vi "LabVIEW Function Structure.vi"() -> ()   [LabVIEW 2017]
uses:
  Picture/Home.ctl
  Picture/Machine Paramter and Control.ctl
  Picture/Vision Paramter and Control.ctl
  Picture/Machine Alarm History.ctl
  Picture/Machine Information.ctl
  Picture/Pause.ctl
  Picture/Start.ctl
  Picture/Stop.ctl
  Picture/Open Image File.ctl
  Picture/Open Excel File.ctl
  Picture/User Login.ctl
  Picture/SaveButtom.ctl
  Picture/Data and Run Information new.ctl
  <vilib>/vision/Image Controls.llb/IMAQ Image.ctl
  <vilib>/userdefined/High Color/IMAQdx.ctl
  SubVIs/Global System.vi
  SubVIs/Trige.vi
  <vilib>/Utility/file.llb/Write Delimited Spreadsheet (string).vi
  <vilib>/Utility/file.llb/Write Delimited Spreadsheet (DBL).vi
  <vilib>/Utility/file.llb/Read Delimited Spreadsheet (string).vi
  <resource>/objmgr/imaqdx.rc
panel:
  out "Message":string
  out "引用输出":refnum<k24>
  out "数字 3":dbl
  out "字符串":string
  out "元素":string
  out "数据上传OK/NG 2":bool
  out "路径 2":path
  out "压力表有无 2":string="0"
  out "压力表代码":string
  out "压力表有无":string
  out "连接的字符串":string
  out "数组 2":T1[](array[typedef])
  out "夹爪压力保存路径":path
  out "工单数量":string
  out "压力表类型":string
  out "工单号":string
  out "T/F":string
  out "ValidateBarcode":string="True,10270194,C.0C.50E,Firehawk药物支架系统（CE无标签）RV3035,RV3035,10"
  out "字符一致性连接的字符串":string
  out "computer3":string
  out "computer2":string
  out "computer1":string
  out "运行时间 4":dbl
  in  "前后位置切换":bool
  out "穿管检测初始化状态":bool
  out "穿管压力获取初始化状态":bool
  out "表面检测初始化状态":bool
  out "表面检测处理初始化状态":bool
  out "字符检测初始化状态":bool
  out "扫码枪初始化状态":bool
  out "task out Input 2":refnum<k7>
  out "task out Output 2":refnum<k7>
  out "项名称 2":string[](array[string])
  out "All Files in Dir 2":path[](array[path]) caption="目录中的所有文件"
  in  "数组":dbl[](array[numeric])=[1.0, 2.0, 3.0, 4.0, 5.0, 6.0, 7.0, 8.0, 9.0, 10.0, 11.0, 12.0, 13.0, 14.0, 15.0, 16.0, 17.0, 18.0, 19.0]
  out "Start Time 3":u32
  out "CCD6":path
  out "task out Output":refnum<k7>
  out "task out Input":refnum<k7>
  in  "选项卡控件":T2(tab)
  in  "数值":dbl format="%#_13g"
  in  "选项卡控件 2":enum32{"选项卡 1", "选项卡 2", "选项卡 3"}(tab)
  out "表面检测相机5":T1(plugin-control)
  out "表面检测相机4":T1(plugin-control)
  out "表面检测相机3":T1(plugin-control)
  out "衬丝检测":T1(plugin-control)
  in  "返工按钮":bool
  out "字符比对":bool
  out "穿管相机1":T1(plugin-control)
  out "字符检测相机6":T1(plugin-control)
  in  "穿管触发":bool=TRUE
  out "穿管相机2":T1(plugin-control)
  in  "表面检测触发":bool=TRUE
  in  "字符检测触发":bool=TRUE
  out "XY Graph":cluster{"Y":dbl[], "Y":dbl[]}[](graph) caption="压力-位置图"
  out "相机字符识别":string
  out "扫码枪字符识别":string
  in  "扫码枪触发":bool
  in  "穿管结果强制":bool
  out "传递信息显示":string
  out "x/y":dbl
  out "数据上传OK/NG":bool
  out "穿管产品型号":string[](array[string])
  out "表面产品型号":string[](array[string])
  out "产品型号":string
  out "模板匹配OK/NG":bool
  out "相机A":T1(plugin-control)
  in  "CCDA手动触发":bool
  out "字符方向判定结果":bool
  out "通讯状态":bool
  out "DB5000X-IsSuccess":bool
  out "DB5000R-IsSuccess":bool
  out "DB5000W":bool
  out "设备状态":string="Please Click Start Botton\n------------------------------------"
  out "lock":bool
  out "Tel":string="何东坡 15850164018"
  out "SoftWare Name":string="何东坡 15850164018"
  out "Company Name":string="昆山嘉斯特自动化\n\n昆山嘉斯特自动化"
  out "SW  Updated :":string="#1"
  out "SW  Rev :":string="1.0.0.0V"
  out "Build Date :":string="2018/10/20"
  out "Machine Factor":string[][](table)=[["MOTION", "LIGHT", "SCAN", "VISION"]]
  in  "电脑一表面检测图像处理状态":bool
  in  "电脑一CCD读字符状态":bool
  in  "电脑一穿管检测状态":bool
  in  "电脑一穿管压力获取状态":bool
  in  "电脑一条码枪扫码状态":bool
  in  "确定按钮":bool
  out "结果":string
  in  "输入":string
  in  "压力表数据库":string[][](table)=[["C.0C.01B", "C.0C.19B", "C.0C.01C", "C.0C.19C", "C.0B.0QE", "C.0B.40E"], ["C.0C.02B", "C.0C.74B", "C.0C.02C", "C.0C.20C", "C.0B.0RE", "C.0B.41E"], ["C.0C.03B", "C.0C.24B", "C.0C.03C", "C.0C.21C", "C.0B.0SE", "C.0B.02E"], ["C.0C.04B", "C.0C.20B", "C.0C.04C", "C.0C.22C", "C.0B.0TE", "C.0B.03E"], ["C.0C.05B", "C.0C.78B", "C.0C.05C", "C.0C.23C", "C.0B.0UE", "C.0B.42E"], ["C.0C.06B", "C.0C.25B", "C.0C.06C", "C.0C.24C", "C.0B.0VE", "C.0B.43E"], ["C.0C.07B", "C.0C.19G", "C.0C.07C", "C.0C.25C", "C.0B.0WE", "C.0B.06E"], ["C.0C.08B", "C.0C.20G", "C.0C.08C", "C.0C.26C", "C.0B.0XE", "C.0B.07E"], ["C.0C.09B", "C.0C.24G", "C.0C.09C", "C.0C.27C", "C.0B.0YE", "C.0B.44E"], ["C.0C.10B", "C.0C.25G", "C.0C.10C", "C.0C.28C", "C.0B.0ZE", "C.0B.45E"], ["C.0C.11B", "C.0A.0JD", "C.0C.11C", "C.0C.30C", "C.0B.10E", "C.0B.63E"], ["C.0C.12B", "C.0A.0KD", "C.0C.12C", "C.0C.51C", "C.0B.11E", "C.0B.11E"], ["C.0C.13B", "C.0A.0PD", "C.0C.13C", "C.0C.52C", "C.0B.12E", "C.0B.46E"], ["C.0C.14B", "C.0A.0QD", "C.0C.14C", "C.0C.53C", "C.0B.13E", "C.0B.47E"], ["C.0C.15B", "C.0A.16D", "C.0C.15C", "C.0C.54C", "C.0B.14E", "C.0B.64E"], ["C.0C.16B", "C.0A.1AD", "C.0C.16C", "C.0C.55C", "C.0B.15E", "C.0B.15E"], ["C.0C.17B", "", "C.0C.17C", "C.0C.56C", "C.0B.16E", "C.0B.04F"], ["C.0C.18B", "", "C.0C.18C", "C.0C.57C", "C.0B.17E", "C.0B.05F"], ["C.0C.21B", "", "C.0C.31C", "C.0C.58C", "C.0B.18E", "C.0B.06F"], ["C.0C.22B", "", "C.0C.32C", "C.0C.59C", "C.0B.19E", "C.0B.07F"], ["C.0C.23B", "", "C.0C.33C", "C.0C.60C", "C.0B.1AE", "C.0B.08F"], ["C.0C.59B", "", "C.0C.34C", "C.0C.19E", "C.0B.1BE", "C.0B.09F"], ["C.0C.60B", "", "C.0C.35C", "C.0C.20E", "C.0B.1CE", "C.0B.10F"], ["C.0C.61B", "", "C.0C.36C", "C.0C.21E", "C.0B.1DE", "C.0B.11F"], ["C.0C.62B", "", "C.0C.37C", "C.0C.22E", "C.0B.1EE", "C.0B.12F"], ["C.0C.63B", "", "C.0C.38C", "C.0C.23E", "C.0B.1FE", "C.0B.13F"], ["C.0C.64B", "", "C.0C.39C", "C.0C.24E", "C.0B.1GE", "C.0B.14F"], ["C.0C.65B", "", "C.0C.40C", "C.0C.25E", "C.0B.1HE", "C.0B.15F"], ["C.0C.66B", "", "C.0C.41C", "C.0C.26E", "C.0B.1KE", ""], ["C.0C.67B", "", "C.0C.42C", "C.0C.27E", "C.0B.1LE", ""], ["C.0C.68B", "", "C.0C.43C", "C.0C.28E", "C.0B.1NE", ""], ["C.0C.69B", "", "C.0C.44C", "C.0C.51E", "C.0B.1QE", ""], ["C.0C.70B", "", "C.0C.45C", "C.0C.52E", "C.0B.1SE", ""], ["C.0C.71B", "", "C.0C.46C", "C.0C.53E", "C.0B.1EE", ""], ["C.0C.72B", "", "C.0C.47C", "C.0C.54E", "C.0B.1FE", ""], ["C.0C.73B", "", "C.0C.48C", "C.0C.55E", "C.0B.0QE", ""], ["C.0C.75B", "", "C.0C.49C", "C.0C.56E", "C.0B.0RE", ""], ["C.0C.76B", "", "C.0C.50C", "C.0C.57E", "C.0B.1GE", ""], ["C.0C.77B", "", "C.0C.29C", "C.0C.58E", "C.0B.1HE", ""], ["C.0C.01G", "", "C.0C.01E", "C.0C.59E", "C.0B.0UE", ""], ["C.0C.02G", "", "C.0C.02E", "C.0C.60E", "C.0B.0VE", ""], ["C.0C.03G", "", "C.0C.03E", "C.0C.19H", "C.0B.0WE", ""], ["C.0C.04G", "", "C.0C.04E", "C.0C.20H", "C.0B.1KE", ""], ["C.0C.05G", "", "C.0C.05E", "C.0C.21H", "C.0B.1LE", ""], ["C.0C.06G", "", "C.0C.06E", "C.0C.22H", "C.0B.0YE", ""], ["C.0C.07G", "", "C.0C.07E", "C.0C.23H", "C.0B.0ZE", ""], ["C.0C.08G", "", "C.0C.08E", "C.0C.24H", "C.0B.10E", ""], ["C.0C.09G", "", "C.0C.09E", "C.0C.25H", "C.0B.1NE", ""], ["C.0C.10G", "", "C.0C.10E", "C.0C.26H", "C.0B.12E", ""], ["C.0C.11G", "", "C.0C.11E", "C.0C.27H", "C.0B.13E", ""], ["C.0C.12G", "", "C.0C.12E", "C.0C.28H", "C.0B.14E", ""], ["C.0C.13G", "", "C.0C.13E", "C.0C.29H", "C.0B.1QE", ""], ["C.0C.14G", "", "C.0C.14E", "C.0C.30H", "C.0B.16E", ""], ["C.0C.15G", "", "C.0C.15E", "", "C.0B.17E", ""], ["C.0C.16G", "", "C.0C.16E", "", "C.0B.18E", ""], ["C.0C.17G", "", "C.0C.17E", "", "C.0B.1SE", ""], ["C.0C.18G", "", "C.0C.18E", "", "C.0B.1AE", ""], ["C.0C.21G", "", "C.0C.29E", "", "C.0B.1BE", ""], ["C.0C.22G", "", "C.0C.30E", "", "C.0B.1CE", ""], ["C.0C.23G", "", "C.0C.31E", "", "C.0B.31B", ""], ["C.0A.00D", "", "C.0C.32E", "", "C.0B.32B", ""], ["C.0A.01D", "", "C.0C.33E", "", "C.0B.33B", ""], ["C.0A.02D", "", "C.0C.34E", "", "C.0B.34B", ""], ["C.0A.03D", "", "C.0C.35E", "", "C.0B.35B", ""], ["C.0A.04D", "", "C.0C.36E", "", "C.0B.36B", ""], ["C.0A.05D", "", "C.0C.37E", "", "C.0B.37B", ""], ["C.0A.06D", "", "C.0C.38E", "", "C.0B.38B", ""], ["C.0A.07D", "", "C.0C.39E", "", "C.0B.39B", ""], ["C.0A.08D", "", "C.0C.40E", "", "C.0B.3AB", ""], ["C.0A.09D", "", "C.0C.41E", "", "C.0B.3BB", ""], ["C.0A.0AD", "", "C.0C.42E", "", "C.0B.3CB", ""], ["C.0A.0BD", "", "C.0C.43E", "", "C.0B.1EB", ""], ["C.0A.0CD", "", "C.0C.44E", "", "C.0B.1FB", ""], ["C.0A.0DD", "", "C.0C.45E", "", "C.0B.1GB", ""], ["C.0A.0ED", "", "C.0C.46E", "", "C.0B.12B", ""], ["C.0A.0FD", "", "C.0C.47E", "", "C.0B.1HB", ""], ["C.0A.0GD", "", "C.0C.48E", "", "C.0B.14B", ""], ["C.0A.0HD", "", "C.0C.49E", "", "C.0B.1JB", ""], ["C.0A.0LD", "", "C.0C.50E", "", "C.0B.16B", ""], ["C.0A.0MD", "", "C.0C.51E", "", "C.0B.1KB", ""], ["C.0A.0ND", "", "C.0C.52E", "", "C.0B.18B", ""], ["C.0A.0RD", "", "C.0C.53E", "", "C.0B.1LB", ""], ["C.0A.0SD", "", "C.0C.54E", "", "C.0B.1CB", ""], ["C.0A.0TD", "", "C.0C.55E", "", "C.0B.1MB", ""], ["C.0A.0UD", "", "C.0C.56E", "", "C.0B.1NB", ""], ["C.0A.0VD", "", "C.0C.57E", "", "C.0B.1PB", ""], ["C.0A.0WD", "", "C.0C.58E", "", "C.0B.1QB", ""], ["C.0A.0XD", "", "C.0C.59E", "", "C.0B.1RB", ""], ["C.0A.0YD", "", "C.0C.60E", "", "C.0B.1SB", ""], ["C.0A.0ZD", "", "C.0C.01H", "", "C.0B.1TB", ""], ["C.0A.10D", "", "C.0C.02H", "", "C.0B.1UB", ""], ["C.0A.11D", "", "C.0C.03H", "", "C.0B.1VB", ""], ["C.0A.12D", "", "C.0C.04H", "", "C.0B.1WB", ""], ["C.0A.13D", "", "C.0C.05H", "", "C.0B.1XB", ""], ["C.0A.14D", "", "C.0C.06H", "", "C.0B.1YB", ""], ["C.0A.15D", "", "C.0C.07H", "", "C.0B.1ZB", ""], ["C.0A.17D", "", "C.0C.08H", "", "C.0B.13B", ""], ["C.0A.18D", "", "C.0C.09H", "", "C.0B.21B", ""], ["C.0A.19D", "", "C.0C.10H", "", "C.0B.22B", ""], ["C.0A.1BD", "", "C.0C.11H", "", "C.0B.23B", ""], ["C.0A.1CD", "", "C.0C.12H", "", "C.0B.15B", ""], ["C.0A.1DD", "", "C.0C.13H", "", "C.0B.25B", ""], ["C.0A.1ED", "", "C.0C.14H", "", "C.0B.26B", ""], ["C.0A.1FD", "", "C.0C.15H", "", "C.0B.27B", ""], ["C.0A.1GD", "", "C.0C.16H", "", "C.0B.17B", ""], ["C.0A.1HD", "", "C.0C.17H", "", "C.0B.29B", ""], ["C.0A.1JD", "", "C.0C.18H", "", "C.0B.2AB", ""], ["C.0A.1KD", "", "C.0C.19H", "", "C.0B.2BB", ""], ["C.0A.1LD", "", "C.0C.20H", "", "C.0B.19B", ""], ["C.0A.1MD", "", "C.0C.21H", "", "C.0B.2DB", ""], ["C.0A.1ND", "", "C.0C.22H", "", "C.0B.2EB", ""], ["C.0A.1PD", "", "C.0C.23H", "", "C.0B.2FB", ""], ["", "", "C.0C.24H", "", "C.0B.2GB", ""], ["", "", "C.0C.25H", "", "C.0B.1AB", ""], ["", "", "C.0C.26H", "", "C.0B.1BB", ""], ["", "", "C.0C.27H", "", "C.0B.2KB", ""], ["", "", "C.0C.28H", "", "C.0B.2LB", ""], ["", "", "C.0C.29H", "", "C.0B.2MB", ""], ["", "", "C.0C.30H", "", "C.0B.1DB", ""], ["", "", "C.04.001", "", "C.0B.2PB", ""], ["", "", "C.04.002", "", "C.0B.2QB", ""], ["", "", "C.04.003", "", "C.0B.2RB", ""], ["", "", "C.04.004", "", "C.0B.2SB", ""], ["", "", "C.04.005", "", "C.0B.2TB", ""], ["", "", "C.04.006", "", "C.0B.2UB", ""], ["", "", "C.04.007", "", "C.0B.2VB", ""], ["", "", "C.04.008", "", "C.0B.2WB", ""], ["", "", "C.04.009", "", "C.0B.2XB", ""], ["", "", "C.04.010", "", "C.0B.2YB", ""], ["", "", "C.04.011", "", "C.0B.2ZB", ""], ["", "", "C.04.012", "", "C.0B.30B", ""], ["", "", "C.04.013", "", "C.0B.48E", ""], ["", "", "C.04.014", "", "C.0B.49E", ""], ["", "", "C.04.015", "", "C.0B.65E", ""], ["", "", "C.04.016", "", "C.0B.19E", ""], ["", "", "C.04.017", "", "C.0B.50E", ""], ["", "", "C.04.018", "", "C.0B.51E", ""], ["", "", "C.04.019", "", "C.0B.22E", ""], ["", "", "C.04.020", "", "C.0B.23E", ""], ["", "", "C.04.021", "", "C.0B.52E", ""], ["", "", "C.04.022", "", "C.0B.53E", ""], ["", "", "C.04.023", "", "C.0B.26E", ""], ["", "", "C.04.024", "", "C.0B.27E", ""], ["", "", "C.04.025", "", "C.0B.54E", ""], ["", "", "C.04.026", "", "C.0B.30E", ""], ["", "", "C.04.027", "", "C.0B.31E", ""], ["", "", "C.04.028", "", "C.0B.55E", ""], ["", "", "C.04.029", "", "C.0B.56E", ""], ["", "", "C.04.030", "", "C.0B.57E", ""], ["", "", "C.04.031", "", "C.0B.58E", ""], ["", "", "C.04.032", "", "C.0B.34E", ""], ["", "", "C.04.033", "", "C.0B.35E", ""], ["", "", "C.04.034", "", "C.0B.59E", ""], ["", "", "C.04.035", "", "C.0B.60E", ""], ["", "", "C.04.036", "", "C.0B.61E", ""], ["", "", "C.04.037", "", "C.0B.62E", ""], ["", "", "C.04.038", "", "C.0B.38E", ""], ["", "", "C.04.039", "", "C.0B.39E", ""], ["", "", "C.04.040", "", "C.0B.16F", ""], ["", "", "C.04.041", "", "C.0B.17F", ""], ["", "", "C.04.042", "", "C.0B.18F", ""], ["", "", "C.04.043", "", "C.0B.19F", ""], ["", "", "C.04.044", "", "C.0B.20F", ""], ["", "", "C.04.045", "", "C.0B.21F", ""], ["", "", "C.04.046", "", "C.0B.22F", ""], ["", "", "C.04.047", "", "C.0B.23F", ""], ["", "", "C.04.048", "", "C.0B.24F", ""], ["", "", "C.04.049", "", "C.0B.25F", ""], ["", "", "C.04.050", "", "C.0B.26F", ""], ["", "", "C.04.051", "", "C.0B.27F", ""], ["", "", "C.04.052", "", "C.0B.28F", ""], ["", "", "C.04.053", "", "C.0B.29F", ""], ["", "", "C.04.054", "", "C.0B.30F", ""], ["", "", "C.04.055", "", "C.0B.31F", ""], ["", "", "C.04.056", "", "C.0B.32F", ""], ["", "", "C.04.057", "", "C.0B.33F", ""], ["", "", "C.04.058", "", "C.0B.34F", ""], ["", "", "C.04.059", "", "C.0B.35F", ""], ["", "", "C.04.060", "", "C.0B.36F", ""], ["", "", "C.08.001", "", "C.0B.37F", ""], ["", "", "C.08.002", "", "C.0B.38F", ""], ["", "", "C.08.003", "", "C.0B.39F", ""], ["", "", "C.08.004", "", "C.0B.40F", ""], ["", "", "C.08.005", "", "C.0B.41F", ""], ["", "", "C.08.006", "", "C.0B.42F", ""], ["", "", "C.08.007", "", "C.0B.30B", ""], ["", "", "C.08.008", "", "C.0B.2ZB", ""], ["", "", "C.08.009", "", "C.0B.2YB", ""], ["", "", "C.08.010", "", "C.0B.2XB", ""], ["", "", "C.08.011", "", "C.0B.2WB", ""], ["", "", "C.08.012", "", "C.0B.2VB", ""], ["", "", "C.08.013", "", "C.0B.2UB", ""], ["", "", "C.08.014", "", "C.0B.2TB", ""], ["", "", "C.08.015", "", "C.0B.2SB", ""], ["", "", "C.08.016", "", "C.0B.2RB", ""], ["", "", "C.08.017", "", "C.0B.2QB", ""], ["", "", "C.08.018", "", "C.0B.2PB", ""], ["", "", "C.08.019", "", "C.0B.1DB", ""], ["", "", "C.08.020", "", "C.0B.1CB", ""], ["", "", "C.08.021", "", "C.0B.2MB", ""], ["", "", "C.08.022", "", "C.0B.1LB", ""], ["", "", "C.08.023", "", "C.0B.2LB", ""], ["", "", "C.08.024", "", "C.0B.2KB", ""], ["", "", "C.08.025", "", "C.0B.1BB", ""], ["", "", "C.08.026", "", "C.0B.1AB", ""], ["", "", "C.08.027", "", "C.0B.2GB", ""], ["", "", "C.08.028", "", "C.0B.2FB", ""], ["", "", "C.08.029", "", "C.0B.2EB", ""], ["", "", "C.08.030", "", "C.0B.2DB", ""], ["", "", "C.08.031", "", "C.0B.19B", ""], ["", "", "C.08.032", "", "C.0B.18B", ""], ["", "", "C.08.033", "", "C.0B.2BB", ""], ["", "", "C.08.034", "", "C.0B.1KB", ""], ["", "", "C.08.035", "", "C.0B.2AB", ""], ["", "", "C.08.036", "", "C.0B.29B", ""], ["", "", "C.08.037", "", "C.0B.17B", ""], ["", "", "C.08.038", "", "C.0B.16B", ""], ["", "", "C.08.039", "", "C.0B.27B", ""], ["", "", "C.08.040", "", "C.0B.1JB", ""], ["", "", "C.08.041", "", "C.0B.26B", ""], ["", "", "C.08.042", "", "C.0B.25B", ""], ["", "", "C.08.043", "", "C.0B.15B", ""], ["", "", "C.08.044", "", "C.0B.14B", ""], ["", "", "C.08.045", "", "C.0B.23B", ""], ["", "", "C.08.046", "", "C.0B.1HB", ""], ["", "", "C.08.047", "", "C.0B.22B", ""], ["", "", "C.08.048", "", "C.0B.21B", ""], ["", "", "C.08.049", "", "C.0B.13B", ""], ["", "", "C.08.050", "", "C.0B.12B", ""], ["", "", "C.08.051", "", "C.0B.1ZB", ""], ["", "", "C.08.052", "", "C.0B.1GB", ""], ["", "", "C.08.053", "", "C.0B.1YB", ""], ["", "", "C.08.054", "", "C.0B.1XB", ""], ["", "", "C.08.055", "", "C.0B.1WB", ""], ["", "", "C.08.056", "", "C.0B.1FB", ""], ["", "", "C.08.057", "", "C.0B.1VB", ""], ["", "", "C.08.058", "", "C.0B.1EB", ""], ["", "", "C.08.059", "", "C.0B.1UB", ""], ["", "", "C.08.060", "", "C.0B.1TB", ""], ["", "", "", "", "C.0B.1SB", ""], ["", "", "", "", "C.0B.1RB", ""], ["", "", "", "", "C.0B.1QB", ""], ["", "", "", "", "C.0B.1PB", ""], ["", "", "", "", "C.0B.1NB", ""], ["", "", "", "", "C.0B.1MB", ""], ["", "", "", "", "C.0B.3CB", ""], ["", "", "", "", "C.0B.3BB", ""], ["", "", "", "", "C.0B.3AB", ""], ["", "", "", "", "C.0B.39B", ""], ["", "", "", "", "C.0B.38B", ""], ["", "", "", "", "C.0B.37B", ""], ["", "", "", "", "C.0B.36B", ""], ["", "", "", "", "C.0B.35B", ""], ["", "", "", "", "C.0B.34B", ""], ["", "", "", "", "C.0B.33B", ""], ["", "", "", "", "C.0B.32B", ""], ["", "", "", "", "C.0B.31B", ""], ["", "", "", "", "C.0B.1TE", ""], ["", "", "", "", "C.0B.1DE", ""], ["", "", "", "", "C.0B.1CE", ""], ["", "", "", "", "C.0B.1BE", ""], ["", "", "", "", "C.0B.1AE", ""], ["", "", "", "", "C.0B.1SE", ""], ["", "", "", "", "C.0B.18E", ""], ["", "", "", "", "C.0B.17E", ""], ["", "", "", "", "C.0B.16E", ""], ["", "", "", "", "C.0B.1QE", ""], ["", "", "", "", "C.0B.14E", ""], ["", "", "", "", "C.0B.13E", ""], ["", "", "", "", "C.0B.12E", ""], ["", "", "", "", "C.0B.1NE", ""], ["", "", "", "", "C.0B.10E", ""], ["", "", "", "", "C.0B.0ZE", ""], ["", "", "", "", "C.0B.0YE", ""], ["", "", "", "", "C.0B.1LE", ""], ["", "", "", "", "C.0B.1KE", ""], ["", "", "", "", "C.0B.0WE", ""], ["", "", "", "", "C.0B.0VE", ""], ["", "", "", "", "C.0B.0UE", ""], ["", "", "", "", "C.0B.1HE", ""], ["", "", "", "", "C.0B.1GE", ""], ["", "", "", "", "C.0B.0RE", ""], ["", "", "", "", "C.0B.0QE", ""], ["", "", "", "", "C.0B.1FE", ""], ["", "", "", "", "C.0B.1EE", ""]]
  in  "Save 压力表数据库 Message":T3
  in  "警报记录":string[][](table)
  in  "压力表打印代码据库":string[][](table)=[["C.0A.00D", "C.04.001", "C.0B.31B", ""], ["C.0A.01D", "C.04.002", "C.0B.32B", ""], ["C.0A.02D", "C.04.003", "C.0B.33B", ""], ["C.0A.03D", "C.04.004", "C.0B.34B", ""], ["C.0A.04D", "C.04.005", "C.0B.35B", ""], ["C.0A.05D", "C.04.006", "C.0B.36B", ""], ["C.0A.06D", "C.04.007", "C.0B.37B", ""], ["C.0A.07D", "C.04.008", "C.0B.38B", ""], ["C.0A.08D", "C.04.009", "C.0B.39B", ""], ["C.0A.09D", "C.04.010", "C.0B.3AB", ""], ["C.0A.0AD", "C.04.011", "C.0B.3BB", ""], ["C.0A.0BD", "C.04.012", "C.0B.3CB", ""], ["C.0A.0CD", "C.04.013", "C.0B.1MB", ""], ["C.0A.0DD", "C.04.014", "C.0B.1NB", ""], ["C.0A.0ED", "C.04.015", "C.0B.1PB", ""], ["C.0A.0FD", "C.04.016", "C.0B.1QB", ""], ["C.0A.0GD", "C.04.017", "C.0B.1RB", ""], ["C.0A.0HD", "C.04.018", "C.0B.1SB", ""], ["C.0A.0JD", "C.04.019", "C.0B.1TB", ""], ["C.0A.0KD", "C.04.020", "C.0B.1UB", ""], ["C.0A.0LD", "C.04.021", "C.0B.1VB", ""], ["C.0A.0MD", "C.04.022", "C.0B.1WB", ""], ["C.0A.0ND", "C.04.023", "C.0B.1XB", ""], ["C.0A.0PD", "C.04.024", "C.0B.1YB", ""], ["C.0A.0QD", "C.04.025", "C.0B.1ZB", ""], ["C.0A.0RD", "C.04.026", "C.0B.13B", ""], ["C.0A.0SD", "C.04.027", "C.0B.21B", ""], ["C.0A.0TD", "C.04.028", "C.0B.22B", ""], ["C.0A.0UD", "C.04.029", "C.0B.23B", ""], ["C.0A.0VD", "C.04.030", "C.0B.15B", ""], ["C.0A.0WD", "C.04.031", "C.0B.25B", ""], ["C.0A.0XD", "C.04.032", "C.0B.26B", ""], ["C.0A.0YD", "C.04.033", "C.0B.27B", ""], ["C.0A.0ZD", "C.04.034", "C.0B.17B", ""], ["C.0A.10D", "C.04.035", "C.0B.29B", ""], ["C.0A.11D", "C.04.036", "C.0B.2AB", ""], ["C.0A.12D", "C.04.037", "C.0B.2BB", ""], ["C.0A.13D", "C.04.038", "C.0B.19B", ""], ["C.0A.14D", "C.04.039", "C.0B.2DB", ""], ["C.0A.15D", "C.04.040", "C.0B.2EB", ""], ["C.0A.16D", "C.04.041", "C.0B.2FB", ""], ["C.0A.17D", "C.04.042", "C.0B.2GB", ""], ["C.0A.18D", "C.04.043", "C.0B.1AB", ""], ["C.0A.19D", "C.04.044", "C.0B.1BB", ""], ["C.0A.1AD", "C.04.045", "C.0B.2KB", ""], ["C.0A.1BD", "C.04.046", "C.0B.2LB", ""], ["C.0A.1CD", "C.04.047", "C.0B.2MB", ""], ["C.0A.1DD", "C.04.048", "C.0B.1DB", ""], ["C.0A.1ED", "C.04.049", "C.0B.2PB", ""], ["C.0A.1FD", "C.04.050", "C.0B.2QB", ""], ["C.0A.1GD", "C.04.051", "C.0B.2RB", ""], ["C.0A.1HD", "C.04.052", "C.0B.2SB", ""], ["C.0A.1JD", "C.04.053", "C.0B.2TB", ""], ["C.0A.1KD", "C.04.054", "C.0B.2UB", ""], ["C.0A.1LD", "C.04.055", "C.0B.2VB", ""], ["C.0A.1MD", "C.04.056", "C.0B.2WB", ""], ["C.0A.1ND", "C.04.057", "C.0B.2XB", ""], ["C.0A.1PD", "C.04.058", "C.0B.2YB", ""], ["C.0C.01B", "C.04.059", "C.0B.2ZB", ""], ["C.0C.02B", "C.04.060", "C.0B.30B", ""], ["C.0C.03B", "C.08.001", "C.0B.00N", " "], ["C.0C.04B", "C.08.002", "C.0B.01N", " "], ["C.0C.05B", "C.08.003", "C.0B.02N", " "], ["C.0C.06B", "C.08.004", "C.0B.03N", " "], ["C.0C.07B", "C.08.005", "C.0B.04N", " "], ["C.0C.08B", "C.08.006", "C.0B.05N", " "], ["C.0C.09B", "C.08.007", "C.0B.06N", " "], ["C.0C.10B", "C.08.008", "C.0B.07N", " "], ["C.0C.11B", "C.08.009", "C.0B.08N", " "], ["C.0C.12B", "C.08.010", "C.0B.09N", " "], ["C.0C.13B", "C.08.011", "C.0B.10N", " "], ["C.0C.14B", "C.08.012", "C.0B.11N", " "], ["C.0C.15B", "C.08.013", "C.0B.12N", " "], ["C.0C.16B", "C.08.014", "C.0B.13N", " "], ["C.0C.17B", "C.08.015", "C.0B.14N", " "], ["C.0C.18B", "C.08.016", "C.0B.15N", " "], ["C.0C.19B", "C.08.017", "C.0B.16N", " "], ["C.0C.20B", "C.08.018", "C.0B.17N", " "], ["C.0C.21B", "C.08.019", "C.0B.18N", " "], ["C.0C.22B", "C.08.020", "C.0B.19N", " "], ["C.0C.23B", "C.08.021", "C.0B.20N", " "], ["C.0C.24B", "C.08.022", "C.0B.21N", " "], ["C.0C.25B", "C.08.023", "C.0B.22N", " "], ["C.0C.59B", "C.08.024", "C.0B.23N", " "], ["C.0C.60B", "C.08.025", "C.0B.24N", " "], ["C.0C.61B", "C.08.026", "C.0B.25N", " "], ["C.0C.62B", "C.08.027", "C.0B.26N", " "], ["C.0C.63B", "C.08.028", "C.0B.27N", " "], ["C.0C.64B", "C.08.029", "C.0B.28N", " "], ["C.0C.65B", "C.08.030", "C.0B.29N", " "], ["C.0C.66B", "C.08.031", "C.0B.40E", " "], ["C.0C.67B", "C.08.032", "C.0B.41E", " "], ["C.0C.68B", "C.08.033", "C.0B.02E", " "], ["C.0C.69B", "C.08.034", "C.0B.03E", " "], ["C.0C.70B", "C.08.035", "C.0B.42E", " "], ["C.0C.71B", "C.08.036", "C.0B.43E", " "], ["C.0C.72B", "C.08.037", "C.0B.06E", " "], ["C.0C.73B", "C.08.038", "C.0B.07E", " "], ["C.0C.74B", "C.08.039", "C.0B.44E", " "], ["C.0C.75B", "C.08.040", "C.0B.45E", " "], ["C.0C.76B", "C.08.041", "C.0B.63E", " "], ["C.0C.77B", "C.08.042", "C.0B.11E", " "], ["C.0C.78B", "C.08.043", "C.0B.46E", " "], ["C.0C.01G", "C.08.044", "C.0B.47E", " "], ["C.0C.02G", "C.08.045", "C.0B.64E", " "], ["C.0C.03G", "C.08.046", "C.0B.15E", " "], ["C.0C.04G", "C.08.047", "C.0B.48E", " "], ["C.0C.05G", "C.08.048", "C.0B.49E", " "], ["C.0C.06G", "C.08.049", "C.0B.65E", " "], ["C.0C.07G", "C.08.050", "C.0B.19E", " "], ["C.0C.08G", "C.08.051", "C.0B.50E", " "], ["C.0C.09G", "C.08.052", "C.0B.51E", " "], ["C.0C.10G", "C.08.053", "C.0B.22E", " "], ["C.0C.11G", "C.08.054", "C.0B.23E", " "], ["C.0C.12G", "C.08.055", "C.0B.52E", " "], ["C.0C.13G", "C.08.056", "C.0B.53E", " "], ["C.0C.14G", "C.08.057", "C.0B.26E", " "], ["C.0C.15G", "C.08.058", "C.0B.27E", " "], ["C.0C.16G", "C.08.059", "C.0B.54E", " "], ["C.0C.17G", "C.08.060", "C.0B.30E", " "], ["C.0C.18G", "C.0C.01C", "C.0B.31E", " "], ["C.0C.19G", "C.0C.02C", "C.0B.55E", " "], ["C.0C.20G", "C.0C.03C", "C.0B.56E", " "], ["C.0C.21G", "C.0C.04C", "C.0B.57E", " "], ["C.0C.22G", "C.0C.05C", "C.0B.58E", " "], ["C.0C.23G", "C.0C.06C", "C.0B.34E", " "], ["C.0C.24G", "C.0C.07C", "C.0B.35E", " "], ["C.0C.25G", "C.0C.08C", "C.0B.59E", " "], [" ", "C.0C.09C", "C.0B.60E", " "], [" ", "C.0C.10C", "C.0B.61E", " "], [" ", "C.0C.11C", "C.0B.62E", " "], [" ", "C.0C.12C", "C.0B.38E", " "], [" ", "C.0C.13C", "C.0B.39E", " "], [" ", "C.0C.14C", "C.0B.0QE", " "], [" ", "C.0C.15C", "C.0B.0RE", " "], [" ", "C.0C.16C", "C.0B.0SE", " "], [" ", "C.0C.17C", "C.0B.0TE", " "], [" ", "C.0C.18C", "C.0B.0UE", " "], [" ", "C.0C.19C", "C.0B.0VE", " "], [" ", "C.0C.20C", "C.0B.0WE", " "], [" ", "C.0C.21C", "C.0B.0XE", " "], [" ", "C.0C.22C", "C.0B.0YE", " "], [" ", "C.0C.23C", "C.0B.0ZE", " "], [" ", "C.0C.24C", "C.0B.10E", " "], [" ", "C.0C.25C", "C.0B.11E", " "], [" ", "C.0C.26C", "C.0B.12E", " "], [" ", "C.0C.27C", "C.0B.13E", " "], [" ", "C.0C.28C", "C.0B.14E", " "], [" ", "C.0C.29C", "C.0B.15E", " "], [" ", "C.0C.30C", "C.0B.16E", " "], [" ", "C.0C.31C", "C.0B.17E", " "], [" ", "C.0C.32C", "C.0B.18E", " "], [" ", "C.0C.33C", "C.0B.19E", " "], [" ", "C.0C.34C", "C.0B.1AE", " "], [" ", "C.0C.35C", "C.0B.1BE", " "], [" ", "C.0C.36C", "C.0B.1CE", " "], [" ", "C.0C.37C", "C.0B.1DE", " "], [" ", "C.0C.38C", "C.0B.1EE", " "], [" ", "C.0C.39C", "C.0B.1FE", " "], [" ", "C.0C.40C", "C.0B.1GE", " "], [" ", "C.0C.41C", "C.0B.1HE", " "], [" ", "C.0C.42C", "C.0B.1KE", " "], [" ", "C.0C.43C", "C.0B.1LE", " "], [" ", "C.0C.44C", "C.0B.1NE", " "], [" ", "C.0C.45C", "C.0B.1QE", " "], [" ", "C.0C.46C", "C.0B.1SE", " "], [" ", "C.0C.47C", " ", ""], [" ", "C.0C.48C", " ", ""], [" ", "C.0C.49C", " ", ""], [" ", "C.0C.50C", " ", ""], [" ", "C.0C.51C", " ", ""], [" ", "C.0C.52C", " ", ""], [" ", "C.0C.53C", " ", ""], [" ", "C.0C.54C", " ", ""], [" ", "C.0C.55C", " ", ""], [" ", "C.0C.56C", " ", ""], [" ", "C.0C.57C", " ", ""], [" ", "C.0C.58C", " ", ""], [" ", "C.0C.59C", " ", ""], [" ", "C.0C.60C", " ", ""], [" ", "C.0C.01E", " ", ""], [" ", "C.0C.02E", " ", ""], [" ", "C.0C.03E", " ", ""], [" ", "C.0C.04E", " ", ""], [" ", "C.0C.05E", " ", ""], [" ", "C.0C.06E", " ", ""], [" ", "C.0C.07E", " ", ""], [" ", "C.0C.08E", " ", ""], [" ", "C.0C.09E", " ", ""], [" ", "C.0C.10E", " ", ""], [" ", "C.0C.11E", " ", ""], [" ", "C.0C.12E", " ", ""], [" ", "C.0C.13E", " ", ""], [" ", "C.0C.14E", " ", ""], [" ", "C.0C.15E", " ", ""], [" ", "C.0C.16E", " ", ""], [" ", "C.0C.17E", " ", ""], [" ", "C.0C.18E", " ", ""], [" ", "C.0C.19E", " ", ""], [" ", "C.0C.20E", " ", ""], [" ", "C.0C.21E", " ", ""], [" ", "C.0C.22E", " ", ""], [" ", "C.0C.23E", " ", ""], [" ", "C.0C.24E", " ", ""], [" ", "C.0C.25E", " ", ""], [" ", "C.0C.26E", " ", ""], [" ", "C.0C.27E", " ", ""], [" ", "C.0C.28E", " ", ""], [" ", "C.0C.29E", " ", ""], [" ", "C.0C.30E", " ", ""], [" ", "C.0C.31E", " ", ""], [" ", "C.0C.32E", " ", ""], [" ", "C.0C.33E", " ", ""], [" ", "C.0C.34E", " ", ""], [" ", "C.0C.35E", " ", ""], [" ", "C.0C.36E", " ", ""], [" ", "C.0C.37E", " ", ""], [" ", "C.0C.38E", " ", ""], [" ", "C.0C.39E", " ", ""], [" ", "C.0C.40E", " ", ""], [" ", "C.0C.41E", " ", ""], [" ", "C.0C.42E", " ", ""], [" ", "C.0C.43E", " ", ""], [" ", "C.0C.44E", " ", ""], [" ", "C.0C.45E", " ", ""], [" ", "C.0C.46E", " ", ""], [" ", "C.0C.47E", " ", ""], [" ", "C.0C.48E", " ", ""], [" ", "C.0C.49E", " ", ""], [" ", "C.0C.50E", " ", ""], [" ", "C.0C.51E", " ", ""], [" ", "C.0C.52E", " ", ""], [" ", "C.0C.53E", " ", ""], [" ", "C.0C.54E", " ", ""], [" ", "C.0C.55E", " ", ""], [" ", "C.0C.56E", " ", ""], [" ", "C.0C.57E", " ", ""], [" ", "C.0C.58E", " ", ""], [" ", "C.0C.59E", " ", ""], [" ", "C.0C.60E", " ", ""]]
  out "产品种类":string
  out "压力表打印代码":string
  in  "Type_b":bool
  in  "Type_c":bool
  in  "computer5":bool
  in  "computer4":bool
  in  "computer3":bool
  in  "computer2":bool
  in  "computer1":bool
  in  "清空数据库":bool
  in  "DB5000.X":T4
  in  "输出OUTPUT":T5
  out "输入INPUT":T6
  in  "PLC参数保存":T3
  out "盘管压力值 2":dbl[](array[numeric])
  in  "补偿值":dbl format="%#_13g"
  out "补偿后压力值":dbl format="%#_3g"
  out "数字":u32
  out "数字 2":u32
  out "衬丝口位置":string
  out "长短料":string
  out "粗细料":string
  out "一致性结果字符串":string
  out "ValidateBarcode 2":string="True,10270194,C.0C.50E,Firehawk药物支架系统（CE无标签）RV3035,RV3035,10"
  out "ValidateBarcode 3":string="True,10270194,C.0C.50E,Firehawk药物支架系统（CE无标签）RV3035,RV3035,10"
  out "夹爪压力值":dbl[](array[numeric])
  in  "DB5000.R":T7
  out "Content":u16
  in  "Vision Paramter Save Buttom":T3
  in  "文件名":string(tree)
  out "数据波形图":dbl[][](graph)
  in  "压力数据显示":string[][](table)
  out "查询图片":T1(plugin-control)
  in  "搜索历史图片":bool
  in  "搜索项":string(tree)
  in  "NG/OK":string(combo)="Image"
  in  "检索条件":string(combo)="CCD6"
  out "Ground 2":u16(ring) items=["Administrator", "Engineer", "Operator"]
  in  "Other Param Save Buttom":T3
  out "Start Time 2":u32
  out "CCD2":path
  out "项名称":string[](array[string])
  out "All Files in Dir":path[](array[path]) caption="目录中的所有文件"
  out "CCD1":path
  in  "logo":T8
  out "CMD":string
  out "路径":path
  in  "Auto Run Load Program Name":string(combo)
  in  "Data and Run Information":T9
  in  "User Login":T10
  in  "Open Excel File":T11
  in  "Open Image File":T12
  in  "Stop":T13
  in  "Start":T14
  in  "Pause":T15
  in  "Machine Inforamtion":T16
  in  "Machine Alarm Histroy":T17
  in  "Vision Paramter and Control":T18
  in  "Machine Paramter and Control":T19
  in  "Home":T20
  in  "计数器清零":bool
  out "条码名称":string="Default"
  out "system time":string
  # "检测孔径检测流程"
  # "孔径判定结果"
  # "Standby"
  # "PLC孔径启动信号"
  # "检测孔径尺寸"
  # "铜片检测流程"
  # "铜片检测结果输出"
  # "Standby"
  # "PLC铜片启动信号"
  # "检测孔径"
  # "LoadSystem"
  # "判定结果"
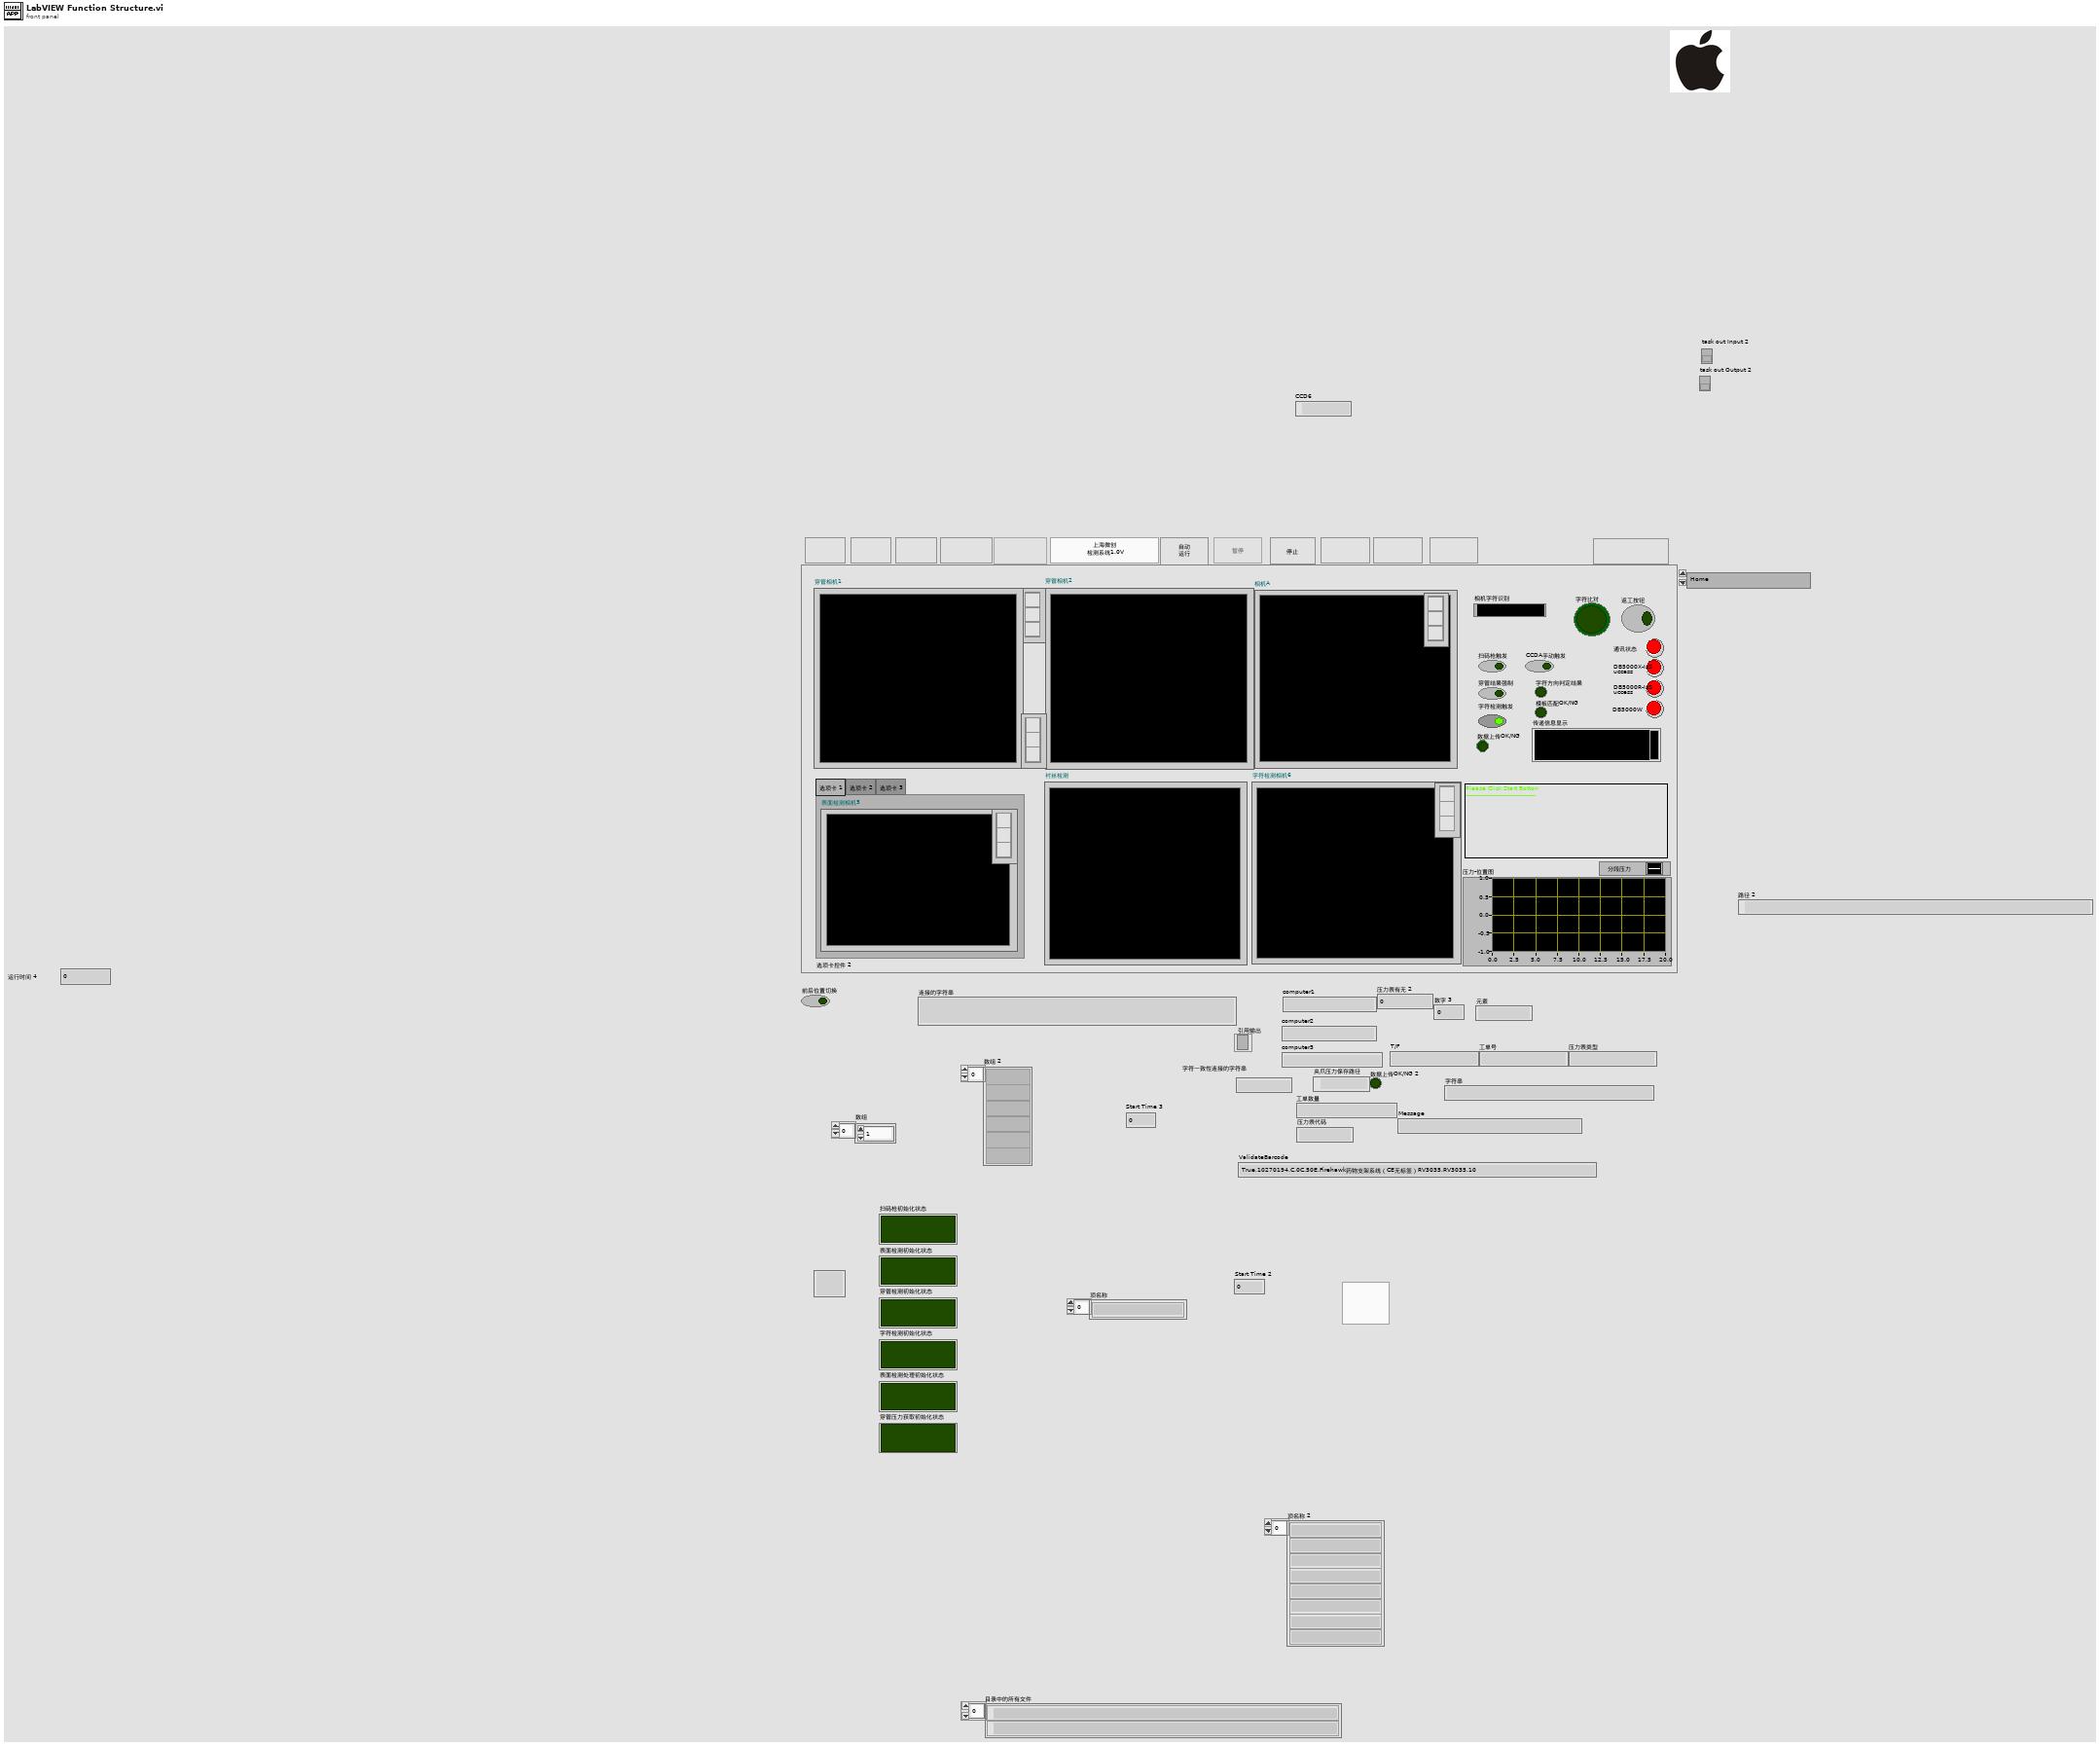
[diagram p1: front panel]
types:
  T1 = typedef "IMAQ Image.ctl" = refnum<image>
  T2 = enum32{"Home", "Machine Information", "Machine Alarm History", "Data and Run Information ", "Machine Paramter and Control", "Vision Paramter and Contorol", "Open Excel File", "Open Image File"}
  T3 = typedef "SaveButtom.ctl" = bool
  T4 = cluster{"字符识别启动\n信号-读":bool, "电脑1扫码枪\n触发-读":bool, "电脑1CCD读取\n字符触发-读":bool, "电脑1表面检测\n触发-读":bool, "电脑1穿管检测\n触发-读":bool, "区间位置\n1-读":bool, "区间位置\n2-读":bool, "区间位置\n3-读":bool, "区间位置\n4-读":bool, "区间位置\n5-读":bool, "区间位置\n6-读":bool, "区间位置\n7-读":bool, "区间位置\n8-读":bool, "区间位置\n9-读":bool, "区间位置\n10-读":bool, "区间位置\n11-读":bool, "区间位置\n12-读":bool, "区间位置\n13-读":bool, "区间位置\n14-读":bool, "区间位置\n15-读":bool, "区间位置\n16-读":bool, "区间位置\n17-读":bool, "区间位置\n18-读":bool, "区间位置\n19-读":bool, "夹爪1\n状态-读":bool, "夹爪2\n状态-读":bool, "夹爪3\n状态-读":bool, "夹爪\n4状态-读":bool, "夹爪\n5状态-读":bool, "夹爪\n6状态-读":bool, "夹爪7\n状态-读":bool, "夹爪8\n状态-读":bool, "夹爪9\n状态-读":bool, "夹爪10\n状态-读":bool, "前后位置\n切换触发-读":bool, "电脑1压力获取\n触发-读":bool, "PC1 ready-\n写 ":bool, "混料-写\n":bool, "字符1检测\npass-写":bool, "字符1检测\nfail-写":bool, "表面检测\npass-写":bool, "表面检测\nfail-写":bool, "穿管检测\npass-写":bool, "穿管检测\nfail-写":bool, "扫码枪\npass-写":bool, "扫码枪fail-\n写":bool, "产品尺寸A-\n写":bool, "产品尺寸B-\n写":bool, "数据传递\n信号-读":bool, "表面检测完\n成信号-读":bool, "穿管NG停止\n信号-写":bool, "电脑1返工\n信号-写":bool, "PLC初始化\n信号-读":bool, "产品尺寸C-\n写":bool, "表面检测错位\n气缸-读":bool, "电脑1衬丝检测\n触发-读":bool, "衬丝能检测\npass-写":bool, "衬丝能检测f\nail-写":bool, "长衬丝-写\n":bool, "短衬丝-写\n":bool, "细料-写":bool, "粗料-写":bool, "一致性检测\n触发-读":bool}
  T5 = cluster{"字符检测pass":bool, "字符检测fail":bool, "表面检测pass":bool, "表面检测fail":bool, "穿管检测pass":bool, "穿管检测fail":bool, "PC1 Ready":bool, "混料":bool, "产品尺寸":bool, "备用1":bool, "字符检测就绪":bool, "表面检测测就绪":bool, "穿管测就绪":bool, "备用2":bool, "备用3":bool, "备用4":bool}
  T6 = cluster{"位置1":bool, "位置2":bool, "位置3":bool, "位置4":bool, "位置6":bool, "位置7":bool, "位置8":bool, "位置9":bool, "位置11":bool, "位置12":bool, "位置13":bool, "位置14":bool, "位置16":bool, "位置17":bool, "位置18":bool, "位置19":bool, "字符检测1触发":bool, "表面检测触发":bool, "穿管检测触发":bool, "位置切换触发":bool, "位置5":bool, "位置10":bool, "位置15":bool, "扫码枪触发":bool, "备用":bool}
  T7 = cluster{"夹爪1压力值":sgl, "夹爪2压力值":sgl, "夹爪3压力值":sgl, "夹爪4压力值":sgl, "夹爪5压力值":sgl, "夹爪6压力值":sgl, "夹爪7压力值":sgl, "夹爪8压力值":sgl, "夹爪9压力值":sgl, "夹爪10压力值":sgl, "盘管底部压力值":sgl, "备用1":sgl, "备用2":sgl, "备用3":sgl, "备用4":sgl}
  T8 = typedef "三星logo.ctl" = bool
  T9 = typedef "Data and Run Information new.ctl" = bool
  T10 = typedef "User Login.ctl" = bool
  T11 = typedef "Open Excel File.ctl" = bool
  T12 = typedef "Open Image File.ctl" = bool
  T13 = typedef "Stop.ctl" = bool
  T14 = typedef "Start.ctl" = bool
  T15 = typedef "Pause.ctl" = bool
  T16 = typedef "Machine Information.ctl" = bool
  T17 = typedef "Machine Alarm History.ctl" = bool
  T18 = typedef "Vision Paramter and Control.ctl" = bool
  T19 = typedef "Machine Paramter and Control.ctl" = bool
  T20 = typedef "Home.ctl" = bool
  T21 = cluster{"index":i32, "this vi":refnum<vi>, "step":cluster{"test step":string[], "step status":bool[], "step index":i32}, "用户登录":cluster{"admin":cluster{"用户名":string[], "密码":string[]}, "engineer":cluster{"用户名":string[], "密码":string[]}, "operator":cluster{"用户名":string[], "密码":string[]}}, "用户权限":i32, "error out":errorcluster, "AllStepNumber":i32, "Run ErrNumber":string, "LoadProgram":string, "TotalNumber":string, "PassNumber":string, "FailNumber":string, "Start Time":string, "2 Pause Message":string, "3 Pause Message":string, "4 Pause Message":string}
  T22 = enum8{"Enabled", "Disabled", "Disabled and Grayed Out"}
  T23 = typedef "Semaphore RefNum" = refnum<k1>
  T24 = cluster{"master data":string, "priority":u16, "secondary data":string[]}
  T25 = cluster{"case name":string[], "queue array":refnum<queue>[]}
  T26 = cluster{"地址":string, "远程端口或服务名称":u16, "超时秒数":dbl}
  T27 = typedef "Image Type" = u32
  T28 = typedef "IMAQdx.ctl" = refnum<k21>
  T29 = cluster{"admin":cluster{"用户名":string[], "密码":string[]}, "engineer":cluster{"用户名":string[], "密码":string[]}, "operator":cluster{"用户名":string[], "密码":string[]}}
  T30 = cluster{"IsNorImage":bool, "Exposure Values":u32, "ImagePath":path}
  T31 = typedef "IMAQ Rectangle" = cluster{"Left":i32, "Top":i32, "Right":i32, "Bottom":i32, "Rotation":dbl}
  T32 = cluster{"Parameters (OCR/OCV 1)":cluster{"Threshold Data":cluster{"Method":enum16{"Fixed Range", "Uniform", "Linear", "Non Linear", "Local", "Color"}, "Looking for":u32, "Color Mode":u32, "Kernel Size":cluster{"Width":i32, "Height":i32}, "Ranges":cluster{"Min":i32, "Max":i32}[]}, "Reject Border":bool, "Number Of Erosions":i32, "Size & Spacing":cluster{"Segment Algorithm":u16, "Min Bounding Rect Width":i32, "Max Bounding Rect Width":i32, "Min Bounding Rect Height":i32, "Max Bounding Rect Height":i32, "Min Character Size":i32, "Max Character Size":i32, "Min Char Spacing":i32, "Max Horiz Element Spacing":i32, "Max Vert Element Spacing":i32, "Max Space Distance":i32}, "Read Options":cluster{"Read Strategy":i32, "Read Resolution":i32, "Scale Dependant":bool, "Aspect Ratio":i32, "Acceptance Level":i32, "Substitution Character":string, "MultiLine":bool}, "Valid Characters":cluster{"Pre-defined characters":i32, "User-defined characters":string}[], "Use Text Pattern":bool, "Orientation":u32, "# Lines Expected":u32, "Number of Blocks":i32}, "Rectangle":T31, "字符长度判定":dbl, "Reference System":cluster{"Origin":cluster{"X":sgl, "Y":sgl}, "Angle (deg)":sgl, "Axis Reference":u32}, "File Path (字符库)":path, "File Path (连接件模板)":path, "Url":string, "accessKey":string}
  T33 = typedef "IMAQ Curve Parameters.ctl" = cluster{"Extraction Mode":u32, "Edge Threshold":i32, "Edge Filter Size":u32, "Min Length":i32, "Row Search Step Size":i32, "Col Search Step Size":i32, "Max Endpoint Gap":i32, "Closed":bool, "Subpixel":bool}
  T34 = typedef "IMAQ Match Range Setting.ctl" = cluster{"Match Constraints":u32, "Min":dbl, "Max":dbl}
  T35 = cluster{"Rectangle":T31, "Settings":cluster{"Curve Parameters":T33, "Match Mode":cluster{"Rotation":bool, "Scale":bool, "Occlusion":bool, "Reserved 1":bool, "Reserved 2":bool, "Reserved 3":bool}, "Range Settings":T34[], "Number of Matches":i32, "Minimum Match Score":sgl, "SubPixel Accuracy":bool, "Adv. Geometric Match Options 2":cluster{"Setup Data Item":u16, "Item Value":dbl}[]}, "Template File Path":path}
  T36 = cluster{"字符识别启动信号-读":bool, "电脑1扫码枪\n触发-读":bool, "电脑1CCD读取\n字符触发-读":bool, "电脑1表面检测\n触发-读":bool, "电脑1穿管检测\n触发-读":bool, "区间位置1-读":bool, "区间位置2-读":bool, "区间位置3-读":bool, "区间位置4-读":bool, "区间位置5-读":bool, "区间位置6-读":bool, "区间位置7-读":bool, "区间位置8-读":bool, "区间位置9-读":bool, "区间位置10-读":bool, "区间位置11-读":bool, "区间位置12-读":bool, "区间位置13-读":bool, "区间位置14-读":bool, "区间位置15-读":bool, "区间位置16-读":bool, "区间位置17-读":bool, "区间位置18-读":bool, "区间位置19-读":bool, "夹爪1状态-读":bool, "夹爪2状态-读":bool, "夹爪3状态-读":bool, "夹爪4状态-读":bool, "夹爪5状态-读":bool, "夹爪6状态-读":bool, "夹爪7状态-读":bool, "夹爪8状态-读":bool, "夹爪9状态-读":bool, "夹爪10状态-读":bool, "电脑1产品前后位置\n切换触发-读":bool, "电脑1压力获取\n触发-读":bool, "PC1 ready-写 ":bool, "混料-写":bool, "字符1检测pass-写":bool, "字符1检测fail-写":bool, "表面检测pass-写":bool, "表面检测fail-写":bool, "穿管检测pass-写":bool, "穿管检测fail-写":bool, "扫码枪pass-写":bool, "扫码枪fail-写":bool, "产品尺寸A-写":bool, "产品尺寸B-写":bool, "数据传递信号-读":bool, "表面检测完成信号-读":bool, "穿管NG停止信号-写":bool, "电脑1返工信号-写":bool, "PLC初始化信号-读":bool, "产品尺寸C-写":bool, "表面检测错位气缸-读":bool, "电脑1衬丝检测触发-读":bool, "衬丝能检测pass-写":bool, "衬丝能检测fail-写":bool, "长衬丝-写":bool, "短衬丝-写":bool, "细料-写":bool, "粗料-写":bool, "一致性检测触发-读":bool}
  T37 = typedef "Edge Options.ctl" = cluster{"Edge Polarity":T38, "Kernel Size":u32, "Width":u32, "Minimum Edge Strength":sgl, "Interpolation Type":enum32{"Zero Order", "Bilinear", "Quadratic", "Cubic", "Bilinear Fixed"}, "Data Processing Method":enum32{"Average", "Median"}}
  T38 = typedef "Edge Polarity.ctl" = u32
  T39 = typedef "IMAQ Line" = cluster{"Start X":i32, "Start Y":i32, "End X":i32, "End Y":i32}
  T40 = cluster{"Settings (Clamp (Rake) 1)":cluster{"Contrast":i32, "Filter width":i32, "Steepness":i32, "Subsampling Ratio":u32, "Show Search Area":bool, "Show Search Lines":bool, "Show Edges Found":bool, "Show Result":bool}, "Options (Find Straight Edge 1)":cluster{"Search Direction":u32, "Edge Options":T37, "Show Search Area":bool, "Show Search Lines":bool, "Show Edges Found":bool, "Show Result":bool, "Search Area Color":u32, "Search Lines Color":u32, "Edge Locations Color":u32, "Result Color":u32, "Overlay Group Name":string}, "相对距离设定":cluster{"上限":dbl, "下限":dbl}, "衬丝直径设定":cluster{"上限":dbl, "下限":dbl}, "保护套直径设定":cluster{"上限":dbl, "下限":dbl}, "Edge Options (Edge Detector 1)":cluster{"Edge Polarity":u32, "Kernel Size":u32, "Width":u32, "Minimum Edge Strength":sgl, "Interpolation Type":enum32{"Zero Order", "Bilinear", "Quadratic", "Cubic", "Bilinear Fixed"}, "Data Processing Method":enum32{"Average", "Median"}}, "保护套标准位置":T39}
  T41 = cluster{"find straight edge Rectangle":T31, "Line 1":T39, "clamp Rectangle ":T31, "Line 2":T39}
  T42 = cluster{"位置1":cluster{"上限":dbl, "下限":dbl}, "位置2":cluster{"上限":dbl, "下限":dbl}, "位置3":cluster{"上限":dbl, "下限":dbl}, "位置4":cluster{"上限":dbl, "下限":dbl}, "位置5":cluster{"上限":dbl, "下限":dbl}, "位置6":cluster{"上限":dbl, "下限":dbl}, "位置7":cluster{"上限":dbl, "下限":dbl}, "位置8":cluster{"上限":dbl, "下限":dbl}, "位置9":cluster{"上限":dbl, "下限":dbl}, "位置10":cluster{"上限":dbl, "下限":dbl}}
  T43 = typedef "Straight Edge Options.ctl" = cluster{"Number of Lines":i32, "Type":T44, "Min. Score":dbl, "Max. Score":dbl, "Orientation":dbl, "Angle Range":dbl, "Angle Tolerance":dbl, "Step Size":u32, "Min. SNR (db)":dbl, "Min. Points (%)":dbl, "Hough Iterations":i32}
  T44 = typedef "Straight Edge Process.ctl" = enum32{"First Edge Rake", "Best Edge Rake", "Hough Edge Rake", "First Edge Projection", "Best Edge Projection"}
  T45 = cluster{"Rectangle":T31, "Find Straight Edge 1":T43, "Process (Edge Detector 1)":enum16{"Get First Edge", "Get First + Last Edge", "Get All Edges", "Get Best Edge"}, "Edge Options (Edge Detector 1)":cluster{"Edge Polarity":u32, "Kernel Size":u32, "Width":u32, "Minimum Edge Strength":sgl, "Interpolation Type":enum32{"Zero Order", "Bilinear", "Quadratic", "Cubic", "Bilinear Fixed"}, "Data Processing Method":enum32{"Average", "Median"}}, "Options (Find Straight Edge 1)":cluster{"Search Direction":u32, "Edge Options":T37, "Show Search Area":bool, "Show Search Lines":bool, "Show Edges Found":bool, "Show Result":bool, "Search Area Color":u32, "Search Lines Color":u32, "Edge Locations Color":u32, "Result Color":u32, "Overlay Group Name":string}, "Parameters (Pattern Matching 1)":cluster{"Number of Matches Requested":i32, "Minimum Match Score":sgl, "Angle Ranges":cluster{"Start Angle":sgl, "End Angle":sgl}[]}, "Template File Path (Pattern Matching 1)":path}
  T46 = cluster{"相机1启动":bool, "相机1反馈":bool, "相机2启动":bool, "相机2反馈":bool, "相机3启动":bool, "相机3反馈":bool, "相机4启动":bool, "相机4反馈":bool, "DI 8":bool, "DI 9":bool, "DI 10":bool, "DI 11":bool, "DI 12":bool, "DI 13":bool, "DI 14":bool, "DI 15":bool, "相机5启动":bool, "相机5反馈":bool, "相机6启动":bool, "相机6反馈":bool}
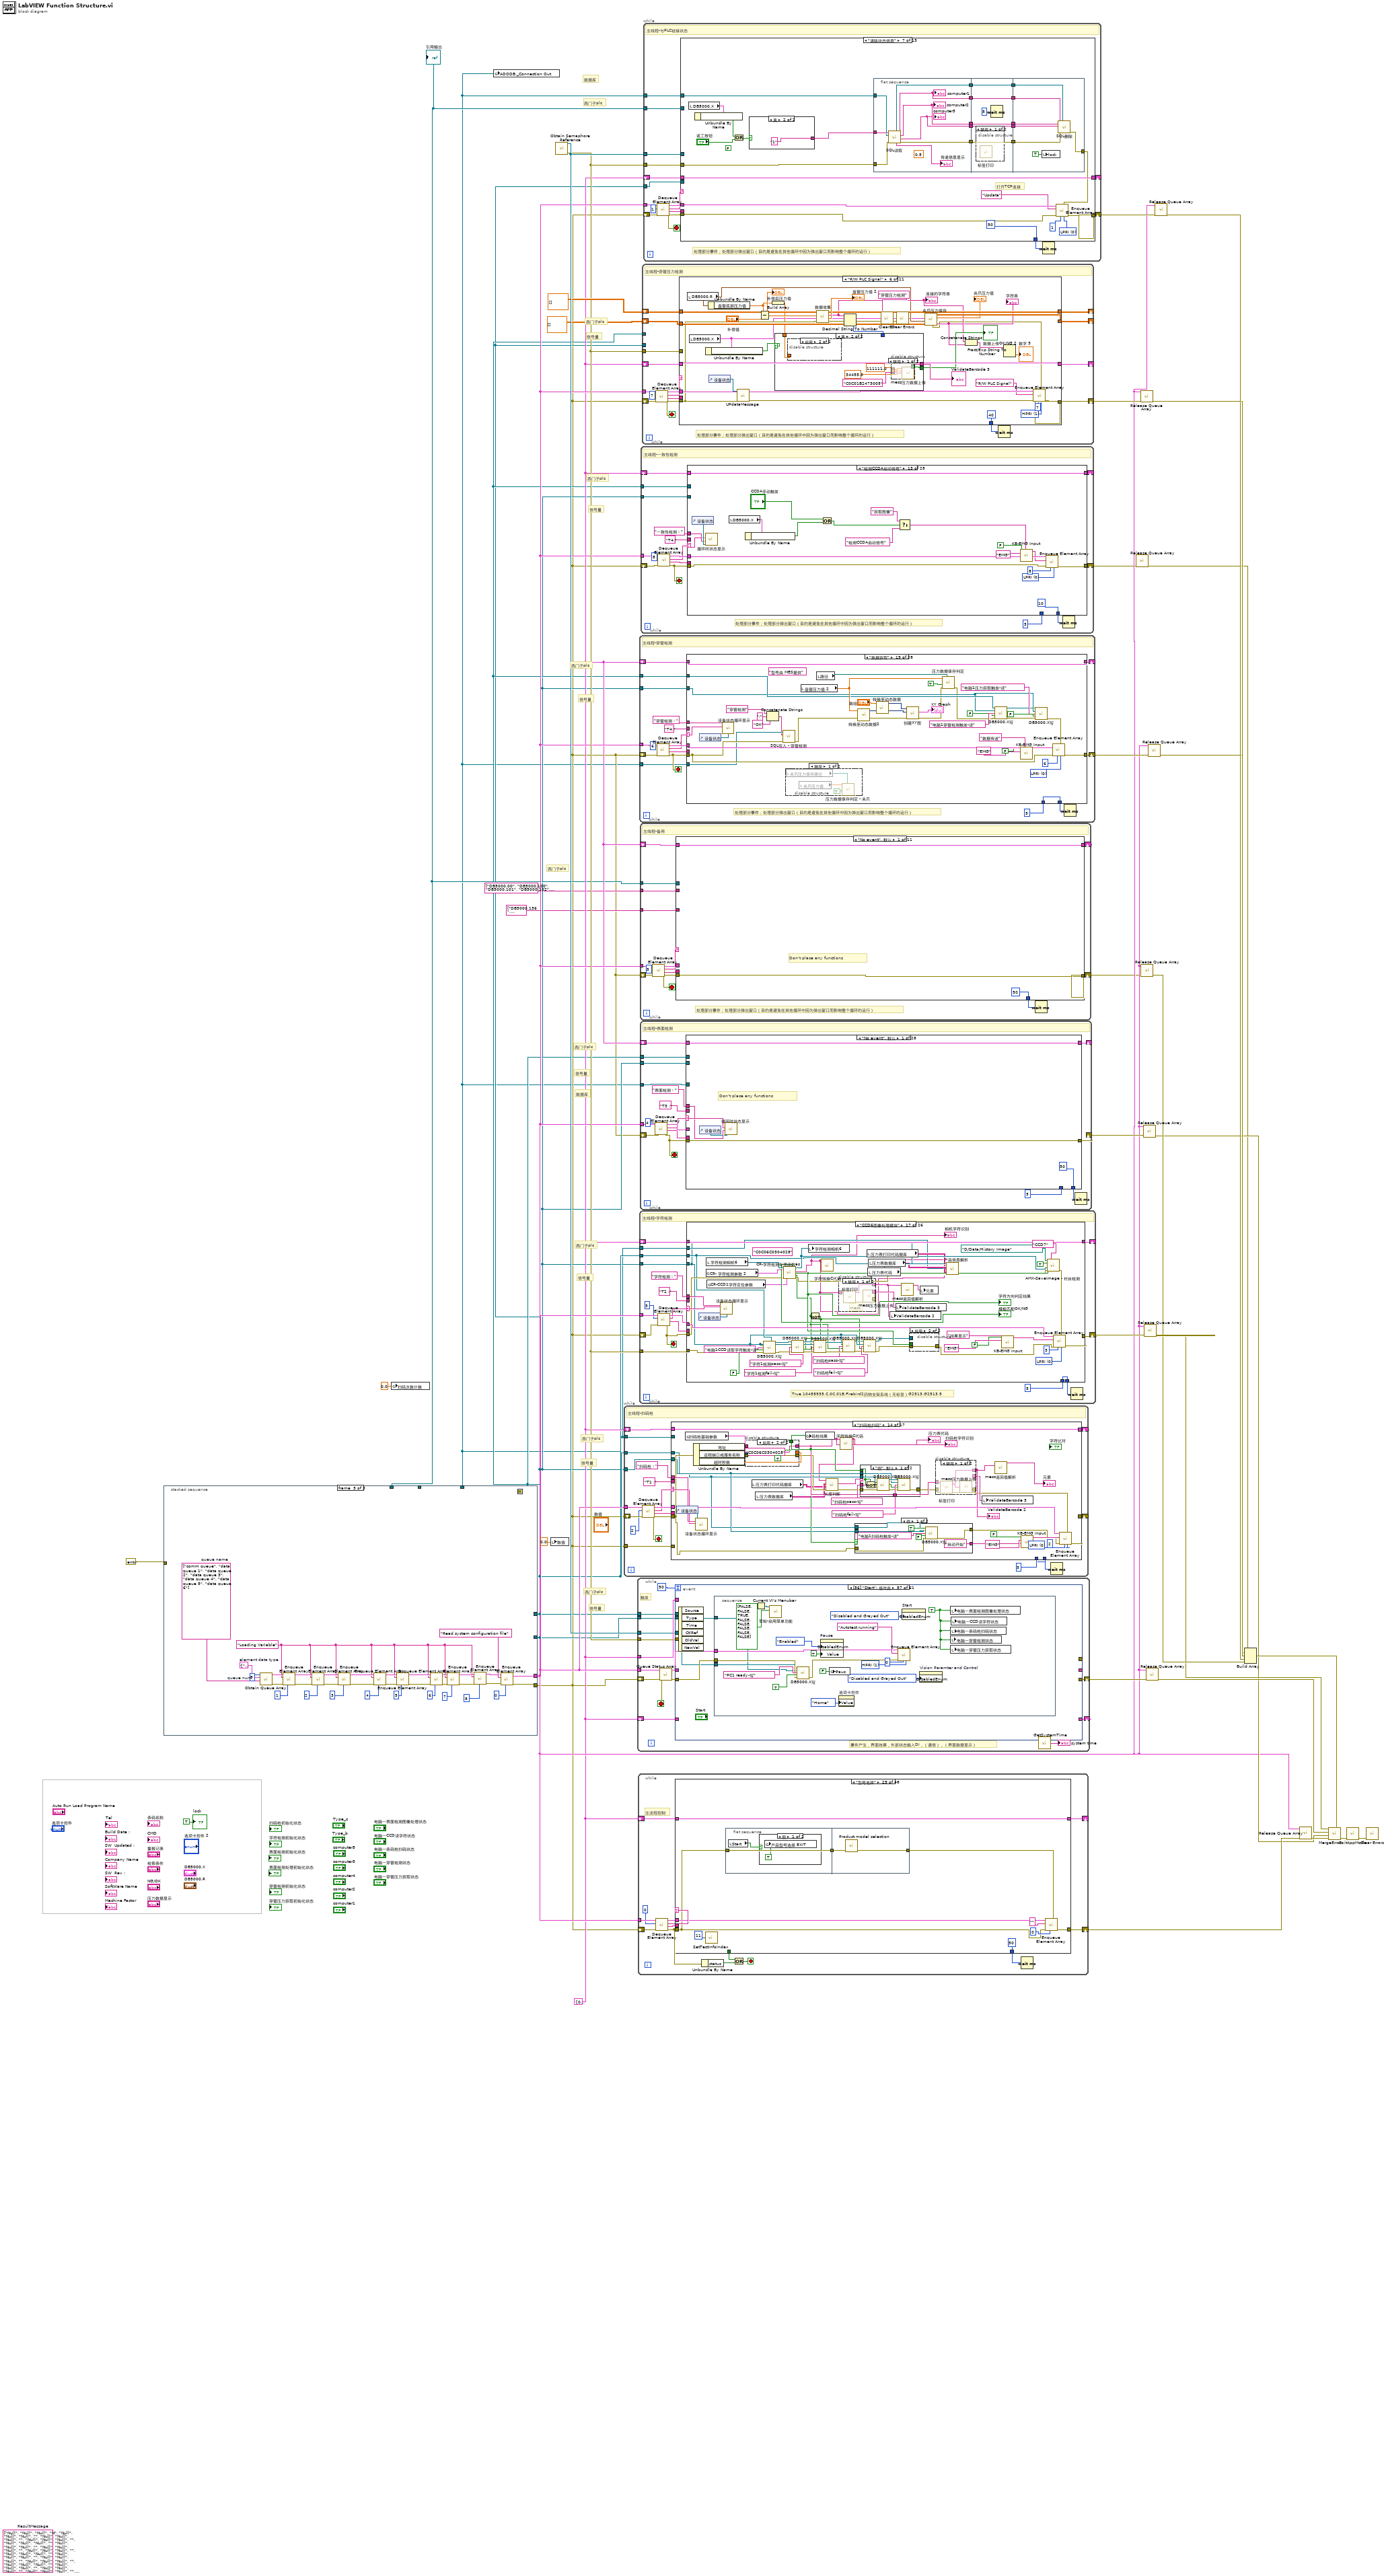
[diagram p0: block diagram]
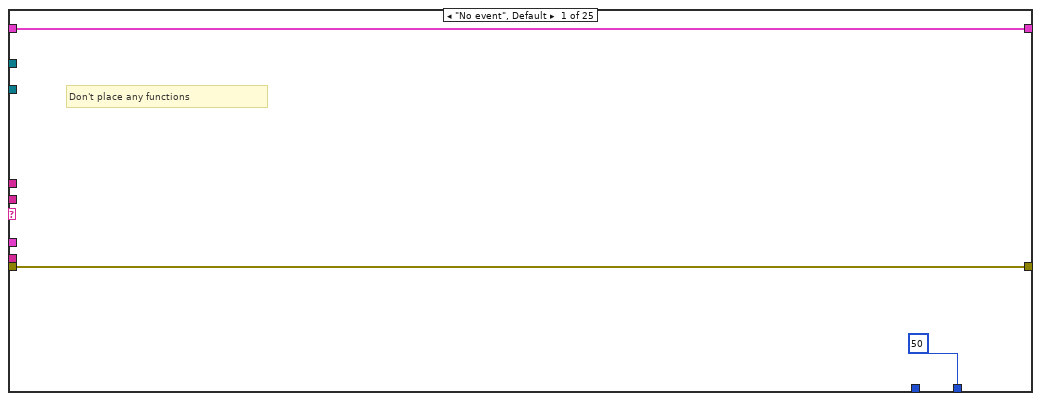
[diagram p2: hidden frame]
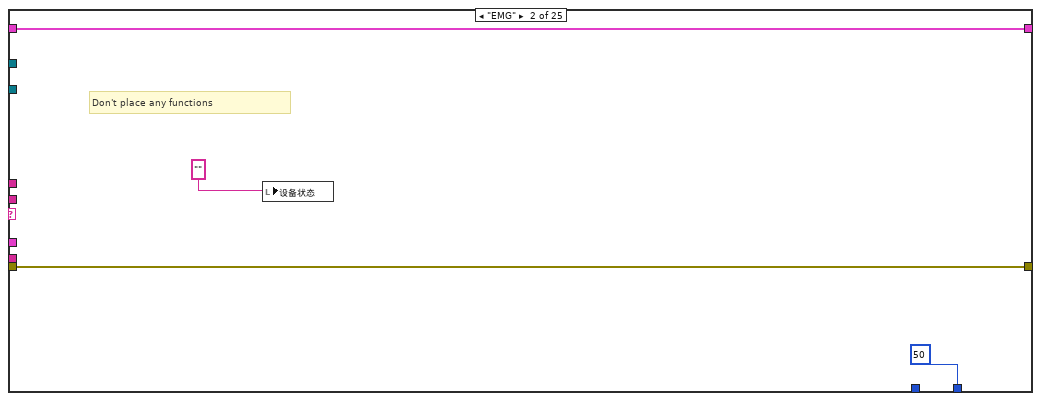
[diagram p3: hidden frame]
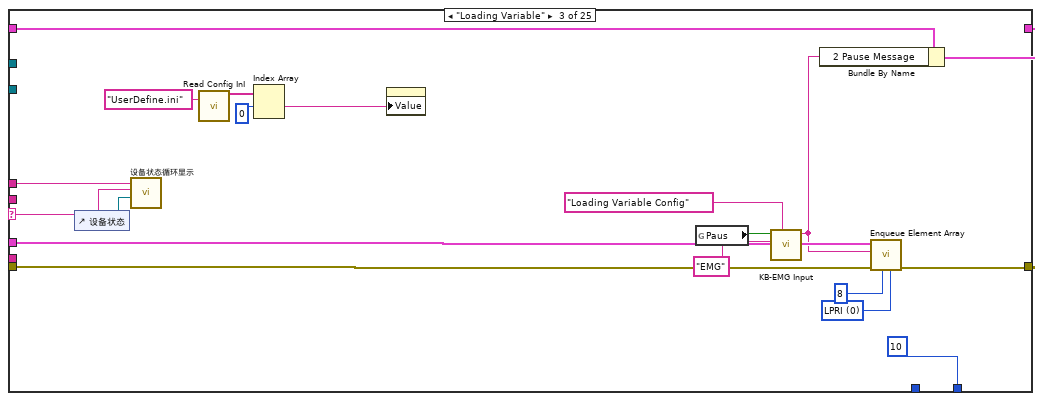
[diagram p4: hidden frame]
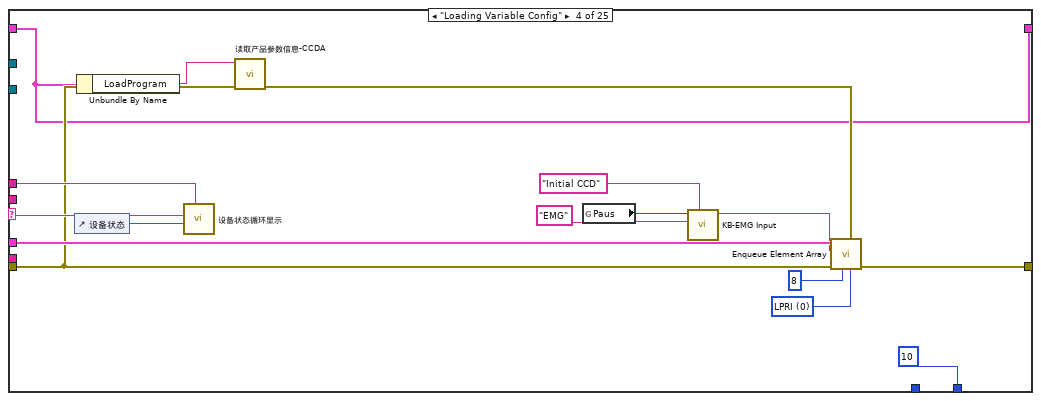
[diagram p5: hidden frame]
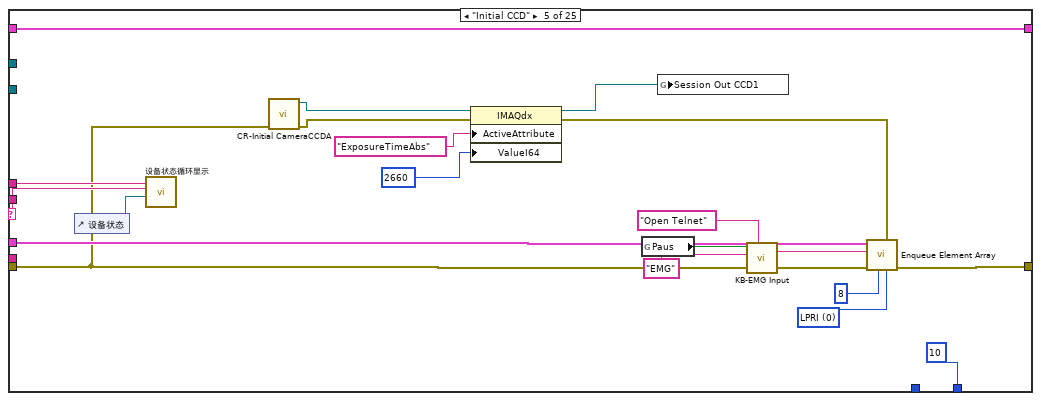
[diagram p6: hidden frame]
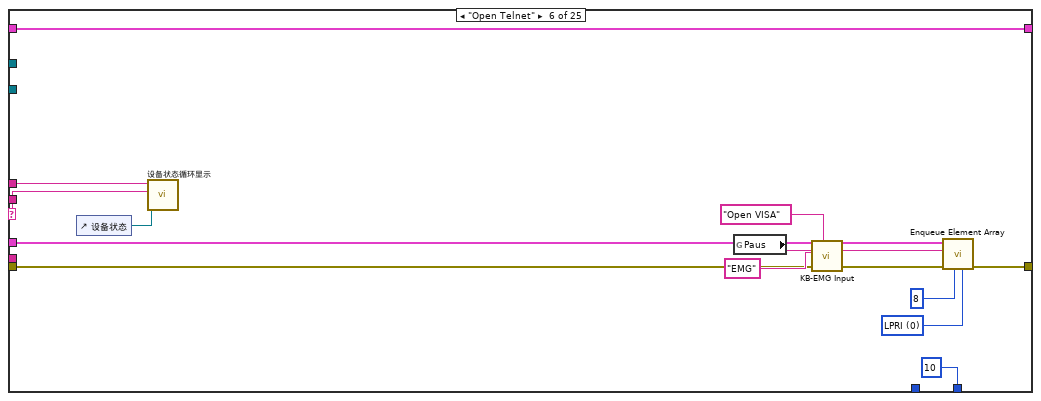
[diagram p7: hidden frame]
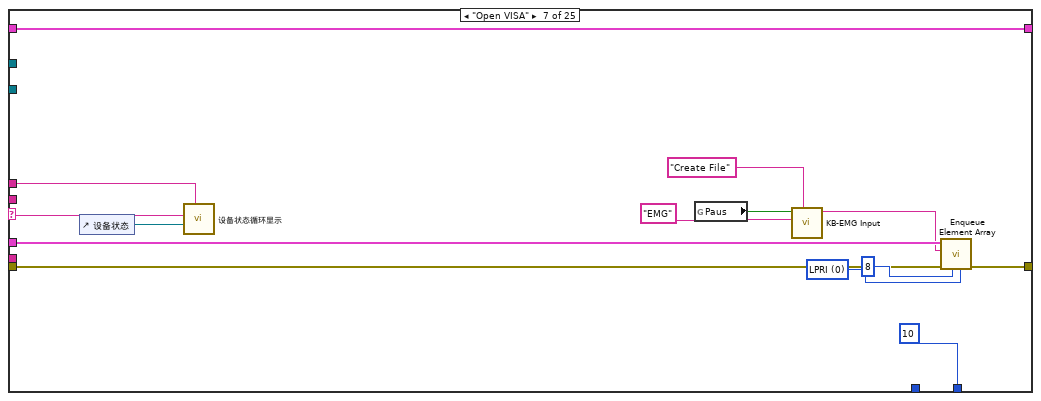
[diagram p8: hidden frame]
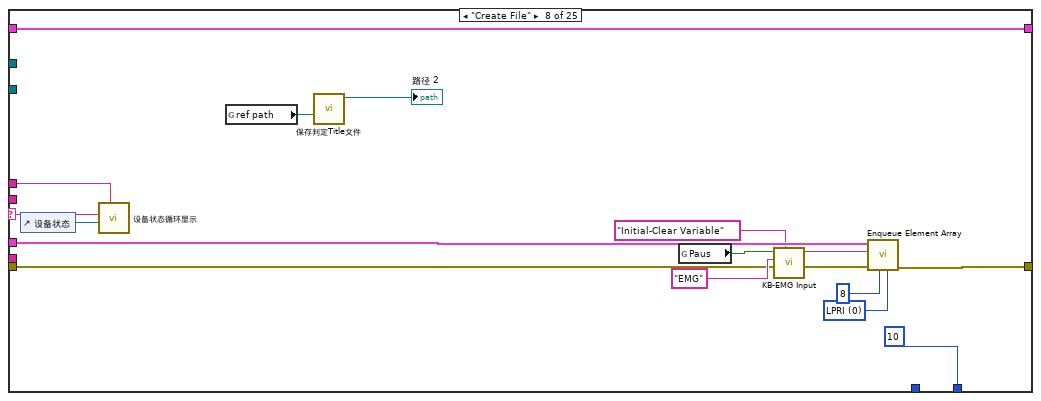
[diagram p9: hidden frame]
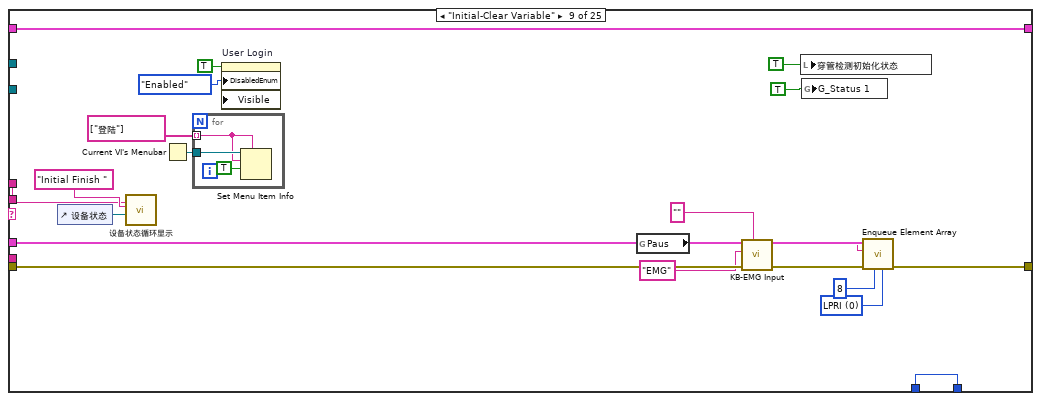
[diagram p10: hidden frame]
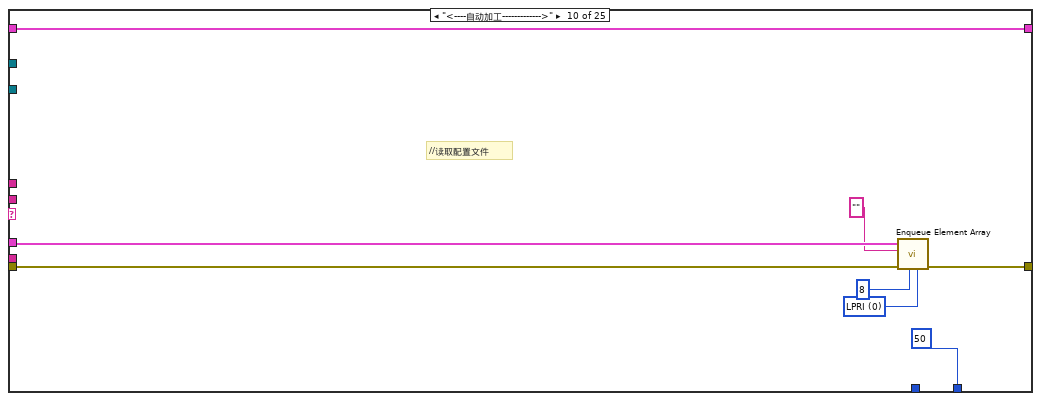
[diagram p11: hidden frame]
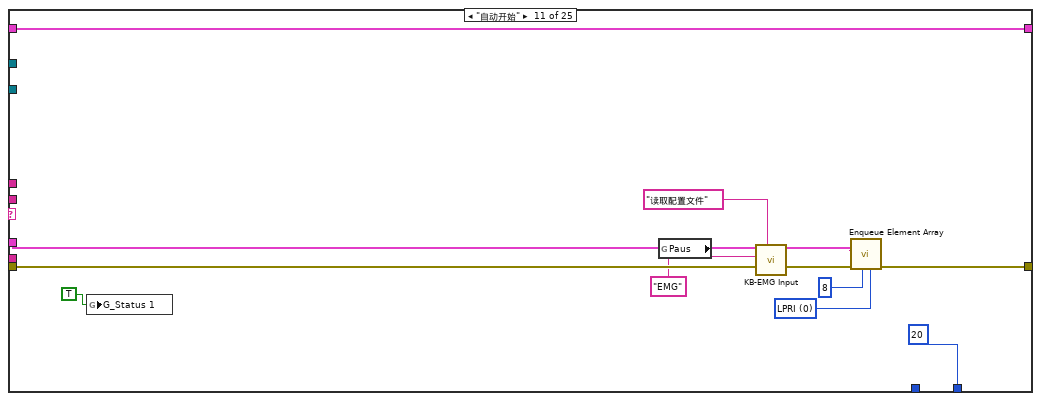
[diagram p12: hidden frame]
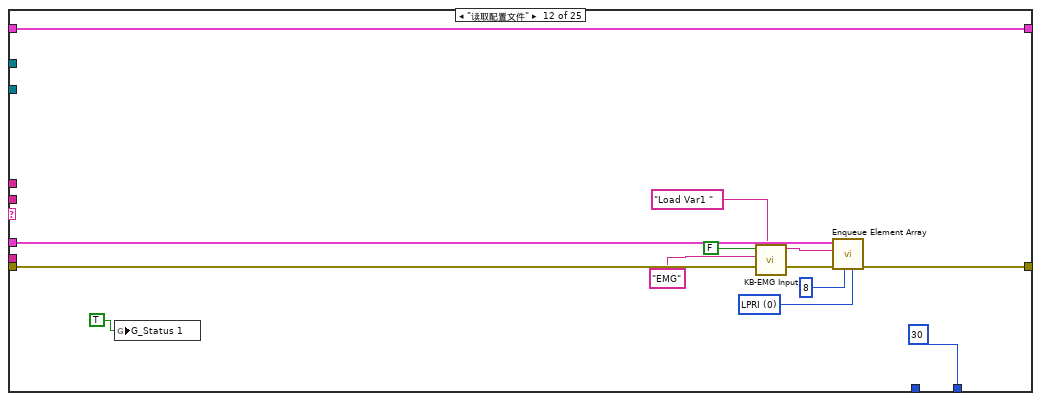
[diagram p13: hidden frame]
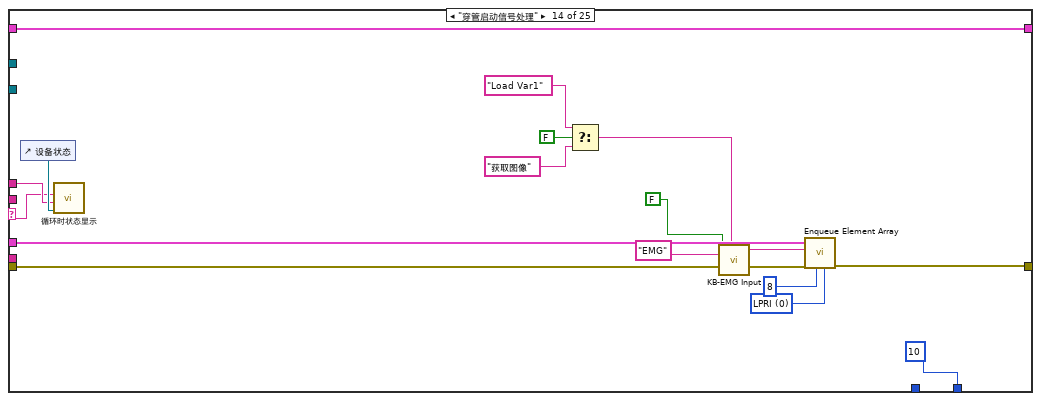
[diagram p14: hidden frame]
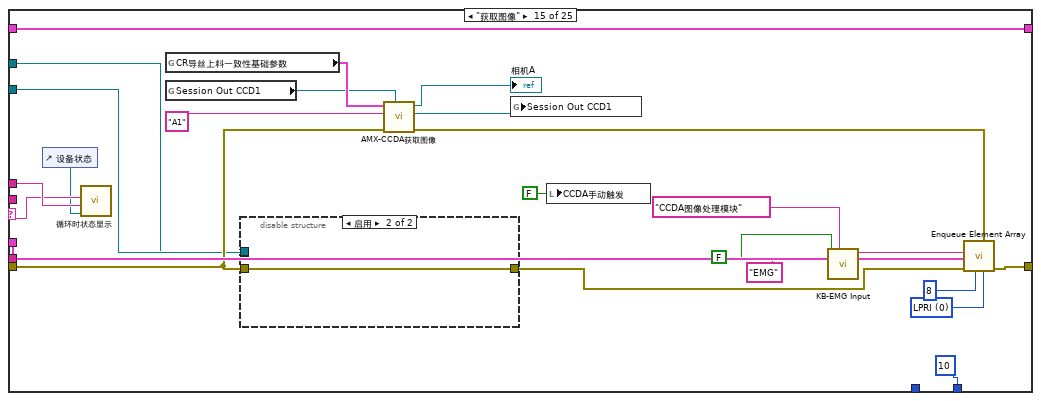
[diagram p15: hidden frame]
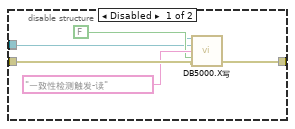
[diagram p16: hidden frame]
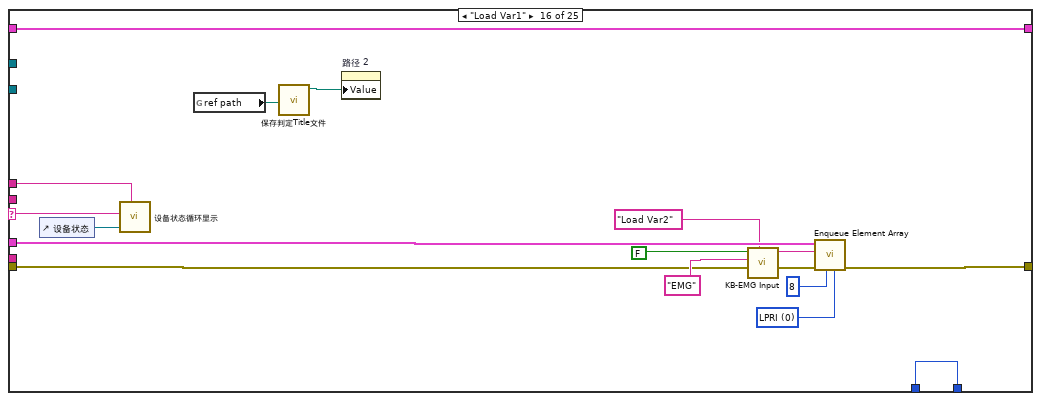
[diagram p17: hidden frame]
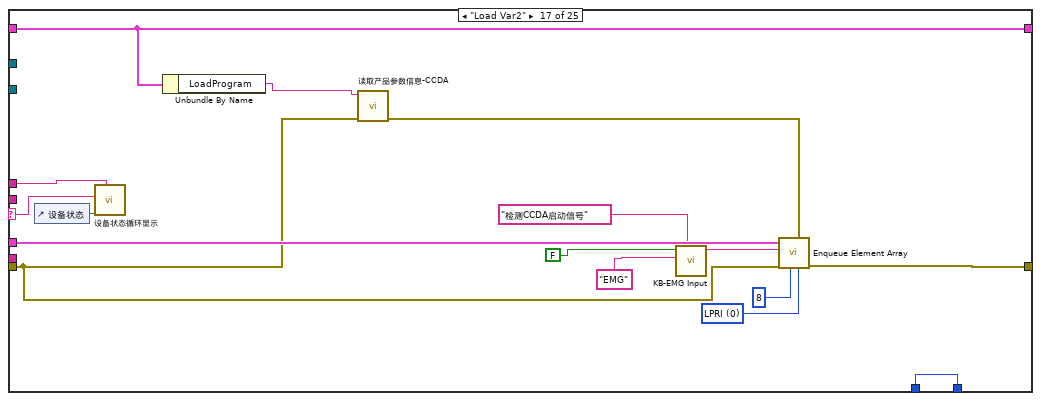
[diagram p18: hidden frame]
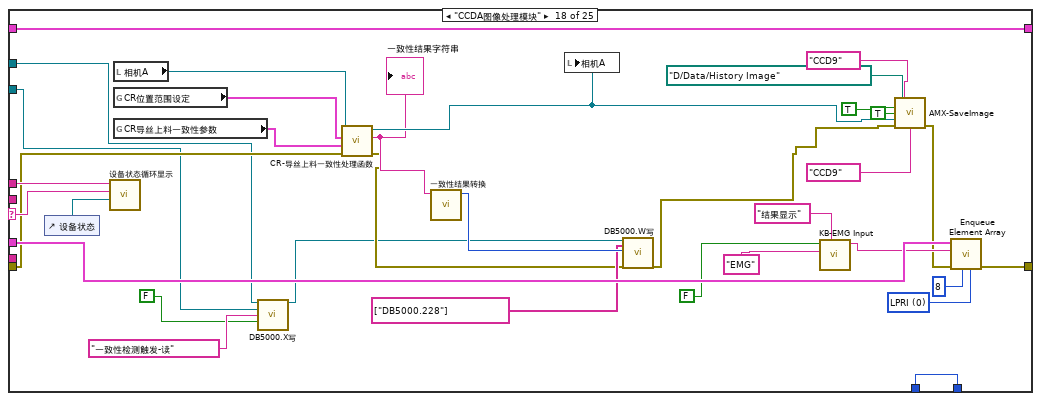
[diagram p19: hidden frame]
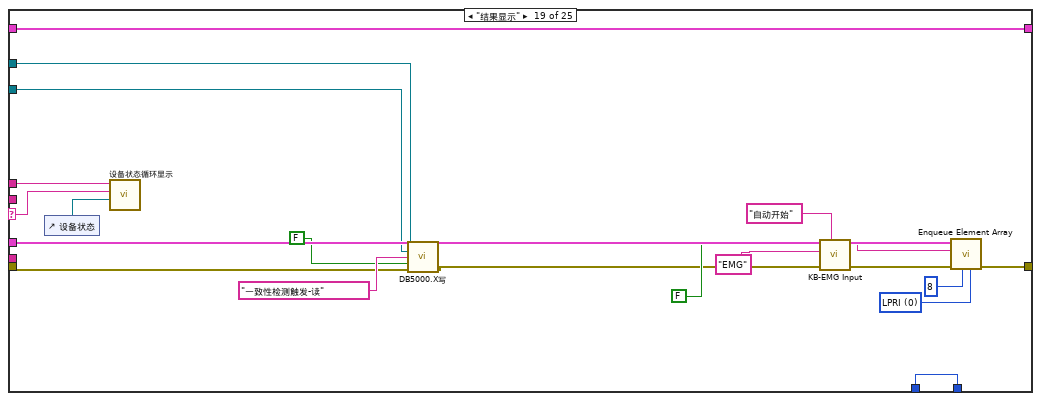
[diagram p20: hidden frame]
diagram:
  (unwired) string[][] [["Null", "Null", "Null", "N"], ["Null", "Null", "Null", ""], ["Null", "Null", "Null", ""], ["Null", "Null", "Null", ""], ["Null", "Null", "Null", ""], ["Null", "Null", "Null", ""], ["Null", "Null", "Null", ""], ["Null", "Null", "Null", ""], ["Null", "Null", "Null", ""], ["Null", "Null", "Null", ""], ["Null", "Null", "Null", ""], ["Null", "Null", "Null", ""], ["Null", "Null", "Null", ""], ["Null", "Null", "Null", ""], ["Null", "Null", "Null", ""], ["Null", "Null", "Null", ""], ["Null", "Null", "Null", ""], ["Null", "Null", "Null", ""], ["Null", "Null", "Null", ""], ["Null", "Null", "Null", ""], ["Null", "Null", "Null", ""], ["Null", "Null", "Null", ""], ["Null", "Null", "Null", ""], ["Null", "Null", "Null", ""], ["Null", "Null", "Null", ""], ["Null", "Null", "Null", ""], ["Null", "Null", "Null", ""], ["Null", "Null", "Null", ""], ["Null", "Null", "Null", ""], ["Null", "Null", "Null", ""], ["Null", "Null", "Null", "N"]]  # ResultMessage
  w14 = T21 {"index"=0, "this vi"=refnum, "step"={"test step"=[], "step status"=[], "step index"=0}, "用户登录"={"admin"={"用户名"=[], "密码"=[]}, "engineer"={"用户名"=[], "密码"=[]}, "operator"={"用户名"=[], "密码"=[]}}, "用户权限"=0, "error out"={"status"=FALSE, "code"=0, "source"=""}, "AllStepNumber"=0, "Run ErrNumber"="", "LoadProgram"="", "TotalNumber"="", "PassNumber"="", "FailNumber"="", "Start Time"="", "2 Pause Message"="", "3 Pause Message"="", "4 Pause Message"=""} ("parameter buffer")
  # "数据库"
  # "信号量"
  # "西门子plc"
  # "信号量"
  # "西门子plc"
  # "信号量"
  # "西门子plc"
  # "信号量"
  # "西门子plc"
  # "信号量"
  # "西门子plc"
  # "信号量"
  # "信号量"
  # "西门子plc"
  # "西门子plc"
  # "西门子plc"
  # "西门子plc"
  # "数据库"
  n1 = stacked-sequence {
    seq-local: [_ w96 _] -> [_ _ _]
    tunnel: [_ _ w132] -> w2
    tunnel: [_ _ w131] -> w15
    tunnel: [_ w95 _] -> _
    tunnel: errorcluster {"status"=FALSE, "code"=0, "source"=""} ("error in (no error)") -> [_ w83 _]
    tunnel: [_ w89 _] -> w1
    tunnel: [_ w84 _] -> w9
    tunnel: [_ w84 _] -> w8
    tunnel: [_ w81 _] -> w7
    frame #0 {
      w41 = "" ("相机字符识别")
      w40 = "" ("电脑一工单数量")
      w42 = FALSE ("电脑一表面检测图像处理状态")
      w43 = "" ("电脑一序号")
      w47 = FALSE ("扫码枪初始化状态")
      w45 = FALSE
      w48 = T15 FALSE ("Pause")
      n2 = shared-variable "我的电脑\\网络共享变量库.lvlib\\电脑一工单数量"(w40) -> ()  [unwired: 1 in, 1 out]
      n3 = local write "相机字符识别"(w41) -> ()
      n4 = local write "扫码枪字符识别"(w41) -> ()
      n5 = shared-variable "我的电脑\\网络共享变量库.lvlib\\电脑一检测信息"(w40) -> ()  [unwired: 1 in, 1 out]
      n6 = local write "传递信息显示"("" ("传递信息显示")) -> ()
      n7 = shared-variable "我的电脑\\网络共享变量库.lvlib\\电脑一序号"(w43) -> ()  [unwired: 1 in, 1 out]
      n8 = shared-variable "我的电脑\\网络共享变量库.lvlib\\电脑一模板类型"(w43) -> ()  [unwired: 1 in, 1 out]
      n9 = shared-variable "我的电脑\\网络共享变量库.lvlib\\电脑一新返工1"(w43) -> ()  [unwired: 1 in, 1 out]
      n10 = shared-variable "我的电脑\\网络共享变量库.lvlib\\电脑一工单号"(w43) -> ()  [unwired: 1 in, 1 out]
      n11 = local write "扫码枪初始化状态"(w47) -> ()
      n12 = local write "字符检测初始化状态"(w47) -> ()
      n13 = local write "表面检测初始化状态"(w47) -> ()
      n14 = local write "穿管检测初始化状态"(w47) -> ()
      n15 = local write "表面检测处理初始化状态"(w47) -> ()
      n16 = local write "穿管压力获取初始化状态"(w47) -> ()
      n17 = disable-structure shown="启用" {
        frame Disabled {
          n18 = for {
            N: 40 -> [_]
            tunnel: [w74] -> w63 mode=indexing
            tunnel: [w73] -> w61 mode=indexing
            tunnel: [w72] -> w62 mode=indexing
            tunnel: [w67] -> _ mode=indexing
            tunnel: [w66] -> _ mode=indexing
            tunnel: [w65] -> _ mode=indexing
            i -> [w75]
            n19 = Number To Decimal String(number=w75) -> (decimal integer string=w68:string)  [unwired: 1 in]
            n20 = Concatenate Strings(w68, "3" ("字符串")) -> (w67:string)
            n21 = Concatenate Strings(w68, "4" ("字符串")) -> (w66:string)
            n22 = Concatenate Strings(w68, "5" ("字符串")) -> (w65:string)
            n23 = call "IMAQ Create"("Image Name"=w67) -> ("New Image"=w74:T1)  [unwired: 4 in, 1 out]
            n24 = call "IMAQ Create"("Image Name"=w66) -> ("New Image"=w72:T1)  [unwired: 4 in, 1 out]
            n25 = call "IMAQ Create"("Image Name"=w65) -> ("New Image"=w73:T1)  [unwired: 4 in, 1 out]
          }
          "数组 2" <- w63
          n26 = global write "Global System.vi" "CCD3"(w63) -> ()
          n27 = global write "Global System.vi" "CCD4"(w62) -> ()
          n28 = global write "Global System.vi" "CCD5"(w61) -> ()
        }
        frame Enabled {
        }
      }
      n29 = local write "电脑一穿管检测状态"(w42) -> ()
      n30 = local write "电脑一表面检测图像处理状态"(w42) -> ()
      n31 = local write "电脑一条码枪扫码状态"(w42) -> ()
      n32 = local write "电脑一穿管压力获取状态"(w42) -> ()
      n33 = local write "电脑一CCD读字符状态"(w42) -> ()
      n34 = disable-structure shown="禁用" {
        frame Disabled {
          n35 = shared-variable "我的电脑\\PLC-OPC.lvlib\\PLC初始化信号"() -> ()  [unwired: 1 in, 2 out]
          n36 = call "SQL-选择清空数据库.vi"("computer1"=TRUE ("computer 4"), "computer 2"=TRUE ("computer 4"), "computer 3"=TRUE ("computer 4"), "computer 4"=TRUE, "computer 5"=TRUE) -> ()  [unwired: 13 in, 2 out]
        }
        frame Enabled {
        }
      }
      n37 = local write "字符比对"(FALSE ("字符比对")) -> ()
      n38 = global write "Global System.vi" "test info C"(string[] ["Read system configuration files", "Read user configuration file"]) -> ()
      n39 = local write "字符检测触发"(w45) -> ()
      n40 = local write "表面检测触发"(w45) -> ()
      n41 = local write "扫码枪触发"(w45) -> ()
      n42 = local write "穿管触发"(w45) -> ()
      n43 = property on="选项卡控件" class="TabCtl (严格)"("Value"=T2."Home" ("选项卡控件")) -> ()  [unwired: 2 in, 2 out]
      n44 = Concatenate Strings("Start....." ("Process 2"), "\r\n") -> (→"设备状态":string)
      n45 = global write "Global System.vi" "CCD1 Trigle Signal"(FALSE ("CCD1 Trigle Signal")) -> ()
      n46 = global write "Global System.vi" "EMG"(FALSE ("EMG")) -> ()
      n47 = global write "Global System.vi" "产品型号选择 EXIT"(FALSE ("EMG")) -> ()
      n48 = global write "Global System.vi" "EMG"(FALSE ("EMG")) -> ()
      n49 = global write "Trige.vi" "Trigle_3"(TRUE ("Trigle_3")) -> ()
      n50 = global write "Global System.vi" "G_Status 1"(TRUE ("G_Status 1")) -> ()
      n51 = global write "Global System.vi" "G_Status 2"(TRUE ("G_Status 1")) -> ()
      n52 = local write "Pause"(w48) -> ()
      n53 = local write "Start"(T14 TRUE ("Start")) -> ()
      n54 = global write "Global System.vi" "Paus"(w48) -> ()
    }
    frame #1 {
      (unwired) T22."Enabled" ("禁用")
      w113 = T22."Disabled and Grayed Out" ("禁用")
      n55 = control-ref of="Start"() -> (w112:refnum<vi>)
      n56 = control-ref of="Pause"() -> (w111:refnum<vi>)
      n57 = control-ref of="Stop"() -> (w110:refnum<vi>)
      n58 = control-ref of="Data and Run Information"() -> (w109:refnum<vi>)
      n59 = control-ref of="Machine Inforamtion"() -> (w108:refnum<vi>)
      n60 = control-ref of="Machine Paramter and Control"() -> (w107:refnum<vi>)
      n61 = control-ref of="Vision Paramter and Control"() -> (w106:refnum<vi>)
      n62 = control-ref of="Machine Alarm Histroy"() -> (w105:refnum<vi>)
      n63 = control-ref of="Open Excel File"() -> (w104:refnum<vi>)
      n64 = control-ref of="Open Image File"() -> (w98:refnum<vi>)
      n65 = Build Array(w112, w111, w110, w109, w108, w107, w106, w105, w104, w98) -> (w103:refnum<vi>[])
      n66 = control-ref of="User Login"() -> (w115:refnum<vi>)
      n67 = control-ref of="Home"() -> (w121:refnum<vi>)
      n68 = Build Array(w115) -> (w116:refnum<vi>[])
      n69 = Build Array(w121) -> (w120:refnum<vi>[])
      n70 = call <vilib>:"Obtain Semaphore Reference.vi"("error in (no error)"=w83) -> ("error out"=w82:errorcluster, "semaphore"=w81:T23)  [unwired: 4 in, 1 out]
      n71 = call "初始化SIEMENS.vi"("错误输入（无错误）"=w83) -> ("错误输出"=w88:errorcluster, "通讯状态"=→"通讯状态":bool, "gInitialSIEMENSS7"=w86:refnum<k24>)  [unwired: 8 in]
      n72 = call "军蚁-工具栏按钮操作.vi"("error in (no error)"=w83, "布尔"=FALSE, "禁用"=w113, "引用数组"=w116) -> ("error out"=w101:errorcluster)  [unwired: 7 in]
      n73 = call "军蚁-工具栏按钮操作.vi"("error in (no error)"=w83, "布尔"=TRUE, "禁用"=w113, "引用数组"=w103) -> ("error out"=w100:errorcluster)  [unwired: 7 in]
      n74 = call "军蚁-工具栏按钮操作.vi"("error in (no error)"=w83, "布尔"=TRUE, "禁用"=T22."Enabled", "引用数组"=w120) -> ("error out"=w102:errorcluster)  [unwired: 7 in]
      n75 = call "DB5000.X写 -AllRest.vi"("引用"=w86, "semaphore"=w81, "error in (no error)"=w88) -> ("引用输出"=w84:refnum<k24>, "error out"=w87:errorcluster)  [unwired: 11 in]
      n76 = Merge Errors(w102, w101, w100) -> (w99:errorcluster)
      n77 = call <userlib>:"ADO Connection Create.vi"("error in (no error)"=w83) -> ("error out"=w91:errorcluster, "ADODB._Connection Out"=w92:refnum<k7>)  [unwired: 9 in]
      n78 = call "BeforeStart.vi"("error in (no error)"=w99) -> ("error out"=w94:errorcluster, "ref path"=w95:path)  [unwired: 8 in, 1 out]
      n79 = Current VI's Menubar "当前VI菜单栏"() -> (w122:refnum<k9>)
      n80 = global write "Global System.vi" "ref path"(w95) -> ()
      n81 = call <userlib>:"ADO Connection Open.vi"("error in (no error)"=w91, "ConnectionString"="DSN=WCYL2;Driver=wcyljust ODBC 5.1 Driver;UID=root;PWD=root123;", "ADODB._Connection In"=w92) -> ("error out"=w90:errorcluster, "ADODB._Connection Out"=w89:refnum<k7>)  [unwired: 7 in]
      n82 = call "军蚁-禁用菜单功能.vi"("error in"=w94, "菜单引用"=w122) -> ("error Out"=w97:errorcluster)  [unwired: 9 in]
      n83 = Merge Errors(w97, w94, w90, w87, w82) -> (w96:errorcluster)
    }
    frame #2 {
      w123 = "Loading Variable" ("master data")
      w154 = string[] ["comm queue", "data queue 1", "data queue 2", "data queue 3", "data queue 4", "data queue 5", "data queue 6"]  # queue name
      w155 = 9  # queue num
      w156 = T24 {"master data"="", "priority"=0, "secondary data"=[]}  # element data type
      n84 = call "Obtain Queue Array.vi"("queue name"=w154, "element data type"=w156, "queue num"=w155) -> ("error out"=w148:errorcluster, "queue out"=w149:T25)  [unwired: 2 in, 1 out]
      n85 = call "Enqueue Element Array.vi"("queue index"=1, "error in"=w148, "master data"=w123, "queue in"=w149) -> ("error out"=w146:errorcluster, "queue out"=w147:T25)  [unwired: 6 in]
      n86 = call "Enqueue Element Array.vi"("queue index"=2, "error in"=w146, "master data"=w123, "queue in"=w147) -> ("error out"=w144:errorcluster, "queue out"=w145:T25)  [unwired: 6 in]
      n87 = call "Enqueue Element Array.vi"("queue index"=3, "error in"=w144, "master data"=w123, "queue in"=w145) -> ("error out"=w142:errorcluster, "queue out"=w143:T25)  [unwired: 6 in]
      n88 = call "Enqueue Element Array.vi"("queue index"=4, "error in"=w142, "master data"=w123, "queue in"=w143) -> ("error out"=w135:errorcluster, "queue out"=w136:T25)  [unwired: 6 in]
      n89 = call "Enqueue Element Array.vi"("queue index"=5, "error in"=w135, "master data"=w123, "queue in"=w136) -> ("error out"=w138:errorcluster, "queue out"=w137:T25)  [unwired: 6 in]
      n90 = call "Enqueue Element Array.vi"("queue index"=6, "error in"=w138, "master data"=w123, "queue in"=w137) -> ("error out"=w133:errorcluster, "queue out"=w134:T25)  [unwired: 6 in]
      n91 = call "Enqueue Element Array.vi"("queue index"=7, "error in"=w133, "master data"=w123, "queue in"=w134) -> ("error out"=w127:errorcluster, "queue out"=w129:T25)  [unwired: 6 in]
      n92 = call "Enqueue Element Array.vi"("queue index"=8, "error in"=w127, "master data"=w123, "queue in"=w129) -> ("error out"=w126:errorcluster, "queue out"=w128:T25)  [unwired: 6 in]
      n93 = call "Enqueue Element Array.vi"("queue index"=0, "error in"=w126, "master data"="Read system configuration file", "queue in"=w128) -> ("error out"=w132:errorcluster, "queue out"=w131:T25)  [unwired: 6 in]
    }
  }
  "引用输出" <- w9
  n94 = global write "Global System.vi" "扫码次数计数"(0.0 ("扫码次数计数")) -> ()
  n95 = global write "Global System.vi" "ADODB._Connection Out"(w1) -> ()
  n96 = local write "数值"(0.0 ("数值")) -> ()
  n97 = call <vilib>:"Obtain Semaphore Reference.vi"() -> ("error out"=w17:errorcluster, "semaphore"=w26:T23)  [unwired: 5 in, 1 out]
  n98 = while "While循环" {
    shift-right: [w174] -> _
    shift-left: w2 -> [w170]
    shift-right: [w171] -> _
    shift-left: w14 -> [w172]
    tunnel: w15 -> [w166]
    tunnel: w2 -> [w160]
    tunnel: w8 -> [w159]
    tunnel: w7 -> [w158]
    tunnel: w1 -> [w157]
    stop <- w165 stop-if-true
    # "主线程-扫码枪"
    n99 = call "Dequeue Element Array.vi"("queue in"=w166, "queue index"=2, "error in"=w170) -> ("queue out"=w169:T25, "master data"=w168:string, "secondary data"=w167:string[], "error out"=w165:errorcluster)  [unwired: 2 in, 1 out]
    n100 = case shown="\"扫码枪扫码\"" w168 {
      selector: w168 -> [w176 _ w196 w212 w226 w239 w253 w267 _ _ _ w331 w346 w382 w480 w568 _]
      tunnel: w169 -> [_ _ w206 w222 w236 w250 w264 w278 w297 w307 w321 w340 w351 w387 w485 w578 w583]
      tunnel: w165 -> [w178 w184 w195 w211 w225 w240 w254 w268 w292 w303 w310 w332 w344 w368 w466 w575 w580]
      tunnel: [w178 w184 w205 w221 w235 w249 w263 w277 w296 w306 w320 w339 w356 w392 w490 w577 w591] -> w174
      tunnel: [50 50 10 10 10 10 10 10 w293 50 20 10 w352 w388 w486 w567 50] -> w173
      tunnel: w172 -> [w179 w185 w188 w209 w224 w238 w252 w266 w285 w304 w312 w329 w343 w380 w478 w566 w589]
      tunnel: [w179 w185 w187 w209 w224 w238 w252 w266 w285 w304 w312 w328 w343 w380 w478 w566 w589] -> w171
      tunnel: w167 -> [_ _ _ _ _ _ _ _ _ _ _ _ _ _ _ _ _]
      tunnel: "扫码枪 : " -> [w175 _ w198 w214 w228 w246 w260 w274 w290 _ _ w334 w353 w389 w487 _ _]
      tunnel: "T1 :" -> [_ _ _ _ _ _ _ _ _ _ _ _ _ _ _ _ _]
      tunnel: 5 -> [_ _ _ _ _ _ _ _ w293 _ _ _ w352 w388 w486 w567 _]
      tunnel: w160 -> [_ _ _ _ _ _ _ _ _ _ _ _ _ _ _ _ _]
      tunnel: w159 -> [_ _ _ _ _ _ _ _ _ _ _ _ _ w366 w459 _ _]
      tunnel: w158 -> [_ _ _ _ _ _ _ _ _ _ _ _ _ w365 w458 _ _]
      tunnel: w157 -> [_ _ _ _ _ _ _ _ _ _ _ _ _ _ w451 _ _]
      frame "No event", Default {
        # "Don't place any functions"
        n101 = disable-structure shown="禁用" {
          disable-tunnel: w176 -> [w181 _]
          disable-tunnel: w175 -> [w180 _]
          frame Disabled {
            n102 = control-ref of="设备状态"() -> (w182:refnum<vi>)
            n103 = call "循环时状态显示.vi"("Str引用句柄"=w182, "cmd:"=w180, "新信息输入"=w181) -> ()  [unwired: 9 in]
          }
          frame Enabled {
          }
        }
      }
      frame "EMG" {
        # "Don't place any functions"
      }
      frame "Loading Variable" {
        w203 = u16 0 items=["HPRI"=1, "LPRI"=0] ("priority")
        n104 = control-ref of="设备状态"() -> (w202:refnum<vi>)
        n105 = call "设备状态循环显示.vi"("cmd:"=w198, "Str引用句柄"=w202, "新信息输入"=w196) -> ()  [unwired: 9 in]
        n106 = call "Read Config InI.vi"("名称或相对路径"="UserDefine.ini") -> ("ParamSet"=w189:string[])  [unwired: 14 in, 4 out]
        n107 = Index Array(array=w189, index #1=0 ("索引")) -> (element #1=w186:string)  [unwired: 1 in, 1 out]
        n108 = global read "Global System.vi" "ref path"() -> (w192:path)
        n109 = Build Path(base path=w192, name or relative path="Template Program" ("名称或相对路径")) -> (appended path=w194:path)
        n110 = Build Path(base path=w194, name or relative path=w186) -> ()  [unwired: 1 out]
        n111 = global read "Global System.vi" "Paus"() -> (w200:bool)
        n112 = Bundle By Name(cluster=w188, "LoadProgram"=w186) -> (w187:T21)
        n113 = call "KB-EMG Input.vi"("Other Message"="Loading Variable Config" ("Element 1"), "EMG Iput"="EMG", "Emg"=w200) -> ("String OutPut"=w197:string)  [unwired: 8 in]
        n114 = call "Enqueue Element Array.vi"("priority"=w203, "queue index"=2, "error in"=w195, "master data"=w197, "queue in"=w206) -> ("error out"=w205:errorcluster)  [unwired: 5 in, 1 out]
      }
      frame "Loading Variable Config" {
        w219 = u16 0 items=["HPRI"=1, "LPRI"=0] ("priority")
        n115 = control-ref of="设备状态"() -> (w218:refnum<vi>)
        n116 = call "设备状态循环显示.vi"("cmd:"=w214, "Str引用句柄"=w218, "新信息输入"=w212) -> ()  [unwired: 9 in]
        n117 = Unbundle By Name(w209) -> ("LoadProgram"=w208:string)
        n118 = call "读取扫码枪参数.vi"("错误输入（无错误）"=w211, "LoadProductName"=w208) -> ("错误输出"=w210:errorcluster)  [unwired: 9 in]
        n119 = global read "Global System.vi" "Paus"() -> (w216:bool)
        n120 = call "KB-EMG Input.vi"("Other Message"="Initial CCD" ("Element 1"), "EMG Iput"="EMG", "Emg"=w216) -> ("String OutPut"=w213:string)  [unwired: 8 in]
        n121 = call "Enqueue Element Array.vi"("priority"=w219, "device error in"=w210, "queue index"=2, "error in"=w211, "master data"=w213, "queue in"=w222) -> ("error out"=w221:errorcluster)  [unwired: 4 in, 1 out]
      }
      frame "Initial CCD" {
        w233 = u16 0 items=["HPRI"=1, "LPRI"=0] ("priority")
        n122 = control-ref of="设备状态"() -> (w232:refnum<vi>)
        n123 = call "设备状态循环显示.vi"("cmd:"=w228, "Str引用句柄"=w232, "新信息输入"=w226) -> ()  [unwired: 9 in]
        n124 = global read "Global System.vi" "Paus"() -> (w230:bool)
        n125 = call "KB-EMG Input.vi"("Other Message"="Open Telnet" ("Element 1"), "EMG Iput"="EMG", "Emg"=w230) -> ("String OutPut"=w227:string)  [unwired: 8 in]
        n126 = call "Enqueue Element Array.vi"("priority"=w233, "queue index"=2, "error in"=w225, "master data"=w227, "queue in"=w236) -> ("error out"=w235:errorcluster)  [unwired: 5 in, 1 out]
      }
      frame "Open Telnet" {
        w247 = u16 0 items=["HPRI"=1, "LPRI"=0] ("priority")
        n127 = control-ref of="设备状态"() -> (w245:refnum<vi>)
        n128 = call "设备状态循环显示.vi"("cmd:"=w246, "Str引用句柄"=w245, "新信息输入"=w239) -> ()  [unwired: 9 in]
        n129 = global read "Global System.vi" "Paus"() -> (w243:bool)
        n130 = call "KB-EMG Input.vi"("Other Message"="Open VISA" ("master data"), "EMG Iput"="EMG", "Emg"=w243) -> ("String OutPut"=w241:string)  [unwired: 8 in]
        n131 = call "Enqueue Element Array.vi"("priority"=w247, "queue index"=2, "error in"=w240, "master data"=w241, "queue in"=w250) -> ("error out"=w249:errorcluster)  [unwired: 5 in, 1 out]
      }
      frame "Open VISA" {
        w261 = u16 0 items=["HPRI"=1, "LPRI"=0] ("priority")
        n132 = control-ref of="设备状态"() -> (w259:refnum<vi>)
        n133 = call "设备状态循环显示.vi"("cmd:"=w260, "Str引用句柄"=w259, "新信息输入"=w253) -> ()  [unwired: 9 in]
        n134 = global read "Global System.vi" "Paus"() -> (w257:bool)
        n135 = call "KB-EMG Input.vi"("Other Message"="Create File" ("master data"), "EMG Iput"="EMG", "Emg"=w257) -> ("String OutPut"=w255:string)  [unwired: 8 in]
        n136 = call "Enqueue Element Array.vi"("priority"=w261, "queue index"=2, "error in"=w254, "master data"=w255, "queue in"=w264) -> ("error out"=w263:errorcluster)  [unwired: 5 in, 1 out]
      }
      frame "Create File" {
        w275 = u16 0 items=["HPRI"=1, "LPRI"=0] ("priority")
        n137 = control-ref of="设备状态"() -> (w273:refnum<vi>)
        n138 = call "设备状态循环显示.vi"("cmd:"=w274, "Str引用句柄"=w273, "新信息输入"=w267) -> ()  [unwired: 9 in]
        n139 = global read "Global System.vi" "Paus"() -> (w271:bool)
        n140 = call "KB-EMG Input.vi"("Other Message"="Initial-Clear Variable" ("master data"), "EMG Iput"="EMG", "Emg"=w271) -> ("String OutPut"=w269:string)  [unwired: 8 in]
        n141 = call "Enqueue Element Array.vi"("priority"=w275, "queue index"=2, "error in"=w268, "master data"=w269, "queue in"=w278) -> ("error out"=w277:errorcluster)  [unwired: 5 in, 1 out]
      }
      frame "Initial-Clear Variable" {
        w294 = u16 0 items=["HPRI"=1, "LPRI"=0] ("priority")
        n142 = control-ref of="设备状态"() -> (w291:refnum<vi>)
        n143 = call "设备状态循环显示.vi"("cmd:"=w290, "Str引用句柄"=w291, "新信息输入"="Initial Finish " ("字符串")) -> ()  [unwired: 9 in]
        n144 = Current VI's Menubar() -> (w283:refnum<k9>)
        n145 = for {
          tunnel: w283 -> [w300]
          tunnel: string[] ["登陆"] -> [w298] mode=indexing
          n146 = Set Menu Item Info(7:w298, 9:TRUE ("已启用"), 10:w298, 11:w300) -> ()  [unwired: 3 in, 2 out]
        }
        n147 = local write "扫码枪初始化状态"(TRUE ("扫码枪初始化状态")) -> ()
        n148 = global write "Global System.vi" "扫码次数计数"(0.0 ("扫码次数计数")) -> ()
        n149 = global read "Global System.vi" "Paus"() -> (w288:bool)
        n150 = call "KB-EMG Input.vi"("Other Message"="" ("Element 1"), "EMG Iput"="EMG", "Emg"=w288) -> ("String OutPut"=w286:string)  [unwired: 8 in]
        n151 = call "Enqueue Element Array.vi"("priority"=w294, "queue index"=2, "error in"=w292, "master data"=w286, "queue in"=w297) -> ("error out"=w296:errorcluster)  [unwired: 5 in, 1 out]
      }
      frame "<----自动加工------------->" {
        w301 = u16 0 items=["HPRI"=1, "LPRI"=0] ("priority")
        # "//读取配置文件"
        n152 = call "Enqueue Element Array.vi"("priority"=w301, "queue index"=2, "error in"=w303, "master data"="" ("Element 1"), "queue in"=w307) -> ("error out"=w306:errorcluster)  [unwired: 5 in, 1 out]
      }
      frame "自动开始" {
        w318 = u16 0 items=["HPRI"=1, "LPRI"=0] ("priority")
        n153 = global write "Global System.vi" "G_Status 2"(TRUE ("G_Status 1")) -> ()
        n154 = global write "Global System.vi" "码枪结果"(FALSE ("码枪结果")) -> ()
        n155 = global read "Global System.vi" "Paus"() -> (w315:bool)
        n156 = call "KB-EMG Input.vi"("Other Message"="读取网络变量" ("EMG Iput"), "EMG Iput"="EMG", "Emg"=w315) -> ("String OutPut"=w314:string)  [unwired: 8 in]
        n157 = call "Enqueue Element Array.vi"("priority"=w318, "queue index"=2, "error in"=w310, "master data"=w314, "queue in"=w321) -> ("error out"=w320:errorcluster)  [unwired: 5 in, 1 out]
      }
      frame "读取网络变量" {
        w337 = u16 0 items=["HPRI"=1, "LPRI"=0] ("priority")
        # "正面垫片PLC启动信号"
        n158 = control-ref of="设备状态"() -> (w335:refnum<vi>)
        n159 = local read "DB5000.X"() -> (w323:T4)
        n160 = call "循环时状态显示 - 3.vi"("Str引用句柄"=w335, "cmd:"=w334, "新信息输入"=w331) -> ()  [unwired: 9 in]
        n161 = Unbundle By Name(w323) -> ("电脑1扫码枪\n触发-读"=w322:bool)
        n162 = Or(x=w322, y="扫码枪触发") -> (x .or. y?=w325:bool)
        n163 = case shown="假" w325 {
          tunnel: ["读取网络变量" ("EMG Iput") " Load Var2" ("EMG Iput")] -> w326
          frame False {
          }
          frame True {
          }
        }
        n164 = call "KB-EMG Input.vi"("Other Message"=w326, "EMG Iput"="EMG", "Emg"=FALSE) -> ("String OutPut"=w327:string)  [unwired: 8 in]
        n165 = Bundle By Name(cluster=w329, "2 Pause Message"=w327) -> (w328:T21)
        n166 = call "Enqueue Element Array.vi"("priority"=w337, "queue index"=2, "error in"=w332, "master data"=w327, "queue in"=w340) -> ("error out"=w339:errorcluster)  [unwired: 5 in, 1 out]
      }
      frame "Load Var2" {
        w354 = u16 0 items=["HPRI"=1, "LPRI"=0] ("priority")
        n167 = control-ref of="设备状态"() -> (w347:refnum<vi>)
        n168 = call "设备状态循环显示.vi"("cmd:"=w353, "Str引用句柄"=w347, "新信息输入"=w346) -> ()  [unwired: 9 in]
        n169 = call "KB-EMG Input.vi"("Other Message"="扫码枪扫码" ("t"), "EMG Iput"="EMG", "Emg"=FALSE) -> ("String OutPut"=w345:string)  [unwired: 8 in]
        n170 = call "Enqueue Element Array.vi"("priority"=w354, "queue index"=2, "error in"=w344, "master data"=w345, "queue in"=w351) -> ("error out"=w356:errorcluster)  [unwired: 5 in, 1 out]
      }
      frame "扫码枪扫码" {
        w390 = u16 0 items=["HPRI"=1, "LPRI"=0] ("priority")
        n171 = control-ref of="设备状态"() -> (w383:refnum<vi>)
        n172 = global read "Global System.vi" "扫码枪基础参数"() -> (w379:T26)
        n173 = Unbundle By Name(w379) -> ("地址"=w378:string, "远程端口或服务名称"=w377:u16, "超时秒数"=w376:dbl)
        n174 = call "设备状态循环显示.vi"("cmd:"=w389, "Str引用句柄"=w383, "新信息输入"=w382) -> ()  [unwired: 9 in]
        n175 = disable-structure shown="启用" {
          disable-tunnel: w378 -> [w399 _]
          disable-tunnel: w377 -> [w398 _]
          disable-tunnel: w376 -> [w397 _]
          disable-tunnel: [w396 "C0C06C0304028" ("扫码枪字符识别")] -> w370
          disable-tunnel: [w395 TRUE ("码枪结果")] -> w369
          disable-tunnel: w368 -> [w394 w401]
          disable-tunnel: [w393 w401] -> w364
          frame Disabled {
            n176 = call "扫码触发.vi"("error in (no error)"=w394, "超时秒数"=w397, "远程端口或服务名称"=w398, "地址"=w399) -> ("error out 2"=w393:errorcluster, "结果"=w395:bool, "数据输出"=w396:string)  [unwired: 5 in]
          }
          frame Enabled {
          }
        }
        "扫码枪字符识别" <- w370
        n177 = local read "压力表打印代码据库"() -> (w362:string[][])
        n178 = local read "压力表数据库"() -> (w363:string[][])
        n179 = global write "Global System.vi" "码枪结果"(w369) -> ()
        n180 = call "字符转换C代码.vi"("扫码枪字符识别"=w370) -> ("子字符串 4"=w361:string)  [unwired: 10 in]
        "压力表代码" <- w361
        n181 = call "长度判断.vi"("error in (no error)"=w364, "压力打印代码据库"=w362, "压力表数据库"=w363, "输入元素"=w361) -> ("error out"=w360:errorcluster, "产品种类"=w357:string)  [unwired: 4 in, 2 out]
        n182 = case shown="假" w369 {
          tunnel: ["自动开始" ("t") "结果显示" ("t")] -> w384
          tunnel: w368 -> [w426 w431]
          tunnel: [w425 w431] -> w367
          tunnel: w366 -> [w424 _]
          tunnel: w365 -> [w423 _]
          frame False {
            n183 = call "DB5000.X写.vi"("引用"=w424, "启用延时"=TRUE, "semaphore"=w423, "地址名称"="电脑1扫码枪触发-读" ("组合框"), "value"=FALSE, "error in (no error)"=w426) -> ("error out"=w425:errorcluster)  [unwired: 8 in, 1 out]
          }
          frame True {
          }
        }
        n184 = case shown="\"假\", 默认" w357 {
          tunnel: "扫码枪pass-写" ("组合框") -> [w412 w418]
          tunnel: "扫码枪fail-写" ("组合框") -> [w411 w419]
          tunnel: w369 -> [w404 _]
          tunnel: w366 -> [w408 w417]
          tunnel: w365 -> [w407 w415]
          tunnel: w360 -> [w406 w422]
          tunnel: [w405 w420] -> w359
          frame "假", Default {
            n185 = Not(x=w404) -> (.not. x?=w403:bool)
            n186 = call "DB5000.X写.vi"("引用"=w408, "semaphore"=w407, "地址名称"=w412, "value"=w404, "error in (no error)"=w406) -> ("引用输出"=w409:refnum<k24>, "error out"=w410:errorcluster)  [unwired: 9 in]
            n187 = call "DB5000.X写.vi"("引用"=w409, "semaphore"=w407, "地址名称"=w411, "value"=w403, "error in (no error)"=w410) -> ("error out"=w405:errorcluster)  [unwired: 9 in, 1 out]
          }
          frame "数据匹配失败" {
            n188 = call "DB5000.X写.vi"("引用"=w417, "semaphore"=w415, "地址名称"=w418, "value"=FALSE, "error in (no error)"=w422) -> ("引用输出"=w416:refnum<k24>, "error out"=w421:errorcluster)  [unwired: 9 in]
            n189 = call "DB5000.X写.vi"("引用"=w416, "semaphore"=w415, "地址名称"=w419, "value"=TRUE, "error in (no error)"=w421) -> ("error out"=w420:errorcluster)  [unwired: 9 in, 1 out]
          }
        }
        n190 = disable-structure shown="禁用" {
          disable-tunnel: w359 -> [w433 w438]
          disable-tunnel: [w437 w438] -> w358
          disable-tunnel: [w436 _] -> w375
          disable-tunnel: w370 -> [w435 _]
          disable-tunnel: [w434 _] -> w373
          frame Disabled {
            n191 = call "标签打印.vi"("error in (no error)"=w433, "barcode"=w435) -> ("error out"=w437:errorcluster, "Print"=w436:string)  [unwired: 8 in]
            n192 = call "mess压力数据上传.vi"("barcode"=w435) -> ("ValidateBarcode"=w434:string)  [unwired: 12 in, 2 out]
          }
          frame Enabled {
          }
        }
        "ValidateBarcode 2" <- w375
        n193 = local write "ValidateBarcode 3"(w373) -> ()
        n194 = call "mess返回值解析.vi"("ValidateBarcode"=w375) -> ("元素"=→"元素":string)  [unwired: 10 in]
        n195 = call "KB-EMG Input.vi"("Other Message"=w384, "EMG Iput"="EMG", "Emg"=FALSE) -> ("String OutPut"=w381:string)  [unwired: 8 in]
        n196 = call "Enqueue Element Array.vi"("priority"=w390, "device error in"=w358, "queue index"=2, "error in"=w367, "master data"=w381, "queue in"=w387) -> ("error out"=w392:errorcluster)  [unwired: 4 in, 1 out]
      }
      frame "结果显示" {
        w444 = TRUE ("启用延时")
        w488 = u16 0 items=["HPRI"=1, "LPRI"=0] ("priority")
        n197 = control-ref of="设备状态"() -> (w481:refnum<vi>)
        n198 = local read "扫码枪字符识别"() -> (w440:string)
        n199 = local read "压力表数据库"() -> (w475:string[][])
        n200 = local read "压力表打印代码据库"() -> (w474:string[][])
        n201 = local read "压力表代码"() -> (w476:string)
        n202 = call "设备状态循环显示.vi"("cmd:"=w487, "Str引用句柄"=w481, "新信息输入"=w480) -> ()  [unwired: 9 in]
        n203 = call "DB5000.X写.vi"("引用"=w459, "启用延时"=TRUE, "semaphore"=w458, "地址名称"="电脑1扫码枪触发-读" ("组合框"), "value"=FALSE, "error in (no error)"=w466) -> ("error out"=w465:errorcluster)  [unwired: 8 in, 1 out]
        n204 = call "mess解析.vi"("ValidateBarcode"=w440, "压力表数据库"=w475, "压力打印代码据库"=w474, "输入元素"=w476, "error in (no error)"=w465) -> ("粗细料"=w471:string, "长短料"=w472:string, "压力表有无"=→"压力表有无 2":string, "衬丝口位置"=w473:string, "工单号"=w470:string, "产品种类"=w439:string, "工单数量"=w468:string, "压力表打印代码"=w467:string, "error out"=w461:errorcluster)  [unwired: 10 in, 4 out]
        "粗细料" <- w471
        n205 = local write "压力表打印代码"(w467) -> ()
        n206 = case shown="\"长料\"" w472 {
          tunnel: w461 -> [w536 w544]
          tunnel: w459 -> [w535 w543]
          tunnel: w458 -> [w534 w542]
          tunnel: [w537 w540] -> w457
          tunnel: [w532 w539] -> w447
          tunnel: w444 -> [w531 w538]
          frame "短料", Default {
            w532 = "短衬丝-写" ("组合框")
            n207 = call "DB5000.X写.vi"("引用"=w535, "启用延时"=w531, "semaphore"=w534, "地址名称"=w532, "value"=TRUE ("电脑1扫码枪\n触发-读"), "error in (no error)"=w536) -> ("error out"=w537:errorcluster)  [unwired: 8 in, 1 out]
          }
          frame "长料" {
            w539 = "长衬丝-写" ("组合框")
            n208 = call "DB5000.X写.vi"("引用"=w543, "启用延时"=w538, "semaphore"=w542, "地址名称"=w539, "value"=TRUE ("电脑1扫码枪\n触发-读"), "error in (no error)"=w544) -> ("error out"=w540:errorcluster)  [unwired: 8 in, 1 out]
          }
        }
        n209 = case shown="\"A\", 默认" w473 {
          tunnel: w459 -> [w551 w557 w565]
          tunnel: w458 -> [w550 w556 w564]
          tunnel: w461 -> [w548 w555 w562]
          tunnel: [w547 w554 w561] -> w462
          tunnel: [w546 w553 w560] -> w449
          tunnel: w444 -> [w545 w552 w559]
          frame "A", Default {
            w546 = "产品尺寸A-写" ("组合框")
            n210 = call "DB5000.X写.vi"("引用"=w551, "启用延时"=w545, "semaphore"=w550, "地址名称"=w546, "value"=TRUE ("电脑1扫码枪\n触发-读"), "error in (no error)"=w548) -> ("error out"=w547:errorcluster)  [unwired: 8 in, 1 out]
          }
          frame "B" {
            w553 = "产品尺寸B-写" ("组合框")
            n211 = call "DB5000.X写.vi"("引用"=w557, "启用延时"=w552, "semaphore"=w556, "地址名称"=w553, "value"=TRUE ("电脑1扫码枪\n触发-读"), "error in (no error)"=w555) -> ("error out"=w554:errorcluster)  [unwired: 8 in, 1 out]
          }
          frame "C" {
            w560 = "产品尺寸C-写" ("组合框")
            n212 = call "DB5000.X写.vi"("引用"=w565, "启用延时"=w559, "semaphore"=w564, "地址名称"=w560, "value"=TRUE ("电脑1扫码枪\n触发-读"), "error in (no error)"=w562) -> ("error out"=w561:errorcluster)  [unwired: 8 in, 1 out]
          }
        }
        n213 = case shown="\"粗料\", 默认" w471 {
          tunnel: w461 -> [w523 w530]
          tunnel: [w522 w526] -> w460
          tunnel: w459 -> [w520 w529]
          tunnel: w458 -> [w519 w528]
          tunnel: [w518 w525] -> w448
          tunnel: w444 -> [w517 w524]
          frame "粗料", Default {
            w518 = "粗料-写" ("组合框")
            n214 = call "DB5000.X写.vi"("引用"=w520, "启用延时"=w517, "semaphore"=w519, "地址名称"=w518, "value"=TRUE ("电脑1扫码枪\n触发-读"), "error in (no error)"=w523) -> ("error out"=w522:errorcluster)  [unwired: 8 in, 1 out]
          }
          frame "细料" {
            w525 = "细料-写" ("组合框")
            n215 = call "DB5000.X写.vi"("引用"=w529, "启用延时"=w524, "semaphore"=w528, "地址名称"=w525, "value"=TRUE ("电脑1扫码枪\n触发-读"), "error in (no error)"=w530) -> ("error out"=w526:errorcluster)  [unwired: 8 in, 1 out]
          }
        }
        n216 = disable-structure shown="启用" {
          disable-tunnel: [w491 w492] -> w441
          disable-tunnel: w439 -> [_ w495]
          frame Disabled {
            n217 = global read "Global System.vi" "码枪结果"() -> (w491:bool)
          }
          frame Enabled {
            n218 = Equal?(x=w495, y="数据匹配失败") -> (x = y?=w493:bool)
            n219 = Not(x=w493) -> (.not. x?=w492:bool)
          }
        }
        n220 = Format Date/Time String(time format string (%c)="%Y-%m-%d %H:%M:%S" ("时间格式字符串(%c)")) -> (date/time string=w442:string)  [unwired: 2 in]
        n221 = Build Array(w442, w449, w448, w447) -> (w446:string[])
        n222 = Concatenate Strings("字符一致性:", "OK" ("字符串")) -> (w453:string)
        n223 = Merge Errors(w462, w460, w457) -> (w456:errorcluster)
        n224 = case shown="真" w441 {
          tunnel: w470 -> [w501 w516]
          tunnel: w440 -> [w500 w515]
          tunnel: w456 -> [w498 w514]
          tunnel: [w497 w513] -> w455
          tunnel: w453 -> [w499 w512]
          tunnel: w468 -> [_ _]
          tunnel: w467 -> [_ _]
          tunnel: w439 -> [_ w509]
          tunnel: w451 -> [_ w508]
          frame False {
            n225 = disable-structure shown="启用" {
              disable-tunnel: w501 -> [w507 _]
              disable-tunnel: w500 -> [w506 _]
              disable-tunnel: w499 -> [w505 _]
              disable-tunnel: w498 -> [w504 _]
              disable-tunnel: [w503 _] -> w497
              frame Disabled {
                n226 = call "SQL写入 - NG.vi"("WorkNumber"=w507, "ProductNumber"=w506, "TestMessage"=w505, "ProssureType"="A1", "error in (no error)"=w504) -> ("error out"=w503:errorcluster)  [unwired: 9 in, 1 out]
              }
              frame Enabled {
              }
            }
            n227 = local write "字符比对"(FALSE ("字符比对")) -> ()
          }
          frame True {
            n228 = call "SQL写入.vi"("WorkNumber"=w516, "ProductNumber"=w515, "TestMessage"=w512, "ProssureType"=w509, "error in (no error)"=w514, "ADODB._Connection In"=w508, "Workorder"="1000") -> ("error out"=w513:errorcluster)  [unwired: 11 in, 1 out]
            n229 = local write "字符比对"(FALSE ("字符比对")) -> ()
          }
        }
        n230 = call-poly <vilib>:"Write Delimited Spreadsheet.vi"("file path (dialog if empty)"=path "C:/Users/Administrator/Desktop/产品信息.txt", "1D data"=w446, "append to file? (new file:F)"=TRUE) -> ()  [unwired: 11 in, 2 out]
        n231 = call "KB-EMG Input.vi"("Other Message"="自动开始" ("t"), "EMG Iput"="EMG", "Emg"=FALSE) -> ("String OutPut"=w479:string)  [unwired: 8 in]
        n232 = call "Enqueue Element Array.vi"("priority"=w488, "device error in"=w455, "queue index"=2, "error in"=w466, "master data"=w479, "queue in"=w485) -> ("error out"=w490:errorcluster)  [unwired: 4 in, 1 out]
      }
      frame "<-----自动加工结束--------手动部分------->" {
        w573 = u16 0 items=["HPRI"=1, "LPRI"=0] ("priority")
        # "//读取配置文件"
        n233 = local read "设备状态"() -> (w572:string)
        n234 = Concatenate Strings(w572, "....." ("字符串"), "\r\n", w568) -> (w569:string)
        n235 = local write "设备状态"(w569) -> ()
        n236 = call "Enqueue Element Array.vi"("priority"=w573, "queue index"=2, "error in"=w575, "master data"="" ("Element 1"), "queue in"=w578) -> ("error out"=w577:errorcluster)  [unwired: 5 in, 1 out]
      }
      frame "*Emergency alarm" {
        w586 = u16 1 items=["HPRI"=1, "LPRI"=0] ("priority")
        w587 = u16 0 items=["HPRI"=1, "LPRI"=0] ("priority")
        n237 = call "Enqueue Element Array.vi"("priority"=w586, "queue index"=0, "error in"=w580, "master data"="" ("Element 1"), "queue in"=w583) -> ("error out"=w581:errorcluster, "queue out"=w582:T25)  [unwired: 5 in]
        n238 = call "SetTestInfoIndex.vi"("test info index"=13) -> ()
        n239 = call "Enqueue Element Array.vi"("priority"=w587, "queue index"=2, "error in"=w581, "master data"="" ("Element 1"), "queue in"=w582) -> ("error out"=w591:errorcluster)  [unwired: 5 in, 1 out]
      }
    }
    n240 = Wait (ms)(milliseconds to wait=w173) -> ()  [unwired: 1 out]
  }
  n241 = while {
    shift-right: [w598] -> w33
    shift-left: w2 -> [w603]
    shift-right: [w601] -> _
    shift-left: w14 -> [w602]
    tunnel: w15 -> [w605]
    tunnel: w14 -> [w597]
    tunnel: w26 -> [w596]
    tunnel: w17 -> [w595]
    tunnel: w8 -> [w594]
    tunnel: w7 -> [w593]
    stop <- w599 stop-if-true
    # "触发"
    # "事件产生，界面效果，外部状态输入DI，（通信），（界面数据显示）"
    n242 = call "Queue Status Array.vi"("error in (no error)"=w603, "queue in"=w605) -> ("error out"=w599:errorcluster, "queue out"=w600:T25)  [unwired: 4 in]
    n243 = event shown="[56] \"Start\": 值改变" {
      selector: _ -> [_ _ _ _ _ _ _ _ _ _ _ _ _ _ _ _ _ _ _ _ _ _ _ _ _ _ _ _ _ _ _ _ _ _ _ _ _ _ _ _ _ _ _ _ _ _ _ _ _ _ _ _ _ _ _ _ _ _ _ _ _]
      dyn-events: _ -> [_ _ _ _ _ _ _ _ _ _ _ _ _ _ _ _ _ _ _ _ _ _ _ _ _ _ _ _ _ _ _ _ _ _ _ _ _ _ _ _ _ _ _ _ _ _ _ _ _ _ _ _ _ _ _ _ _ _ _ _ _]
      timeout: 50 -> [_ _ _ _ _ _ _ _ _ _ _ _ _ _ _ _ _ _ _ _ _ _ _ _ _ _ _ _ _ _ _ _ _ _ _ _ _ _ _ _ _ _ _ _ _ _ _ _ _ _ _ _ _ _ _ _ _ _ _ _ _]
      tunnel: w602 -> [w610 w618 w625 _ _ _ _ _ _ _ _ _ _ _ _ _ _ _ _ _ _ _ _ _ _ _ _ _ _ _ _ _ _ _ _ _ _ _ _ _ _ _ _ _ _ _ _ _ _ _ _ _ _ _ _ _ _ _ _ _ _]
      tunnel: [w610 w618 w625 _ _ _ _ _ _ _ _ _ _ _ _ _ _ _ _ _ _ _ _ _ _ _ _ _ _ _ _ _ _ _ _ _ _ _ _ _ _ _ _ _ _ _ _ _ _ _ _ _ _ _ _ _ _ _ _ _ _] -> w601
      tunnel: [errorcluster {"status"=FALSE, "code"=0, "source"=""} ("error out") _ _ _ _ _ _ _ _ _ _ _ _ _ _ _ _ _ _ _ _ _ _ _ _ _ _ _ _ _ _ _ _ _ _ _ _ _ _ _ _ _ _ _ _ _ _ _ _ _ _ _ _ _ _ _ _ _ _ _ _] -> _
      tunnel: w600 -> [w608 w617 w624 w712 w720 w731 w738 w744 w753 w762 w771 w780 w798 w818 w833 w842 _ _ _ _ _ _ _ _ _ _ _ _ _ _ _ _ _ _ _ _ _ _ _ _ _ _ _ _ _ _ _ _ _ _ _ _ w1069 w1078 w1090 w1092 w1101 w1124 w1143 w1183 w1221]
      tunnel: w599 -> [w607 w616 w623 w711 w719 w730 w737 w743 w752 w761 w770 w779 w793 w817 w832 w841 w852 w860 w866 w872 w878 w884 w890 w896 w902 w908 w914 w920 w926 w932 w938 w944 w950 w956 w962 w968 w974 w980 w986 w992 w998 w1004 w1010 w1016 w1022 w1028 w1034 w1040 w1046 w1052 w1058 w1064 w1068 w1077 w1089 w1091 w1100 w1123 w1142 w1179 w1210]
      tunnel: [w607 w615 w622 _ w718 w728 w735 w742 w751 w760 w769 w778 w793 w817 w831 w840 w851 w859 w865 w871 w877 w883 w889 w895 w901 w907 w913 w919 w925 w931 w937 w943 w949 w955 w961 w967 w973 w979 w985 w991 w997 w1003 w1009 w1015 w1021 w1027 w1033 w1039 w1045 w1051 w1057 w1063 w1067 w1076 w1088 _ _ w1121 w1142 w1178 w1220] -> w598
      tunnel: [w608 w614 w621 _ _ w729 w736 _ _ _ _ _ w798 w818 _ _ _ _ _ _ _ _ _ _ _ _ _ _ _ _ _ _ _ _ _ _ _ _ _ _ _ _ _ _ _ _ _ _ _ _ _ _ _ _ _ _ _ w1122 w1143 w1183 w1217] -> _
      tunnel: w597 -> [_ _ _ _ _ _ _ _ _ _ _ _ _ _ _ _ _ _ _ _ _ _ _ _ _ _ _ _ _ _ _ _ _ _ _ _ _ _ _ _ _ _ _ _ _ _ _ _ _ _ _ _ _ _ _ _ _ _ _ _ _]
      tunnel: w596 -> [_ _ _ _ _ _ _ _ _ _ _ _ _ _ _ _ _ _ _ _ _ _ _ _ _ _ _ _ _ _ _ _ _ _ _ _ _ _ _ _ _ _ _ _ _ _ _ _ _ _ _ _ _ _ _ _ _ _ w1135 _ _]
      tunnel: w595 -> [_ _ _ _ _ _ _ _ _ _ _ _ _ _ _ _ _ _ _ _ _ _ _ _ _ _ _ _ _ _ _ _ _ _ _ _ _ _ _ _ _ _ _ _ _ _ _ _ _ _ _ _ _ _ _ _ _ _ w1133 _ _]
      tunnel: w594 -> [_ _ _ _ _ _ _ _ _ _ _ _ _ _ _ _ _ w862 w868 w874 w880 w886 w892 w898 w904 w910 w916 w922 w928 w934 w940 w946 w952 w958 w964 w970 w976 w982 w988 w994 w1000 w1006 w1012 w1018 w1024 w1030 w1036 w1042 w1048 w1054 w1060 w1066 _ _ _ _ w1099 _ w1128 w1176 w1212]
      tunnel: w593 -> [_ _ _ _ _ _ _ _ _ _ _ _ _ _ _ _ _ w857 w863 w869 w875 w881 w887 w893 w899 w905 w911 w917 w923 w929 w935 w941 w947 w953 w959 w965 w971 w977 w983 w989 w995 w1001 w1007 w1013 w1019 w1025 w1031 w1037 w1043 w1049 w1055 w1061 _ _ _ _ w1098 _ w1129 w1177 w1211]
      event Timeout {
        # "不要在事件结构里面放入\"弹出窗口\"这样的VI保证该循环畅通无阻。"
        n244 = event-data() -> ()  [unwired: 1 in, 1 out]
      }
      event Panel Close? {
        w612 = u16 1 items=["HPRI"=1, "LPRI"=0] ("priority")
        n245 = event-data() -> ()  [unwired: 1 in, 4 out]
        n246 = call "Enqueue Element Array.vi"("priority"=w612, "queue index"=0, "error in"=w616, "master data"="*Exit application", "queue in"=w617) -> ("error out"=w615:errorcluster, "queue out"=w614:T25)  [unwired: 5 in]
        n247 = event-data("Discard?"=TRUE) -> ()  [unwired: 1 in, 1 out]
      }
      event Menu Selection (User) {
        n248 = event-data() -> ("ItemTag"=w620:string)  [unwired: 1 in, 6 out]
        n249 = case shown="\"产品型号删除\"" w620 {
          tunnel: w624 -> [w627 w635 w640 w652 w666 w673 w680 w687 w691 w698 w705 w710]
          tunnel: w623 -> [w626 w634 w639 w651 w665 w672 w679 w686 w690 w697 w704 w709]
          tunnel: [w626 w633 w638 w650 w664 w671 w678 w685 w688 w695 w702 w709] -> w622
          tunnel: [w627 w632 w637 w649 w663 w670 w677 w684 w689 w696 w703 w710] -> w621
          frame "登陆", Default {
            (unwired) enum32{"Login", "Statistics"}."Login" ("Login and Satistics")
            (unwired) enum32{"Login", "UPH"}."Login" ("Main UPH and Login")
            n250 = property on="选项卡控件" class="TabCtl (严格)"("Value"=T2."Home" ("选项卡控件")) -> ()  [unwired: 2 in, 2 out]
          }
          frame "SOP帮助" {
            w630 = u16 1 items=["HPRI"=1, "LPRI"=0] ("priority")
            n251 = call "Enqueue Element Array.vi"("priority"=w630, "queue index"=0, "error in"=w634, "master data"="SOP帮助", "queue in"=w635) -> ("error out"=w633:errorcluster, "queue out"=w632:T25)  [unwired: 5 in]
          }
          frame "PLC信号" {
            n252 = disable-structure shown="禁用" {
              disable-tunnel: w640 -> [w647 _]
              disable-tunnel: w639 -> [w646 _]
              disable-tunnel: [w645 _] -> w638
              disable-tunnel: [w644 _] -> w637
              frame Disabled {
                w642 = u16 1 items=["HPRI"=1, "LPRI"=0] ("priority")
                n253 = call "Enqueue Element Array.vi"("priority"=w642, "queue index"=0, "error in"=w646, "master data"="SOP帮助", "queue in"=w647) -> ("error out"=w645:errorcluster, "queue out"=w644:T25)  [unwired: 5 in]
              }
              frame Enabled {
              }
            }
            n254 = property on="选项卡控件" class="TabCtl (严格)"("Value"=T2."Machine Paramter and Control" ("选项卡控件")) -> ()  [unwired: 2 in, 2 out]
          }
          frame "数据库清理" {
            n255 = disable-structure shown="禁用" {
              disable-tunnel: w652 -> [w659 _]
              disable-tunnel: w651 -> [w658 _]
              disable-tunnel: [w657 _] -> w650
              disable-tunnel: [w656 _] -> w649
              frame Disabled {
                w654 = u16 1 items=["HPRI"=1, "LPRI"=0] ("priority")
                n256 = call "Enqueue Element Array.vi"("priority"=w654, "queue index"=0, "error in"=w658, "master data"="数据库清理", "queue in"=w659) -> ("error out"=w657:errorcluster, "queue out"=w656:T25)  [unwired: 5 in]
              }
              frame Enabled {
              }
            }
            n257 = property on="选项卡控件" class="TabCtl (严格)"("Value"=T2."Data and Run Information " ("选项卡控件")) -> ()  [unwired: 2 in, 2 out]
          }
          frame "基本参数设置" {
            w661 = u16 1 items=["HPRI"=1, "LPRI"=0] ("priority")
            n258 = call "Enqueue Element Array.vi"("priority"=w661, "queue index"=0, "error in"=w665, "master data"="基本参数设", "queue in"=w666) -> ("error out"=w664:errorcluster, "queue out"=w663:T25)  [unwired: 5 in]
          }
          frame "型号选择" {
            w668 = u16 1 items=["HPRI"=1, "LPRI"=0] ("priority")
            n259 = call "Enqueue Element Array.vi"("priority"=w668, "queue index"=0, "error in"=w672, "master data"="型号选择", "queue in"=w673) -> ("error out"=w671:errorcluster, "queue out"=w670:T25)  [unwired: 5 in]
          }
          frame "产品型号新增" {
            w675 = u16 1 items=["HPRI"=1, "LPRI"=0] ("priority")
            n260 = call "Enqueue Element Array.vi"("priority"=w675, "queue index"=0, "error in"=w679, "master data"="产品新增", "queue in"=w680) -> ("error out"=w678:errorcluster, "queue out"=w677:T25)  [unwired: 5 in]
          }
          frame "产品型号删除" {
            w682 = u16 1 items=["HPRI"=1, "LPRI"=0] ("priority")
            n261 = call "Enqueue Element Array.vi"("priority"=w682, "queue index"=0, "error in"=w686, "master data"="产品型号删除", "queue in"=w687) -> ("error out"=w685:errorcluster, "queue out"=w684:T25)  [unwired: 5 in]
          }
          frame "相机参数设置" {
            w693 = u16 1 items=["HPRI"=1, "LPRI"=0] ("priority")
            n262 = call "Enqueue Element Array.vi"("priority"=w693, "queue index"=0, "error in"=w690, "master data"="Vision Paramter and Control", "queue in"=w691) -> ("error out"=w688:errorcluster, "queue out"=w689:T25)  [unwired: 5 in]
          }
          frame "镭射参数设置" {
            w700 = u16 1 items=["HPRI"=1, "LPRI"=0] ("priority")
            n263 = call "Enqueue Element Array.vi"("priority"=w700, "queue index"=0, "error in"=w697, "master data"="Machine Paramter and Control", "queue in"=w698) -> ("error out"=w695:errorcluster, "queue out"=w696:T25)  [unwired: 5 in]
          }
          frame "串口参数设置" {
            w707 = u16 1 items=["HPRI"=1, "LPRI"=0] ("priority")
            n264 = call "Enqueue Element Array.vi"("priority"=w707, "queue index"=0, "error in"=w704, "master data"="Machine Alarm Histroy", "queue in"=w705) -> ("error out"=w702:errorcluster, "queue out"=w703:T25)  [unwired: 5 in]
          }
          frame "参数设置" {
          }
        }
      }
      event "计数器清零": Value Change {
        n265 = event-data() -> ()  [unwired: 1 in, 6 out]
        n266 = stacked-sequence {
          tunnel: w712 -> [w714 _]
          tunnel: w711 -> [w713 _]
          frame #0 {
            w716 = u16 1 items=["HPRI"=1, "LPRI"=0] ("priority")
            n267 = call "Enqueue Element Array.vi"("priority"=w716, "queue index"=2, "error in"=w713, "master data"="清除", "queue in"=w714) -> ()  [unwired: 5 in, 2 out]
          }
          frame #1 {
            (unwired) 0.0 ("计数器")
          }
        }
      }
      event Value Change {
        n268 = event-data() -> ()  [unwired: 1 in, 6 out]
        n269 = stacked-sequence {
          tunnel: w720 -> [w723]
          tunnel: w719 -> [w722]
          tunnel: [w721] -> w718
          frame #0 {
            w725 = u16 1 items=["HPRI"=1, "LPRI"=0] ("priority")
            (unwired) enum32{"Login", "Statistics"}."Login" ("Login and Satistics")
            n270 = call "Enqueue Element Array.vi"("priority"=w725, "queue index"=0, "error in"=w722, "master data"="登录", "queue in"=w723) -> ("error out"=w721:errorcluster)  [unwired: 5 in, 1 out]
            n271 = property on="选项卡控件" class="TabCtl (严格)"("Value"=T2."Home" ("选项卡控件")) -> ()  [unwired: 2 in, 2 out]
          }
        }
      }
      event Value Change {
        w733 = u16 1 items=["HPRI"=1, "LPRI"=0] ("priority")
        n272 = event-data() -> ()  [unwired: 1 in, 3 out]
        n273 = call "Enqueue Element Array.vi"("priority"=w733, "queue index"=0, "error in"=w730, "master data"="Machine Paramter and Control", "queue in"=w731) -> ("error out"=w728:errorcluster, "queue out"=w729:T25)  [unwired: 5 in]
      }
      event "清空数据库": Value Change {
        w740 = u16 1 items=["HPRI"=1, "LPRI"=0] ("priority")
        n274 = event-data() -> ()  [unwired: 1 in, 6 out]
        n275 = call "Enqueue Element Array.vi"("priority"=w740, "queue index"=0, "error in"=w737, "master data"="数据库清理", "queue in"=w738) -> ("error out"=w735:errorcluster, "queue out"=w736:T25)  [unwired: 5 in]
      }
      event Value Change {
        n276 = event-data() -> ()  [unwired: 1 in, 3 out]
        n277 = stacked-sequence {
          tunnel: w744 -> [w747]
          tunnel: w743 -> [w746]
          tunnel: [w745] -> w742
          frame #0 {
            w749 = u16 1 items=["HPRI"=1, "LPRI"=0] ("priority")
            n278 = call "Enqueue Element Array.vi"("priority"=w749, "queue index"=0, "error in"=w746, "master data"="Machine Inforamtion", "queue in"=w747) -> ("error out"=w745:errorcluster)  [unwired: 5 in, 1 out]
          }
        }
      }
      event Value Change {
        n279 = event-data() -> ()  [unwired: 1 in, 3 out]
        n280 = stacked-sequence {
          tunnel: w753 -> [w756]
          tunnel: w752 -> [w755]
          tunnel: [w754] -> w751
          frame #0 {
            w758 = u16 1 items=["HPRI"=1, "LPRI"=0] ("priority")
            n281 = call "Enqueue Element Array.vi"("priority"=w758, "queue index"=0, "error in"=w755, "master data"="型号选择", "queue in"=w756) -> ("error out"=w754:errorcluster)  [unwired: 5 in, 1 out]
          }
        }
      }
      event Value Change {
        n282 = event-data() -> ()  [unwired: 1 in, 3 out]
        n283 = stacked-sequence {
          tunnel: w762 -> [w765]
          tunnel: w761 -> [w764]
          tunnel: [w763] -> w760
          frame #0 {
            w767 = u16 1 items=["HPRI"=1, "LPRI"=0] ("priority")
            n284 = call "Enqueue Element Array.vi"("priority"=w767, "queue index"=0, "error in"=w764, "master data"="Machine Alarm Histroy", "queue in"=w765) -> ("error out"=w763:errorcluster)  [unwired: 5 in, 1 out]
          }
        }
      }
      event Value Change {
        n285 = event-data() -> ()  [unwired: 1 in, 3 out]
        n286 = stacked-sequence {
          tunnel: w771 -> [w774]
          tunnel: w770 -> [w773]
          tunnel: [w772] -> w769
          frame #0 {
            w776 = u16 1 items=["HPRI"=1, "LPRI"=0] ("priority")
            n287 = call "Enqueue Element Array.vi"("priority"=w776, "queue index"=0, "error in"=w773, "master data"="Data and Run Information", "queue in"=w774) -> ("error out"=w772:errorcluster)  [unwired: 5 in, 1 out]
          }
        }
      }
      event Value Change {
        n288 = event-data() -> ()  [unwired: 1 in, 3 out]
        n289 = stacked-sequence {
          tunnel: w780 -> [w783]
          tunnel: w779 -> [w782]
          tunnel: [w781] -> w778
          frame #0 {
            w785 = u16 1 items=["HPRI"=1, "LPRI"=0] ("priority")
            n290 = call "Enqueue Element Array.vi"("priority"=w785, "queue index"=0, "error in"=w782, "master data"="Open Image File", "queue in"=w783) -> ("error out"=w781:errorcluster)  [unwired: 5 in, 1 out]
          }
        }
      }
      event "搜索项": Value Change {
        n291 = event-data() -> ("NewVal"=w796:string)  [unwired: 1 in]
        n292 = Match Pattern(string=w796, regular expression=".png" ("正则表达式"), offset (0)=0 ("偏移量(0)")) -> (offset past match=w790:i32)  [unwired: 3 out]
        n293 = Match Pattern(string=w796, regular expression=".jpeg" ("正则表达式"), offset (0)=0 ("偏移量(0)")) -> (offset past match=w794:i32)  [unwired: 3 out]
        n294 = Less Than 0?(x=w790) -> (x < 0?=w789:bool)
        n295 = Less Than 0?(x=w794) -> (x < 0?=w788:bool)
        n296 = Not And(1:w788, 2:w789) -> (0:w787:bool)
        n297 = case shown="真" w787 {
          tunnel: w796 -> [_ w811]
          tunnel: w793 -> [_ w806]
          frame False {
            n298 = One Button Dialog(message="请点击选择图片" ("消息")) -> ()  [unwired: 1 in, 1 out]
          }
          frame True {
            w807 = T27 4 items=["Grayscale (U8)", "Grayscale (I16)", "Grayscale (SGL)", "Complex (CSG)", "RGB (U32)", "HSL (U32)", "RGB (U64)", "Grayscale (U16)"] ("Image Type")
            w809 = 0 ("开始索引(0)")
            n299 = local read "项名称"() -> (w810:string[])
            n300 = call "IMAQ Create"("Border Size"=w809, "Image Name"="Test", "Image Type"=w807, "error in (no error)"=w806) -> ("New Image"=w805:T1, "error out"=w804:errorcluster)  [unwired: 1 in]
            n301 = Search 1D Array(1D array=w810, element=w811, start index (0)=w809) -> (index of element=w803:i32)
            n302 = local read "All Files in Dir"() -> (w802:path[])
            n303 = Index Array(array=w802, index=w803) -> (element=w801:path)
            n304 = call "IMAQ ReadFile"("File Path"=w801, "error in (no error)"=w804, "Image"=w805) -> ("Image Out"=→"查询图片":T1)  [unwired: 4 in, 4 out]
          }
        }
      }
      event "文件名": Value Change {
        n305 = event-data() -> ("NewVal"=w812:string)  [unwired: 1 in]
        n306 = Match Pattern(string=w812, regular expression=".xls" ("正则表达式"), offset (0)=0 ("偏移量(0)")) -> (offset past match=w814:i32)  [unwired: 3 out]
        n307 = Greater Than 0?(x=w814) -> (x > 0?=w813:bool)
        n308 = case shown="真" w813 {
          tunnel: w817 -> [_ w827]
          tunnel: w812 -> [_ w820]
          frame False {
            n309 = One Button Dialog(message="请点击选择图片" ("消息")) -> ()  [unwired: 1 in, 1 out]
          }
          frame True {
            n310 = local read "项名称 2"() -> (w824:string[])
            n311 = local read "All Files in Dir 2"() -> (w825:path[])
            n312 = Search 1D Array(1D array=w824, element=w820, start index (0)=0 ("开始索引(0)")) -> (index of element=w829:i32)
            n313 = Index Array(array=w825, index=w829) -> (element=w828:path)
            n314 = call "读取历史数据.vi"("file path (dialog if empty)"=w828, "error in (no error)"=w827) -> ("Title"=w821:string[], "Data"=w823:string[][], "行首字符串"=w822:string[], "数据波形图"=→"数据波形图":dbl[][])  [unwired: 9 in, 1 out]
            n315 = property on="压力数据显示" class="Tbl (严格)"("Column Headers[]"=w821, "Row Headers[]"=w822, "Value"=w823) -> ()  [unwired: 2 in, 2 out]
          }
        }
      }
      event "搜索历史图片": Value Change {
        n316 = event-data() -> ()  [unwired: 1 in, 6 out]
        n317 = stacked-sequence {
          tunnel: w833 -> [w836]
          tunnel: w832 -> [w835]
          tunnel: [w834] -> w831
          frame #0 {
            w838 = u16 1 items=["HPRI"=1, "LPRI"=0] ("priority")
            n318 = call "Enqueue Element Array.vi"("priority"=w838, "queue index"=0, "error in"=w835, "master data"="Search Histroy Image", "queue in"=w836) -> ("error out"=w834:errorcluster)  [unwired: 5 in, 1 out]
          }
        }
      }
      event Value Change {
        n319 = event-data() -> ()  [unwired: 1 in, 3 out]
        n320 = stacked-sequence {
          tunnel: w842 -> [w845]
          tunnel: w841 -> [w844]
          tunnel: [w843] -> w840
          frame #0 {
            w847 = u16 1 items=["HPRI"=1, "LPRI"=0] ("priority")
            n321 = call "Enqueue Element Array.vi"("priority"=w847, "queue index"=0, "error in"=w844, "master data"="Open Excel File", "queue in"=w845) -> ("error out"=w843:errorcluster)  [unwired: 5 in, 1 out]
          }
        }
      }
      event "确定按钮": Value Change {
        n322 = event-data() -> ()  [unwired: 1 in, 6 out]
        n323 = local read "压力表打印代码据库"() -> (w850:string[][])
        n324 = local read "压力表数据库"() -> (w856:string[][])
        n325 = call "长度判断.vi"("输入元素 2"="输入", "error in (no error)"=w852, "压力打印代码据库"=w850, "压力表数据库"=w856, "输入元素"="输入") -> ("error out"=w851:errorcluster, "压力表打印代码"=→"压力表打印代码":string, "产品种类"=→"产品种类":string, "压力表有无判定"=→"结果":string)  [unwired: 3 in]
      }
      event "DB5000.X.字符识别启动\n信号-读": Value Change {
        n326 = event-data() -> ("NewVal"=w861:bool)  [unwired: 1 in, 1 out]
        n327 = call "DB5000.X写.vi"("引用"=w862, "semaphore"=w857, "地址名称"="字符识别启动信号-读" ("组合框"), "value"=w861, "error in (no error)"=w860) -> ("error out"=w859:errorcluster)  [unwired: 9 in, 1 out]
      }
      event "DB5000.X.电脑1扫码枪\n触发-读": Value Change {
        n328 = event-data() -> ("NewVal"=w867:bool)  [unwired: 1 in, 1 out]
        n329 = call "DB5000.X写.vi"("引用"=w868, "semaphore"=w863, "地址名称"="电脑1扫码枪触发-读" ("组合框"), "value"=w867, "error in (no error)"=w866) -> ("error out"=w865:errorcluster)  [unwired: 9 in, 1 out]
      }
      event "DB5000.X.电脑1CCD读取\n字符触发-读": Value Change {
        n330 = event-data() -> ("NewVal"=w873:bool)  [unwired: 1 in, 1 out]
        n331 = call "DB5000.X写.vi"("引用"=w874, "semaphore"=w869, "地址名称"="电脑1CCD读取字符触发-读" ("组合框"), "value"=w873, "error in (no error)"=w872) -> ("error out"=w871:errorcluster)  [unwired: 9 in, 1 out]
      }
      event "DB5000.X.电脑1表面检测\n触发-读": Value Change {
        n332 = event-data() -> ("NewVal"=w879:bool)  [unwired: 1 in, 1 out]
        n333 = call "DB5000.X写.vi"("引用"=w880, "semaphore"=w875, "地址名称"="电脑1表面检测触发-读" ("组合框"), "value"=w879, "error in (no error)"=w878) -> ("error out"=w877:errorcluster)  [unwired: 9 in, 1 out]
      }
      event "DB5000.X.电脑1穿管检测\n触发-读": Value Change {
        n334 = event-data() -> ("NewVal"=w885:bool)  [unwired: 1 in, 1 out]
        n335 = call "DB5000.X写.vi"("引用"=w886, "semaphore"=w881, "地址名称"="电脑1穿管检测触发-读" ("组合框"), "value"=w885, "error in (no error)"=w884) -> ("error out"=w883:errorcluster)  [unwired: 9 in, 1 out]
      }
      event "DB5000.X.区间位置\n1-读": Value Change {
        n336 = event-data() -> ("NewVal"=w891:bool)  [unwired: 1 in, 1 out]
        n337 = call "DB5000.X写.vi"("引用"=w892, "semaphore"=w887, "地址名称"="区间位置1-读" ("组合框"), "value"=w891, "error in (no error)"=w890) -> ("error out"=w889:errorcluster)  [unwired: 9 in, 1 out]
      }
      event "DB5000.X.前后位置\n切换触发-读": Value Change {
        n338 = event-data() -> ("NewVal"=w897:bool)  [unwired: 1 in, 1 out]
        n339 = call "DB5000.X写.vi"("引用"=w898, "semaphore"=w893, "地址名称"="电脑1产品前后位置切换触发-读" ("组合框"), "value"=w897, "error in (no error)"=w896) -> ("error out"=w895:errorcluster)  [unwired: 9 in, 1 out]
      }
      event "DB5000.X.电脑1压力获取\n触发-读": Value Change {
        n340 = event-data() -> ("NewVal"=w903:bool)  [unwired: 1 in, 1 out]
        n341 = call "DB5000.X写.vi"("引用"=w904, "semaphore"=w899, "地址名称"="电脑1压力获取触发-读" ("组合框"), "value"=w903, "error in (no error)"=w902) -> ("error out"=w901:errorcluster)  [unwired: 9 in, 1 out]
      }
      event "DB5000.X.PC1 ready-\n写": Value Change {
        n342 = event-data() -> ("NewVal"=w909:bool)  [unwired: 1 in, 1 out]
        n343 = call "DB5000.X写.vi"("引用"=w910, "semaphore"=w905, "地址名称"="PC1 ready-写" ("组合框"), "value"=w909, "error in (no error)"=w908) -> ("error out"=w907:errorcluster)  [unwired: 9 in, 1 out]
      }
      event "DB5000.X.混料-写": Value Change {
        n344 = event-data() -> ("NewVal"=w915:bool)  [unwired: 1 in, 1 out]
        n345 = call "DB5000.X写.vi"("引用"=w916, "semaphore"=w911, "地址名称"="混料-写" ("组合框"), "value"=w915, "error in (no error)"=w914) -> ("error out"=w913:errorcluster)  [unwired: 9 in, 1 out]
      }
      event "DB5000.X.字符1检测\npass-写": Value Change {
        n346 = event-data() -> ("NewVal"=w921:bool)  [unwired: 1 in, 1 out]
        n347 = call "DB5000.X写.vi"("引用"=w922, "semaphore"=w917, "地址名称"="字符1检测pass-写" ("组合框"), "value"=w921, "error in (no error)"=w920) -> ("error out"=w919:errorcluster)  [unwired: 9 in, 1 out]
      }
      event "DB5000.X.字符1检测\nfail-写": Value Change {
        n348 = event-data() -> ("NewVal"=w927:bool)  [unwired: 1 in, 1 out]
        n349 = call "DB5000.X写.vi"("引用"=w928, "semaphore"=w923, "地址名称"="字符1检测fail-写" ("组合框"), "value"=w927, "error in (no error)"=w926) -> ("error out"=w925:errorcluster)  [unwired: 9 in, 1 out]
      }
      event "DB5000.X.表面检测\npass-写": Value Change {
        n350 = event-data() -> ("NewVal"=w933:bool)  [unwired: 1 in, 1 out]
        n351 = call "DB5000.X写.vi"("引用"=w934, "semaphore"=w929, "地址名称"="表面检测pass-写" ("组合框"), "value"=w933, "error in (no error)"=w932) -> ("error out"=w931:errorcluster)  [unwired: 9 in, 1 out]
      }
      event "DB5000.X.表面检测\nfail-写": Value Change {
        n352 = event-data() -> ("NewVal"=w939:bool)  [unwired: 1 in, 1 out]
        n353 = call "DB5000.X写.vi"("引用"=w940, "semaphore"=w935, "地址名称"="表面检测fail-写" ("组合框"), "value"=w939, "error in (no error)"=w938) -> ("error out"=w937:errorcluster)  [unwired: 9 in, 1 out]
      }
      event "DB5000.X.穿管检测\npass-写": Value Change {
        n354 = event-data() -> ("NewVal"=w945:bool)  [unwired: 1 in, 1 out]
        n355 = call "DB5000.X写.vi"("引用"=w946, "semaphore"=w941, "地址名称"="穿管检测pass-写" ("组合框"), "value"=w945, "error in (no error)"=w944) -> ("error out"=w943:errorcluster)  [unwired: 9 in, 1 out]
      }
      event "DB5000.X.穿管检测\nfail-写": Value Change {
        n356 = event-data() -> ("NewVal"=w951:bool)  [unwired: 1 in, 1 out]
        n357 = call "DB5000.X写.vi"("引用"=w952, "semaphore"=w947, "地址名称"="穿管检测fail-写" ("组合框"), "value"=w951, "error in (no error)"=w950) -> ("error out"=w949:errorcluster)  [unwired: 9 in, 1 out]
      }
      event "DB5000.X.扫码枪\npass-写": Value Change {
        n358 = event-data() -> ("NewVal"=w957:bool)  [unwired: 1 in, 1 out]
        n359 = call "DB5000.X写.vi"("引用"=w958, "semaphore"=w953, "地址名称"="扫码枪pass-写" ("组合框"), "value"=w957, "error in (no error)"=w956) -> ("error out"=w955:errorcluster)  [unwired: 9 in, 1 out]
      }
      event "DB5000.X.扫码枪fail-\n写": Value Change {
        n360 = event-data() -> ("NewVal"=w963:bool)  [unwired: 1 in, 1 out]
        n361 = call "DB5000.X写.vi"("引用"=w964, "semaphore"=w959, "地址名称"="扫码枪fail-写" ("组合框"), "value"=w963, "error in (no error)"=w962) -> ("error out"=w961:errorcluster)  [unwired: 9 in, 1 out]
      }
      event "DB5000.X.产品尺寸A-\n写": Value Change {
        n362 = event-data() -> ("NewVal"=w969:bool)  [unwired: 1 in, 1 out]
        n363 = call "DB5000.X写.vi"("引用"=w970, "semaphore"=w965, "地址名称"="产品尺寸A-写" ("组合框"), "value"=w969, "error in (no error)"=w968) -> ("error out"=w967:errorcluster)  [unwired: 9 in, 1 out]
      }
      event "DB5000.X.产品尺寸B-\n写": Value Change {
        n364 = event-data() -> ("NewVal"=w975:bool)  [unwired: 1 in, 1 out]
        n365 = call "DB5000.X写.vi"("引用"=w976, "semaphore"=w971, "地址名称"="产品尺寸B-写" ("组合框"), "value"=w975, "error in (no error)"=w974) -> ("error out"=w973:errorcluster)  [unwired: 9 in, 1 out]
      }
      event "DB5000.X.数据传递\n信号-读": Value Change {
        n366 = event-data() -> ("NewVal"=w981:bool)  [unwired: 1 in, 1 out]
        n367 = call "DB5000.X写.vi"("引用"=w982, "semaphore"=w977, "地址名称"="数据传递信号-读" ("组合框"), "value"=w981, "error in (no error)"=w980) -> ("error out"=w979:errorcluster)  [unwired: 9 in, 1 out]
      }
      event "DB5000.X.表面检测完\n成信号-读": Value Change {
        n368 = event-data() -> ("NewVal"=w987:bool)  [unwired: 1 in, 1 out]
        n369 = call "DB5000.X写.vi"("引用"=w988, "semaphore"=w983, "地址名称"="表面检测完成信号-读" ("组合框"), "value"=w987, "error in (no error)"=w986) -> ("error out"=w985:errorcluster)  [unwired: 9 in, 1 out]
      }
      event "DB5000.X.穿管NG停止\n信号-写": Value Change {
        n370 = event-data() -> ("NewVal"=w993:bool)  [unwired: 1 in, 1 out]
        n371 = call "DB5000.X写.vi"("引用"=w994, "semaphore"=w989, "地址名称"="穿管NG停止信号-写" ("组合框"), "value"=w993, "error in (no error)"=w992) -> ("error out"=w991:errorcluster)  [unwired: 9 in, 1 out]
      }
      event "DB5000.X.电脑1返工\n信号-写": Value Change {
        n372 = event-data() -> ("NewVal"=w999:bool)  [unwired: 1 in, 1 out]
        n373 = call "DB5000.X写.vi"("引用"=w1000, "semaphore"=w995, "地址名称"="电脑1返工信号-写" ("组合框"), "value"=w999, "error in (no error)"=w998) -> ("error out"=w997:errorcluster)  [unwired: 9 in, 1 out]
      }
      event "DB5000.X.PLC初始化\n信号-读": Value Change {
        n374 = event-data() -> ("NewVal"=w1005:bool)  [unwired: 1 in, 1 out]
        n375 = call "DB5000.X写.vi"("引用"=w1006, "semaphore"=w1001, "地址名称"="PLC初始化信号-读" ("组合框"), "value"=w1005, "error in (no error)"=w1004) -> ("error out"=w1003:errorcluster)  [unwired: 9 in, 1 out]
      }
      event "DB5000.X.产品尺寸C-\n写": Value Change {
        n376 = event-data() -> ("NewVal"=w1011:bool)  [unwired: 1 in, 1 out]
        n377 = call "DB5000.X写.vi"("引用"=w1012, "semaphore"=w1007, "地址名称"="产品尺寸C-写" ("组合框"), "value"=w1011, "error in (no error)"=w1010) -> ("error out"=w1009:errorcluster)  [unwired: 9 in, 1 out]
      }
      event "DB5000.X.表面检测错位\n气缸-读": Value Change {
        n378 = event-data() -> ("NewVal"=w1017:bool)  [unwired: 1 in, 1 out]
        n379 = call "DB5000.X写.vi"("引用"=w1018, "semaphore"=w1013, "地址名称"="表面检测错位气缸-读" ("组合框"), "value"=w1017, "error in (no error)"=w1016) -> ("error out"=w1015:errorcluster)  [unwired: 9 in, 1 out]
      }
      event "DB5000.X.电脑1衬丝检测\n触发-读": Value Change {
        n380 = event-data() -> ("NewVal"=w1023:bool)  [unwired: 1 in, 1 out]
        n381 = call "DB5000.X写.vi"("引用"=w1024, "semaphore"=w1019, "地址名称"="电脑1衬丝检测触发-读" ("组合框"), "value"=w1023, "error in (no error)"=w1022) -> ("error out"=w1021:errorcluster)  [unwired: 9 in, 1 out]
      }
      event "DB5000.X.衬丝能检测\npass-写": Value Change {
        n382 = event-data() -> ("NewVal"=w1029:bool)  [unwired: 1 in, 1 out]
        n383 = call "DB5000.X写.vi"("引用"=w1030, "semaphore"=w1025, "地址名称"="衬丝能检测pass-写" ("组合框"), "value"=w1029, "error in (no error)"=w1028) -> ("error out"=w1027:errorcluster)  [unwired: 9 in, 1 out]
      }
      event "DB5000.X.衬丝能检测f\nail-写": Value Change {
        n384 = event-data() -> ("NewVal"=w1035:bool)  [unwired: 1 in, 1 out]
        n385 = call "DB5000.X写.vi"("引用"=w1036, "semaphore"=w1031, "地址名称"="衬丝能检测fail-写" ("组合框"), "value"=w1035, "error in (no error)"=w1034) -> ("error out"=w1033:errorcluster)  [unwired: 9 in, 1 out]
      }
      event "DB5000.X.长衬丝-写": Value Change {
        n386 = event-data() -> ("NewVal"=w1041:bool)  [unwired: 1 in, 1 out]
        n387 = call "DB5000.X写.vi"("引用"=w1042, "semaphore"=w1037, "地址名称"="长衬丝-写" ("组合框"), "value"=w1041, "error in (no error)"=w1040) -> ("error out"=w1039:errorcluster)  [unwired: 9 in, 1 out]
      }
      event "DB5000.X.短衬丝-写": Value Change {
        n388 = event-data() -> ("NewVal"=w1047:bool)  [unwired: 1 in, 1 out]
        n389 = call "DB5000.X写.vi"("引用"=w1048, "semaphore"=w1043, "地址名称"="短衬丝-写" ("组合框"), "value"=w1047, "error in (no error)"=w1046) -> ("error out"=w1045:errorcluster)  [unwired: 9 in, 1 out]
      }
      event "DB5000.X.细料-写": Value Change {
        n390 = event-data() -> ("NewVal"=w1053:bool)  [unwired: 1 in, 1 out]
        n391 = call "DB5000.X写.vi"("引用"=w1054, "semaphore"=w1049, "地址名称"="细料-写" ("组合框"), "value"=w1053, "error in (no error)"=w1052) -> ("error out"=w1051:errorcluster)  [unwired: 9 in, 1 out]
      }
      event "DB5000.X.粗料-写": Value Change {
        n392 = event-data() -> ("NewVal"=w1059:bool)  [unwired: 1 in, 1 out]
        n393 = call "DB5000.X写.vi"("引用"=w1060, "semaphore"=w1055, "地址名称"="粗料-写" ("组合框"), "value"=w1059, "error in (no error)"=w1058) -> ("error out"=w1057:errorcluster)  [unwired: 9 in, 1 out]
      }
      event "DB5000.X.一致性检测\n触发-读": Value Change {
        n394 = event-data() -> ("NewVal"=w1065:bool)  [unwired: 1 in, 1 out]
        n395 = call "DB5000.X写.vi"("引用"=w1066, "semaphore"=w1061, "地址名称"="一致性检测触发-读" ("组合框"), "value"=w1065, "error in (no error)"=w1064) -> ("error out"=w1063:errorcluster)  [unwired: 9 in, 1 out]
      }
      event Value Change {
        n396 = event-data() -> ()  [unwired: 1 in, 3 out]
        n397 = stacked-sequence {
          tunnel: w1069 -> [w1072]
          tunnel: w1068 -> [w1071]
          tunnel: [w1070] -> w1067
          frame #0 {
            w1074 = u16 1 items=["HPRI"=1, "LPRI"=0] ("priority")
            n398 = call "Enqueue Element Array.vi"("priority"=w1074, "queue index"=2, "error in"=w1071, "master data"="Machine Paramter Save Buttom", "queue in"=w1072) -> ("error out"=w1070:errorcluster)  [unwired: 5 in, 1 out]
          }
        }
      }
      event Value Change {
        n399 = event-data() -> ()  [unwired: 1 in, 3 out]
        n400 = stacked-sequence {
          tunnel: w1078 -> [w1081]
          tunnel: w1077 -> [w1080]
          tunnel: [w1079] -> w1076
          frame #0 {
            w1083 = u16 1 items=["HPRI"=1, "LPRI"=0] ("priority")
            n401 = call "Enqueue Element Array.vi"("priority"=w1083, "queue index"=0, "error in"=w1080, "master data"="Save 压力表数据库 Message", "queue in"=w1081) -> ("error out"=w1079:errorcluster)  [unwired: 5 in, 1 out]
          }
        }
      }
      event Value Change {
        w1086 = u16 1 items=["HPRI"=1, "LPRI"=0] ("priority")
        n402 = event-data() -> ()  [unwired: 1 in, 3 out]
        n403 = call "Enqueue Element Array.vi"("priority"=w1086, "queue index"=2, "error in"=w1089, "master data"="Other Param Save Buttom", "queue in"=w1090) -> ("error out"=w1088:errorcluster)  [unwired: 5 in, 1 out]
      }
      event Value Change {
        n404 = event-data() -> ()  [unwired: 1 in, 6 out]
        n405 = stacked-sequence {
          tunnel: w1092 -> [w1094]
          tunnel: w1091 -> [w1093]
          frame #0 {
            w1096 = u16 1 items=["HPRI"=1, "LPRI"=0] ("priority")
            n406 = call "Enqueue Element Array.vi"("priority"=w1096, "queue index"=0, "error in"=w1093, "master data"="Home", "queue in"=w1094) -> ()  [unwired: 5 in, 2 out]
          }
        }
      }
      event Value Change {
        n407 = event-data() -> ()  [unwired: 1 in, 6 out]
        n408 = stacked-sequence {
          tunnel: w1101 -> [w1117]
          tunnel: w1100 -> [w1106]
          tunnel: w1099 -> [w1104]
          tunnel: w1098 -> [w1103]
          frame #0 {
            w1109 = TRUE ("电脑一表面检测图像处理状态")
            w1119 = u16 1 items=["HPRI"=1, "LPRI"=0] ("priority")
            n409 = Current VI's Menubar() -> (w1110:refnum<k9>)
            n410 = call "军蚁-启用菜单功能.vi"("数组"=bool[] [FALSE, FALSE, TRUE, FALSE, FALSE, FALSE, FALSE, FALSE], "菜单引用"=w1110) -> ()  [unwired: 9 in, 1 out]
            n411 = call "DB5000.X写.vi"("引用"=w1104, "semaphore"=w1103, "地址名称"="PC1 ready-写" ("组合框"), "value"=TRUE, "error in (no error)"=w1106) -> ("error out"=w1105:errorcluster)  [unwired: 9 in, 1 out]
            n412 = property on="Pause" class="Bool (严格)"("DisabledEnum"=T22."Enabled" ("禁用"), "Value"=TRUE ("可见")) -> ()  [unwired: 2 in, 2 out]
            n413 = global write "Global System.vi" "Paus"(FALSE ("Paus")) -> ()
            n414 = property on="选项卡控件" class="TabCtl (严格)"("Value"=T2."Home" ("选项卡控件")) -> ()  [unwired: 2 in, 2 out]
            n415 = call "Enqueue Element Array.vi"("priority"=w1119, "queue index"=0, "error in"=w1105, "master data"="Autotest running", "queue in"=w1117) -> ()  [unwired: 5 in, 2 out]
            n416 = property on="Start" class="Bool (严格)"("DisabledEnum"=T22."Disabled and Grayed Out" ("禁用")) -> ()  [unwired: 2 in, 2 out]
            n417 = property on="Vision Paramter and Control" class="Bool (严格)"("DisabledEnum"=T22."Disabled and Grayed Out" ("禁用")) -> ()  [unwired: 2 in, 2 out]
            n418 = local write "电脑一穿管检测状态"(w1109) -> ()
            n419 = local write "电脑一表面检测图像处理状态"(w1109) -> ()
            n420 = local write "电脑一条码枪扫码状态"(w1109) -> ()
            n421 = local write "电脑一穿管压力获取状态"(w1109) -> ()
            n422 = local write "电脑一CCD读字符状态"(w1109) -> ()
          }
        }
      }
      event Value Change {
        w1126 = u16 1 items=["HPRI"=1, "LPRI"=0] ("priority")
        n423 = event-data() -> ()  [unwired: 1 in, 6 out]
        n424 = call "Enqueue Element Array.vi"("priority"=w1126, "queue index"=2, "error in"=w1123, "master data"="Vision Paramter Save", "queue in"=w1124) -> ("error out"=w1121:errorcluster, "queue out"=w1122:T25)  [unwired: 5 in]
      }
      event Value Change {
        n425 = event-data() -> ()  [unwired: 1 in, 1 out]
        n426 = flat-sequence {
          tunnel: [w1147] -> w1140
          tunnel: [w1147] -> w1139
          tunnel: [w1146] -> w1136
          tunnel: w1135 -> [w1146]
          tunnel: [w1145] -> w1134
          tunnel: w1133 -> [w1145]
          tunnel: [w1144] -> w1130
          tunnel: w1140 -> [w1169]
          tunnel: [w1169] -> w1138
          tunnel: w1139 -> [_]
          tunnel: w1136 -> [w1168]
          tunnel: w1134 -> [w1167]
          tunnel: [w1154] -> w1132
          tunnel: [w1166] -> w1131
          tunnel: w1130 -> [w1165]
          tunnel: w1128 -> [w1153]
          tunnel: w1129 -> [w1152]
          tunnel: w1128 -> [w1151]
          tunnel: w1138 -> [w1173]
          tunnel: [w1173] -> w1137
          tunnel: w1132 -> [w1171]
          tunnel: w1131 -> [w1170]
          tunnel: w1137 -> [w1175]
          frame #0 {
            n427 = global read "Global System.vi" "ADODB._Connection Out"() -> (w1144:refnum<k7>)
            n428 = Two Button Dialog(message="退出程序" ("消息"), 1:"取消" ("F按钮名称（“取消”）"), 2:"确定" ("T按钮名称（“确定”）")) -> (T button?=w1147:bool)
          }
          frame #1 {
            n429 = call <userlib>:"ADO Connection Close.vi"("ADODB._Connection In"=w1165) -> ()  [unwired: 9 in, 2 out]
            n430 = call <vilib>:"Acquire Semaphore.vi"("error in (no error)"=w1167, "semaphore"=w1168) -> ("error out"=w1155:errorcluster, "semaphore out"=w1166:T23)  [unwired: 3 in, 1 out]
            n431 = call "关闭SIEMENS.vi"("gInitialSIEMENSS7 In"=w1151) -> ()  [unwired: 10 in, 1 out]
            n432 = global read "Global System.vi" "Session Out CCD0"() -> (w1164:T28)
            n433 = global read "Global System.vi" "Session Out CCD1"() -> (w1163:T28)
            n434 = global read "Global System.vi" "Session Out CCD2"() -> (w1162:T28)
            n435 = global read "Global System.vi" "Session Out CCD3"() -> (w1161:T28)
            n436 = global read "Global System.vi" "Session Out CCD4"() -> (w1160:T28)
            n437 = global read "Global System.vi" "Session Out CCD5"() -> (w1159:T28)
            n438 = global read "Global System.vi" "Session Out CCD6"() -> (w1158:T28)
            n439 = Build Array(w1164, w1163, w1162, w1161, w1160, w1159, w1158) -> ()  [unwired: 1 out]
            n440 = call "DB5000.X写.vi"("引用"=w1153, "semaphore"=w1152, "地址名称"="PC1 ready-写" ("组合框"), "value"=FALSE, "error in (no error)"=w1155) -> ("error out"=w1154:errorcluster)  [unwired: 9 in, 1 out]
          }
          frame #2 {
            n441 = call <vilib>:"Release Semaphore Reference.vi"("error in (no error)"=w1171, "semaphore"=w1170) -> ()  [unwired: 8 in, 2 out]
            n442 = Wait (ms)(milliseconds to wait=u32 500 ("等待时间（毫秒）")) -> ()  [unwired: 1 out]
          }
          frame #3 {
            w1174 = FALSE ("电脑一表面检测图像处理状态")
            n443 = Quit LabVIEW(quit? (T)=w1175) -> ()
            n444 = local write "电脑一穿管检测状态"(w1174) -> ()
            n445 = local write "电脑一表面检测图像处理状态"(w1174) -> ()
            n446 = local write "电脑一条码枪扫码状态"(w1174) -> ()
            n447 = local write "电脑一穿管压力获取状态"(w1174) -> ()
            n448 = local write "电脑一CCD读字符状态"(w1174) -> ()
          }
        }
        n449 = property on="Start" class="Bool (严格)"("DisabledEnum"=T22."Enabled" ("禁用")) -> ()  [unwired: 2 in, 2 out]
      }
      event Value Change {
        n450 = event-data() -> ()  [unwired: 1 in, 6 out]
        n451 = flat-sequence {
          tunnel: [w1185] -> w1182
          tunnel: [w1185] -> _
          tunnel: [w1184] -> w1180
          tunnel: w1182 -> [w1205]
          tunnel: [w1205] -> w1181
          tunnel: w1180 -> [w1204]
          tunnel: w1179 -> [w1195]
          tunnel: [w1194] -> w1178
          tunnel: w1176 -> [w1193]
          tunnel: w1177 -> [w1192]
          tunnel: w1176 -> [w1189]
          tunnel: w1181 -> [w1207]
          frame #0 {
            n452 = global read "Global System.vi" "ADODB._Connection Out"() -> (w1184:refnum<k7>)
            n453 = Two Button Dialog(message="退出程序" ("消息"), 1:"取消" ("F按钮名称（“取消”）"), 2:"确定" ("T按钮名称（“确定”）")) -> (T button?=w1185:bool)
          }
          frame #1 {
            n454 = call "关闭SIEMENS.vi"("gInitialSIEMENSS7 In"=w1189) -> ()  [unwired: 10 in, 1 out]
            n455 = global read "Global System.vi" "Session Out CCD2"() -> (w1201:T28)
            n456 = global read "Global System.vi" "Session Out CCD0"() -> (w1203:T28)
            n457 = global read "Global System.vi" "Session Out CCD1"() -> (w1202:T28)
            n458 = global read "Global System.vi" "Session Out CCD3"() -> (w1200:T28)
            n459 = global read "Global System.vi" "Session Out CCD4"() -> (w1199:T28)
            n460 = global read "Global System.vi" "Session Out CCD5"() -> (w1198:T28)
            n461 = global read "Global System.vi" "Session Out CCD6"() -> (w1197:T28)
            n462 = call "DB5000.X写.vi"("引用"=w1193, "semaphore"=w1192, "地址名称"="PC1 ready-写" ("组合框"), "value"=FALSE, "error in (no error)"=w1195) -> ("error out"=w1194:errorcluster)  [unwired: 9 in, 1 out]
            n463 = Build Array(w1203, w1202, w1201, w1200, w1199, w1198, w1197) -> (w1196:T28[])
            n464 = call <userlib>:"ADO Connection Close.vi"("ADODB._Connection In"=w1204) -> ()  [unwired: 9 in, 2 out]
            n465 = call "相机关闭.vi"("数组"=w1196) -> ()  [unwired: 10 in, 1 out]
          }
          frame #2 {
            w1206 = FALSE ("电脑一表面检测图像处理状态")
            n466 = Quit LabVIEW(quit? (T)=w1207) -> ()
            n467 = local write "电脑一穿管检测状态"(w1206) -> ()
            n468 = local write "电脑一表面检测图像处理状态"(w1206) -> ()
            n469 = local write "电脑一条码枪扫码状态"(w1206) -> ()
            n470 = local write "电脑一穿管压力获取状态"(w1206) -> ()
            n471 = local write "电脑一CCD读字符状态"(w1206) -> ()
          }
        }
      }
      event Value Change {
        w1215 = FALSE ("电脑一表面检测图像处理状态")
        (unwired) T22."Enabled" ("禁用")
        (unwired) "Pause" ("布尔文本.文本")
        (unwired) cluster{u32, u32}[] [{16711680, 0}] ("颜色[4]")
        n472 = event-data() -> ()  [unwired: 1 in, 6 out]
        n473 = local write "Start"(T14 TRUE ("Start")) -> ()
        n474 = property on="Pause" class="Bool (严格)"("DisabledEnum"=T22."Disabled and Grayed Out" ("禁用")) -> ()  [unwired: 2 in, 2 out]
        n475 = call "DB5000.X写.vi"("引用"=w1212, "semaphore"=w1211, "地址名称"="PC1 ready-写" ("组合框"), "value"=FALSE, "error in (no error)"=w1210) -> ("error out"=w1209:errorcluster)  [unwired: 9 in, 1 out]
        n476 = property on="Start" class="Bool (严格)"("DisabledEnum"=T22."Enabled" ("禁用")) -> ()  [unwired: 2 in, 2 out]
        n477 = local write "电脑一穿管检测状态"(w1215) -> ()
        n478 = local write "电脑一表面检测图像处理状态"(w1215) -> ()
        n479 = local write "电脑一条码枪扫码状态"(w1215) -> ()
        n480 = local write "电脑一穿管压力获取状态"(w1215) -> ()
        n481 = local write "电脑一CCD读字符状态"(w1215) -> ()
        n482 = property on="Vision Paramter and Control" class="Bool (严格)"("DisabledEnum"=T22."Enabled" ("禁用")) -> ()  [unwired: 2 in, 2 out]
        n483 = local read "Ground 2"() -> (w1216:u16)
        n484 = global write "Global System.vi" "Paus"(TRUE ("Paus")) -> ()
        n485 = case shown="5" w1216 {
          frame 0, 1 {
            # "Administrator"
            n486 = Current VI's Menubar() -> (w1224:refnum<k9>)
            n487 = call "军蚁-启用菜单功能.vi"("数组"=bool[] [TRUE, TRUE, FALSE, FALSE, FALSE, TRUE, TRUE, TRUE], "菜单引用"=w1224) -> ()  [unwired: 9 in, 1 out]
          }
          frame 2, Default {
            # "Operator"
            n488 = Current VI's Menubar() -> (w1226:refnum<k9>)
            n489 = call "军蚁-启用菜单功能.vi"("数组"=bool[] [FALSE, FALSE, FALSE, FALSE, FALSE, FALSE, FALSE, FALSE], "菜单引用"=w1226) -> ()  [unwired: 9 in, 1 out]
          }
          frame 5 {
            # "Administrator"
            n490 = Current VI's Menubar() -> (w1228:refnum<k9>)
            n491 = call "军蚁-启用菜单功能.vi"("数组"=bool[] [TRUE, TRUE, FALSE, FALSE, FALSE, TRUE, TRUE, TRUE], "菜单引用"=w1228) -> ()  [unwired: 9 in, 1 out]
          }
        }
        n492 = disable-structure shown="禁用" {
          disable-tunnel: w1221 -> [w1237 _]
          disable-tunnel: w1210 -> [w1236 _]
          disable-tunnel: [w1235 _] -> w1220
          disable-tunnel: [w1234 _] -> w1217
          disable-tunnel: w1209 -> [w1230 _]
          frame Disabled {
            w1232 = u16 1 items=["HPRI"=1, "LPRI"=0] ("priority")
            n493 = call "Enqueue Element Array.vi"("priority"=w1232, "device error in"=w1230, "queue index"=2, "error in"=w1236, "master data"="", "queue in"=w1237) -> ("error out"=w1235:errorcluster, "queue out"=w1234:T25)  [unwired: 4 in]
          }
          frame Enabled {
          }
        }
      }
    }
    n494 = call "GetSystemTime.vi"() -> ("date/time string"=→"system time":string)  [unwired: 7 in]
  }
  n495 = while {
    shift-right: [w1251] -> w34
    shift-left: w2 -> [w1239]
    shift-right: [w1245] -> _
    shift-left: w14 -> [w1246]
    tunnel: w15 -> [w1241]
    stop <- w1250 stop-if-true
    # "主流程控制"
    n496 = call "Dequeue Element Array.vi"("queue in"=w1241, "queue index"=0 ("timeout in ms (-1)"), "error in"=w1239) -> ("queue out"=w1243:T25, "master data"=w1238:string, "secondary data"=w1242:string[], "error out"=w1244:errorcluster)  [unwired: 2 in, 1 out]
    n497 = case shown="\"型号选择\"" w1238 {
      tunnel: w1243 -> [_ w1266 w1275 w1294 w1297 w1308 w1317 w1329 _ w1393 w1409 _ w1419 w1427 w1435 w1443 _ w1457 w1462 w1487 w1528 w1532 _ w1555 w1565 w1575 w1584 w1594 w1604 w1620 w1637 w1666 w1694 w1709 w1718 w1735 w1745 w1755 w1769 w1785 w1808 w1814 _ w1832 _ _ _ w1855]
      tunnel: w1244 -> [w1252 w1262 w1269 w1291 w1296 w1304 w1313 w1320 w1387 w1390 w1407 w1414 w1417 w1425 w1433 w1441 w1448 w1454 w1461 w1486 w1526 w1531 w1547 w1550 w1560 w1570 w1579 w1588 w1598 w1614 w1628 w1659 w1688 w1704 w1712 w1730 w1740 w1750 w1758 w1779 w1803 w1816 w1822 w1831 w1840 w1843 w1847 w1851]
      tunnel: [w1252 w1265 w1274 w1293 w1301 w1307 w1316 w1328 w1387 w1392 w1408 w1414 w1418 w1426 w1434 w1442 w1448 w1456 w1460 w1490 w1493 w1530 w1547 w1554 w1564 w1574 w1583 w1593 w1603 w1619 w1636 w1665 w1693 w1708 w1717 w1734 w1744 w1754 w1768 w1784 w1807 w1820 w1822 w1830 w1840 w1843 w1847 w1854] -> w1251
      tunnel: [_ _ _ _ _ _ _ _ _ _ _ _ _ _ _ _ _ _ _ _ _ _ _ _ _ _ _ _ _ _ _ _ _ _ _ _ _ _ _ _ _ _ _ _ TRUE _ _ _] -> w1248
      tunnel: [_ 50 50 50 50 50 10 10 _ 50 50 _ 50 50 50 50 _ 50 50 50 50 20 _ 50 50 50 50 50 50 50 50 50 50 50 50 50 50 50 50 50 50 50 _ 50 10 _ 50 50] -> w1247
      tunnel: w1246 -> [w1253 w1261 w1272 w1288 w1299 w1305 w1314 w1324 w1388 w1397 w1413 w1415 w1423 w1431 w1439 w1447 w1449 w1455 w1479 w1482 w1527 w1534 w1548 w1552 w1562 w1572 w1581 w1591 w1601 w1617 w1634 w1663 w1691 w1706 w1715 w1732 w1742 w1752 w1766 w1782 w1805 w1818 w1823 w1829 w1841 w1844 w1848 w1852]
      tunnel: [w1253 w1260 w1272 w1288 w1299 w1305 w1314 w1323 w1388 w1397 w1413 w1415 w1423 w1431 w1439 w1447 w1449 w1455 w1479 w1482 w1527 w1534 w1548 w1552 w1562 w1572 w1581 w1591 w1601 w1617 w1634 w1663 w1691 w1706 w1715 w1732 w1742 w1752 w1766 w1782 w1805 w1818 w1823 w1829 w1841 w1844 w1848 w1852] -> w1245
      tunnel: w1242 -> [_ _ _ _ _ _ _ _ _ _ _ _ _ _ _ _ _ _ _ _ _ _ _ _ _ _ _ _ _ _ _ _ _ _ _ _ _ _ _ _ _ _ _ w1828 _ _ _ _]
      frame "----------初始化----------" {
      }
      frame "Read system configuration file" {
        # "系统文件属于不给客户开放的参数配置"
        n498 = call "SetTestInfoIndex.vi"("test info index"=-1) -> ()
        n499 = global read "Global System.vi" "ref path"() -> (w1255:path)
        n500 = Build Path ("创建路径")(base path=w1255, name or relative path="SystemDefine.ini" ("名称或相对路径")) -> (appended path=w1254:path)
        n501 = call "ReadSysConfigForStart.vi"("error in"=w1262, "configuration file path"=w1254) -> ("error out"=w1257:errorcluster, "用户登录"=w1259:T29)  [unwired: 8 in]
        n502 = Bundle By Name(cluster=w1261, "用户登录"=w1259) -> (w1260:T21)
        n503 = call "Enqueue Element Array.vi"("device error in"=w1257, "queue index"=0, "error in"=w1262, "master data"="Read user configuration file" ("Element 1"), "queue in"=w1266) -> ("error out"=w1265:errorcluster)  [unwired: 5 in, 1 out]
      }
      frame "Read user configuration file" {
        # "用户文件属于给客户开放的参数配置"
        n504 = call "SetTestInfoIndex.vi"("test info index"=-1) -> ()
        n505 = disable-structure shown="启用" {
          disable-tunnel: w1269 -> [w1278 w1280]
          disable-tunnel: [w1277 w1280] -> w1268
          frame Disabled {
            n506 = call "ReadSysParaSetting.vi"("error in"=w1278, "config file name"="UserDefine.ini") -> ("error out"=w1277:errorcluster)  [unwired: 8 in, 1 out]
          }
          frame Enabled {
          }
        }
        n507 = call "Enqueue Element Array.vi"("device error in"=w1268, "queue index"=0, "error in"=w1269, "master data"="Initialization interface" ("Element 1"), "queue in"=w1275) -> ("error out"=w1274:errorcluster)  [unwired: 5 in, 1 out]
      }
      frame "Initialization interface" {
        (unwired) path "D:/Inspect System/Source Code/压力表型号数据库.txt" ("基路径")
        (unwired) enum32{"Login", "Statistics"}."Login" ("Login and Satistics")
        n508 = call "SetTestInfoIndex.vi"("test info index"=-1) -> ()
        n509 = global read "Global System.vi" "ref path"() -> (w1285:path)
        n510 = Build Path(base path=w1285, name or relative path="压力表型号数据库.txt" ("名称或相对路径")) -> (appended path=w1283:path)
        n511 = Build Path(base path=w1285, name or relative path="压力表打印代码.txt" ("名称或相对路径")) -> (appended path=w1282:path)
        n512 = call-poly <vilib>:"Read Delimited Spreadsheet.vi"("file path (dialog if empty)"=w1282) -> ("all rows"=w1281:string[][])  [unwired: 9 in, 5 out]
        n513 = call-poly <vilib>:"Read Delimited Spreadsheet.vi"("file path (dialog if empty)"=w1283) -> ("all rows"=w1287:string[][])  [unwired: 9 in, 5 out]
        n514 = local write "压力表打印代码据库"(w1281) -> ()
        n515 = local write "压力表数据库"(w1287) -> ()
        n516 = call "Enqueue Element Array.vi"("queue index"=0, "error in"=w1291, "master data"="Hardware initialization" ("Element 1"), "queue in"=w1294) -> ("error out"=w1293:errorcluster)  [unwired: 6 in, 1 out]
      }
      frame "Hardware initialization" {
        # "设备硬件的初始化，这里有可能会有多步。\ncase结构可以在下面无限添加。"
        n517 = call "Enqueue Element Array.vi"("queue index"=0, "error in"=w1296, "master data"="" ("Element 1"), "queue in"=w1297) -> ("error out"=w1301:errorcluster)  [unwired: 6 in, 1 out]
      }
      frame "----------用户登录----------" {
        n518 = call "Enqueue Element Array.vi"("queue index"=0, "error in"=w1304, "master data"="" ("Element 1"), "queue in"=w1308) -> ("error out"=w1307:errorcluster)  [unwired: 6 in, 1 out]
      }
      frame "登录" {
        n519 = call "登录.vi"("error in (no error)"=w1313) -> ("error in (no error) 2"=w1312:errorcluster, "Ground 2"=→"Ground 2":u16, "Element 1"=w1311:string)  [unwired: 8 in]
        n520 = call "Enqueue Element Array.vi"("device error in"=w1312, "queue index"=0, "error in"=w1313, "master data"=w1311, "queue in"=w1317) -> ("error out"=w1316:errorcluster)  [unwired: 5 in, 1 out]
      }
      frame "*Initialization UI after login" {
        (unwired) string[] ["参数设置", "基本参数设置", "相机参数设置", "串口参数设置", "网络参数设置", "图像处理序列", "型号选择"]
        n521 = local read "Ground 2"() -> (w1319:u16)
        n522 = Bundle By Name(cluster=w1324, "用户权限"=w1319) -> (w1323:T21)
        n523 = call "SetTestInfoIndex.vi"("test info index"=15) -> ()
        n524 = Current VI's Menubar() -> (w1322:refnum<k9>)
        n525 = case shown="5" w1319 {
          tunnel: w1322 -> [w1348 w1366 w1386]
          tunnel: T22."Disabled and Grayed Out" ("禁用") -> [_ _ _]
          tunnel: w1320 -> [w1338 w1357 w1381]
          frame 2, Default {
            (unwired) enum32{"Login", "Statistics"}."Statistics" ("Login and Satistics")
            # "Operator"
            n526 = call "军蚁-启用菜单功能.vi"("error in"=w1338, "数组"=bool[] [FALSE, FALSE, FALSE, FALSE, FALSE, FALSE, FALSE, FALSE], "菜单引用"=w1348) -> ()  [unwired: 8 in, 1 out]
            n527 = control-ref of="Start"() -> (w1337:refnum<vi>)
            n528 = control-ref of="Pause"() -> (w1336:refnum<vi>)
            n529 = control-ref of="Stop"() -> (w1335:refnum<vi>)
            n530 = control-ref of="Vision Paramter and Control"() -> (w1344:refnum<vi>)
            n531 = control-ref of="Open Excel File"() -> (w1334:refnum<vi>)
            n532 = control-ref of="Machine Paramter and Control"() -> (w1345:refnum<vi>)
            n533 = control-ref of="Data and Run Information"() -> (w1343:refnum<vi>)
            n534 = control-ref of="Machine Inforamtion"() -> (w1342:refnum<vi>)
            n535 = control-ref of="Machine Alarm Histroy"() -> (w1341:refnum<vi>)
            n536 = control-ref of="Data and Run Information"() -> (w1340:refnum<vi>)
            n537 = Build Array(w1337, w1336, w1335, w1334) -> (w1333:refnum<vi>[])
            n538 = Build Array(w1345, w1344, w1343, w1342, w1341, w1340) -> (w1339:refnum<vi>[])
            n539 = call "军蚁-工具栏按钮操作.vi"("error in (no error)"=w1338, "布尔"=FALSE, "禁用"=T22."Disabled and Grayed Out", "引用数组"=w1339) -> ()  [unwired: 7 in, 1 out]
            n540 = call "军蚁-工具栏按钮操作.vi"("error in (no error)"=w1338, "布尔"=TRUE, "禁用"=T22."Enabled", "引用数组"=w1333) -> ()  [unwired: 7 in, 1 out]
          }
          frame 5 {
            (unwired) bool[] [TRUE, FALSE, FALSE, FALSE, FALSE, FALSE, FALSE]
            (unwired) enum32{"Login", "Statistics"}."Statistics" ("Login and Satistics")
            w1355 = TRUE
            # "Engineer"
            n541 = call "军蚁-启用菜单功能.vi"("error in"=w1357, "数组"=bool[] [TRUE, TRUE, FALSE, FALSE, FALSE, TRUE, TRUE, TRUE], "菜单引用"=w1366) -> ()  [unwired: 8 in, 1 out]
            n542 = control-ref of="Start"() -> (w1361:refnum<vi>)
            n543 = control-ref of="Pause"() -> (w1360:refnum<vi>)
            n544 = control-ref of="Stop"() -> (w1359:refnum<vi>)
            n545 = control-ref of="Data and Run Information"() -> (w1362:refnum<vi>)
            n546 = control-ref of="Open Excel File"() -> (w1363:refnum<vi>)
            n547 = control-ref of="Open Image File"() -> (w1364:refnum<vi>)
            n548 = control-ref of="Machine Paramter and Control"() -> (w1354:refnum<vi>)
            n549 = control-ref of="Vision Paramter and Control"() -> (w1353:refnum<vi>)
            n550 = control-ref of="Machine Inforamtion"() -> (w1352:refnum<vi>)
            n551 = Build Array(w1361, w1360, w1359, w1362, w1363, w1364) -> (w1358:refnum<vi>[])
            n552 = Build Array(w1354, w1353, w1352) -> (w1351:refnum<vi>[])
            n553 = call "军蚁-工具栏按钮操作.vi"("error in (no error)"=w1357, "布尔"=w1355, "禁用"=T22."Enabled", "引用数组"=w1358) -> ()  [unwired: 7 in, 1 out]
            n554 = call "军蚁-工具栏按钮操作.vi"("error in (no error)"=w1357, "布尔"=w1355, "禁用"=T22."Disabled and Grayed Out", "引用数组"=w1351) -> ()  [unwired: 7 in, 1 out]
          }
          frame 0, 1 {
            (unwired) enum32{"Login", "Statistics"}."Statistics" ("Login and Satistics")
            # "Administrator"
            n555 = control-ref of="Data and Run Information"() -> (w1368:refnum<vi>)
            n556 = control-ref of="Open Excel File"() -> (w1383:refnum<vi>)
            n557 = Build Array(w1368, w1383) -> (w1382:refnum<vi>[])
            n558 = call "军蚁-启用菜单功能.vi"("error in"=w1381, "数组"=bool[] [TRUE, TRUE, FALSE, FALSE, FALSE, TRUE, TRUE, TRUE], "菜单引用"=w1386) -> ()  [unwired: 8 in, 1 out]
            n559 = control-ref of="Start"() -> (w1378:refnum<vi>)
            n560 = control-ref of="Pause"() -> (w1377:refnum<vi>)
            n561 = control-ref of="Stop"() -> (w1376:refnum<vi>)
            n562 = control-ref of="Open Excel File"() -> (w1375:refnum<vi>)
            n563 = control-ref of="Open Image File"() -> (w1374:refnum<vi>)
            n564 = control-ref of="Machine Paramter and Control"() -> (w1373:refnum<vi>)
            n565 = control-ref of="Vision Paramter and Control"() -> (w1372:refnum<vi>)
            n566 = control-ref of="Machine Inforamtion"() -> (w1371:refnum<vi>)
            n567 = control-ref of="Machine Alarm Histroy"() -> (w1367:refnum<vi>)
            n568 = Build Array(w1378, w1377, w1376, w1375, w1374, w1373, w1372, w1371, w1367) -> (w1370:refnum<vi>[])
            n569 = call "军蚁-工具栏按钮操作.vi"("error in (no error)"=w1381, "布尔"=TRUE, "禁用"=T22."Enabled", "引用数组"=w1370) -> ()  [unwired: 7 in, 1 out]
            n570 = call "军蚁-工具栏按钮操作.vi"("error in (no error)"=w1381, "布尔"=FALSE, "禁用"=T22."Disabled and Grayed Out", "引用数组"=w1382) -> ()  [unwired: 7 in, 1 out]
          }
        }
        n571 = call "Enqueue Element Array.vi"("queue index"=0, "error in"=w1320, "master data"="" ("Element 1"), "queue in"=w1329) -> ("error out"=w1328:errorcluster)  [unwired: 6 in, 1 out]
      }
      frame "----------参数设置----------" {
      }
      frame "Parameter setup" {
        # "parameter setup  dialogbox\n\nInitial UI"
        n572 = call "SetTestInfoIndex.vi"("test info index"=1) -> ()
        n573 = disable-structure shown="禁用" {
          disable-tunnel: w1390 -> [w1399 w1402]
          disable-tunnel: [w1398 w1402] -> w1389
          frame Disabled {
            n574 = global read "Global System.vi" "ref path"() -> (w1401:path)
            n575 = call "Read User File Data.vi"("error in"=w1399, "名称或相对路径"="SystemDefine.ini", "ref path"=w1401) -> ("error out"=w1398:errorcluster)  [unwired: 7 in, 1 out]
          }
          frame Enabled {
          }
        }
        n576 = call "Enqueue Element Array.vi"("device error in"=w1389, "queue index"=0, "error in"=w1390, "master data"="" ("Element 1"), "queue in"=w1393) -> ("error out"=w1392:errorcluster)  [unwired: 5 in, 1 out]
      }
      frame "Save data" {
        n577 = call "SetTestInfoIndex.vi"("test info index"=1) -> ()
        n578 = global read "Global System.vi" "ref path"() -> (w1405:path)
        n579 = Build Path(base path=w1405, name or relative path="UserDefine.ini" ("名称或相对路径")) -> (appended path=w1403:path)
        n580 = call "Write Data To User File.vi"("File path"=w1403) -> ()  [unwired: 10 in, 1 out]
        n581 = call "Enqueue Element Array.vi"("queue index"=0, "error in"=w1407, "master data"="" ("Element 1"), "queue in"=w1409) -> ("error out"=w1408:errorcluster)  [unwired: 6 in, 1 out]
      }
      frame "----------界面跳转初始化----------" {
      }
      frame "Main Interface" {
        n582 = call "SetTestInfoIndex.vi"("test info index"=1) -> ()
        n583 = call "Enqueue Element Array.vi"("queue index"=0, "error in"=w1417, "master data"="Reset device" ("Element 1"), "queue in"=w1419) -> ("error out"=w1418:errorcluster)  [unwired: 6 in, 1 out]
      }
      frame "Reset device" {
        n584 = call "SetTestInfoIndex.vi"("test info index"=1) -> ()
        n585 = call "Enqueue Element Array.vi"("queue index"=0, "error in"=w1425, "master data"="Software reset" ("Element 1"), "queue in"=w1427) -> ("error out"=w1426:errorcluster)  [unwired: 6 in, 1 out]
      }
      frame "Software reset" {
        n586 = call "SetTestInfoIndex.vi"("test info index"=1) -> ()
        n587 = call "Enqueue Element Array.vi"("queue index"=0, "error in"=w1433, "master data"="Hardware reset" ("Element 1"), "queue in"=w1435) -> ("error out"=w1434:errorcluster)  [unwired: 6 in, 1 out]
      }
      frame "Hardware reset" {
        n588 = call "SetTestInfoIndex.vi"("test info index"=1) -> ()
        n589 = call "Enqueue Element Array.vi"("queue index"=0, "error in"=w1441, "master data"="" ("Element 1"), "queue in"=w1443) -> ("error out"=w1442:errorcluster)  [unwired: 6 in, 1 out]
      }
      frame "----------自动化测试----------" {
      }
      frame "Autotest running" {
        w1451 = u16 1 items=["HPRI"=1, "LPRI"=0] ("priority")
        n590 = call "SetTestInfoIndex.vi"("test info index"=-1) -> ()
        n591 = disable-structure shown="禁用" {
          frame Disabled {
            n592 = property on="Pause" class="Bool (严格)"("DisabledEnum"=T22."Disabled" ("禁用")) -> ()  [unwired: 2 in, 2 out]
          }
          frame Enabled {
          }
        }
        n593 = call "Enqueue Element Array.vi"("priority"=w1451, "queue index"=0, "error in"=w1454, "master data"="检测启动按钮" ("Element 1"), "queue in"=w1457) -> ("error out"=w1456:errorcluster)  [unwired: 5 in, 1 out]
      }
      frame "所有工位复位" {
        w1463 = u16 1 items=["HPRI"=1, "LPRI"=0] ("priority")
        n594 = call "SetTestInfoIndex.vi"("test info index"=-1) -> ()
        n595 = call "Enqueue Element Array.vi"("priority"=w1463, "queue index"=2, "error in"=w1461, "master data"="读取配置文件", "queue in"=w1462) -> ("error out"=w1467:errorcluster, "queue out"=w1466:T25)  [unwired: 5 in]
        n596 = call "Enqueue Element Array.vi"("priority"=w1463, "queue index"=3, "error in"=w1467, "master data"="读取配置文件", "queue in"=w1466) -> ("error out"=w1469:errorcluster, "queue out"=w1470:T25)  [unwired: 5 in]
        n597 = call "Enqueue Element Array.vi"("priority"=w1463, "queue index"=4, "error in"=w1469, "master data"="读取配置文件", "queue in"=w1470) -> ("error out"=w1471:errorcluster, "queue out"=w1472:T25)  [unwired: 5 in]
        n598 = call "Enqueue Element Array.vi"("priority"=w1463, "queue index"=0, "error in"=w1471, "master data"="检测所有工位复位", "queue in"=w1472) -> ("error out"=w1460:errorcluster)  [unwired: 5 in, 1 out]
      }
      frame "检测所有工位复位" {
        n599 = call "SetTestInfoIndex.vi"("test info index"=-1) -> ()
        n600 = Select(t="Autotest running" ("Element 1"), s=TRUE, f="检测所有工位复位" ("Element 1")) -> (s? t:f=w1483:string)
        n601 = call "Enqueue Element Array.vi"("queue index"=0, "error in"=w1486, "master data"=w1483, "queue in"=w1487) -> ("error out"=w1490:errorcluster)  [unwired: 6 in, 1 out]
      }
      frame "检测启动按钮" {
        w1495 = u16 1 items=["HPRI"=1, "LPRI"=0] ("priority")
        w1500 = u16 1 items=["HPRI"=1, "LPRI"=0] ("priority")
        (unwired) "自动开始" ("t")
        w1507 = u16 1 items=["HPRI"=1, "LPRI"=0] ("priority")
        w1512 = u16 1 items=["HPRI"=1, "LPRI"=0] ("priority")
        w1513 = u16 1 items=["HPRI"=1, "LPRI"=0] ("priority")
        w1520 = u16 1 items=["HPRI"=1, "LPRI"=0] ("priority")
        w1522 = u16 1 items=["HPRI"=1, "LPRI"=0] ("priority")
        n602 = call "SetTestInfoIndex.vi"("test info index"=-1) -> ()
        n603 = call "Enqueue Element Array.vi"("priority"=w1522, "queue index"=6, "error in"=w1526, "master data"="自动开始" ("t"), "queue in"=w1528) -> ("error out"=w1503:errorcluster, "queue out"=w1505:T25)  [unwired: 5 in]
        n604 = call "Enqueue Element Array.vi"("priority"=w1507, "queue index"=5, "error in"=w1503, "master data"="自动开始" ("t"), "queue in"=w1505) -> ("error out"=w1502:errorcluster, "queue out"=w1504:T25)  [unwired: 5 in]
        n605 = call "Enqueue Element Array.vi"("priority"=w1500, "queue index"=3, "error in"=w1502, "master data"="自动开始" ("t"), "queue in"=w1504) -> ("error out"=w1518:errorcluster, "queue out"=w1519:T25)  [unwired: 5 in]
        n606 = call "Enqueue Element Array.vi"("priority"=w1520, "queue index"=4, "error in"=w1518, "master data"="自动开始" ("t"), "queue in"=w1519) -> ("error out"=w1517:errorcluster, "queue out"=w1515:T25)  [unwired: 5 in]
        n607 = call "Enqueue Element Array.vi"("priority"=w1513, "queue index"=2, "error in"=w1517, "queue in"=w1515) -> ("error out"=w1510:errorcluster, "queue out"=w1509:T25)  [unwired: 6 in]
        n608 = call "Enqueue Element Array.vi"("priority"=w1512, "queue index"=7, "error in"=w1510, "master data"="自动开始" ("t"), "queue in"=w1509) -> ("error out"=w1494:errorcluster, "queue out"=w1492:T25)  [unwired: 5 in]
        n609 = call "Enqueue Element Array.vi"("priority"=w1495, "queue index"=8, "error in"=w1494, "master data"="自动开始" ("t"), "queue in"=w1492) -> ("error out"=w1493:errorcluster)  [unwired: 5 in, 1 out]
      }
      frame "马达停止" {
        n610 = call "SetTestInfoIndex.vi"("test info index"=-1) -> ()
        n611 = disable-structure shown="禁用" {
          disable-tunnel: w1532 -> [w1538 _]
          disable-tunnel: w1531 -> [w1537 _]
          disable-tunnel: [w1536 _] -> w1530
          frame Disabled {
            w1543 = u16 1 items=["HPRI"=1, "LPRI"=0] ("priority")
            w1540 = u16 1 items=["HPRI"=1, "LPRI"=0] ("priority")
            n612 = call "Enqueue Element Array.vi"("priority"=w1540, "queue index"=2, "error in"=w1537, "master data"="No event", "queue in"=w1538) -> ("error out"=w1546:errorcluster, "queue out"=w1545:T25)  [unwired: 5 in]
            n613 = call "Enqueue Element Array.vi"("priority"=w1543, "queue index"=3, "error in"=w1546, "master data"="No event", "queue in"=w1545) -> ("error out"=w1536:errorcluster)  [unwired: 5 in, 1 out]
          }
          frame Enabled {
          }
        }
      }
      frame "----------手动测试----------" {
      }
      frame "Manual test" {
        n614 = call "SetTestInfoIndex.vi"("test info index"=11) -> ()
        n615 = call "Enqueue Element Array.vi"("queue index"=0, "error in"=w1550, "master data"="" ("Element 1"), "queue in"=w1555) -> ("error out"=w1554:errorcluster)  [unwired: 6 in, 1 out]
      }
      frame "Machine Paramter and Control" {
        w1557 = TRUE
        n616 = call "SetTestInfoIndex.vi"("test info index"=11) -> ()
        n617 = property on="选项卡控件" class="TabCtl (严格)"("Value"=T2."Machine Paramter and Control" ("选项卡控件")) -> ()  [unwired: 2 in, 2 out]
        n618 = property on="Vision Paramter and Control" class="Bool (严格)"("Value"=w1557) -> ()  [unwired: 2 in, 2 out]
        n619 = property on="Machine Alarm Histroy" class="Bool (严格)"("Value"=w1557) -> ()  [unwired: 2 in, 2 out]
        n620 = property on="Data and Run Information" class="Bool (严格)"("Value"=w1557) -> ()  [unwired: 2 in, 2 out]
        n621 = property on="Machine Inforamtion" class="Bool (严格)"("Value"=w1557) -> ()  [unwired: 2 in, 2 out]
        n622 = property on="Start" class="Bool (严格)"("Value"=w1557) -> ()  [unwired: 2 in, 2 out]
        n623 = property on="Pause" class="Bool (严格)"("Value"=w1557) -> ()  [unwired: 2 in, 2 out]
        n624 = property on="Stop" class="Bool (严格)"("Value"=w1557) -> ()  [unwired: 2 in, 2 out]
        n625 = property on="Open Image File" class="Bool (严格)"("Value"=w1557) -> ()  [unwired: 2 in, 2 out]
        n626 = property on="Open Excel File" class="Bool (严格)"("Value"=w1557) -> ()  [unwired: 2 in, 2 out]
        n627 = property on="User Login" class="Bool (严格)"("Value"=w1557) -> ()  [unwired: 2 in, 2 out]
        n628 = property on="Home" class="Bool (严格)"("Value"=w1557) -> ()  [unwired: 2 in, 2 out]
        n629 = call "Enqueue Element Array.vi"("queue index"=0, "error in"=w1560, "master data"="" ("Element 1"), "queue in"=w1565) -> ("error out"=w1564:errorcluster)  [unwired: 6 in, 1 out]
      }
      frame "Home" {
        (unwired) enum32{"Login", "Statistics"}."Statistics" ("Login and Satistics")
        (unwired) enum32{"Login", "UPH"}."UPH" ("Main UPH and Login")
        w1567 = TRUE
        n630 = call "SetTestInfoIndex.vi"("test info index"=11) -> ()
        n631 = property on="选项卡控件" class="TabCtl (严格)"("Value"=T2."Home" ("选项卡控件")) -> ()  [unwired: 2 in, 2 out]
        n632 = property on="Vision Paramter and Control" class="Bool (严格)"("Value"=w1567) -> ()  [unwired: 2 in, 2 out]
        n633 = property on="Machine Alarm Histroy" class="Bool (严格)"("Value"=w1567) -> ()  [unwired: 2 in, 2 out]
        n634 = property on="Data and Run Information" class="Bool (严格)"("Value"=w1567) -> ()  [unwired: 2 in, 2 out]
        n635 = property on="Machine Inforamtion" class="Bool (严格)"("Value"=w1567) -> ()  [unwired: 2 in, 2 out]
        n636 = property on="Machine Paramter and Control" class="Bool (严格)"("Value"=w1567) -> ()  [unwired: 2 in, 2 out]
        n637 = property on="Start" class="Bool (严格)"("Value"=w1567) -> ()  [unwired: 2 in, 2 out]
        n638 = property on="Pause" class="Bool (严格)"("Value"=w1567) -> ()  [unwired: 2 in, 2 out]
        n639 = property on="Stop" class="Bool (严格)"("Value"=w1567) -> ()  [unwired: 2 in, 2 out]
        n640 = property on="Open Image File" class="Bool (严格)"("Value"=w1567) -> ()  [unwired: 2 in, 2 out]
        n641 = property on="Open Excel File" class="Bool (严格)"("Value"=w1567) -> ()  [unwired: 2 in, 2 out]
        n642 = property on="User Login" class="Bool (严格)"("Value"=w1567) -> ()  [unwired: 2 in, 2 out]
        n643 = call "Enqueue Element Array.vi"("queue index"=0, "error in"=w1570, "master data"="" ("Element 1"), "queue in"=w1575) -> ("error out"=w1574:errorcluster)  [unwired: 6 in, 1 out]
      }
      frame "注册机" {
        n644 = call "注册.vi"("Key Number"="pottery" ("Key")) -> ("error out"=w1577:errorcluster)  [unwired: 10 in]
        n645 = case shown="无错误" w1577 {
          selector: w1577 -> [w1586 _]
          frame No Error {
            n646 = call "显示对话框信息"("error in (no error)"=w1586) -> ()  [unwired: 9 in, 2 out]
          }
          frame Error {
          }
        }
        n647 = call "Enqueue Element Array.vi"("queue index"=0, "error in"=w1579, "master data"="" ("Element 1"), "queue in"=w1584) -> ("error out"=w1583:errorcluster)  [unwired: 6 in, 1 out]
      }
      frame "基本参数设" {
        n648 = call "SetTestInfoIndex.vi"("test info index"=11) -> ()
        n649 = call "UI-BaseParamSet.vi"("error in (no error)"=w1588) -> ("error out"=w1587:errorcluster)  [unwired: 10 in]
        n650 = call "Enqueue Element Array.vi"("device error in"=w1587, "queue index"=0, "error in"=w1588, "master data"="" ("Element 1"), "queue in"=w1594) -> ("error out"=w1593:errorcluster)  [unwired: 5 in, 1 out]
      }
      frame "型号选择" {
        n651 = call "SetTestInfoIndex.vi"("test info index"=11) -> ()
        n652 = flat-sequence {
          tunnel: w1598 -> [w1607]
          tunnel: [w1607] -> w1596
          tunnel: [w1610] -> w1597
          tunnel: w1596 -> [w1611]
          frame #0 {
            n653 = local read "Start"() -> (w1606:T14)
            n654 = case shown="假" w1606 {
              frame False {
                n655 = global write "Global System.vi" "产品型号选择 EXIT"(TRUE ("产品型号选择 EXIT")) -> ()
              }
              frame True {
                n656 = global write "Global System.vi" "产品型号选择 EXIT"(FALSE ("产品型号选择 EXIT")) -> ()
              }
            }
          }
          frame #1 {
            n657 = call "Product model selection.vi"("error in (no error)"=w1611) -> ("error in (no error) 2"=w1610:errorcluster)  [unwired: 10 in]
          }
        }
        n658 = call "Enqueue Element Array.vi"("device error in"=w1597, "queue index"=0, "error in"=w1598, "master data"="" ("Element 1"), "queue in"=w1604) -> ("error out"=w1603:errorcluster)  [unwired: 5 in, 1 out]
      }
      frame "产品新增" {
        n659 = call "SetTestInfoIndex.vi"("test info index"=11) -> ()
        n660 = flat-sequence {
          tunnel: w1614 -> [w1623]
          tunnel: [w1623] -> w1612
          tunnel: [w1624] -> w1613
          tunnel: w1612 -> [w1625]
          frame #0 {
            n661 = global write "Global System.vi" "产品型号选择 EXIT"(FALSE ("产品型号选择 EXIT")) -> ()
          }
          frame #1 {
            n662 = call "产品新增.vi"("error in (no error)"=w1625) -> ("error in (no error) 2"=w1624:errorcluster)  [unwired: 10 in]
          }
        }
        n663 = call "Enqueue Element Array.vi"("device error in"=w1613, "queue index"=0, "error in"=w1614, "master data"="" ("Element 1"), "queue in"=w1620) -> ("error out"=w1619:errorcluster)  [unwired: 5 in, 1 out]
      }
      frame "数据库清理" {
        n664 = global read "Global System.vi" "ADODB._Connection Out"() -> (w1626:refnum<k7>)
        n665 = call "SetTestInfoIndex.vi"("test info index"=11) -> ()
        n666 = Two Button Dialog(message="清空数据库" ("消息")) -> (T button?=w1630:bool)  [unwired: 2 in]
        n667 = case shown="真" w1630 {
          tunnel: w1628 -> [w1644 w1654]
          tunnel: [w1644 w1653] -> w1627
          tunnel: w1626 -> [_ w1645]
          frame False {
          }
          frame True {
            n668 = local read "computer1"() -> (w1652:bool)
            n669 = local read "computer2"() -> (w1651:bool)
            n670 = local read "computer3"() -> (w1650:bool)
            n671 = local read "computer4"() -> (w1649:bool)
            n672 = local read "computer5"() -> (w1648:bool)
            n673 = local read "Type_b"() -> (w1646:bool)
            n674 = local read "Type_c"() -> (w1647:bool)
            n675 = call "SQL-选择清空数据库.vi"("computer1"=w1652, "computer 2"=w1651, "ADODB._Connection Out"=w1645, "computer 3"=w1650, "computer 4"=w1649, "error in (no error)"=w1654, "type_c"=w1647, "computer 5"=w1648, "type_b"=w1646) -> ("error out"=w1653:errorcluster)  [unwired: 9 in, 1 out]
          }
        }
        n676 = property on="选项卡控件" class="TabCtl (严格)"("Value"=T2."Data and Run Information " ("选项卡控件")) -> ()  [unwired: 2 in, 2 out]
        n677 = disable-structure shown="禁用" {
          frame Disabled {
            n678 = case shown="\"computer1\"" {
              selector: _ -> [_ _ _ _ _]
              frame "computer2", Default {
                n679 = call "SQL-清空数据库信息.vi"("字符串"="truncate table computer2;" ("Command Text")) -> ()  [unwired: 10 in, 1 out]
              }
              frame "computer1" {
                n680 = call "SQL-清空数据库信息.vi"("字符串"="truncate table computer1;" ("Command Text")) -> ()  [unwired: 10 in, 1 out]
              }
              frame "computer3" {
                n681 = call "SQL-清空数据库信息.vi"("字符串"="truncate table computer3;" ("Command Text")) -> ()  [unwired: 10 in, 1 out]
              }
              frame "computer4" {
                n682 = call "SQL-清空数据库信息.vi"("字符串"="truncate table computer4;" ("Command Text")) -> ()  [unwired: 10 in, 1 out]
              }
              frame "computer5" {
                n683 = call "SQL-清空数据库信息.vi"("字符串"="truncate table computer5;" ("Command Text")) -> ()  [unwired: 10 in, 1 out]
              }
            }
          }
          frame Enabled {
          }
        }
        n684 = call "Enqueue Element Array.vi"("device error in"=w1627, "queue index"=0, "error in"=w1628, "master data"="" ("Element 1"), "queue in"=w1637) -> ("error out"=w1636:errorcluster)  [unwired: 5 in, 1 out]
      }
      frame "Save 压力表数据库 Message" {
        (unwired) path "D:/Inspect System/Source Code/压力表型号数据库.txt" ("file path (dialog if empty)")
        n685 = call "SetTestInfoIndex.vi"("test info index"=11) -> ()
        n686 = Two Button Dialog(message="数据保存成功" ("消息"), 1:"取消" ("按钮名称（“确定”）"), 2:"确定" ("T按钮名称（“确定”）")) -> (T button?=w1656:bool)
        n687 = property on="选项卡控件" class="TabCtl (严格)"("Value"=T2."Machine Alarm History" ("选项卡控件")) -> ()  [unwired: 2 in, 2 out]
        n688 = case shown="真" w1656 {
          frame False {
          }
          frame True {
            (unwired) TRUE ("append to file? (new file:F)")
            n689 = Index Array(array="压力表数据库", index (col) #1=0 ("禁用的索引 (列)"), index (col) #2=1 ("禁用的索引 (列)"), index (col) #3=2 ("禁用的索引 (列)")) -> (element #1=w1683:string[], element #2=w1682:string[], element #3=w1681:string[])  [unwired: 3 in]
            n690 = global read "Global System.vi" "ref path"() -> (w1673:path)
            n691 = Index Array(array="压力表打印代码据库") -> (element=w1669:string[])  [unwired: 2 in]
            n692 = Build Path(base path=w1673, name or relative path="压力表型号数据库.txt" ("名称或相对路径")) -> (appended path=w1674:path)
            n693 = Build Array(w1683, w1682, w1681) -> (w1677:string[][])
            n694 = Build Path(base path=w1673, name or relative path="压力表打印代码.txt" ("名称或相对路径")) -> (appended path=w1668:path)
            n695 = call-poly <vilib>:"Write Delimited Spreadsheet.vi"("file path (dialog if empty)"=w1668, "1D data"=w1669, "transpose? (no:F)"=TRUE) -> ()  [unwired: 11 in, 2 out]
            n696 = call-poly <vilib>:"Write Delimited Spreadsheet.vi"("file path (dialog if empty)"=w1674, "2D data"=w1677, "append to file? (new file:F)"=TRUE, "transpose? (no:F)"=TRUE) -> ()  [unwired: 10 in, 2 out]
          }
        }
        n697 = call "Enqueue Element Array.vi"("queue index"=0, "error in"=w1659, "master data"="" ("Element 1"), "queue in"=w1666) -> ("error out"=w1665:errorcluster)  [unwired: 6 in, 1 out]
      }
      frame "产品型号删除" {
        n698 = call "SetTestInfoIndex.vi"("test info index"=11) -> ()
        n699 = flat-sequence {
          tunnel: w1688 -> [w1697]
          tunnel: [w1697] -> w1686
          tunnel: [w1698] -> w1687
          tunnel: w1686 -> [w1699]
          frame #0 {
            n700 = global write "Global System.vi" "产品型号选择 EXIT"(FALSE ("产品型号选择 EXIT")) -> ()
          }
          frame #1 {
            n701 = call "产品删除.vi"("error in (no error)"=w1699) -> ("error in (no error) 2"=w1698:errorcluster)  [unwired: 10 in]
          }
        }
        n702 = call "Enqueue Element Array.vi"("device error in"=w1687, "queue index"=0, "error in"=w1688, "master data"="" ("Element 1"), "queue in"=w1694) -> ("error out"=w1693:errorcluster)  [unwired: 5 in, 1 out]
      }
      frame "Machine Inforamtion" {
        w1701 = TRUE
        n703 = call "SetTestInfoIndex.vi"("test info index"=11) -> ()
        n704 = property on="选项卡控件" class="TabCtl (严格)"("Value"=T2."Machine Information" ("选项卡控件")) -> ()  [unwired: 2 in, 2 out]
        n705 = call "Read Machine Component Models.vi"("名称或相对路径"="Machine Compoent models.txt") -> ()  [unwired: 10 in, 1 out]
        n706 = property on="Machine Paramter and Control" class="Bool (严格)"("Value"=w1701) -> ()  [unwired: 2 in, 2 out]
        n707 = property on="Vision Paramter and Control" class="Bool (严格)"("Value"=w1701) -> ()  [unwired: 2 in, 2 out]
        n708 = property on="Machine Alarm Histroy" class="Bool (严格)"("Value"=w1701) -> ()  [unwired: 2 in, 2 out]
        n709 = property on="Data and Run Information" class="Bool (严格)"("Value"=w1701) -> ()  [unwired: 2 in, 2 out]
        n710 = property on="Start" class="Bool (严格)"("Value"=w1701) -> ()  [unwired: 2 in, 2 out]
        n711 = property on="Pause" class="Bool (严格)"("Value"=w1701) -> ()  [unwired: 2 in, 2 out]
        n712 = property on="Stop" class="Bool (严格)"("Value"=w1701) -> ()  [unwired: 2 in, 2 out]
        n713 = property on="Open Image File" class="Bool (严格)"("Value"=w1701) -> ()  [unwired: 2 in, 2 out]
        n714 = property on="Open Excel File" class="Bool (严格)"("Value"=w1701) -> ()  [unwired: 2 in, 2 out]
        n715 = property on="Home" class="Bool (严格)"("Value"=w1701) -> ()  [unwired: 2 in, 2 out]
        n716 = property on="User Login" class="Bool (严格)"("Value"=w1701) -> ()  [unwired: 2 in, 2 out]
        n717 = call "Enqueue Element Array.vi"("queue index"=0, "error in"=w1704, "master data"="" ("Element 1"), "queue in"=w1709) -> ("error out"=w1708:errorcluster)  [unwired: 6 in, 1 out]
      }
      frame "SOP帮助" {
        (unwired) "C:\\Users\\Administrator\\Desktop\\实验图片\\铜垫片检测\\LX Inspect System\\Source Code\\GRR模板\\Foot 段差检测机-操作指导书.docx" ("command line")
        n718 = call "SetTestInfoIndex.vi"("test info index"=11) -> ()
        n719 = disable-structure shown="禁用" {
          disable-tunnel: w1712 -> [w1721 w1726]
          disable-tunnel: [w1720 w1726] -> w1711
          frame Disabled {
            n720 = global read "Global System.vi" "ref path"() -> (w1725:path)
            n721 = Build Path(base path=w1725, name or relative path="SOP.docx" ("名称或相对路径")) -> (appended path=w1723:path)
            n722 = Path To String(path=w1723) -> (string=w1722:string)
            n723 = call <vilib>:"System Exec.vi"("error in (no error)"=w1721, "command line"=w1722) -> ("error out"=w1720:errorcluster)  [unwired: 6 in, 3 out]
          }
          frame Enabled {
          }
        }
        n724 = call "Enqueue Element Array.vi"("device error in"=w1711, "queue index"=0, "error in"=w1712, "master data"="" ("Element 1"), "queue in"=w1718) -> ("error out"=w1717:errorcluster)  [unwired: 5 in, 1 out]
      }
      frame "Vision Paramter and Control" {
        w1727 = TRUE
        n725 = call "SetTestInfoIndex.vi"("test info index"=11) -> ()
        n726 = property on="选项卡控件" class="TabCtl (严格)"("Value"=T2."Vision Paramter and Contorol" ("选项卡控件")) -> ()  [unwired: 2 in, 2 out]
        n727 = property on="Machine Paramter and Control" class="Bool (严格)"("Value"=w1727) -> ()  [unwired: 2 in, 2 out]
        n728 = property on="Machine Alarm Histroy" class="Bool (严格)"("Value"=w1727) -> ()  [unwired: 2 in, 2 out]
        n729 = property on="Data and Run Information" class="Bool (严格)"("Value"=w1727) -> ()  [unwired: 2 in, 2 out]
        n730 = property on="Machine Inforamtion" class="Bool (严格)"("Value"=w1727) -> ()  [unwired: 2 in, 2 out]
        n731 = property on="Start" class="Bool (严格)"("Value"=w1727) -> ()  [unwired: 2 in, 2 out]
        n732 = property on="Pause" class="Bool (严格)"("Value"=w1727) -> ()  [unwired: 2 in, 2 out]
        n733 = property on="Stop" class="Bool (严格)"("Value"=w1727) -> ()  [unwired: 2 in, 2 out]
        n734 = property on="Open Image File" class="Bool (严格)"("Value"=w1727) -> ()  [unwired: 2 in, 2 out]
        n735 = property on="Open Excel File" class="Bool (严格)"("Value"=w1727) -> ()  [unwired: 2 in, 2 out]
        n736 = property on="User Login" class="Bool (严格)"("Value"=w1727) -> ()  [unwired: 2 in, 2 out]
        n737 = property on="Home" class="Bool (严格)"("Value"=w1727) -> ()  [unwired: 2 in, 2 out]
        n738 = call "Enqueue Element Array.vi"("queue index"=0, "error in"=w1730, "master data"="" ("Element 1"), "queue in"=w1735) -> ("error out"=w1734:errorcluster)  [unwired: 6 in, 1 out]
      }
      frame "Machine Alarm Histroy" {
        w1737 = TRUE
        n739 = call "SetTestInfoIndex.vi"("test info index"=11) -> ()
        n740 = property on="选项卡控件" class="TabCtl (严格)"("Value"=T2."Machine Alarm History" ("选项卡控件")) -> ()  [unwired: 2 in, 2 out]
        n741 = property on="Machine Paramter and Control" class="Bool (严格)"("Value"=w1737) -> ()  [unwired: 2 in, 2 out]
        n742 = property on="Vision Paramter and Control" class="Bool (严格)"("Value"=w1737) -> ()  [unwired: 2 in, 2 out]
        n743 = property on="Data and Run Information" class="Bool (严格)"("Value"=w1737) -> ()  [unwired: 2 in, 2 out]
        n744 = property on="Machine Inforamtion" class="Bool (严格)"("Value"=w1737) -> ()  [unwired: 2 in, 2 out]
        n745 = property on="Start" class="Bool (严格)"("Value"=w1737) -> ()  [unwired: 2 in, 2 out]
        n746 = property on="Pause" class="Bool (严格)"("Value"=w1737) -> ()  [unwired: 2 in, 2 out]
        n747 = property on="Stop" class="Bool (严格)"("Value"=w1737) -> ()  [unwired: 2 in, 2 out]
        n748 = property on="Open Image File" class="Bool (严格)"("Value"=w1737) -> ()  [unwired: 2 in, 2 out]
        n749 = property on="Open Excel File" class="Bool (严格)"("Value"=w1737) -> ()  [unwired: 2 in, 2 out]
        n750 = property on="Home" class="Bool (严格)"("Value"=w1737) -> ()  [unwired: 2 in, 2 out]
        n751 = property on="User Login" class="Bool (严格)"("Value"=w1737) -> ()  [unwired: 2 in, 2 out]
        n752 = call "Enqueue Element Array.vi"("queue index"=0, "error in"=w1740, "master data"="" ("Element 1"), "queue in"=w1745) -> ("error out"=w1744:errorcluster)  [unwired: 6 in, 1 out]
      }
      frame "Data and Run Information" {
        w1747 = TRUE
        n753 = call "SetTestInfoIndex.vi"("test info index"=11) -> ()
        n754 = property on="选项卡控件" class="TabCtl (严格)"("Value"=T2."Data and Run Information " ("选项卡控件")) -> ()  [unwired: 2 in, 2 out]
        n755 = property on="Machine Paramter and Control" class="Bool (严格)"("Value"=w1747) -> ()  [unwired: 2 in, 2 out]
        n756 = property on="Vision Paramter and Control" class="Bool (严格)"("Value"=w1747) -> ()  [unwired: 2 in, 2 out]
        n757 = property on="Machine Alarm Histroy" class="Bool (严格)"("Value"=w1747) -> ()  [unwired: 2 in, 2 out]
        n758 = property on="Machine Inforamtion" class="Bool (严格)"("Value"=w1747) -> ()  [unwired: 2 in, 2 out]
        n759 = property on="Start" class="Bool (严格)"("Value"=w1747) -> ()  [unwired: 2 in, 2 out]
        n760 = property on="Pause" class="Bool (严格)"("Value"=w1747) -> ()  [unwired: 2 in, 2 out]
        n761 = property on="Stop" class="Bool (严格)"("Value"=w1747) -> ()  [unwired: 2 in, 2 out]
        n762 = property on="Open Image File" class="Bool (严格)"("Value"=w1747) -> ()  [unwired: 2 in, 2 out]
        n763 = property on="Open Excel File" class="Bool (严格)"("Value"=w1747) -> ()  [unwired: 2 in, 2 out]
        n764 = property on="Home" class="Bool (严格)"("Value"=w1747) -> ()  [unwired: 2 in, 2 out]
        n765 = property on="User Login" class="Bool (严格)"("Value"=w1747) -> ()  [unwired: 2 in, 2 out]
        n766 = call "Enqueue Element Array.vi"("queue index"=0, "error in"=w1750, "master data"="" ("Element 1"), "queue in"=w1755) -> ("error out"=w1754:errorcluster)  [unwired: 6 in, 1 out]
      }
      frame "Open Image File" {
        w1762 = TRUE
        n767 = call "SetTestInfoIndex.vi"("test info index"=11) -> ()
        n768 = property on="Machine Paramter and Control" class="Bool (严格)"("Value"=w1762) -> ()  [unwired: 2 in, 2 out]
        n769 = property on="Vision Paramter and Control" class="Bool (严格)"("Value"=w1762) -> ()  [unwired: 2 in, 2 out]
        n770 = property on="Machine Alarm Histroy" class="Bool (严格)"("Value"=w1762) -> ()  [unwired: 2 in, 2 out]
        n771 = property on="Data and Run Information" class="Bool (严格)"("Value"=w1762) -> ()  [unwired: 2 in, 2 out]
        n772 = property on="Machine Inforamtion" class="Bool (严格)"("Value"=w1762) -> ()  [unwired: 2 in, 2 out]
        n773 = property on="Home" class="Bool (严格)"("Value"=w1762) -> ()  [unwired: 2 in, 2 out]
        n774 = property on="Start" class="Bool (严格)"("Value"=w1762) -> ()  [unwired: 2 in, 2 out]
        n775 = property on="Pause" class="Bool (严格)"("Value"=w1762) -> ()  [unwired: 2 in, 2 out]
        n776 = property on="Stop" class="Bool (严格)"("Value"=w1762) -> ()  [unwired: 2 in, 2 out]
        n777 = property on="Open Excel File" class="Bool (严格)"("Value"=w1762) -> ()  [unwired: 2 in, 2 out]
        n778 = property on="User Login" class="Bool (严格)"("Value"=w1762) -> ()  [unwired: 2 in, 2 out]
        n779 = property on="选项卡控件" class="TabCtl (严格)"("Value"=T2."Open Image File" ("选项卡控件")) -> ()  [unwired: 2 in, 2 out]
        n780 = call <vilib>:"Recursive File List.vi"("error in (no error)"=w1758, "Folder Path"=path "D:/Data/History Image") -> ("error out"=w1760:errorcluster, "dup Folder Path"=w1761:path)  [unwired: 5 in, 3 out]
        n781 = List Folder(path=w1761, error in=w1760) -> (error out=w1757:errorcluster)  [unwired: 2 in, 3 out]
        n782 = call "Enqueue Element Array.vi"("queue index"=0, "error in"=w1757, "master data"="" ("Element 1"), "queue in"=w1769) -> ("error out"=w1768:errorcluster)  [unwired: 6 in, 1 out]
      }
      frame "Search Histroy Image" {
        n783 = property on="NG/OK" class="CmbBox"() -> ("Value"=w1777:string)  [unwired: 2 in, 2 out]
        n784 = property on="检索条件" class="CmbBox"() -> ("Value"=w1778:string)  [unwired: 2 in, 2 out]
        n785 = call "SetTestInfoIndex.vi"("test info index"=11) -> ()
        n786 = call "TSP-搜索树形列表.vi"("error in (no error)"=w1779, "NG/OK"=w1777, "检索条件"=w1778) -> ("错误输出"=w1776:errorcluster, "项缩进层次"=w1772:i32[], "项名称"=w1773:string[], "All Files in Dir"=→"All Files in Dir":path[])  [unwired: 4 in, 1 out]
        "项名称" <- w1773
        n787 = invoke on="搜索项" class="Tree (严格)" method="Edit Tree Items.Delete"(error in=w1776) -> (error out=w1775:errorcluster)  [unwired: 4 in, 4 out]
        n788 = for {
          shift-right: [w1789] -> w1774
          shift-left: w1775 -> [w1790]
          tunnel: w1773 -> [w1788] mode=indexing
          tunnel: w1772 -> [w1787] mode=indexing
          n789 = invoke on="搜索项" class="Tree (严格)" method="Edit Tree Items.Add Item to End"(error in=w1790, "Left Cell"=w1788, "Item Indent"=w1787) -> (error out=w1789:errorcluster)  [unwired: 5 in, 7 out]
        }
        n790 = call "Enqueue Element Array.vi"("device error in"=w1774, "queue index"=0, "error in"=w1779, "master data"="" ("Element 1"), "queue in"=w1785) -> ("error out"=w1784:errorcluster)  [unwired: 5 in, 1 out]
      }
      frame "Open Excel File" {
        n791 = call "SetTestInfoIndex.vi"("test info index"=11) -> ()
        n792 = property on="选项卡控件" class="TabCtl (严格)"("Value"=T2."Open Excel File" ("选项卡控件")) -> ()  [unwired: 2 in, 2 out]
        n793 = Build Path(base path=path "D:/Inspect System/Source Code" ("基路径"), name or relative path="data" ("名称或相对路径")) -> (appended path=w1797:path)
        n794 = call <vilib>:"Recursive File List.vi"("Folder Path"=w1797) -> ("error out"=w1800:errorcluster, "dup Folder Path"=w1799:path)  [unwired: 6 in, 3 out]
        n795 = call "TSP-搜索树形列表（表格）.vi"() -> ("错误输出"=w1794:errorcluster, "项缩进层次"=w1793:i32[], "项名称"=w1792:string[], "All Files in Dir"=→"All Files in Dir 2":path[])  [unwired: 7 in, 1 out]
        "项名称 2" <- w1792
        n796 = List Folder(path=w1799, error in=w1800) -> ()  [unwired: 2 in, 4 out]
        n797 = invoke on="文件名" class="Tree (严格)" method="Edit Tree Items.Delete"(error in=w1794) -> (error out=w1795:errorcluster)  [unwired: 4 in, 4 out]
        n798 = for {
          shift-right: [w1810] -> _
          shift-left: w1795 -> [w1811]
          tunnel: w1792 -> [w1813] mode=indexing
          tunnel: w1793 -> [w1812] mode=indexing
          n799 = invoke on="文件名" class="Tree (严格)" method="Edit Tree Items.Add Item to End"(error in=w1811, "Left Cell"=w1813, "Item Indent"=w1812) -> (error out=w1810:errorcluster)  [unwired: 5 in, 7 out]
        }
        n800 = call "Enqueue Element Array.vi"("queue index"=0, "error in"=w1803, "master data"="" ("Element 1"), "queue in"=w1808) -> ("error out"=w1807:errorcluster)  [unwired: 6 in, 1 out]
      }
      frame "P Chart Select" {
        n801 = call "SetTestInfoIndex.vi"("test info index"=11) -> ()
        n802 = call "Enqueue Element Array.vi"("queue index"=0, "error in"=w1816, "master data"="" ("Element 1"), "queue in"=w1814) -> ("error out"=w1820:errorcluster)  [unwired: 6 in, 1 out]
      }
      frame "----------数据查询----------" {
      }
      frame "*Error handler" {
        n803 = call "SetTestInfoIndex.vi"("test info index"=5) -> ()
        n804 = call "GeneralErrorHandler.vi"("secondary data"=w1828) -> ("stop?"=w1827:bool)  [unwired: 7 in, 1 out]
        n805 = case shown="真" w1827 {
          tunnel: [_ "*Reset device"] -> w1826
          tunnel: [_ w1835] -> w1825
          frame False {
          }
          frame True {
            n806 = Build Array("*Exit application" ("Element 1")) -> (w1835:string[])
          }
        }
        n807 = call "Enqueue Element Array.vi"("queue index"=0, "error in"=w1831, "secondary data"=w1825, "master data"=w1826, "queue in"=w1832) -> ("error out"=w1830:errorcluster)  [unwired: 5 in, 1 out]
      }
      frame "*Exit application" {
        n808 = call "SetTestInfoIndex.vi"("test info index"=7) -> ()
      }
      frame "----------9----------" {
      }
      frame "No event", Default {
        # "Don't place any functions"
        n809 = call "SetTestInfoIndex.vi"("test info index"=-1) -> ()
      }
      frame "Template case" {
        n810 = call "SetTestInfoIndex.vi"("test info index"=-1) -> ()
        n811 = call "Enqueue Element Array.vi"("queue index"=0, "error in"=w1851, "master data"="" ("Element 1"), "queue in"=w1855) -> ("error out"=w1854:errorcluster)  [unwired: 6 in, 1 out]
      }
    }
    n812 = Unbundle By Name(w1244) -> ("status"=w1249:bool)
    n813 = Or(x=w1248, y=w1249) -> (x .or. y?=w1250:bool)
    n814 = Wait (ms)(milliseconds to wait=w1247) -> ()  [unwired: 1 out]
  }
  n815 = while "While循环" {
    shift-right: [w1873] -> w32
    shift-left: w2 -> [w1869]
    shift-right: [w1870] -> _
    shift-left: w14 -> [w1871]
    tunnel: w15 -> [w1865]
    tunnel: w7 -> [w1858]
    tunnel: w8 -> [w1859]
    tunnel: w1 -> [w1857]
    stop <- w1864 stop-if-true
    # "处理部分事件；处理部分弹出窗口（目的是避免在其他循环中因为弹出窗口而影响整个循环的运行）"
    # "主线程-穿管检测"
    n816 = call "Dequeue Element Array.vi"("queue in"=w1865, "queue index"=6, "error in"=w1869) -> ("queue out"=w1868:T25, "master data"=w1867:string, "secondary data"=w1866:string[], "error out"=w1864:errorcluster)  [unwired: 2 in, 1 out]
    n817 = case shown="\"数据获取\"" w1867 {
      selector: w1867 -> [_ _ w1888 w1908 w1926 w1939 w1952 w1967 _ _ _ _ w2050 w2078 w2108 w2118 w2137 w2178 w2234 w2256 w2274 _ w2302 w2318 w2328 w2339 w2349 _]
      tunnel: w1868 -> [_ _ w1902 w1918 w1935 w1949 w1963 w1980 w2001 w2011 w2024 w2036 w2059 w2088 w2115 w2126 w2142 w2183 w2239 w2261 w2285 w2294 w2308 w2324 w2334 w2345 w2356 w2361]
      tunnel: w1864 -> [w1875 w1879 w1889 w1906 w1925 w1940 w1953 w1968 w1993 w2007 w2020 w2032 w2042 w2079 w2089 w2117 w2134 w2170 w2215 w2254 w2281 w2291 w2305 w2321 w2331 w2342 w2352 w2358]
      tunnel: [w1875 w1879 w1901 w1917 w1924 w1948 w1962 w1979 w2000 w2010 w2023 w2035 w2058 w2087 w2114 w2131 w2147 w2188 w2244 w2266 w2284 w2293 w2307 w2323 w2333 w2344 w2355 w2369] -> w1873
      tunnel: [50 50 10 10 10 10 10 10 w1996 50 20 30 10 10 w2103 w2127 w2143 w2184 w2240 w2262 w2273 50 50 50 50 50 50 50] -> w1872
      tunnel: w1871 -> [w1876 w1880 w1883 w1904 w1920 w1937 w1951 w1966 w1983 w2008 w2014 w2026 w2048 w2076 w2106 w2116 w2132 w2160 w2232 w2253 w2282 w2288 w2301 w2314 w2326 w2336 w2353 w2367]
      tunnel: [w1876 w1880 w1890 w1904 w1920 w1937 w1951 w1966 w1983 w2008 w2014 w2026 w2048 w2076 w2106 w2116 w2132 w2160 w2232 w2253 w2282 w2288 w2301 w2313 w2326 w2336 w2353 w2367] -> w1870
      tunnel: w1866 -> [_ _ _ _ _ _ _ _ _ _ _ _ _ _ _ _ _ _ _ _ _ _ _ _ _ _ _ _]
      tunnel: "穿管检测 : " -> [_ _ w1891 w1910 w1928 w1945 w1959 w1976 w1990 _ _ _ w2052 w2081 w2109 w2128 w2144 w2185 w2241 w2263 _ _ w2300 _ _ w2338 _ _]
      tunnel: "T4:" -> [_ _ _ _ _ _ _ _ _ _ _ _ _ _ _ _ _ _ _ _ _ _ _ _ _ _ w2348 _]
      tunnel: 5 -> [_ _ _ _ _ _ _ _ w1996 _ _ _ _ _ w2103 w2127 w2143 w2184 w2240 w2262 w2273 _ _ _ _ _ _ _]
      tunnel: w1859 -> [_ _ _ _ _ _ _ _ _ _ _ _ _ _ _ _ _ w2150 w2222 _ _ _ _ _ _ _ _ _]
      tunnel: w1858 -> [_ _ _ _ _ _ _ _ _ _ _ _ _ _ _ _ _ w2149 w2219 _ _ _ _ _ _ _ _ _]
      tunnel: w1857 -> [_ _ _ _ _ _ _ _ _ _ _ _ _ _ _ _ _ _ w2214 _ _ _ _ _ _ _ _ _]
      frame "No event", Default {
        # "Don't place any functions"
      }
      frame "EMG" {
        # "Don't place any functions"
        n818 = local write "设备状态"("") -> ()
      }
      frame "Loading Variable" {
        w1899 = u16 0 items=["HPRI"=1, "LPRI"=0] ("priority")
        n819 = control-ref of="设备状态"() -> (w1895:refnum<vi>)
        n820 = call "设备状态循环显示.vi"("cmd:"=w1891, "Str引用句柄"=w1895, "新信息输入"=w1888) -> ()  [unwired: 9 in]
        n821 = call "Read Config InI.vi"("名称或相对路径"="UserDefine.ini") -> ("ParamSet"=w1898:string[])  [unwired: 14 in, 4 out]
        n822 = Index Array(array=w1898, index #1=0 ("索引")) -> (element #1=w1882:string)  [unwired: 1 in, 1 out]
        n823 = global read "Global System.vi" "ref path"() -> (w1887:path)
        n824 = property on="Auto Run Load Program Name" class="CmbBox"("Value"=w1882) -> ()  [unwired: 2 in, 2 out]
        n825 = Build Path(base path=w1887, name or relative path="Template Program" ("名称或相对路径")) -> (appended path=w1885:path)
        n826 = Build Path(base path=w1885, name or relative path=w1882) -> (appended path=→"CCD1":path)
        n827 = global read "Global System.vi" "Paus"() -> (w1893:bool)
        n828 = call "KB-EMG Input.vi"("Other Message"="Loading Variable Config" ("Element 1"), "EMG Iput"="EMG", "Emg"=w1893) -> ("String OutPut"=w1881:string)  [unwired: 8 in]
        n829 = Bundle By Name(cluster=w1883, "2 Pause Message"=w1881, "LoadProgram"=w1882) -> (w1890:T21)
        n830 = call "Enqueue Element Array.vi"("priority"=w1899, "queue index"=6, "error in"=w1889, "master data"=w1881, "queue in"=w1902) -> ("error out"=w1901:errorcluster)  [unwired: 5 in, 1 out]
      }
      frame "Loading Variable Config" {
        w1915 = u16 0 items=["HPRI"=1, "LPRI"=0] ("priority")
        n831 = control-ref of="设备状态"() -> (w1914:refnum<vi>)
        n832 = Unbundle By Name(w1904) -> ("LoadProgram"=w1907:string)
        n833 = call "设备状态循环显示.vi"("cmd:"=w1910, "Str引用句柄"=w1914, "新信息输入"=w1908) -> ()  [unwired: 9 in]
        n834 = call "读取产品参数信息-CCD1CCD2.vi"("错误输入（无错误）"=w1906, "LoadProductName"=w1907) -> ("错误输出"=w1905:errorcluster)  [unwired: 9 in]
        n835 = global read "Global System.vi" "Paus"() -> (w1912:bool)
        n836 = call "KB-EMG Input.vi"("Other Message"="Initial CCD" ("Element 1"), "EMG Iput"="EMG", "Emg"=w1912) -> ("String OutPut"=w1909:string)  [unwired: 8 in]
        n837 = call "Enqueue Element Array.vi"("priority"=w1915, "device error in"=w1905, "queue index"=6, "error in"=w1906, "master data"=w1909, "queue in"=w1918) -> ("error out"=w1917:errorcluster)  [unwired: 4 in, 1 out]
      }
      frame "Initial CCD" {
        w1933 = u16 0 items=["HPRI"=1, "LPRI"=0] ("priority")
        n838 = control-ref of="设备状态"() -> (w1932:refnum<vi>)
        n839 = call "设备状态循环显示.vi"("cmd:"=w1928, "Str引用句柄"=w1932, "新信息输入"=w1926) -> ()  [unwired: 9 in]
        n840 = call "CR-Initial CameraCCD12.vi"("error in (no error)"=w1925) -> ("error out"=w1923:errorcluster, "Session Out 2"=w1921:T28, "Session Out"=w1922:T28)  [unwired: 8 in]
        n841 = global write "Global System.vi" "Session Out CCD3"(w1921) -> ()
        n842 = global write "Global System.vi" "Session Out CCD2"(w1922) -> ()
        n843 = global read "Global System.vi" "Paus"() -> (w1930:bool)
        n844 = call "KB-EMG Input.vi"("Other Message"="Open Telnet" ("Element 1"), "EMG Iput"="EMG", "Emg"=w1930) -> ("String OutPut"=w1927:string)  [unwired: 8 in]
        n845 = call "Enqueue Element Array.vi"("priority"=w1933, "device error in"=w1923, "queue index"=6, "error in"=w1925, "master data"=w1927, "queue in"=w1935) -> ("error out"=w1924:errorcluster)  [unwired: 4 in, 1 out]
      }
      frame "Open Telnet" {
        w1946 = u16 0 items=["HPRI"=1, "LPRI"=0] ("priority")
        n846 = control-ref of="设备状态"() -> (w1944:refnum<vi>)
        n847 = call "设备状态循环显示.vi"("cmd:"=w1945, "Str引用句柄"=w1944, "新信息输入"=w1939) -> ()  [unwired: 9 in]
        n848 = global read "Global System.vi" "Paus"() -> (w1942:bool)
        n849 = call "KB-EMG Input.vi"("Other Message"="Open VISA" ("master data"), "EMG Iput"="EMG", "Emg"=w1942) -> ("String OutPut"=w1938:string)  [unwired: 8 in]
        n850 = call "Enqueue Element Array.vi"("priority"=w1946, "queue index"=6, "error in"=w1940, "master data"=w1938, "queue in"=w1949) -> ("error out"=w1948:errorcluster)  [unwired: 5 in, 1 out]
      }
      frame "Open VISA" {
        w1960 = u16 0 items=["HPRI"=1, "LPRI"=0] ("priority")
        n851 = control-ref of="设备状态"() -> (w1958:refnum<vi>)
        n852 = call "设备状态循环显示.vi"("cmd:"=w1959, "Str引用句柄"=w1958, "新信息输入"=w1952) -> ()  [unwired: 9 in]
        n853 = global read "Global System.vi" "Paus"() -> (w1956:bool)
        n854 = call "KB-EMG Input.vi"("Other Message"="Create File" ("master data"), "EMG Iput"="EMG", "Emg"=w1956) -> ("String OutPut"=w1954:string)  [unwired: 8 in]
        n855 = call "Enqueue Element Array.vi"("priority"=w1960, "queue index"=6, "error in"=w1953, "master data"=w1954, "queue in"=w1963) -> ("error out"=w1962:errorcluster)  [unwired: 5 in, 1 out]
      }
      frame "Create File" {
        w1977 = u16 0 items=["HPRI"=1, "LPRI"=0] ("priority")
        n856 = control-ref of="设备状态"() -> (w1975:refnum<vi>)
        n857 = call "设备状态循环显示.vi"("cmd:"=w1976, "Str引用句柄"=w1975, "新信息输入"=w1967) -> ()  [unwired: 9 in]
        n858 = global read "Global System.vi" "ref path"() -> (w1970:path)
        n859 = call "保存判定Title文件.vi"("基路径"=w1970) -> ("路径"=→"路径":path, "路径 2"=→"夹爪压力保存路径":path)  [unwired: 4 in, 5 out]
        n860 = global read "Global System.vi" "Paus"() -> (w1973:bool)
        n861 = call "KB-EMG Input.vi"("Other Message"="Initial-Clear Variable" ("master data"), "EMG Iput"="EMG", "Emg"=w1973) -> ("String OutPut"=w1971:string)  [unwired: 8 in]
        n862 = call "Enqueue Element Array.vi"("priority"=w1977, "queue index"=6, "error in"=w1968, "master data"=w1971, "queue in"=w1980) -> ("error out"=w1979:errorcluster)  [unwired: 5 in, 1 out]
      }
      frame "Initial-Clear Variable" {
        w1998 = u16 0 items=["HPRI"=1, "LPRI"=0] ("priority")
        n863 = control-ref of="设备状态"() -> (w1992:refnum<vi>)
        n864 = call "设备状态循环显示.vi"("cmd:"=w1990, "Str引用句柄"=w1992, "新信息输入"="Initial Finish " ("字符串")) -> ()  [unwired: 9 in]
        n865 = Current VI's Menubar() -> (w1995:refnum<k9>)
        n866 = for {
          tunnel: w1995 -> [w2004]
          tunnel: string[] ["登陆"] -> [w2002] mode=indexing
          n867 = Set Menu Item Info(7:w2002, 9:TRUE ("已启用"), 10:w2002, 11:w2004) -> ()  [unwired: 3 in, 2 out]
        }
        n868 = property on="User Login" class="Bool (严格)"("DisabledEnum"=T22."Enabled" ("禁用"), "Visible"=TRUE ("可见")) -> ()  [unwired: 2 in, 2 out]
        n869 = global read "Global System.vi" "Paus"() -> (w1988:bool)
        n870 = local write "穿管检测初始化状态"(TRUE ("穿管检测初始化状态")) -> ()
        n871 = global write "Global System.vi" "G_Status 1"(TRUE ("G_Status 1")) -> ()
        n872 = call "KB-EMG Input.vi"("Other Message"="" ("Element 1"), "EMG Iput"="EMG", "Emg"=w1988) -> ("String OutPut"=w1986:string)  [unwired: 8 in]
        n873 = call "Enqueue Element Array.vi"("priority"=w1998, "queue index"=6, "error in"=w1993, "master data"=w1986, "queue in"=w2001) -> ("error out"=w2000:errorcluster)  [unwired: 5 in, 1 out]
      }
      frame "<----自动加工------------->" {
        w2005 = u16 0 items=["HPRI"=1, "LPRI"=0] ("priority")
        # "//读取配置文件"
        n874 = call "Enqueue Element Array.vi"("priority"=w2005, "queue index"=6, "error in"=w2007, "master data"="" ("Element 1"), "queue in"=w2011) -> ("error out"=w2010:errorcluster)  [unwired: 5 in, 1 out]
      }
      frame "自动开始" {
        w2021 = u16 0 items=["HPRI"=1, "LPRI"=0] ("priority")
        n875 = global write "Global System.vi" "G_Status 1"(TRUE ("G_Status 1")) -> ()
        n876 = global read "Global System.vi" "Paus"() -> (w2017:bool)
        n877 = call "KB-EMG Input.vi"("Other Message"="读取配置文件", "EMG Iput"="EMG", "Emg"=w2017) -> ("String OutPut"=w2016:string)  [unwired: 8 in]
        n878 = call "Enqueue Element Array.vi"("priority"=w2021, "queue index"=6, "error in"=w2020, "master data"=w2016, "queue in"=w2024) -> ("error out"=w2023:errorcluster)  [unwired: 5 in, 1 out]
      }
      frame "读取配置文件" {
        w2033 = u16 0 items=["HPRI"=1, "LPRI"=0] ("priority")
        n879 = global write "Global System.vi" "G_Status 1"(TRUE ("G_Status 1")) -> ()
        n880 = call "KB-EMG Input.vi"("Other Message"="Load Var1 ", "EMG Iput"="EMG", "Emg"=FALSE) -> ("String OutPut"=w2028:string)  [unwired: 8 in]
        n881 = call "Enqueue Element Array.vi"("priority"=w2033, "queue index"=6, "error in"=w2032, "master data"=w2028, "queue in"=w2036) -> ("error out"=w2035:errorcluster)  [unwired: 5 in, 1 out]
      }
      frame "检测CCD1,2穿管启动信号" {
        w2056 = u16 0 items=["HPRI"=1, "LPRI"=0] ("priority")
        n882 = local read "DB5000.X"() -> (w2039:T4)
        n883 = control-ref of="设备状态"() -> (w2053:refnum<vi>)
        n884 = Unbundle By Name(w2039) -> ("电脑1穿管检测\n触发-读"=w2038:bool, "电脑1压力获取\n触发-读"=w2037:bool)
        n885 = call "循环时状态显示.vi"("Str引用句柄"=w2053, "cmd:"=w2052, "新信息输入"=w2050) -> ()  [unwired: 9 in]
        n886 = Or(x="穿管触发", y=w2038) -> (x .or. y?=w2041:bool)
        n887 = Build Array(w2041, w2037) -> (w2046:bool[])
        n888 = call "上升沿检测.vi"("input"=w2041) -> ("output"=w2040:bool)  [unwired: 9 in, 1 out]
        n889 = Boolean Array To Number(Boolean array=w2046) -> (number=w2045:u32)
        "数字" <- w2045
        n890 = case shown="假" w2040 {
          tunnel: [w2060 w2062] -> w2043
          tunnel: w2042 -> [w2060 w2061]
          frame False {
          }
          frame True {
            n891 = disable-structure shown="禁用" {
              disable-tunnel: [w2067 _] -> w2062
              disable-tunnel: w2061 -> [w2066 _]
              frame Disabled {
                n892 = call "SQL穿管型号数据库读取.vi"("error in (no error)"=w2066) -> ("error out"=w2064:errorcluster, "已删除的部分"=→"穿管产品型号":string[], "元素"=w2065:string)  [unwired: 6 in, 2 out]
                n893 = call "SQL穿管型号删除.vi"("Type_c"=w2065, "error in (no error)"=w2064) -> ("error out"=w2067:errorcluster)  [unwired: 13 in]
              }
              frame Enabled {
              }
            }
          }
        }
        n894 = case shown="1" w2045 {
          tunnel: ["检测CCD1,2穿管启动信号" ("f") "穿管启动信号处理" ("EMG Iput") "数据获取" ("f")] -> w2044
          frame 0, Default {
          }
          frame 1 {
          }
          frame 2, 3 {
            n895 = disable-structure shown="启用" {
              frame Disabled {
                w2071 = dbl[] [0.0, 0.0, 0.0, 0.0, 0.0, 0.0, 0.0, 0.0, 0.0, 0.0, 0.0, 0.0, 0.0, 0.0, 0.0, 0.0, 0.0, 0.0, 0.0] ("盘管压力值")
                n896 = local write "盘管压力值 2"(w2071) -> ()
                n897 = local write "夹爪压力值"(w2071) -> ()
              }
              frame Enabled {
              }
            }
          }
        }
        n898 = call "KB-EMG Input.vi"("Other Message"=w2044, "EMG Iput"="EMG", "Emg"=FALSE) -> ("String OutPut"=w2054:string)  [unwired: 8 in]
        n899 = call "Enqueue Element Array.vi"("priority"=w2056, "device error in"=w2043, "queue index"=6, "error in"=w2042, "master data"=w2054, "queue in"=w2059) -> ("error out"=w2058:errorcluster)  [unwired: 4 in, 1 out]
      }
      frame "穿管启动信号处理" {
        w2085 = u16 0 items=["HPRI"=1, "LPRI"=0] ("priority")
        n900 = control-ref of="设备状态"() -> (w2082:refnum<vi>)
        n901 = call "循环时状态显示.vi"("Str引用句柄"=w2082, "cmd:"=w2081, "新信息输入"=w2078) -> ()  [unwired: 9 in]
        n902 = Select(t="Load Var1" ("EMG Iput"), s=FALSE, f="获取图像") -> (s? t:f=w2073:string)
        n903 = call "KB-EMG Input.vi"("Other Message"=w2073, "EMG Iput"="EMG", "Emg"=FALSE) -> ("String OutPut"=w2083:string)  [unwired: 8 in]
        n904 = call "Enqueue Element Array.vi"("priority"=w2085, "queue index"=6, "error in"=w2079, "master data"=w2083, "queue in"=w2088) -> ("error out"=w2087:errorcluster)  [unwired: 5 in, 1 out]
      }
      frame "获取图像" {
        (unwired) 150
        w2112 = u16 0 items=["HPRI"=1, "LPRI"=0] ("priority")
        n905 = control-ref of="设备状态"() -> (w2104:refnum<vi>)
        n906 = call "循环时状态显示.vi"("Str引用句柄"=w2104, "cmd:"=w2109, "新信息输入"=w2108) -> ()  [unwired: 9 in]
        n907 = global read "Global System.vi" "CCD2基础参数"() -> (w2094:T30)
        n908 = global read "Global System.vi" "Session Out CCD3"() -> (w2090:T28)
        n909 = global read "Global System.vi" "Session Out CCD2"() -> (w2091:T28)
        n910 = global read "Global System.vi" "CCD1基础参数"() -> (w2095:T30)
        n911 = call "AMX-CCD2获取图像.vi"("Session Out CCD3"=w2090, "error in (no error)"=w2089, "Image Name"="T2", "ParamsUI"=w2094) -> ("error out"=w2099:errorcluster, "Session Out"=w2092:T28, "Image out"=→"穿管相机2":T1)  [unwired: 4 in, 1 out]
        n912 = call "AMX-CCD1获取图像.vi"("Session Out CCD2"=w2091, "error in (no error)"=w2089, "Image Name"="I1", "ParamsUI"=w2095) -> ("error out"=w2101:errorcluster, "Session Out"=w2093:T28, "Image out"=→"穿管相机1":T1)  [unwired: 4 in, 1 out]
        n913 = global write "Global System.vi" "Session Out CCD3"(w2092) -> ()
        n914 = global write "Global System.vi" "Session Out CCD2"(w2093) -> ()
        n915 = Merge Errors(w2101, w2099) -> (w2100:errorcluster)
        n916 = call "KB-EMG Input.vi"("Other Message"="CCD1图像处理模块" ("EMG Iput"), "EMG Iput"="EMG", "Emg"=FALSE) -> ("String OutPut"=w2110:string)  [unwired: 8 in]
        n917 = call "Enqueue Element Array.vi"("priority"=w2112, "device error in"=w2100, "queue index"=6, "error in"=w2089, "master data"=w2110, "queue in"=w2115) -> ("error out"=w2114:errorcluster)  [unwired: 4 in, 1 out]
      }
      frame "Load Var1" {
        w2129 = u16 0 items=["HPRI"=1, "LPRI"=0] ("priority")
        n918 = control-ref of="设备状态"() -> (w2120:refnum<vi>)
        n919 = call "设备状态循环显示.vi"("cmd:"=w2128, "Str引用句柄"=w2120, "新信息输入"=w2118) -> ()  [unwired: 9 in]
        n920 = global read "Global System.vi" "ref path"() -> (w2125:path)
        n921 = call "保存判定Title文件.vi"("基路径"=w2125) -> ("路径"=w2124:path)  [unwired: 4 in, 6 out]
        n922 = property on="路径" class="Path"("Value"=w2124) -> ()  [unwired: 2 in, 2 out]
        n923 = call "KB-EMG Input.vi"("Other Message"="Load Var2" ("t"), "EMG Iput"="EMG", "Emg"=FALSE) -> ("String OutPut"=w2119:string)  [unwired: 8 in]
        n924 = call "Enqueue Element Array.vi"("priority"=w2129, "queue index"=6, "error in"=w2117, "master data"=w2119, "queue in"=w2126) -> ("error out"=w2131:errorcluster)  [unwired: 5 in, 1 out]
      }
      frame "Load Var2" {
        w2145 = u16 0 items=["HPRI"=1, "LPRI"=0] ("priority")
        n925 = control-ref of="设备状态"() -> (w2138:refnum<vi>)
        n926 = call "设备状态循环显示.vi"("cmd:"=w2144, "Str引用句柄"=w2138, "新信息输入"=w2137) -> ()  [unwired: 9 in]
        n927 = Unbundle By Name(w2132) -> ("LoadProgram"=w2135:string)
        n928 = call "读取产品参数信息-CCD1CCD2.vi"("错误输入（无错误）"=w2134, "LoadProductName"=w2135) -> ("错误输出"=w2133:errorcluster)  [unwired: 9 in]
        n929 = call "KB-EMG Input.vi"("Other Message"="检测CCD1,2穿管启动信号" ("t"), "EMG Iput"="EMG", "Emg"=FALSE) -> ("String OutPut"=w2136:string)  [unwired: 8 in]
        n930 = call "Enqueue Element Array.vi"("priority"=w2145, "device error in"=w2133, "queue index"=6, "error in"=w2134, "master data"=w2136, "queue in"=w2142) -> ("error out"=w2147:errorcluster)  [unwired: 4 in, 1 out]
      }
      frame "CCD1图像处理模块" {
        w2166 = path "D:/Data/History Image" ("基路径")
        w2186 = u16 0 items=["HPRI"=1, "LPRI"=0] ("priority")
        n931 = control-ref of="设备状态"() -> (w2179:refnum<vi>)
        n932 = call "设备状态循环显示.vi"("cmd:"=w2185, "Str引用句柄"=w2179, "新信息输入"=w2178) -> ()  [unwired: 9 in]
        n933 = local read "穿管相机1"() -> (w2176:T1)
        n934 = local read "穿管相机2"() -> (w2171:T1)
        n935 = call "AMX-CCD2 自动处理图像.vi"("Image In"=w2171, "error in (no error)"=w2170) -> ("Image Out"=w2165:T1, "NO LINES"=w2157:bool, "CCD2-L"=w2161:bool, "CCD2-R"=w2162:bool, "error out"=w2169:errorcluster)  [unwired: 9 in]
        n936 = call "AMX-CCD 自动处理图像.vi"("Image In"=w2176, "error in (no error)"=w2170) -> ("Image Out"=w2175:T1, "NO LINES"=w2158:bool, "CCD1-R"=w2163:bool, "CCD1-L"=w2164:bool, "error out"=w2172:errorcluster)  [unwired: 9 in]
        n937 = Merge Errors(w2172, w2169) -> (w2151:errorcluster)
        n938 = local write "穿管相机1"(w2175) -> ()
        n939 = local write "穿管相机2"(w2165) -> ()
        n940 = Not(x=w2158) -> (.not. x?=w2156:bool)
        n941 = Not(x=w2157) -> (.not. x?=w2155:bool)
        n942 = Compound Arithmetic op=AND "复合运算"(w2156, w2164, w2163, w2162, w2161, w2155) -> (w2148:bool)
        n943 = case shown="假" "穿管结果强制" {
          tunnel: w2148 -> [w2196 _]
          tunnel: [w2197 w2201] -> w2152
          tunnel: w2151 -> [w2199 w2206]
          tunnel: w2150 -> [w2192 w2203]
          tunnel: w2149 -> [w2190 w2202]
          frame False {
            w2189 = FALSE ("启用延时")
            n944 = Not(x=w2196) -> (.not. x?=w2195:bool)
            n945 = call "DB5000.X写.vi"("引用"=w2192, "启用延时"=w2189, "semaphore"=w2190, "地址名称"="穿管检测pass-写" ("组合框"), "value"=w2196, "error in (no error)"=w2199) -> ("引用输出"=w2191:refnum<k24>, "error out"=w2198:errorcluster)  [unwired: 8 in]
            n946 = call "DB5000.X写.vi"("引用"=w2191, "启用延时"=w2189, "semaphore"=w2190, "地址名称"="穿管检测fail-写" ("组合框"), "value"=w2195, "error in (no error)"=w2198) -> ("error out"=w2197:errorcluster)  [unwired: 8 in, 1 out]
          }
          frame True {
            n947 = call "DB5000.X写.vi"("引用"=w2203, "启用延时"=FALSE, "semaphore"=w2202, "地址名称"="穿管检测pass-写" ("组合框"), "value"=TRUE, "error in (no error)"=w2206) -> ("error out"=w2201:errorcluster)  [unwired: 8 in, 1 out]
          }
        }
        n948 = call "KB-EMG Input.vi"("Other Message"="检测CCD1,2穿管启动信号" ("t"), "EMG Iput"="EMG", "Emg"=FALSE) -> ("String OutPut"=w2177:string)  [unwired: 8 in]
        n949 = call "AMX-SaveImage.vi"("基路径"=w2166, "CCD Name"="CCD2", "布尔"=TRUE, "结果"=w2148, "Image in"=w2165, "类型"="CCD2" ("CCD Name")) -> ()  [unwired: 9 in, 1 out]
        n950 = call "Enqueue Element Array.vi"("priority"=w2186, "device error in"=w2152, "queue index"=6, "error in"=w2170, "master data"=w2177, "queue in"=w2183) -> ("error out"=w2188:errorcluster)  [unwired: 4 in, 1 out]
        n951 = call "AMX-SaveImage.vi"("基路径"=w2166, "CCD Name"="CCD1", "布尔"=FALSE, "Image in"=w2175, "error in (no error)"=w2151, "类型"="CCD1" ("CCD Name")) -> ()  [unwired: 9 in, 1 out]
      }
      frame "数据获取" {
        (unwired) "型号由 MES提供"
        w2242 = u16 0 items=["HPRI"=1, "LPRI"=0] ("priority")
        n952 = control-ref of="设备状态"() -> (w2235:refnum<vi>)
        n953 = call "设备状态循环显示.vi"("cmd:"=w2241, "Str引用句柄"=w2235, "新信息输入"=w2234) -> ()  [unwired: 9 in]
        n954 = Concatenate Strings("穿管检测" ("TestMessage"), ":" ("字符串"), "OK" ("字符串")) -> (w2210:string)
        n955 = call "SQL写入 - 穿管检测.vi"("ADODB._Connection In"=w2214, "TestMessage"=w2210, "error in (no error)"=w2215) -> ("error out"=w2209:errorcluster)  [unwired: 11 in, 1 out]
        n956 = disable-structure shown="禁用" {
          frame Disabled {
            n957 = local read "夹爪压力保存路径"() -> (w2246:path)
            n958 = local read "夹爪压力值"() -> (w2245:dbl[])
            n959 = call "压力数据保存判定 - 夹爪.vi"("路径"=w2246, "布尔"=TRUE, "添加的数组"=w2245) -> ()  [unwired: 9 in]
          }
          frame Enabled {
          }
        }
        n960 = local read "盘管压力值 2"() -> (w2225:dbl[])
        n961 = local read "路径"() -> (w2226:path)
        n962 = call "转换至动态数据2"("Array"=w2225) -> ("Dynamic Data Type"=w2231:dynamicdata)  [unwired: 3 in]
        n963 = call "转换至动态数据"("Array"="数组") -> ("Dynamic Data Type"=w2230:dynamicdata)  [unwired: 3 in]
        n964 = call "创建XY图"("error in (no error)"=w2209, "Y Input"=w2231, "X Input"=w2230) -> ("error out"=w2208:errorcluster, "XY Graph"=→"XY Graph":cluster{"X":dbl[], "Y":dbl[]}[])  [unwired: 7 in]
        n965 = call "压力数据保存判定.vi"("路径"=w2226, "error in (no error)"=w2208, "布尔"=TRUE, "添加的数组"=w2225) -> ("error out"=w2207:errorcluster)  [unwired: 7 in]
        n966 = call "DB5000.X写.vi"("引用"=w2222, "semaphore"=w2219, "地址名称"="电脑1穿管检测触发-读" ("组合框"), "value"=FALSE, "error in (no error)"=w2207) -> ("引用输出"=w2218:refnum<k24>, "error out"=w2217:errorcluster)  [unwired: 9 in]
        n967 = call "KB-EMG Input.vi"("Other Message"="数据传送" ("t"), "EMG Iput"="EMG", "Emg"=FALSE) -> ("String OutPut"=w2233:string)  [unwired: 8 in]
        n968 = call "DB5000.X写.vi"("引用"=w2218, "semaphore"=w2219, "地址名称"="电脑1压力获取触发-读" ("组合框"), "value"=FALSE, "error in (no error)"=w2217) -> ("error out"=w2216:errorcluster)  [unwired: 9 in, 1 out]
        n969 = call "Enqueue Element Array.vi"("priority"=w2242, "device error in"=w2216, "queue index"=6, "error in"=w2215, "master data"=w2233, "queue in"=w2239) -> ("error out"=w2244:errorcluster)  [unwired: 4 in, 1 out]
      }
      frame "数据传送" {
        w2252 = dbl[] [0.0, 0.0, 0.0, 0.0, 0.0, 0.0, 0.0, 0.0, 0.0, 0.0, 0.0, 0.0, 0.0, 0.0, 0.0, 0.0, 0.0, 0.0, 0.0] ("盘管压力值")
        w2264 = u16 0 items=["HPRI"=1, "LPRI"=0] ("priority")
        n970 = control-ref of="设备状态"() -> (w2257:refnum<vi>)
        n971 = call "设备状态循环显示.vi"("cmd:"=w2263, "Str引用句柄"=w2257, "新信息输入"=w2256) -> ()  [unwired: 9 in]
        n972 = local read "数字 3"() -> (w2248:dbl)
        n973 = disable-structure shown="禁用" {
          disable-tunnel: w2248 -> [w2272 _]
          disable-tunnel: "C0C01B2473002" ("扫码枪字符识别") -> [w2270 _]
          disable-tunnel: _ -> [w2268 _]
          disable-tunnel: [w2267 _] -> w2250
          frame Disabled {
            n974 = call "mess压力数据上传.vi"("夹持力"=0.0, "压力"=w2272, "barcode"=w2270, "wkc_no"="SB-QN-304", "error in (no error)"=w2268) -> ("数据上传OK/NG"=w2267:bool)  [unwired: 8 in, 2 out]
          }
          frame Enabled {
          }
        }
        "数据上传OK/NG" <- w2250
        n975 = local write "数据上传OK/NG"(FALSE ("数据上传OK/NG")) -> ()
        n976 = local write "盘管压力值 2"(w2252) -> ()
        n977 = local write "夹爪压力值"(w2252) -> ()
        n978 = call "KB-EMG Input.vi"("Other Message"="自动开始" ("t"), "EMG Iput"="EMG", "Emg"=FALSE) -> ("String OutPut"=w2255:string)  [unwired: 8 in]
        n979 = call "Enqueue Element Array.vi"("priority"=w2264, "queue index"=6, "error in"=w2254, "master data"=w2255, "queue in"=w2261) -> ("error out"=w2266:errorcluster)  [unwired: 5 in, 1 out]
      }
      frame "<-----自动加工结束--------手动部分------->" {
        w2279 = u16 0 items=["HPRI"=1, "LPRI"=0] ("priority")
        # "//读取配置文件"
        n980 = local read "设备状态"() -> (w2278:string)
        n981 = Concatenate Strings(w2278, "....." ("字符串"), "\r\n", w2274) -> (w2275:string)
        n982 = local write "设备状态"(w2275) -> ()
        n983 = call "Enqueue Element Array.vi"("priority"=w2279, "queue index"=6, "error in"=w2281, "master data"="" ("Element 1"), "queue in"=w2285) -> ("error out"=w2284:errorcluster)  [unwired: 5 in, 1 out]
      }
      frame "Machine Paramter Save Buttom" {
        w2289 = u16 0 items=["HPRI"=1, "LPRI"=0] ("priority")
        n984 = One Button Dialog(message="确认保存" ("消息")) -> (true=w2287:bool)  [unwired: 1 in]
        n985 = case shown="真" w2287 {
          frame False {
          }
          frame True {
            n986 = global read "Global System.vi" "ref path"() -> (w2298:path)
            n987 = Build Path(base path=w2298, name or relative path="PLC Connect Signal.txt" ("名称或相对路径")) -> (appended path=w2296:path)
            n988 = call-poly <vilib>:"Write Delimited Spreadsheet.vi"("file path (dialog if empty)"=w2296) -> ()  [unwired: 13 in, 2 out]
          }
        }
        n989 = call "Enqueue Element Array.vi"("priority"=w2289, "queue index"=6, "error in"=w2291, "master data"="" ("Element 1"), "queue in"=w2294) -> ("error out"=w2293:errorcluster)  [unwired: 5 in, 1 out]
      }
      frame "Other Param Save Buttom" {
        w2303 = u16 0 items=["HPRI"=1, "LPRI"=0] ("priority")
        n990 = control-ref of="设备状态"() -> (w2299:refnum<vi>)
        n991 = call "设备状态循环显示.vi"("cmd:"=w2300, "Str引用句柄"=w2299, "新信息输入"=w2302) -> ()  [unwired: 9 in]
        n992 = call "Enqueue Element Array.vi"("priority"=w2303, "queue index"=6, "error in"=w2305, "master data"="" ("Element 1"), "queue in"=w2308) -> ("error out"=w2307:errorcluster)  [unwired: 5 in, 1 out]
      }
      frame "Reset Static" {
        w2311 = "0" ("TotalNumber")
        w2319 = u16 0 items=["HPRI"=1, "LPRI"=0] ("priority")
        n993 = control-ref of="设备状态"() -> (w2310:refnum<vi>)
        n994 = call "设备状态循环显示.vi"("Str引用句柄"=w2310, "新信息输入"=w2318) -> ()  [unwired: 10 in]
        n995 = Bundle By Name(cluster=w2314, "TotalNumber"=w2311, "PassNumber"=w2311, "FailNumber"=w2311) -> (w2313:T21)
        n996 = Initialize Array("0", 3 ("维数大小")) -> (w2312:string[])
        n997 = call "3D-ResetTotalNumber.vi"("Inputs_BaseParam"=w2312, "名称或相对路径"="UserDefine.ini") -> ()  [unwired: 10 in]
        n998 = call "Enqueue Element Array.vi"("priority"=w2319, "queue index"=6, "error in"=w2321, "master data"="" ("Element 1"), "queue in"=w2324) -> ("error out"=w2323:errorcluster)  [unwired: 5 in, 1 out]
      }
      frame "启动9点校正功能" {
        w2329 = u16 0 items=["HPRI"=1, "LPRI"=0] ("priority")
        n999 = control-ref of="设备状态"() -> (w2327:refnum<vi>)
        n1000 = call "设备状态循环显示.vi"("Str引用句柄"=w2327, "新信息输入"=w2328) -> ()  [unwired: 10 in]
        n1001 = call "Enqueue Element Array.vi"("priority"=w2329, "queue index"=6, "error in"=w2331, "master data"="" ("Element 1"), "queue in"=w2334) -> ("error out"=w2333:errorcluster)  [unwired: 5 in, 1 out]
      }
      frame "Clear" {
        w2340 = u16 0 items=["HPRI"=1, "LPRI"=0] ("priority")
        n1002 = control-ref of="设备状态"() -> (w2337:refnum<vi>)
        n1003 = call "设备状态循环显示.vi"("cmd:"=w2338, "Str引用句柄"=w2337, "新信息输入"=w2339) -> ()  [unwired: 9 in]
        n1004 = call "Enqueue Element Array.vi"("priority"=w2340, "queue index"=6, "error in"=w2342, "master data"="" ("Element 1"), "queue in"=w2345) -> ("error out"=w2344:errorcluster)  [unwired: 5 in, 1 out]
      }
      frame "Vision Paramter Save" {
        w2350 = u16 0 items=["HPRI"=1, "LPRI"=0] ("priority")
        n1005 = control-ref of="设备状态"() -> (w2347:refnum<vi>)
        n1006 = call "设备状态循环显示.vi"("cmd:"=w2348, "Str引用句柄"=w2347, "新信息输入"=w2349) -> ()  [unwired: 9 in]
        n1007 = call "Enqueue Element Array.vi"("priority"=w2350, "queue index"=6, "error in"=w2352, "master data"="" ("Element 1"), "queue in"=w2356) -> ("error out"=w2355:errorcluster)  [unwired: 5 in, 1 out]
      }
      frame "*Emergency alarm" {
        w2364 = u16 1 items=["HPRI"=1, "LPRI"=0] ("priority")
        w2365 = u16 0 items=["HPRI"=1, "LPRI"=0] ("priority")
        n1008 = call "Enqueue Element Array.vi"("priority"=w2364, "queue index"=0, "error in"=w2358, "master data"="" ("Element 1"), "queue in"=w2361) -> ("error out"=w2359:errorcluster, "queue out"=w2360:T25)  [unwired: 5 in]
        n1009 = call "Enqueue Element Array.vi"("priority"=w2365, "queue index"=6, "error in"=w2359, "master data"="" ("Element 1"), "queue in"=w2360) -> ("error out"=w2369:errorcluster)  [unwired: 5 in, 1 out]
      }
    }
    n1010 = Wait (ms)(milliseconds to wait=w1872) -> ()  [unwired: 1 out]
  }
  n1011 = while "While循环" {
    shift-right: [w2388] -> w27
    shift-left: w2 -> [w2384]
    shift-right: [w2385] -> _
    shift-left: w14 -> [w2386]
    tunnel: w15 -> [w2380]
    tunnel: w17 -> [w2374]
    tunnel: w8 -> [w2372]
    tunnel: w7 -> [w2373]
    tunnel: w1 -> [w2371]
    stop <- w2379 stop-if-true
    # "True,10458935,C.0C.01B,Firebird2药物支架系统（无标签）G2513,G2513,5"
    # "主线程-字符检测"
    n1012 = call "Dequeue Element Array.vi"("queue in"=w2380, "queue index"=3, "error in"=w2384) -> ("queue out"=w2383:T25, "master data"=w2382:string, "secondary data"=w2381:string[], "error out"=w2379:errorcluster)  [unwired: 2 in, 1 out]
    n1013 = case shown="\"CCD6图像处理模块\"" w2382 {
      selector: w2382 -> [w2390 _ w2409 w2427 w2445 w2467 w2480 w2494 _ _ _ w2559 w2581 w2611 w2624 w2641 w2697 w2736 w2773 w2817 w2842 _ w2870 w2880 w2890 _]
      tunnel: w2383 -> [_ _ w2421 w2437 w2455 w2477 w2491 w2505 w2526 w2536 w2549 w2569 w2590 w2620 w2630 w2646 w2702 w2741 w2778 w2822 w2853 w2862 w2876 w2886 w2897 w2903]
      tunnel: w2379 -> [w2392 w2398 w2410 w2425 w2444 w2465 w2481 w2495 w2518 w2532 w2545 w2560 w2574 w2606 w2623 w2639 w2685 w2733 w2770 w2810 w2849 w2859 w2873 w2883 w2893 w2900]
      tunnel: [w2392 w2398 w2420 w2436 w2454 w2476 w2490 w2504 w2525 w2535 w2548 w2568 w2589 w2619 w2635 w2651 w2707 w2746 w2783 w2827 w2852 w2861 w2875 w2885 w2896 w2911] -> w2388
      tunnel: [50 50 10 10 10 10 10 10 w2521 50 20 10 10 10 w2631 w2647 w2703 w2742 w2779 w2823 w2841 50 50 50 50 50] -> w2387
      tunnel: w2386 -> [w2393 w2399 w2404 w2423 w2443 w2466 w2479 w2493 w2509 w2533 w2539 w2557 w2579 w2609 w2622 w2636 w2691 w2734 w2771 w2813 w2850 w2856 w2869 w2878 w2894 w2909]
      tunnel: [w2393 w2399 w2403 w2423 w2443 w2466 w2479 w2493 w2509 w2533 w2539 w2557 w2579 w2609 w2622 w2636 w2691 w2734 w2771 w2813 w2850 w2856 w2869 w2878 w2894 w2909] -> w2385
      tunnel: w2381 -> [_ _ _ _ _ _ _ _ _ _ _ _ _ _ _ _ _ _ _ _ _ _ _ _ _ _]
      tunnel: "字符检测 : " -> [w2389 _ w2411 w2429 w2447 w2473 w2487 w2501 w2515 _ _ w2562 w2583 w2613 w2632 w2648 w2704 w2743 w2780 w2824 _ _ w2868 _ _ _]
      tunnel: "T2 :" -> [_ _ _ _ _ _ _ _ _ _ _ _ _ _ _ _ _ _ _ _ _ _ _ _ w2889 _]
      tunnel: 5 -> [_ _ _ _ _ _ _ _ w2521 _ _ _ _ _ w2631 w2647 w2703 w2742 w2779 w2823 w2841 _ _ _ _ _]
      tunnel: w2374 -> [_ _ _ _ _ _ _ _ _ _ _ _ _ _ _ _ w2675 _ _ _ _ _ _ _ _ _]
      tunnel: w2373 -> [_ _ _ _ _ _ _ _ _ _ _ _ w2572 _ _ _ w2659 _ _ w2809 _ _ _ _ _ _]
      tunnel: w2372 -> [_ _ _ _ _ _ _ _ _ _ _ _ w2571 _ _ _ w2671 _ _ w2808 _ _ _ _ _ _]
      tunnel: w2371 -> [_ _ _ _ _ _ _ _ _ _ _ _ _ _ _ _ w2666 _ _ _ _ _ _ _ _ _]
      frame "No event", Default {
        # "Don't place any functions"
        n1014 = disable-structure shown="禁用" {
          disable-tunnel: w2390 -> [w2395 _]
          disable-tunnel: w2389 -> [w2394 _]
          frame Disabled {
            n1015 = control-ref of="设备状态"() -> (w2396:refnum<vi>)
            n1016 = call "循环时状态显示.vi"("Str引用句柄"=w2396, "cmd:"=w2394, "新信息输入"=w2395) -> ()  [unwired: 9 in]
          }
          frame Enabled {
          }
        }
      }
      frame "EMG" {
        # "Don't place any functions"
      }
      frame "Loading Variable" {
        w2418 = u16 0 items=["HPRI"=1, "LPRI"=0] ("priority")
        # "potteryTemplete"
        n1017 = control-ref of="设备状态"() -> (w2414:refnum<vi>)
        n1018 = call "设备状态循环显示.vi"("cmd:"=w2411, "Str引用句柄"=w2414, "新信息输入"=w2409) -> ()  [unwired: 9 in]
        n1019 = call "Read Config InI.vi"("名称或相对路径"="UserDefine.ini") -> ("ParamSet"=w2417:string[])  [unwired: 14 in, 4 out]
        n1020 = global read "Global System.vi" "ref path"() -> (w2408:path)
        n1021 = Index Array(array=w2417, index #1=0 ("索引")) -> (element #1=w2401:string)  [unwired: 1 in, 1 out]
        n1022 = Build Path(base path=w2408, name or relative path="Template Program" ("名称或相对路径")) -> (appended path=w2406:path)
        n1023 = Build Path(base path=w2406, name or relative path=w2401) -> (appended path=→"CCD6":path)
        n1024 = global read "Global System.vi" "Paus"() -> (w2412:bool)
        n1025 = call "KB-EMG Input.vi"("Other Message"="Loading Variable Config" ("Element 1"), "EMG Iput"="EMG", "Emg"=w2412) -> ("String OutPut"=w2400:string)  [unwired: 8 in]
        n1026 = Bundle By Name(cluster=w2404, "2 Pause Message"=w2400, "LoadProgram"=w2401) -> (w2403:T21)
        n1027 = call "Enqueue Element Array.vi"("priority"=w2418, "queue index"=3, "error in"=w2410, "master data"=w2400, "queue in"=w2421) -> ("error out"=w2420:errorcluster)  [unwired: 5 in, 1 out]
      }
      frame "Loading Variable Config" {
        w2434 = u16 0 items=["HPRI"=1, "LPRI"=0] ("priority")
        n1028 = control-ref of="设备状态"() -> (w2433:refnum<vi>)
        n1029 = call "设备状态循环显示.vi"("cmd:"=w2429, "Str引用句柄"=w2433, "新信息输入"=w2427) -> ()  [unwired: 9 in]
        n1030 = Unbundle By Name(w2423) -> ("LoadProgram"=w2426:string)
        n1031 = call "读取产品参数信息-CCD6.vi"("错误输入（无错误）"=w2425, "LoadProductName"=w2426) -> ("错误输出"=w2424:errorcluster)  [unwired: 9 in]
        n1032 = global read "Global System.vi" "Paus"() -> (w2431:bool)
        n1033 = call "KB-EMG Input.vi"("Other Message"="Initial CCD" ("Element 1"), "EMG Iput"="EMG", "Emg"=w2431) -> ("String OutPut"=w2428:string)  [unwired: 8 in]
        n1034 = call "Enqueue Element Array.vi"("priority"=w2434, "device error in"=w2424, "queue index"=3, "error in"=w2425, "master data"=w2428, "queue in"=w2437) -> ("error out"=w2436:errorcluster)  [unwired: 4 in, 1 out]
      }
      frame "Initial CCD" {
        w2452 = u16 0 items=["HPRI"=1, "LPRI"=0] ("priority")
        n1035 = control-ref of="设备状态"() -> (w2451:refnum<vi>)
        n1036 = call "设备状态循环显示.vi"("cmd:"=w2447, "Str引用句柄"=w2451, "新信息输入"=w2445) -> ()  [unwired: 9 in]
        n1037 = call "CR-Initial CameraCCD6.vi"("error in (no error)"=w2444) -> ("error out"=w2440:errorcluster, "Session Out"=w2442:T28)  [unwired: 9 in]
        n1038 = disable-structure shown="启用" {
          disable-tunnel: w2442 -> [w2461 w2464]
          disable-tunnel: [w2460 w2464] -> w2441
          disable-tunnel: w2440 -> [w2459 w2463]
          disable-tunnel: [w2458 w2463] -> w2439
          frame Enabled {
            n1039 = property class="IMAQdx"(reference=w2461, error in=w2459, "ActiveAttribute"="ExposureTimeAbs", "ValueI64"=i64 654) -> (reference out=w2460:T28, error out=w2458:errorcluster)
          }
          frame Disabled {
          }
        }
        n1040 = global read "Global System.vi" "Paus"() -> (w2449:bool)
        n1041 = global write "Global System.vi" "Session Out CCD0"(w2441) -> ()
        n1042 = call "KB-EMG Input.vi"("Other Message"="Open Telnet" ("Element 1"), "EMG Iput"="EMG", "Emg"=w2449) -> ("String OutPut"=w2446:string)  [unwired: 8 in]
        n1043 = call "Enqueue Element Array.vi"("priority"=w2452, "device error in"=w2439, "queue index"=3, "error in"=w2444, "master data"=w2446, "queue in"=w2455) -> ("error out"=w2454:errorcluster)  [unwired: 4 in, 1 out]
      }
      frame "Open Telnet" {
        w2474 = u16 0 items=["HPRI"=1, "LPRI"=0] ("priority")
        n1044 = control-ref of="设备状态"() -> (w2472:refnum<vi>)
        n1045 = call "设备状态循环显示.vi"("cmd:"=w2473, "Str引用句柄"=w2472, "新信息输入"=w2467) -> ()  [unwired: 9 in]
        n1046 = global read "Global System.vi" "Paus"() -> (w2470:bool)
        n1047 = call "KB-EMG Input.vi"("Other Message"="Open VISA" ("master data"), "EMG Iput"="EMG", "Emg"=w2470) -> ("String OutPut"=w2468:string)  [unwired: 8 in]
        n1048 = call "Enqueue Element Array.vi"("priority"=w2474, "queue index"=3, "error in"=w2465, "master data"=w2468, "queue in"=w2477) -> ("error out"=w2476:errorcluster)  [unwired: 5 in, 1 out]
      }
      frame "Open VISA" {
        w2488 = u16 0 items=["HPRI"=1, "LPRI"=0] ("priority")
        n1049 = control-ref of="设备状态"() -> (w2486:refnum<vi>)
        n1050 = call "设备状态循环显示.vi"("cmd:"=w2487, "Str引用句柄"=w2486, "新信息输入"=w2480) -> ()  [unwired: 9 in]
        n1051 = global read "Global System.vi" "Paus"() -> (w2484:bool)
        n1052 = call "KB-EMG Input.vi"("Other Message"="Create File" ("master data"), "EMG Iput"="EMG", "Emg"=w2484) -> ("String OutPut"=w2482:string)  [unwired: 8 in]
        n1053 = call "Enqueue Element Array.vi"("priority"=w2488, "queue index"=3, "error in"=w2481, "master data"=w2482, "queue in"=w2491) -> ("error out"=w2490:errorcluster)  [unwired: 5 in, 1 out]
      }
      frame "Create File" {
        w2502 = u16 0 items=["HPRI"=1, "LPRI"=0] ("priority")
        n1054 = control-ref of="设备状态"() -> (w2500:refnum<vi>)
        n1055 = call "设备状态循环显示.vi"("cmd:"=w2501, "Str引用句柄"=w2500, "新信息输入"=w2494) -> ()  [unwired: 9 in]
        n1056 = global read "Global System.vi" "Paus"() -> (w2498:bool)
        n1057 = call "KB-EMG Input.vi"("Other Message"="Initial-Clear Variable" ("master data"), "EMG Iput"="EMG", "Emg"=w2498) -> ("String OutPut"=w2496:string)  [unwired: 8 in]
        n1058 = call "Enqueue Element Array.vi"("priority"=w2502, "queue index"=3, "error in"=w2495, "master data"=w2496, "queue in"=w2505) -> ("error out"=w2504:errorcluster)  [unwired: 5 in, 1 out]
      }
      frame "Initial-Clear Variable" {
        w2523 = u16 0 items=["HPRI"=1, "LPRI"=0] ("priority")
        n1059 = control-ref of="设备状态"() -> (w2517:refnum<vi>)
        n1060 = call "设备状态循环显示.vi"("cmd:"=w2515, "Str引用句柄"=w2517, "新信息输入"="Initial Finish " ("字符串")) -> ()  [unwired: 9 in]
        n1061 = Current VI's Menubar() -> (w2520:refnum<k9>)
        n1062 = for {
          tunnel: w2520 -> [w2529]
          tunnel: string[] ["登陆"] -> [w2527] mode=indexing
          n1063 = Set Menu Item Info(7:w2527, 9:TRUE ("已启用"), 10:w2527, 11:w2529) -> ()  [unwired: 3 in, 2 out]
        }
        n1064 = global read "Global System.vi" "Paus"() -> (w2513:bool)
        n1065 = call "KB-EMG Input.vi"("Other Message"="" ("Element 1"), "EMG Iput"="EMG", "Emg"=w2513) -> ("String OutPut"=w2511:string)  [unwired: 8 in]
        n1066 = local write "字符检测初始化状态"(TRUE ("字符检测初始化状态")) -> ()
        n1067 = local write "字符检测触发"(FALSE ("字符检测触发")) -> ()
        n1068 = global write "Global System.vi" "G_Status 2"(TRUE ("G_Status 1")) -> ()
        n1069 = property on="User Login" class="Bool (严格)"("DisabledEnum"=T22."Enabled" ("禁用")) -> ()  [unwired: 2 in, 2 out]
        n1070 = call "Enqueue Element Array.vi"("priority"=w2523, "queue index"=3, "error in"=w2518, "master data"=w2511, "queue in"=w2526) -> ("error out"=w2525:errorcluster)  [unwired: 5 in, 1 out]
      }
      frame "<----自动加工------------->" {
        w2530 = u16 0 items=["HPRI"=1, "LPRI"=0] ("priority")
        # "//读取配置文件"
        n1071 = call "Enqueue Element Array.vi"("priority"=w2530, "queue index"=3, "error in"=w2532, "master data"="" ("Element 1"), "queue in"=w2536) -> ("error out"=w2535:errorcluster)  [unwired: 5 in, 1 out]
      }
      frame "自动开始" {
        w2546 = u16 0 items=["HPRI"=1, "LPRI"=0] ("priority")
        n1072 = global write "Global System.vi" "G_Status 2"(TRUE ("G_Status 1")) -> ()
        n1073 = global read "Global System.vi" "Paus"() -> (w2542:bool)
        n1074 = call "KB-EMG Input.vi"("Other Message"="Load Var1", "EMG Iput"="EMG", "Emg"=w2542) -> ("String OutPut"=w2541:string)  [unwired: 8 in]
        n1075 = call "Enqueue Element Array.vi"("priority"=w2546, "queue index"=3, "error in"=w2545, "master data"=w2541, "queue in"=w2549) -> ("error out"=w2548:errorcluster)  [unwired: 5 in, 1 out]
      }
      frame "检测CCD6启动信号" {
        w2566 = u16 0 items=["HPRI"=1, "LPRI"=0] ("priority")
        # "正面垫片PLC启动信号"
        n1076 = control-ref of="设备状态"() -> (w2563:refnum<vi>)
        n1077 = call "循环时状态显示 - 3.vi"("Str引用句柄"=w2563, "cmd:"=w2562, "新信息输入"=w2559) -> ()  [unwired: 9 in]
        n1078 = local read "DB5000.X"() -> (w2551:T4)
        n1079 = Unbundle By Name(w2551) -> ("电脑1CCD读取\n字符触发-读"=w2550:bool)
        n1080 = Or(x="字符检测触发", y=w2550) -> (x .or. y?=w2553:bool)
        n1081 = Select(t="字符启动信号处理" ("EMG Iput"), s=w2553, f="检测CCD6启动信号" ("EMG Iput")) -> (s? t:f=w2555:string)
        n1082 = case shown="真" w2553 {
          frame False {
          }
          frame True {
            n1083 = global write "Global System.vi" "G_Status 2"(TRUE ("G_Status 1")) -> ()
          }
        }
        n1084 = call "KB-EMG Input.vi"("Other Message"=w2555, "EMG Iput"="EMG", "Emg"=FALSE) -> ("String OutPut"=w2564:string)  [unwired: 8 in]
        n1085 = call "Enqueue Element Array.vi"("priority"=w2566, "queue index"=3, "error in"=w2560, "master data"=w2564, "queue in"=w2569) -> ("error out"=w2568:errorcluster)  [unwired: 5 in, 1 out]
      }
      frame "字符启动信号处理" {
        w2587 = u16 0 items=["HPRI"=1, "LPRI"=0] ("priority")
        n1086 = control-ref of="设备状态"() -> (w2584:refnum<vi>)
        n1087 = call "循环时状态显示 - 3.vi"("Str引用句柄"=w2584, "cmd:"=w2583, "新信息输入"=w2581) -> ()  [unwired: 9 in]
        n1088 = disable-structure shown="启用" {
          disable-tunnel: w2574 -> [w2596 w2597]
          disable-tunnel: [w2595 w2597] -> w2573
          disable-tunnel: w2572 -> [w2592 _]
          disable-tunnel: w2571 -> [w2591 _]
          frame Disabled {
            n1089 = call "DB5000.X写.vi"("引用"=w2591, "semaphore"=w2592, "地址名称"="电脑1CCD读取字符触发-读" ("组合框"), "value"=FALSE, "error in (no error)"=w2596) -> ("error out"=w2595:errorcluster)  [unwired: 9 in, 1 out]
          }
          frame Enabled {
          }
        }
        n1090 = Select(t="Load Var1" ("EMG Iput"), s=FALSE, f="获取图像") -> (s? t:f=w2576:string)
        n1091 = call "KB-EMG Input.vi"("Other Message"=w2576, "EMG Iput"="EMG", "Emg"=FALSE) -> ("String OutPut"=w2585:string)  [unwired: 8 in]
        n1092 = call "Enqueue Element Array.vi"("priority"=w2587, "queue index"=3, "error in"=w2573, "master data"=w2585, "queue in"=w2590) -> ("error out"=w2589:errorcluster)  [unwired: 5 in, 1 out]
      }
      frame "获取图像" {
        w2617 = u16 0 items=["HPRI"=1, "LPRI"=0] ("priority")
        n1093 = control-ref of="设备状态"() -> (w2614:refnum<vi>)
        n1094 = call "循环时状态显示 - 3.vi"("Str引用句柄"=w2614, "cmd:"=w2613, "新信息输入"=w2611) -> ()  [unwired: 9 in]
        n1095 = global read "Global System.vi" "字符检测基础参数"() -> (w2605:T30)
        n1096 = global read "Global System.vi" "Session Out CCD0"() -> (w2604:T28)
        n1097 = call "A 侧面 处理函数CCD6.vi"("Session Out CCD1"=w2604, "error in (no error)"=w2606, "Image Name"="T6", "CR-字符检测基础参数"=w2605) -> ("error out"=w2600:errorcluster, "Session Out"=w2607:T28, "Image out"=w2603:T1)  [unwired: 4 in, 1 out]
        n1098 = global write "Global System.vi" "Session Out CCD0"(w2607) -> ()
        n1099 = call "字符图片截取.vi"("Image"=w2603) -> ("Image 3"=→"字符检测相机6":T1)  [unwired: 8 in, 2 out]
        n1100 = call "ClearErr.vi"("error in (no error)"=w2600, "运行位置"="字符检测获取图像") -> ("error out"=w2599:errorcluster)  [unwired: 9 in]
        n1101 = call "KB-EMG Input.vi"("Other Message"="CCD6图像处理模块", "EMG Iput"="EMG", "Emg"=FALSE) -> ("String OutPut"=w2615:string)  [unwired: 8 in]
        n1102 = call "Enqueue Element Array.vi"("priority"=w2617, "device error in"=w2599, "queue index"=3, "error in"=w2606, "master data"=w2615, "queue in"=w2620) -> ("error out"=w2619:errorcluster)  [unwired: 4 in, 1 out]
      }
      frame "Load Var1" {
        w2633 = u16 0 items=["HPRI"=1, "LPRI"=0] ("priority")
        n1103 = control-ref of="设备状态"() -> (w2626:refnum<vi>)
        n1104 = Tick Count (ms)() -> (millisecond timer value=→"Start Time 3":u32)
        n1105 = call "设备状态循环显示.vi"("cmd:"=w2632, "Str引用句柄"=w2626, "新信息输入"=w2624) -> ()  [unwired: 9 in]
        n1106 = call "KB-EMG Input.vi"("Other Message"="Load Var2" ("t"), "EMG Iput"="EMG", "Emg"=FALSE) -> ("String OutPut"=w2625:string)  [unwired: 8 in]
        n1107 = call "Enqueue Element Array.vi"("priority"=w2633, "queue index"=3, "error in"=w2623, "master data"=w2625, "queue in"=w2630) -> ("error out"=w2635:errorcluster)  [unwired: 5 in, 1 out]
      }
      frame "Load Var2" {
        w2649 = u16 0 items=["HPRI"=1, "LPRI"=0] ("priority")
        n1108 = control-ref of="设备状态"() -> (w2642:refnum<vi>)
        n1109 = call "设备状态循环显示.vi"("cmd:"=w2648, "Str引用句柄"=w2642, "新信息输入"=w2641) -> ()  [unwired: 9 in]
        n1110 = Unbundle By Name(w2636) -> ("LoadProgram"=w2637:string)
        n1111 = call "读取产品参数信息-CCD6.vi"("错误输入（无错误）"=w2639, "LoadProductName"=w2637) -> ("错误输出"=w2638:errorcluster)  [unwired: 9 in]
        n1112 = call "KB-EMG Input.vi"("Other Message"="检测CCD6启动信号" ("t"), "EMG Iput"="EMG", "Emg"=FALSE) -> ("String OutPut"=w2640:string)  [unwired: 8 in]
        n1113 = call "Enqueue Element Array.vi"("priority"=w2649, "device error in"=w2638, "queue index"=3, "error in"=w2639, "master data"=w2640, "queue in"=w2646) -> ("error out"=w2651:errorcluster)  [unwired: 4 in, 1 out]
      }
      frame "CCD6图像处理模块" {
        (unwired) "C0C06C0304028" ("扫码枪字符识别")
        w2705 = u16 0 items=["HPRI"=1, "LPRI"=0] ("priority")
        n1114 = control-ref of="设备状态"() -> (w2698:refnum<vi>)
        n1115 = global read "Global System.vi" "CR- 字符检测参数 2"() -> (w2688:T32)
        n1116 = local read "字符检测相机6"() -> (w2693:T1)
        n1117 = global read "Global System.vi" "CR-CCD1字符定位参数"() -> (w2687:T35)
        n1118 = call "设备状态循环显示.vi"("cmd:"=w2704, "Str引用句柄"=w2698, "新信息输入"=w2697) -> ()  [unwired: 9 in]
        n1119 = call "DB5000.X写.vi"("引用"=w2671, "semaphore"=w2659, "地址名称"="电脑1CCD读取字符触发-读" ("组合框"), "value"=FALSE, "error in (no error)"=w2675) -> ("引用输出"=w2677:refnum<k24>, "error out"=w2676:errorcluster)  [unwired: 9 in]
        n1120 = call "CR-字符检测处理函数as.vi"("Image in"=w2693, "字符识别参数"=w2688, "error in (no error)"=w2685, "CCD1字符定位参数"=w2687) -> ("模板匹配OK/NG"=→"模板匹配OK/NG":bool, "Image out"=w2690:T1, "Data"=w2652:string, "字符方向判定结果"=w2674:bool, "结果"=w2655:bool, "error out"=w2670:errorcluster)  [unwired: 10 in]
        "相机字符识别" <- w2652
        "字符方向判定结果" <- w2674
        n1121 = call "DB5000.X写.vi"("引用"=w2677, "semaphore"=w2659, "地址名称"="字符1检测pass-写" ("组合框"), "value"=w2655, "error in (no error)"=w2676) -> ("引用输出"=w2681:refnum<k24>, "error out"=w2684:errorcluster)  [unwired: 9 in]
        n1122 = local write "字符检测相机6"(w2690) -> ()
        n1123 = Not(x=w2655) -> (.not. x?=w2658:bool)
        n1124 = call "DB5000.X写.vi"("引用"=w2681, "semaphore"=w2659, "地址名称"="字符1检测fail-写" ("组合框"), "value"=w2658, "error in (no error)"=w2684) -> ("引用输出"=w2661:refnum<k24>, "error out"=w2665:errorcluster)  [unwired: 9 in]
        n1125 = call "字符转换C代码.vi"("扫码枪字符识别"=w2652) -> ()  [unwired: 10 in, 1 out]
        n1126 = disable-structure shown="禁用" {
          disable-tunnel: [w2711 _] -> _
          disable-tunnel: [w2710 _] -> w2672
          disable-tunnel: [w2709 _] -> w2673
          disable-tunnel: w2652 -> [w2708 _]
          frame Disabled {
            # "mess"
            n1127 = call "标签打印.vi"("barcode"=w2708) -> ("error out"=w2711:errorcluster, "Print"=w2710:string)  [unwired: 9 in]
            n1128 = call "mess压力数据上传.vi"() -> ("ValidateBarcode"=w2709:string)  [unwired: 13 in, 2 out]
          }
          frame Enabled {
          }
        }
        n1129 = call "DB5000.X写.vi"("引用"=w2661, "semaphore"=w2659, "地址名称"="扫码枪pass-写" ("组合框"), "value"=w2655, "error in (no error)"=w2665) -> ("引用输出"=w2653:refnum<k24>, "error out"=w2654:errorcluster)  [unwired: 9 in]
        n1130 = call "DB5000.X写.vi"("引用"=w2653, "semaphore"=w2659, "地址名称"="扫码枪fail-写" ("组合框"), "value"=w2658, "error in (no error)"=w2654) -> ("引用输出"=w2660:refnum<k24>, "error out"=w2664:errorcluster)  [unwired: 9 in]
        n1131 = local read "压力表打印代码据库"() -> (w2667:string[][])
        n1132 = local read "压力表代码"() -> (w2657:string)
        n1133 = local read "压力表数据库"() -> (w2668:string[][])
        n1134 = local write "ValidateBarcode 2"(w2672) -> ()
        n1135 = local write "ValidateBarcode 3"(w2673) -> ()
        n1136 = call "mess返回值解析.vi"("ValidateBarcode"=w2672) -> ("元素"=w2656:string)  [unwired: 10 in]
        n1137 = disable-structure shown="启用" {
          disable-tunnel: w2660 -> [w2715 _]
          disable-tunnel: [w2714 w2716] -> w2680
          disable-tunnel: w2664 -> [w2713 w2716]
          disable-tunnel: w2674 -> [w2712 _]
          frame Disabled {
            n1138 = call "DB5000.X写.vi"("引用"=w2715, "value"=w2712, "error in (no error)"=w2713) -> ("error out"=w2714:errorcluster)  [unwired: 11 in, 1 out]
          }
          frame Enabled {
          }
        }
        n1139 = local write "元素"(w2656) -> ()
        n1140 = call "产品信息解析.vi"("引用"=w2671, "semaphore"=w2659, "压力打印代码据库"=w2668, "ADODB._Connection In"=w2666, "输入元素"=w2657, "压力表数据库 2"=w2667, "ValidateBarcode"=w2652, "error in (no error)"=w2670) -> ("error out"=w2669:errorcluster)  [unwired: 19 in]
        n1141 = call "KB-EMG Input.vi"("Other Message"="结果显示" ("t"), "EMG Iput"="EMG", "Emg"=FALSE) -> ("String OutPut"=w2696:string)  [unwired: 8 in]
        n1142 = call "AMX-SaveImage - 衬丝检测.vi"("基路径"=path "D:/Data/History Image", "CCD Name"="CCD7", "布尔"=TRUE, "结果"=w2674, "Image in"=w2690, "error in (no error)"=w2669) -> ("error out"=w2692:errorcluster)  [unwired: 9 in]
        n1143 = call "Enqueue Element Array.vi"("priority"=w2705, "device error in"=w2692, "queue index"=3, "error in"=w2680, "master data"=w2696, "queue in"=w2702) -> ("error out"=w2707:errorcluster)  [unwired: 4 in, 1 out]
      }
      frame "MESS" {
        w2744 = u16 0 items=["HPRI"=1, "LPRI"=0] ("priority")
        n1144 = control-ref of="设备状态"() -> (w2737:refnum<vi>)
        n1145 = Unbundle By Name(w2734) -> ()  [unwired: 1 out]
        n1146 = disable-structure shown="禁用" {
          disable-tunnel: w2743 -> [w2756 _]
          disable-tunnel: w2737 -> [w2755 _]
          disable-tunnel: w2736 -> [w2754 _]
          disable-tunnel: w2733 -> [w2751 w2760]
          disable-tunnel: [w2750 w2760] -> w2732
          disable-tunnel: [w2747 _] -> w2731
          frame Disabled {
            n1147 = call "设备状态循环显示.vi"("cmd:"=w2756, "Str引用句柄"=w2755, "新信息输入"=w2754) -> ()  [unwired: 9 in]
            n1148 = local read "字符比对"() -> (w2748:bool)
            n1149 = case shown="假" w2748 {
              tunnel: ["" ("相机字符识别") w2759] -> w2749
              frame False {
                n1150 = local write "相机字符识别"("字符匹配错误" ("相机字符识别")) -> ()
              }
              frame True {
                n1151 = local read "相机字符识别"() -> (w2759:string)
              }
            }
            n1152 = call "MESS测试.vi"("error in (no error)"=w2751, "barcode"=w2749, "accessKey"="a45b2d3334ffs_", "Url"="http://10.6.1.31:8080/MesInnerpackLineIO.asmx") -> ("error out"=w2750:errorcluster, "ValidateBarcode"=w2747:string)  [unwired: 6 in]
          }
          frame Enabled {
          }
        }
        "ValidateBarcode" <- w2731
        n1153 = local read "扫码枪字符识别"() -> (w2719:string)
        n1154 = local read "压力表代码"() -> (w2729:string)
        n1155 = local read "压力表打印代码据库"() -> (w2721:string[][])
        n1156 = local read "压力表数据库"() -> (w2723:string[][])
        n1157 = call <vilib>:"Clear Errors.vi"("error in (no error)"=w2732) -> ("error out"=w2722:errorcluster)  [unwired: 5 in, 1 out]
        n1158 = call "mess解析.vi"("ValidateBarcode"=w2719, "压力表数据库"=w2723, "压力打印代码据库"=w2721, "输入元素"=w2729, "error in (no error)"=w2722) -> ("长短料"=w2717:string, "压力表有无"=→"压力表有无":string, "衬丝口位置"=w2718:string, "产品型号"=→"产品型号":string, "T/F"=→"T/F":string, "工单号"=→"工单号":string, "压力表类型"=→"压力表类型":string, "工单数量"=→"工单数量":string, "error out"=w2730:errorcluster)  [unwired: 10 in, 4 out]
        "衬丝口位置" <- w2718
        "长短料" <- w2717
        n1159 = case shown="\"假\", 默认" w2717 {
          frame "假", Default {
          }
          frame "短料" {
          }
          frame "长料" {
          }
        }
        n1160 = case shown="\"A\"" w2718 {
          frame "假", Default {
          }
          frame "A" {
          }
          frame "B" {
          }
          frame "C" {
          }
        }
        n1161 = call "KB-EMG Input.vi"("Other Message"="结果显示" ("t"), "EMG Iput"="EMG", "Emg"=FALSE) -> ("String OutPut"=w2735:string)  [unwired: 8 in]
        n1162 = call "Enqueue Element Array.vi"("priority"=w2744, "device error in"=w2730, "queue index"=3, "error in"=w2733, "master data"=w2735, "queue in"=w2741) -> ("error out"=w2746:errorcluster)  [unwired: 4 in, 1 out]
      }
      frame "结果显示" {
        w2781 = u16 0 items=["HPRI"=1, "LPRI"=0] ("priority")
        n1163 = control-ref of="设备状态"() -> (w2774:refnum<vi>)
        n1164 = call "设备状态循环显示.vi"("cmd:"=w2780, "Str引用句柄"=w2774, "新信息输入"=w2773) -> ()  [unwired: 9 in]
        n1165 = local read "字符比对"() -> (w2765:bool)
        n1166 = local read "压力表打印代码"() -> (w2761:string)
        n1167 = case shown="假" w2765 {
          tunnel: ["NG" "OK"] -> w2767
          frame False {
          }
          frame True {
          }
        }
        n1168 = local read "扫码枪字符识别"() -> (w2762:string)
        n1169 = local read "工单号"() -> (w2764:string)
        n1170 = local read "工单数量"() -> (w2763:string)
        n1171 = Concatenate Strings("字符一致性:", w2767) -> (w2766:string)
        "字符一致性连接的字符串" <- w2766
        n1172 = disable-structure shown="禁用" {
          disable-tunnel: w2770 -> [w2791 w2805]
          disable-tunnel: [w2790 w2805] -> w2769
          disable-tunnel: w2766 -> [w2789 _]
          disable-tunnel: w2765 -> [w2788 _]
          disable-tunnel: w2764 -> [w2787 _]
          disable-tunnel: w2763 -> [w2786 _]
          disable-tunnel: w2762 -> [w2785 _]
          disable-tunnel: w2761 -> [w2784 _]
          frame Disabled {
            n1173 = case shown="真" w2788 {
              tunnel: w2787 -> [w2797 w2804]
              tunnel: w2785 -> [w2796 w2803]
              tunnel: w2791 -> [w2794 w2802]
              tunnel: [w2793 w2801] -> w2790
              tunnel: w2789 -> [w2795 w2800]
              tunnel: w2786 -> [_ w2799]
              tunnel: w2784 -> [w2792 w2798]
              frame False {
                n1174 = call "SQL写入 - NG.vi"("WorkNumber"=w2797, "ProductNumber"=w2796, "TestMessage"=w2795, "ProssureType"=w2792, "error in (no error)"=w2794) -> ("error out"=w2793:errorcluster)  [unwired: 9 in, 1 out]
              }
              frame True {
                n1175 = call "SQL写入.vi"("WorkNumber"=w2804, "ProductNumber"=w2803, "TestMessage"=w2800, "ProssureType"=w2798, "error in (no error)"=w2802, "Workorder"=w2799) -> ("error out"=w2801:errorcluster)  [unwired: 8 in, 1 out]
              }
            }
          }
          frame Enabled {
          }
        }
        n1176 = call "KB-EMG Input.vi"("Other Message"="数据传送 " ("t"), "EMG Iput"="EMG", "Emg"=FALSE) -> ("String OutPut"=w2772:string)  [unwired: 8 in]
        n1177 = call "Enqueue Element Array.vi"("priority"=w2781, "device error in"=w2769, "queue index"=3, "error in"=w2770, "master data"=w2772, "queue in"=w2778) -> ("error out"=w2783:errorcluster)  [unwired: 4 in, 1 out]
      }
      frame "数据传送" {
        w2825 = u16 0 items=["HPRI"=1, "LPRI"=0] ("priority")
        n1178 = control-ref of="设备状态"() -> (w2818:refnum<vi>)
        n1179 = call "设备状态循环显示.vi"("cmd:"=w2824, "Str引用句柄"=w2818, "新信息输入"=w2817) -> ()  [unwired: 9 in]
        n1180 = local read "Start Time 3"() -> (w2815:u32)
        n1181 = call "LX-runtime.vi"("Start Time 2"=w2815) -> ("运行时间 2"=→"运行时间 4":dbl)  [unwired: 10 in]
        n1182 = disable-structure shown="启用" {
          disable-tunnel: [w2831 w2839] -> w2811
          disable-tunnel: w2810 -> [w2830 w2840]
          disable-tunnel: w2809 -> [w2829 w2838]
          disable-tunnel: w2808 -> [w2828 w2837]
          frame Disabled {
            n1183 = call "DB5000.X写.vi"("引用"=w2828, "semaphore"=w2829, "地址名称"="电脑1CCD读取字符触发-读" ("组合框"), "value"=FALSE, "error in (no error)"=w2830) -> ("error out"=w2831:errorcluster)  [unwired: 9 in, 1 out]
          }
          frame Enabled {
            n1184 = call "DB5000.X写.vi"("引用"=w2837, "启用延时"=TRUE, "semaphore"=w2838, "地址名称"="电脑1扫码枪触发-读" ("组合框"), "value"=FALSE, "error in (no error)"=w2840) -> ("error out"=w2839:errorcluster)  [unwired: 8 in, 1 out]
          }
        }
        n1185 = local write "字符比对"(FALSE ("字符比对")) -> ()
        n1186 = call "KB-EMG Input.vi"("Other Message"="自动开始" ("t"), "EMG Iput"="EMG", "Emg"=FALSE) -> ("String OutPut"=w2816:string)  [unwired: 8 in]
        n1187 = call "Enqueue Element Array.vi"("priority"=w2825, "queue index"=3, "error in"=w2811, "master data"=w2816, "queue in"=w2822) -> ("error out"=w2827:errorcluster)  [unwired: 5 in, 1 out]
      }
      frame "<-----自动加工结束--------手动部分------->" {
        w2847 = u16 0 items=["HPRI"=1, "LPRI"=0] ("priority")
        # "//读取配置文件"
        n1188 = local read "设备状态"() -> (w2846:string)
        n1189 = Concatenate Strings(w2846, "....." ("字符串"), "\r\n", w2842) -> (w2843:string)
        n1190 = local write "设备状态"(w2843) -> ()
        n1191 = call "Enqueue Element Array.vi"("priority"=w2847, "queue index"=3, "error in"=w2849, "master data"="" ("Element 1"), "queue in"=w2853) -> ("error out"=w2852:errorcluster)  [unwired: 5 in, 1 out]
      }
      frame "Machine Paramter Save Buttom" {
        w2857 = u16 0 items=["HPRI"=1, "LPRI"=0] ("priority")
        n1192 = One Button Dialog(message="确认保存" ("消息")) -> (true=w2855:bool)  [unwired: 1 in]
        n1193 = case shown="真" w2855 {
          frame False {
          }
          frame True {
            n1194 = global read "Global System.vi" "ref path"() -> (w2866:path)
            n1195 = Build Path(base path=w2866, name or relative path="PLC Connect Signal.txt" ("名称或相对路径")) -> (appended path=w2864:path)
            n1196 = call-poly <vilib>:"Write Delimited Spreadsheet.vi"("file path (dialog if empty)"=w2864) -> ()  [unwired: 13 in, 2 out]
          }
        }
        n1197 = call "Enqueue Element Array.vi"("priority"=w2857, "queue index"=3, "error in"=w2859, "master data"="" ("Element 1"), "queue in"=w2862) -> ("error out"=w2861:errorcluster)  [unwired: 5 in, 1 out]
      }
      frame "Other Param Save Buttom" {
        w2871 = u16 0 items=["HPRI"=1, "LPRI"=0] ("priority")
        n1198 = control-ref of="设备状态"() -> (w2867:refnum<vi>)
        n1199 = call "设备状态循环显示.vi"("cmd:"=w2868, "Str引用句柄"=w2867, "新信息输入"=w2870) -> ()  [unwired: 9 in]
        n1200 = call "Enqueue Element Array.vi"("priority"=w2871, "queue index"=3, "error in"=w2873, "master data"="" ("Element 1"), "queue in"=w2876) -> ("error out"=w2875:errorcluster)  [unwired: 5 in, 1 out]
      }
      frame "启动9点校正功能" {
        w2881 = u16 0 items=["HPRI"=1, "LPRI"=0] ("priority")
        n1201 = control-ref of="设备状态"() -> (w2879:refnum<vi>)
        n1202 = call "设备状态循环显示.vi"("Str引用句柄"=w2879, "新信息输入"=w2880) -> ()  [unwired: 10 in]
        n1203 = call "Enqueue Element Array.vi"("priority"=w2881, "queue index"=3, "error in"=w2883, "master data"="" ("Element 1"), "queue in"=w2886) -> ("error out"=w2885:errorcluster)  [unwired: 5 in, 1 out]
      }
      frame "Vision Paramter Save" {
        w2891 = u16 0 items=["HPRI"=1, "LPRI"=0] ("priority")
        n1204 = control-ref of="设备状态"() -> (w2888:refnum<vi>)
        n1205 = call "设备状态循环显示.vi"("cmd:"=w2889, "Str引用句柄"=w2888, "新信息输入"=w2890) -> ()  [unwired: 9 in]
        n1206 = call "Enqueue Element Array.vi"("priority"=w2891, "queue index"=3, "error in"=w2893, "master data"="" ("Element 1"), "queue in"=w2897) -> ("error out"=w2896:errorcluster)  [unwired: 5 in, 1 out]
      }
      frame "*Emergency alarm" {
        w2906 = u16 1 items=["HPRI"=1, "LPRI"=0] ("priority")
        w2907 = u16 0 items=["HPRI"=1, "LPRI"=0] ("priority")
        n1207 = call "Enqueue Element Array.vi"("priority"=w2906, "queue index"=0, "error in"=w2900, "master data"="" ("Element 1"), "queue in"=w2903) -> ("error out"=w2901:errorcluster, "queue out"=w2902:T25)  [unwired: 5 in]
        n1208 = call "SetTestInfoIndex.vi"("test info index"=13) -> ()
        n1209 = call "Enqueue Element Array.vi"("priority"=w2907, "queue index"=3, "error in"=w2901, "master data"="" ("Element 1"), "queue in"=w2902) -> ("error out"=w2911:errorcluster)  [unwired: 5 in, 1 out]
      }
    }
    n1210 = Wait (ms)(milliseconds to wait=w2387) -> ()  [unwired: 1 out]
  }
  n1211 = while {
    shift-right: [w2926] -> w13
    shift-left: w2 -> [w2922]
    shift-right: [w2923] -> _
    shift-left: w14 -> [w2924]
    tunnel: w15 -> [w2916]
    tunnel: w9 -> [w2915]
    tunnel: string[] ["DB5000.136", "DB5000.140", "DB5000.144", "DB5000.148", "DB5000.152", "DB5000.156", "DB5000.160", "DB5000.164", "DB5000.168", "DB5000.172", "DB5000.176"] ("地址数组") -> [w2914]
    tunnel: string[] ["DB5000.00", "DB5000.100", "DB5000.101", "DB5000.102", "DB5000.103", "DB5000.104", "DB5000.105", "DB5000.106", "DB5000.107", "DB5000.108", "DB5000.109", "DB5000.110", "DB5000.111", "DB5000.112", "DB5000.113", "DB5000.114", "DB5000.115", "DB5000.116", "DB5000.117", "DB5000.118", "DB5000.119", "DB5000.120", "DB5000.121", "DB5000.122", "DB5000.123", "DB5000.124", "DB5000.125", "DB5000.126", "DB5000.127", "DB5000.128", "DB5000.129", "DB5000.130", "DB5000.131", "DB5000.132", "DB5000.133", "DB5000.134", "DB5000.200", "DB5000.201", "DB5000.202", "DB5000.203", "DB5000.204", "DB5000.205", "DB5000.206", "DB5000.207", "DB5000.208", "DB5000.209", "DB5000.210", "DB5000.211", "DB5000.212", "DB5000.213", "DB5000.214", "DB5000.215", "DB5000.216", "DB5000.217", "DB5000.218", "DB5000.219", "DB5000.220", "DB5000.221", "DB5000.222", "DB5000.223", "DB5000.225", "DB5000.226", "DB5000.227"] ("地址数组 2") -> [w2913]
    stop <- w2918 stop-if-true
    # "处理部分事件；处理部分弹出窗口（目的是避免在其他循环中因为弹出窗口而影响整个循环的运行）"
    # "主线程-备用"
    n1212 = call "Dequeue Element Array.vi"("queue in"=w2916, "queue index"=5, "error in"=w2922) -> ("queue out"=w2921:T25, "master data"=w2920:string, "secondary data"=w2919:string[], "error out"=w2918:errorcluster)  [unwired: 2 in, 1 out]
    n1213 = case shown="\"No event\", 默认" w2920 {
      tunnel: w2921 -> [_ w2936 w2938 w2948 w2956 w2978 w2990 w2998 w3006 w3014 w3020]
      tunnel: w2918 -> [w2928 w2932 w2942 w2946 w2955 w2976 w2987 w2992 w3002 w3010 w3017]
      tunnel: [w2928 w2935 w2944 w2952 w2960 w2982 w2989 w2997 w3005 w3013 w3028] -> w2926
      tunnel: [50 50 50 50 5 50 50 50 50 50 50] -> w2925
      tunnel: w2924 -> [w2929 w2933 w2939 w2949 w2957 w2979 w2984 w2993 w3003 w3011 w3026]
      tunnel: [w2929 w2933 w2939 w2949 w2957 w2979 w2984 w2993 w3003 w3011 w3026] -> w2923
      tunnel: w2919 -> [_ _ _ _ _ _ _ _ _ _ _]
      tunnel: w2915 -> [_ _ _ _ _ w2973 _ _ _ _ _]
      tunnel: w2914 -> [_ _ _ _ _ w2975 _ _ _ _ _]
      tunnel: w2913 -> [_ _ _ _ _ w2974 _ _ _ _ _]
      frame "No event", Default {
        # "Don't place any functions"
      }
      frame "<----自动加工------------->" {
        w2930 = u16 1 items=["HPRI"=1, "LPRI"=0] ("priority")
        # "//读取配置文件"
        n1214 = call "Enqueue Element Array.vi"("priority"=w2930, "queue index"=5, "error in"=w2932, "master data"="" ("Element 1"), "queue in"=w2936) -> ("error out"=w2935:errorcluster)  [unwired: 5 in, 1 out]
      }
      frame "自动开始" {
        w2940 = u16 1 items=["HPRI"=1, "LPRI"=0] ("priority")
        n1215 = call "Enqueue Element Array.vi"("priority"=w2940, "queue index"=5, "error in"=w2942, "master data"="Loading Variable" ("Element 1"), "queue in"=w2938) -> ("error out"=w2944:errorcluster)  [unwired: 5 in, 1 out]
      }
      frame "Loading Variable" {
        w2950 = u16 1 items=["HPRI"=1, "LPRI"=0] ("priority")
        n1216 = call "Enqueue Element Array.vi"("priority"=w2950, "queue index"=5, "error in"=w2946, "master data"="Open PLC Connect" ("Element 1"), "queue in"=w2948) -> ("error out"=w2952:errorcluster)  [unwired: 5 in, 1 out]
      }
      frame "Open PLC Connect" {
        w2958 = u16 1 items=["HPRI"=1, "LPRI"=0] ("priority")
        n1217 = call "Enqueue Element Array.vi"("priority"=w2958, "queue index"=5, "error in"=w2955, "master data"="R/W PLC Signal" ("Element 1"), "queue in"=w2956) -> ("error out"=w2960:errorcluster)  [unwired: 5 in, 1 out]
      }
      frame "R/W PLC Signal" {
        w2980 = u16 0 items=["HPRI"=1, "LPRI"=0] ("priority")
        n1218 = call "DB5000.W读取.vi"("gInitialSIEMENSS7 In"=w2973, "地址数组"=string[] ["DB5000.228"], "error in (no error)"=w2976) -> ("IsSuccess"=→"DB5000W":bool, "Content"=→"Content":u16, "Message"=→"Message":string, "error out"=w2972:errorcluster)  [unwired: 12 in, 1 out]
        n1219 = call "DB5000.R读取.vi"("gInitialSIEMENSS7 In"=w2973, "地址数组"=w2975, "error in (no error)"=w2972) -> ("IsSuccess"=→"DB5000R-IsSuccess":bool, "DB5000.R"=w2966:T7, "error out"=w2971:errorcluster)  [unwired: 12 in, 2 out]
        n1220 = local write "DB5000.R"(w2966) -> ()
        n1221 = call "DB5000.X读取.vi"("gInitialSIEMENSS7 In"=w2973, "地址数组 2"=w2974, "error in (no error)"=w2971) -> ("IsSuccess"=→"DB5000X-IsSuccess":bool, "IO"=w2962:T36, "error out"=w2963:errorcluster)  [unwired: 11 in, 3 out]
        n1222 = Unbundle By Name(w2962) -> ()  [unwired: 3 out]
        n1223 = local write "DB5000.X"(w2962) -> ()
        n1224 = call "Enqueue Element Array.vi"("priority"=w2980, "device error in"=w2963, "queue index"=5, "error in"=w2976, "master data"="R/W PLC Signal" ("Element 1"), "queue in"=w2978) -> ("error out"=w2982:errorcluster)  [unwired: 4 in, 1 out]
      }
      frame "数据获取" {
        w2985 = u16 0 items=["HPRI"=1, "LPRI"=0] ("priority")
        # "打开TCP连接"
        n1225 = call "Enqueue Element Array.vi"("priority"=w2985, "queue index"=5, "error in"=w2987, "master data"="Updata" ("Element 1"), "queue in"=w2990) -> ("error out"=w2989:errorcluster)  [unwired: 5 in, 1 out]
      }
      frame "Updata" {
        w2995 = u16 0 items=["HPRI"=1, "LPRI"=0] ("priority")
        n1226 = call "Enqueue Element Array.vi"("priority"=w2995, "queue index"=5, "error in"=w2992, "master data"="自动开始", "queue in"=w2998) -> ("error out"=w2997:errorcluster)  [unwired: 5 in, 1 out]
      }
      frame "<-----自动加工结束--------->" {
        w3000 = u16 1 items=["HPRI"=1, "LPRI"=0] ("priority")
        # "//读取配置文件"
        n1227 = call "Enqueue Element Array.vi"("priority"=w3000, "queue index"=5, "error in"=w3002, "master data"="" ("Element 1"), "queue in"=w3006) -> ("error out"=w3005:errorcluster)  [unwired: 5 in, 1 out]
      }
      frame "<----------手动部分------------->" {
        w3008 = u16 1 items=["HPRI"=1, "LPRI"=0] ("priority")
        # "//读取配置文件"
        n1228 = call "Enqueue Element Array.vi"("priority"=w3008, "queue index"=5, "error in"=w3010, "master data"="" ("Element 1"), "queue in"=w3014) -> ("error out"=w3013:errorcluster)  [unwired: 5 in, 1 out]
      }
      frame "*Emergency alarm" {
        w3023 = u16 1 items=["HPRI"=1, "LPRI"=0] ("priority")
        w3024 = u16 1 items=["HPRI"=1, "LPRI"=0] ("priority")
        # "发出处理急停信号的命令"
        # "发出处理急停信号的命令"
        n1229 = call "Enqueue Element Array.vi"("priority"=w3023, "queue index"=0, "error in"=w3017, "master data"="" ("Element 1"), "queue in"=w3020) -> ("error out"=w3018:errorcluster, "queue out"=w3019:T25)  [unwired: 5 in]
        n1230 = call "SetTestInfoIndex.vi"("test info index"=13) -> ()
        n1231 = call "Enqueue Element Array.vi"("priority"=w3024, "queue index"=5, "error in"=w3018, "master data"="" ("Element 1"), "queue in"=w3019) -> ("error out"=w3028:errorcluster)  [unwired: 5 in, 1 out]
      }
    }
    n1232 = Wait (ms)(milliseconds to wait=w2925) -> ()  [unwired: 1 out]
  }
  n1233 = while "While循环" {
    shift-right: [w3046] -> w30
    shift-left: w2 -> [w3042]
    shift-right: [w3043] -> _
    shift-left: w14 -> [w3044]
    tunnel: w15 -> [w3038]
    tunnel: w8 -> [w3032]
    tunnel: w7 -> [w3031]
    tunnel: w1 -> [w3030]
    stop <- w3037 stop-if-true
    # "主线程-表面检测"
    n1234 = call "Dequeue Element Array.vi"("queue in"=w3038, "queue index"=4, "error in"=w3042) -> ("queue out"=w3041:T25, "master data"=w3040:string, "secondary data"=w3039:string[], "error out"=w3037:errorcluster)  [unwired: 2 in, 1 out]
    n1235 = case shown="\"No event\", 默认" w3040 {
      selector: w3040 -> [w3049 _ w3064 w3083 w3102 w3114 w3129 w3142 _ _ _ w3211 w3241 w3258 w3278 w3303 w3316 w3333 w3352 w3424 w3462 w3489 w3505 w3517 _ w3545 w3555 _]
      tunnel: w3041 -> [_ _ w3077 w3093 w3111 w3125 w3139 w3153 w3173 w3183 w3185 w3220 w3251 w3268 w3287 w3312 w3322 w3338 w3357 w3429 w3467 w3496 w3510 w3528 w3537 w3551 w3562 w3568]
      tunnel: w3037 -> [w3051 w3054 w3065 w3081 w3101 w3115 w3127 w3143 w3165 w3179 w3193 w3203 w3242 w3259 w3275 w3290 w3315 w3331 w3349 w3421 w3458 w3479 w3503 w3524 w3534 w3548 w3558 w3565]
      tunnel: [w3051 w3054 w3076 w3092 w3110 w3124 w3138 w3152 w3172 w3182 w3196 w3219 w3250 w3267 w3286 w3311 w3327 w3343 w3362 w3434 w3472 w3501 w3515 w3527 w3536 w3550 w3561 w3576] -> w3046
      tunnel: [50 50 10 10 10 10 10 10 w3168 50 1 5 10 10 5 5 w3323 w3339 w3358 w3430 w3468 w3497 w3511 w3516 50 50 50 50] -> w3045
      tunnel: w3044 -> [w3052 w3055 w3059 w3080 w3099 w3113 w3128 w3141 w3156 w3180 w3187 w3205 w3239 w3256 w3276 w3301 w3314 w3328 w3350 w3422 w3460 w3490 w3502 w3525 w3531 w3544 w3559 w3574]
      tunnel: [w3052 w3055 w3058 w3080 w3099 w3113 w3128 w3141 w3156 w3180 w3187 w3205 w3239 w3256 w3276 w3301 w3314 w3328 w3350 w3422 w3460 w3490 w3502 w3525 w3531 w3544 w3559 w3574] -> w3043
      tunnel: w3039 -> [_ _ _ _ _ _ _ _ _ _ _ _ _ _ _ _ _ _ _ _ _ _ _ _ _ _ _ _]
      tunnel: "表面检测 : " -> [w3048 _ w3066 w3085 w3103 w3121 w3135 w3149 w3162 _ _ w3213 w3244 w3261 w3280 w3305 w3324 w3340 w3359 w3431 w3469 w3498 w3512 _ _ w3543 _ _]
      tunnel: "T3 :" -> [_ _ _ _ _ _ _ _ _ _ _ _ _ _ _ _ _ _ _ _ _ _ _ _ _ _ w3554 _]
      tunnel: 5 -> [_ _ _ _ _ _ _ _ w3168 _ _ _ _ _ _ _ w3323 w3339 w3358 w3430 w3468 w3497 w3511 w3516 _ _ _ _]
      tunnel: w3032 -> [_ _ _ _ _ _ _ _ _ _ _ _ _ _ _ w3288 _ _ w3347 w3410 w3454 w3486 _ _ _ _ _ _]
      tunnel: w3031 -> [_ _ _ _ _ _ _ _ _ _ _ _ _ _ _ w3289 _ _ w3346 w3408 w3455 w3480 _ _ _ _ _ _]
      tunnel: w3030 -> [_ _ _ _ _ _ _ _ _ _ _ _ _ _ _ _ _ _ _ w3405 _ w3473 _ _ _ _ _ _]
      frame "No event", Default {
        # "Don't place any functions"
        n1236 = control-ref of="设备状态"() -> (w3047:refnum<vi>)
        n1237 = call "循环时状态显示.vi"("Str引用句柄"=w3047, "cmd:"=w3048, "新信息输入"=w3049) -> ()  [unwired: 9 in]
      }
      frame "EMG" {
        # "Don't place any functions"
      }
      frame "Loading Variable" {
        w3074 = u16 0 items=["HPRI"=1, "LPRI"=0] ("priority")
        n1238 = control-ref of="设备状态"() -> (w3070:refnum<vi>)
        n1239 = call "设备状态循环显示.vi"("cmd:"=w3066, "Str引用句柄"=w3070, "新信息输入"=w3064) -> ()  [unwired: 9 in]
        n1240 = global read "Global System.vi" "ref path"() -> (w3063:path)
        n1241 = call "Read Config InI.vi"("名称或相对路径"="UserDefine.ini") -> ("ParamSet"=w3073:string[])  [unwired: 14 in, 4 out]
        n1242 = Index Array(array=w3073, index #1=0 ("索引")) -> (element #1=w3056:string)  [unwired: 1 in, 1 out]
        n1243 = Build Path(base path=w3063, name or relative path="Template Program" ("名称或相对路径")) -> (appended path=w3061:path)
        n1244 = Build Path(base path=w3061, name or relative path=w3056) -> (appended path=→"CCD2":path)
        n1245 = global read "Global System.vi" "Paus"() -> (w3068:bool)
        n1246 = call "KB-EMG Input.vi"("Other Message"="Loading Variable Config" ("Element 1"), "EMG Iput"="EMG", "Emg"=w3068) -> ("String OutPut"=w3057:string)  [unwired: 8 in]
        n1247 = Bundle By Name(cluster=w3059, "2 Pause Message"=w3057, "LoadProgram"=w3056) -> (w3058:T21)
        n1248 = call "Enqueue Element Array.vi"("priority"=w3074, "queue index"=4, "error in"=w3065, "master data"=w3057, "queue in"=w3077) -> ("error out"=w3076:errorcluster)  [unwired: 5 in, 1 out]
      }
      frame "Loading Variable Config" {
        w3090 = u16 0 items=["HPRI"=1, "LPRI"=0] ("priority")
        n1249 = control-ref of="设备状态"() -> (w3089:refnum<vi>)
        n1250 = Unbundle By Name(w3080) -> ("LoadProgram"=w3082:string)
        n1251 = call "设备状态循环显示.vi"("cmd:"=w3085, "Str引用句柄"=w3089, "新信息输入"=w3083) -> ()  [unwired: 9 in]
        n1252 = call "读取产品参数信息-CCD3CCD4.vi"("错误输入（无错误）"=w3081, "LoadProductName"=w3082) -> ("错误输出"=w3079:errorcluster)  [unwired: 9 in]
        n1253 = global read "Global System.vi" "Paus"() -> (w3087:bool)
        n1254 = call "KB-EMG Input.vi"("Other Message"="Initial CCD" ("Element 1"), "EMG Iput"="EMG", "Emg"=w3087) -> ("String OutPut"=w3084:string)  [unwired: 8 in]
        n1255 = call "Enqueue Element Array.vi"("priority"=w3090, "device error in"=w3079, "queue index"=4, "error in"=w3081, "master data"=w3084, "queue in"=w3093) -> ("error out"=w3092:errorcluster)  [unwired: 4 in, 1 out]
      }
      frame "Initial CCD" {
        w3108 = u16 0 items=["HPRI"=1, "LPRI"=0] ("priority")
        n1256 = control-ref of="设备状态"() -> (w3107:refnum<vi>)
        n1257 = call "设备状态循环显示.vi"("cmd:"=w3103, "Str引用句柄"=w3107, "新信息输入"=w3102) -> ()  [unwired: 9 in]
        n1258 = call "CR-Initial CameraCCD345.vi"("error in (no error)"=w3101) -> ("error out"=w3100:errorcluster, "Session Out5"=w3097:T28, "Session Out6"=w3095:T28, "Session Out4"=w3096:T28)  [unwired: 7 in]
        n1259 = global write "Global System.vi" "Session Out CCD4"(w3096) -> ()
        n1260 = global write "Global System.vi" "Session Out CCD6"(w3095) -> ()
        n1261 = global write "Global System.vi" "Session Out CCD5"(w3097) -> ()
        n1262 = global read "Global System.vi" "Paus"() -> (w3105:bool)
        n1263 = call "KB-EMG Input.vi"("Other Message"="Open Telnet" ("Element 1"), "EMG Iput"="EMG", "Emg"=w3105) -> ("String OutPut"=w3098:string)  [unwired: 8 in]
        n1264 = call "Enqueue Element Array.vi"("priority"=w3108, "device error in"=w3100, "queue index"=4, "error in"=w3101, "master data"=w3098, "queue in"=w3111) -> ("error out"=w3110:errorcluster)  [unwired: 4 in, 1 out]
      }
      frame "Open Telnet" {
        w3122 = u16 0 items=["HPRI"=1, "LPRI"=0] ("priority")
        n1265 = control-ref of="设备状态"() -> (w3120:refnum<vi>)
        n1266 = call "设备状态循环显示.vi"("cmd:"=w3121, "Str引用句柄"=w3120, "新信息输入"=w3114) -> ()  [unwired: 9 in]
        n1267 = global read "Global System.vi" "Paus"() -> (w3118:bool)
        n1268 = call "KB-EMG Input.vi"("Other Message"="Open VISA" ("master data"), "EMG Iput"="EMG", "Emg"=w3118) -> ("String OutPut"=w3116:string)  [unwired: 8 in]
        n1269 = call "Enqueue Element Array.vi"("priority"=w3122, "queue index"=4, "error in"=w3115, "master data"=w3116, "queue in"=w3125) -> ("error out"=w3124:errorcluster)  [unwired: 5 in, 1 out]
      }
      frame "Open VISA" {
        w3136 = u16 0 items=["HPRI"=1, "LPRI"=0] ("priority")
        n1270 = control-ref of="设备状态"() -> (w3134:refnum<vi>)
        n1271 = call "设备状态循环显示.vi"("cmd:"=w3135, "Str引用句柄"=w3134, "新信息输入"=w3129) -> ()  [unwired: 9 in]
        n1272 = global read "Global System.vi" "Paus"() -> (w3132:bool)
        n1273 = call "KB-EMG Input.vi"("Other Message"="Create File" ("master data"), "EMG Iput"="EMG", "Emg"=w3132) -> ("String OutPut"=w3130:string)  [unwired: 8 in]
        n1274 = call "Enqueue Element Array.vi"("priority"=w3136, "queue index"=4, "error in"=w3127, "master data"=w3130, "queue in"=w3139) -> ("error out"=w3138:errorcluster)  [unwired: 5 in, 1 out]
      }
      frame "Create File" {
        w3150 = u16 0 items=["HPRI"=1, "LPRI"=0] ("priority")
        n1275 = control-ref of="设备状态"() -> (w3148:refnum<vi>)
        n1276 = call "设备状态循环显示.vi"("cmd:"=w3149, "Str引用句柄"=w3148, "新信息输入"=w3142) -> ()  [unwired: 9 in]
        n1277 = global read "Global System.vi" "Paus"() -> (w3146:bool)
        n1278 = call "KB-EMG Input.vi"("Other Message"="Initial-Clear Variable" ("master data"), "EMG Iput"="EMG", "Emg"=w3146) -> ("String OutPut"=w3144:string)  [unwired: 8 in]
        n1279 = call "Enqueue Element Array.vi"("priority"=w3150, "queue index"=4, "error in"=w3143, "master data"=w3144, "queue in"=w3153) -> ("error out"=w3152:errorcluster)  [unwired: 5 in, 1 out]
      }
      frame "Initial-Clear Variable" {
        w3170 = u16 0 items=["HPRI"=1, "LPRI"=0] ("priority")
        n1280 = control-ref of="设备状态"() -> (w3164:refnum<vi>)
        n1281 = call "设备状态循环显示.vi"("cmd:"=w3162, "Str引用句柄"=w3164, "新信息输入"="Initial Finish " ("字符串")) -> ()  [unwired: 9 in]
        n1282 = Current VI's Menubar() -> (w3167:refnum<k9>)
        n1283 = for {
          tunnel: w3167 -> [w3176]
          tunnel: string[] ["登陆"] -> [w3174] mode=indexing
          n1284 = Set Menu Item Info(7:w3174, 9:TRUE ("已启用"), 10:w3174, 11:w3176) -> ()  [unwired: 3 in, 2 out]
        }
        n1285 = property on="User Login" class="Bool (严格)"("DisabledEnum"=T22."Enabled" ("禁用")) -> ()  [unwired: 2 in, 2 out]
        n1286 = global read "Global System.vi" "Paus"() -> (w3160:bool)
        n1287 = local write "表面检测初始化状态"(TRUE ("表面检测初始化状态")) -> ()
        n1288 = global write "Global System.vi" "G_Status 2"(TRUE ("G_Status 1")) -> ()
        n1289 = call "KB-EMG Input.vi"("Other Message"="" ("Element 1"), "EMG Iput"="EMG", "Emg"=w3160) -> ("String OutPut"=w3158:string)  [unwired: 8 in]
        n1290 = call "Enqueue Element Array.vi"("priority"=w3170, "queue index"=4, "error in"=w3165, "master data"=w3158, "queue in"=w3173) -> ("error out"=w3172:errorcluster)  [unwired: 5 in, 1 out]
      }
      frame "<----自动加工------------->" {
        w3177 = u16 0 items=["HPRI"=1, "LPRI"=0] ("priority")
        # "//读取配置文件"
        n1291 = call "Enqueue Element Array.vi"("priority"=w3177, "queue index"=4, "error in"=w3179, "master data"="" ("Element 1"), "queue in"=w3183) -> ("error out"=w3182:errorcluster)  [unwired: 5 in, 1 out]
      }
      frame "自动开始" {
        w3194 = u16 0 items=["HPRI"=1, "LPRI"=0] ("priority")
        n1292 = global write "Global System.vi" "G_Status 2"(TRUE ("G_Status 1")) -> ()
        n1293 = global read "Global System.vi" "Paus"() -> (w3190:bool)
        n1294 = call "KB-EMG Input.vi"("Other Message"="Load Var1", "EMG Iput"="EMG", "Emg"=w3190) -> ("String OutPut"=w3189:string)  [unwired: 8 in]
        n1295 = call "Enqueue Element Array.vi"("priority"=w3194, "queue index"=4, "error in"=w3193, "master data"=w3189, "queue in"=w3185) -> ("error out"=w3196:errorcluster)  [unwired: 5 in, 1 out]
      }
      frame "检测CCD3CCD4启动信号" {
        w3217 = u16 0 items=["HPRI"=1, "LPRI"=0] ("priority")
        n1296 = local read "DB5000.X"() -> (w3200:T4)
        n1297 = control-ref of="设备状态"() -> (w3214:refnum<vi>)
        n1298 = Unbundle By Name(w3200) -> ("电脑1表面检测\n触发-读"=w3199:bool, "表面检测完\n成信号-读"=w3198:bool, "电脑1衬丝检测\n触发-读"=w3197:bool)
        n1299 = call "循环时状态显示 - 3.vi"("Str引用句柄"=w3214, "cmd:"=w3213, "新信息输入"=w3211) -> ()  [unwired: 9 in]
        n1300 = Or(x="表面检测触发", y=w3199) -> (x .or. y?=w3202:bool)
        n1301 = Build Array(w3202, w3198, w3197) -> (w3208:bool[])
        n1302 = call "上升沿检测.vi"("input"=w3202) -> ("output"=w3201:bool)  [unwired: 9 in, 1 out]
        n1303 = Boolean Array To Number(Boolean array=w3208) -> (number=w3207:u32)
        "数字 2" <- w3207
        n1304 = case shown="假" w3201 {
          tunnel: [w3221 w3223] -> w3204
          tunnel: w3203 -> [w3221 w3222]
          frame False {
          }
          frame True {
            n1305 = disable-structure shown="禁用" {
              disable-tunnel: [w3229 _] -> w3224
              disable-tunnel: [w3227 _] -> w3223
              disable-tunnel: w3222 -> [w3226 _]
              frame Disabled {
                n1306 = call "SQL表面型号数据库读取.vi"("error in (no error)"=w3226) -> ("error out"=w3228:errorcluster, "已删除的部分"=w3229:string[], "元素"=w3225:string)  [unwired: 7 in, 1 out]
                n1307 = call "SQL表面型号删除.vi"("Type_c"=w3225, "error in (no error)"=w3228) -> ("error out"=w3227:errorcluster)  [unwired: 13 in]
              }
              frame Enabled {
              }
            }
            "表面产品型号" <- w3224
          }
        }
        n1308 = case shown="真" w3201 {
          frame False {
          }
          frame True {
            n1309 = global write "Global System.vi" "G_Status 2"(TRUE ("G_Status 1")) -> ()
          }
        }
        n1310 = case shown="4" w3207 {
          tunnel: ["检测CCD3CCD4启动信号" ("f") "表面检测启动信号处理" ("EMG Iput") "获取图像" ("f") "衬丝检测信号处理" ("f")] -> w3206
          frame 0, Default {
          }
          frame 2, 3 {
          }
          frame 1 {
          }
          frame 4 {
          }
        }
        n1311 = call "KB-EMG Input.vi"("Other Message"=w3206, "EMG Iput"="EMG", "Emg"=FALSE) -> ("String OutPut"=w3215:string)  [unwired: 8 in]
        n1312 = call "Enqueue Element Array.vi"("priority"=w3217, "device error in"=w3204, "queue index"=4, "error in"=w3203, "master data"=w3215, "queue in"=w3220) -> ("error out"=w3219:errorcluster)  [unwired: 4 in, 1 out]
      }
      frame "表面检测启动信号处理" {
        w3248 = u16 0 items=["HPRI"=1, "LPRI"=0] ("priority")
        # "正面垫片PLC启动信号"
        n1313 = control-ref of="设备状态"() -> (w3245:refnum<vi>)
        n1314 = call "循环时状态显示 - 3.vi"("Str引用句柄"=w3245, "cmd:"=w3244, "新信息输入"=w3241) -> ()  [unwired: 9 in]
        n1315 = Select(t="Load Var2" ("EMG Iput"), s=FALSE, f="获取图像") -> (s? t:f=w3236:string)
        n1316 = call "KB-EMG Input.vi"("Other Message"=w3236, "EMG Iput"="EMG", "Emg"=FALSE) -> ("String OutPut"=w3246:string)  [unwired: 8 in]
        n1317 = call "Enqueue Element Array.vi"("priority"=w3248, "queue index"=4, "error in"=w3242, "master data"=w3246, "queue in"=w3251) -> ("error out"=w3250:errorcluster)  [unwired: 5 in, 1 out]
      }
      frame "衬丝检测信号处理" {
        w3265 = u16 0 items=["HPRI"=1, "LPRI"=0] ("priority")
        n1318 = control-ref of="设备状态"() -> (w3262:refnum<vi>)
        n1319 = call "循环时状态显示 - 3.vi"("Str引用句柄"=w3262, "cmd:"=w3261, "新信息输入"=w3258) -> ()  [unwired: 9 in]
        n1320 = Select(t="Load Var2" ("EMG Iput"), s=FALSE, f="衬丝检测获取图像") -> (s? t:f=w3253:string)
        n1321 = call "KB-EMG Input.vi"("Other Message"=w3253, "EMG Iput"="EMG", "Emg"=FALSE) -> ("String OutPut"=w3263:string)  [unwired: 8 in]
        n1322 = call "Enqueue Element Array.vi"("priority"=w3265, "queue index"=4, "error in"=w3259, "master data"=w3263, "queue in"=w3268) -> ("error out"=w3267:errorcluster)  [unwired: 5 in, 1 out]
      }
      frame "获取图像" {
        w3284 = u16 0 items=["HPRI"=1, "LPRI"=0] ("priority")
        n1323 = control-ref of="设备状态"() -> (w3281:refnum<vi>)
        n1324 = call "循环时状态显示 - 3.vi"("Str引用句柄"=w3281, "cmd:"=w3280, "新信息输入"=w3278) -> ()  [unwired: 9 in]
        n1325 = call "CR-表面检测图像获取.vi"("数值"=39.0, "error in (no error)"=w3275) -> ("iamge4"=→"表面检测相机4":T1, "iamge5"=→"表面检测相机5":T1, "iamge3"=→"表面检测相机3":T1, "error out"=w3274:errorcluster)  [unwired: 10 in]
        n1326 = call "KB-EMG Input.vi"("Other Message"="CCD34图像处理模块", "EMG Iput"="EMG", "Emg"=FALSE) -> ("String OutPut"=w3282:string)  [unwired: 8 in]
        n1327 = call "Enqueue Element Array.vi"("priority"=w3284, "device error in"=w3274, "queue index"=4, "error in"=w3275, "master data"=w3282, "queue in"=w3287) -> ("error out"=w3286:errorcluster)  [unwired: 4 in, 1 out]
      }
      frame "衬丝检测获取图像" {
        w3309 = u16 0 items=["HPRI"=1, "LPRI"=0] ("priority")
        n1328 = control-ref of="设备状态"() -> (w3306:refnum<vi>)
        n1329 = call "循环时状态显示 - 3.vi"("Str引用句柄"=w3306, "cmd:"=w3305, "新信息输入"=w3303) -> ()  [unwired: 9 in]
        n1330 = global read "Global System.vi" "衬丝检测基础参数"() -> (w3298:T30)
        n1331 = call "DB5000.X写.vi"("引用"=w3288, "semaphore"=w3289, "地址名称"="电脑1衬丝检测触发-读" ("组合框"), "value"=FALSE, "error in (no error)"=w3290) -> ("error out"=w3291:errorcluster)  [unwired: 9 in, 1 out]
        n1332 = call "A 侧面 处理函数衬丝检测.vi"("error in (no error)"=w3290, "Session in"=T28 "cam6" ("Session Out CCD4"), "Image Name"="chensi4", "CR-检测基础参数"=w3298) -> ("error out"=w3294:errorcluster, "Session Out"=w3296:T28, "Image out"=→"衬丝检测":T1)  [unwired: 4 in, 1 out]
        n1333 = global write "Global System.vi" "Session Out CCD6"(w3296) -> ()
        n1334 = call "KB-EMG Input.vi"("Other Message"="衬丝检测处理模块", "EMG Iput"="EMG", "Emg"=FALSE) -> ("String OutPut"=w3307:string)  [unwired: 8 in]
        n1335 = call "Enqueue Element Array.vi"("priority"=w3309, "device error in"=w3294, "queue index"=4, "error in"=w3291, "master data"=w3307, "queue in"=w3312) -> ("error out"=w3311:errorcluster)  [unwired: 4 in, 1 out]
      }
      frame "Load Var1" {
        w3325 = u16 0 items=["HPRI"=1, "LPRI"=0] ("priority")
        n1336 = Tick Count (ms)() -> (millisecond timer value=→"Start Time 2":u32)
        n1337 = control-ref of="设备状态"() -> (w3318:refnum<vi>)
        n1338 = call "设备状态循环显示.vi"("cmd:"=w3324, "Str引用句柄"=w3318, "新信息输入"=w3316) -> ()  [unwired: 9 in]
        n1339 = call "KB-EMG Input.vi"("Other Message"="Load Var2" ("t"), "EMG Iput"="EMG", "Emg"=FALSE) -> ("String OutPut"=w3317:string)  [unwired: 8 in]
        n1340 = call "Enqueue Element Array.vi"("priority"=w3325, "queue index"=4, "error in"=w3315, "master data"=w3317, "queue in"=w3322) -> ("error out"=w3327:errorcluster)  [unwired: 5 in, 1 out]
      }
      frame "Load Var2" {
        w3341 = u16 0 items=["HPRI"=1, "LPRI"=0] ("priority")
        n1341 = control-ref of="设备状态"() -> (w3334:refnum<vi>)
        n1342 = call "设备状态循环显示.vi"("cmd:"=w3340, "Str引用句柄"=w3334, "新信息输入"=w3333) -> ()  [unwired: 9 in]
        n1343 = Unbundle By Name(w3328) -> ("LoadProgram"=w3329:string)
        n1344 = call "读取产品参数信息-CCD3CCD4.vi"("错误输入（无错误）"=w3331, "LoadProductName"=w3329) -> ("错误输出"=w3330:errorcluster)  [unwired: 9 in]
        n1345 = call "KB-EMG Input.vi"("Other Message"="检测CCD3CCD4启动信号" ("t"), "EMG Iput"="EMG", "Emg"=FALSE) -> ("String OutPut"=w3332:string)  [unwired: 8 in]
        n1346 = call "Enqueue Element Array.vi"("priority"=w3341, "device error in"=w3330, "queue index"=4, "error in"=w3331, "master data"=w3332, "queue in"=w3338) -> ("error out"=w3343:errorcluster)  [unwired: 4 in, 1 out]
      }
      frame "CCD34图像处理模块" {
        w3360 = u16 0 items=["HPRI"=1, "LPRI"=0] ("priority")
        n1347 = control-ref of="设备状态"() -> (w3353:refnum<vi>)
        n1348 = call "设备状态循环显示.vi"("cmd:"=w3359, "Str引用句柄"=w3353, "新信息输入"=w3352) -> ()  [unwired: 9 in]
        n1349 = stacked-sequence {
          seq-local: [w3363 _ _] -> [_ _ w3398]
          tunnel: w3349 -> [_ w3365 _]
          tunnel: [_ w3375 _] -> w3348
          tunnel: [_ _ w3399] -> _
          tunnel: [_ w3371 _] -> _
          tunnel: w3347 -> [_ w3371 _]
          tunnel: w3346 -> [_ w3370 _]
          frame #0 {
            n1350 = Tick Count (ms)() -> (millisecond timer value=w3363:u32)
          }
          frame #1 {
            n1351 = local read "表面检测相机3"() -> (w3394:T1)
            n1352 = local read "表面检测相机4"() -> (w3393:T1)
            n1353 = local read "表面检测相机5"() -> (w3392:T1)
            n1354 = call "AMX-CCD3 自动处理图像 - 副本.vi"("Image IN"=w3393, "Image Name1"="22", "Image Name2"="2", "error in (no error)"=w3365) -> ("Image Out"=w3391:T1, "error out"=w3390:errorcluster)  [unwired: 7 in, 3 out]
            n1355 = call "AMX-CCD3 自动处理图像 - 副本.vi"("Image IN"=w3394, "Image Name1"="1", "Image Name2"="11", "error in (no error)"=w3365) -> ("Image Out"=w3383:T1, "error out"=w3388:errorcluster)  [unwired: 7 in, 3 out]
            n1356 = call "AMX-CCD3 自动处理图像 - 副本.vi"("Image IN"=w3392, "Image Name1"="3", "Image Name2"="33", "error in (no error)"=w3365) -> ("Image Out"=w3364:T1, "error out"=w3389:errorcluster)  [unwired: 7 in, 3 out]
            n1357 = Merge Errors(w3388, w3390, w3389) -> (w3380:errorcluster)
            n1358 = local write "表面检测相机3"(w3383) -> ()
            n1359 = local write "表面检测相机5"(w3364) -> ()
            n1360 = local write "表面检测相机4"(w3391) -> ()
            n1361 = call "AMX-SaveImage.vi"("基路径"=path "D:/Data/History Image", "CCD Name"="CCD8", "布尔"=TRUE, "Image in"=w3364, "error in (no error)"=w3380, "类型"="CCD8" ("CCD Name")) -> ("error out"=w3374:errorcluster)  [unwired: 9 in]
            n1362 = call "DB5000.X写.vi"("引用"=w3371, "semaphore"=w3370, "地址名称"="表面检测pass-写" ("组合框"), "value"=TRUE, "error in (no error)"=w3374) -> ("引用输出"=w3372:refnum<k24>, "error out"=w3373:errorcluster)  [unwired: 9 in]
            n1363 = call "DB5000.X写.vi"("引用"=w3372, "semaphore"=w3370, "地址名称"="表面检测fail-写" ("组合框"), "value"=FALSE, "error in (no error)"=w3373) -> ("error out"=w3375:errorcluster)  [unwired: 9 in, 1 out]
          }
          frame #2 {
            n1364 = Tick Count (ms)() -> (millisecond timer value=w3399:u32)
            n1365 = Subtract(x=w3399, y=w3398) -> (x-y=w3397:u32)
            n1366 = Divide(x=w3397, y=u32 1000) -> (x/y=→"x/y":dbl)
          }
        }
        n1367 = local read "DB5000.X"() -> (w3345:T4)
        n1368 = Unbundle By Name(w3345) -> ("表面检测完\n成信号-读"=w3344:bool)
        n1369 = case shown="真" w3344 {
          tunnel: ["自动开始" ("t") "数据获取" ("t")] -> w3354
          frame False {
          }
          frame True {
          }
        }
        n1370 = call "KB-EMG Input.vi"("Other Message"=w3354, "EMG Iput"="EMG", "Emg"=FALSE) -> ("String OutPut"=w3351:string)  [unwired: 8 in]
        n1371 = call "Enqueue Element Array.vi"("priority"=w3360, "device error in"=w3348, "queue index"=4, "error in"=w3349, "master data"=w3351, "queue in"=w3357) -> ("error out"=w3362:errorcluster)  [unwired: 4 in, 1 out]
      }
      frame "衬丝检测处理模块" {
        w3432 = u16 0 items=["HPRI"=1, "LPRI"=0] ("priority")
        n1372 = control-ref of="设备状态"() -> (w3425:refnum<vi>)
        n1373 = call "设备状态循环显示.vi"("cmd:"=w3431, "Str引用句柄"=w3425, "新信息输入"=w3424) -> ()  [unwired: 9 in]
        n1374 = local read "衬丝检测"() -> (w3417:T1)
        n1375 = global read "Global System.vi" "CR- 衬丝检测参数"() -> (w3420:T40)
        n1376 = global read "Global System.vi" "CR- 衬丝检测ROI参数"() -> (w3419:T41)
        n1377 = call "CR-衬丝检测处理函数.vi"("Image in"=w3417, "CR- 衬丝检测参数"=w3420, "CR- 衬丝检测ROI参数"=w3419, "error in (no error)"=w3421) -> ("Image out"=w3418:T1, "保护套距离"=w3416:bool, "衬丝有无"=w3415:bool, "error out"=w3411:errorcluster)  [unwired: 5 in, 3 out]
        n1378 = And(x=w3416, y=w3415) -> (x .and. y?=w3406:bool)
        n1379 = local write "衬丝检测"(w3418) -> ()
        n1380 = disable-structure shown="启用" {
          disable-tunnel: w3411 -> [w3447 w3453]
          disable-tunnel: [w3438 w3452] -> w3403
          disable-tunnel: w3410 -> [w3446 w3448]
          disable-tunnel: "衬丝能检测pass-写" ("组合框") -> [w3444 _]
          disable-tunnel: w3408 -> [w3443 w3449]
          disable-tunnel: "衬丝能检测fail-写" ("组合框") -> [w3441 w3451]
          disable-tunnel: w3406 -> [w3436 _]
          disable-tunnel: w3405 -> [w3437 _]
          disable-tunnel: [w3436 _] -> w3404
          frame Enabled {
            n1381 = Not(x=w3436) -> (.not. x?=w3442:bool)
            n1382 = call <vilib>:"Clear Errors.vi"("error in (no error)"=w3447) -> ("error out"=w3435:errorcluster)  [unwired: 5 in, 1 out]
            n1383 = call "DB5000.X写.vi"("引用"=w3446, "semaphore"=w3443, "地址名称"=w3444, "value"=w3436, "error in (no error)"=w3435) -> ("引用输出"=w3445:refnum<k24>, "error out"=w3440:errorcluster)  [unwired: 9 in]
            n1384 = call "DB5000.X写.vi"("引用"=w3445, "semaphore"=w3443, "地址名称"=w3441, "value"=w3442, "error in (no error)"=w3440) -> ("error out"=w3439:errorcluster)  [unwired: 9 in, 1 out]
            n1385 = call "衬丝头检测结果数据库判定.vi"("error in (no error)"=w3439, "衬丝头检测结果"=w3436, "ADODB._Connection In"=w3437) -> ("error out"=w3438:errorcluster)  [unwired: 7 in, 1 out]
          }
          frame Disabled {
            n1386 = call "DB5000.X写.vi"("引用"=w3448, "semaphore"=w3449, "地址名称"=w3451, "value"=TRUE, "error in (no error)"=w3453) -> ("error out"=w3452:errorcluster)  [unwired: 9 in, 1 out]
          }
        }
        n1387 = call "KB-EMG Input.vi"("Other Message"="衬丝检测复位" ("t"), "EMG Iput"="EMG", "Emg"=FALSE) -> ("String OutPut"=w3423:string)  [unwired: 8 in]
        n1388 = call "AMX-SaveImage - 衬丝检测.vi"("基路径"=path "D:/Data/History Image", "CCD Name"="CCD6", "布尔"=TRUE, "结果"=w3404, "Image in"=w3418, "error in (no error)"=w3403) -> ("error out"=w3402:errorcluster)  [unwired: 9 in]
        n1389 = call "Enqueue Element Array.vi"("priority"=w3432, "device error in"=w3402, "queue index"=4, "error in"=w3421, "master data"=w3423, "queue in"=w3429) -> ("error out"=w3434:errorcluster)  [unwired: 4 in, 1 out]
      }
      frame "衬丝检测复位" {
        w3470 = u16 0 items=["HPRI"=1, "LPRI"=0] ("priority")
        n1390 = control-ref of="设备状态"() -> (w3463:refnum<vi>)
        n1391 = call "设备状态循环显示.vi"("cmd:"=w3469, "Str引用句柄"=w3463, "新信息输入"=w3462) -> ()  [unwired: 9 in]
        n1392 = call "DB5000.X写.vi"("引用"=w3454, "semaphore"=w3455, "地址名称"="电脑1衬丝检测触发-读" ("组合框"), "value"=FALSE, "error in (no error)"=w3458) -> ("error out"=w3459:errorcluster)  [unwired: 9 in, 1 out]
        n1393 = call "KB-EMG Input.vi"("Other Message"="自动开始" ("t"), "EMG Iput"="EMG", "Emg"=FALSE) -> ("String OutPut"=w3461:string)  [unwired: 8 in]
        n1394 = call "Enqueue Element Array.vi"("priority"=w3470, "queue index"=4, "error in"=w3459, "master data"=w3461, "queue in"=w3467) -> ("error out"=w3472:errorcluster)  [unwired: 5 in, 1 out]
      }
      frame "数据获取" {
        w3499 = u16 0 items=["HPRI"=1, "LPRI"=0] ("priority")
        n1395 = control-ref of="设备状态"() -> (w3492:refnum<vi>)
        n1396 = call "设备状态循环显示.vi"("cmd:"=w3498, "Str引用句柄"=w3492, "新信息输入"=w3489) -> ()  [unwired: 9 in]
        n1397 = call "DB5000.X写.vi"("引用"=w3486, "semaphore"=w3480, "地址名称"="电脑1表面检测触发-读" ("组合框"), "value"=FALSE, "error in (no error)"=w3479) -> ("引用输出"=w3481:refnum<k24>, "error out"=w3482:errorcluster)  [unwired: 9 in]
        n1398 = call "DB5000.X写.vi"("引用"=w3481, "semaphore"=w3480, "地址名称"="表面检测完成信号-读" ("组合框"), "value"=FALSE, "error in (no error)"=w3482) -> ("error out"=w3483:errorcluster)  [unwired: 9 in, 1 out]
        n1399 = Concatenate Strings("表面检测" ("TestMessage"), ":" ("字符串"), "OK" ("字符串")) -> (w3474:string)
        n1400 = call "SQL写入 - 表面检测.vi"("ADODB._Connection In"=w3473, "TestMessage"=w3474, "error in (no error)"=w3479) -> ("error out"=w3478:errorcluster)  [unwired: 11 in, 1 out]
        n1401 = call "KB-EMG Input.vi"("Other Message"="数据传送" ("t"), "EMG Iput"="EMG", "Emg"=FALSE) -> ("String OutPut"=w3491:string)  [unwired: 8 in]
        n1402 = call "Enqueue Element Array.vi"("priority"=w3499, "device error in"=w3478, "queue index"=4, "error in"=w3483, "master data"=w3491, "queue in"=w3496) -> ("error out"=w3501:errorcluster)  [unwired: 4 in, 1 out]
      }
      frame "数据传送" {
        w3513 = u16 0 items=["HPRI"=1, "LPRI"=0] ("priority")
        n1403 = control-ref of="设备状态"() -> (w3506:refnum<vi>)
        n1404 = call "设备状态循环显示.vi"("cmd:"=w3512, "Str引用句柄"=w3506, "新信息输入"=w3505) -> ()  [unwired: 9 in]
        n1405 = call "KB-EMG Input.vi"("Other Message"="自动开始" ("t"), "EMG Iput"="EMG", "Emg"=FALSE) -> ("String OutPut"=w3504:string)  [unwired: 8 in]
        n1406 = call "Enqueue Element Array.vi"("priority"=w3513, "queue index"=4, "error in"=w3503, "master data"=w3504, "queue in"=w3510) -> ("error out"=w3515:errorcluster)  [unwired: 5 in, 1 out]
      }
      frame "<-----自动加工结束--------手动部分------->" {
        w3522 = u16 0 items=["HPRI"=1, "LPRI"=0] ("priority")
        # "//读取配置文件"
        n1407 = local read "设备状态"() -> (w3521:string)
        n1408 = Concatenate Strings(w3521, "....." ("字符串"), "\r\n", w3517) -> (w3518:string)
        n1409 = local write "设备状态"(w3518) -> ()
        n1410 = call "Enqueue Element Array.vi"("priority"=w3522, "queue index"=4, "error in"=w3524, "master data"="" ("Element 1"), "queue in"=w3528) -> ("error out"=w3527:errorcluster)  [unwired: 5 in, 1 out]
      }
      frame "Machine Paramter Save Buttom" {
        w3532 = u16 0 items=["HPRI"=1, "LPRI"=0] ("priority")
        n1411 = One Button Dialog(message="确认保存" ("消息")) -> (true=w3530:bool)  [unwired: 1 in]
        n1412 = case shown="真" w3530 {
          frame False {
          }
          frame True {
            n1413 = global read "Global System.vi" "ref path"() -> (w3541:path)
            n1414 = Build Path(base path=w3541, name or relative path="PLC Connect Signal.txt" ("名称或相对路径")) -> (appended path=w3539:path)
            n1415 = call-poly <vilib>:"Write Delimited Spreadsheet.vi"("file path (dialog if empty)"=w3539) -> ()  [unwired: 13 in, 2 out]
          }
        }
        n1416 = call "Enqueue Element Array.vi"("priority"=w3532, "queue index"=4, "error in"=w3534, "master data"="" ("Element 1"), "queue in"=w3537) -> ("error out"=w3536:errorcluster)  [unwired: 5 in, 1 out]
      }
      frame "Other Param Save Buttom" {
        w3546 = u16 0 items=["HPRI"=1, "LPRI"=0] ("priority")
        n1417 = control-ref of="设备状态"() -> (w3542:refnum<vi>)
        n1418 = call "设备状态循环显示.vi"("cmd:"=w3543, "Str引用句柄"=w3542, "新信息输入"=w3545) -> ()  [unwired: 9 in]
        n1419 = call "Enqueue Element Array.vi"("priority"=w3546, "queue index"=4, "error in"=w3548, "master data"="" ("Element 1"), "queue in"=w3551) -> ("error out"=w3550:errorcluster)  [unwired: 5 in, 1 out]
      }
      frame "Vision Paramter Save" {
        w3556 = u16 0 items=["HPRI"=1, "LPRI"=0] ("priority")
        n1420 = control-ref of="设备状态"() -> (w3553:refnum<vi>)
        n1421 = call "设备状态循环显示.vi"("cmd:"=w3554, "Str引用句柄"=w3553, "新信息输入"=w3555) -> ()  [unwired: 9 in]
        n1422 = call "Enqueue Element Array.vi"("priority"=w3556, "queue index"=4, "error in"=w3558, "master data"="" ("Element 1"), "queue in"=w3562) -> ("error out"=w3561:errorcluster)  [unwired: 5 in, 1 out]
      }
      frame "*Emergency alarm" {
        w3571 = u16 1 items=["HPRI"=1, "LPRI"=0] ("priority")
        w3572 = u16 0 items=["HPRI"=1, "LPRI"=0] ("priority")
        n1423 = call "Enqueue Element Array.vi"("priority"=w3571, "queue index"=0, "error in"=w3565, "master data"="" ("Element 1"), "queue in"=w3568) -> ("error out"=w3566:errorcluster, "queue out"=w3567:T25)  [unwired: 5 in]
        n1424 = call "SetTestInfoIndex.vi"("test info index"=13) -> ()
        n1425 = call "Enqueue Element Array.vi"("priority"=w3572, "queue index"=4, "error in"=w3566, "master data"="" ("Element 1"), "queue in"=w3567) -> ("error out"=w3576:errorcluster)  [unwired: 5 in, 1 out]
      }
    }
    n1426 = Wait (ms)(milliseconds to wait=w3045) -> ()  [unwired: 1 out]
  }
  n1427 = while "While循环" {
    shift-right: [w3593] -> w12
    shift-left: w2 -> [w3589]
    shift-right: [w3590] -> _
    shift-left: w14 -> [w3591]
    tunnel: w15 -> [w3585]
    tunnel: w8 -> [w3578]
    tunnel: w7 -> [w3579]
    stop <- w3584 stop-if-true
    # "处理部分事件；处理部分弹出窗口（目的是避免在其他循环中因为弹出窗口而影响整个循环的运行）"
    # "主线程-一致性检测"
    n1428 = call "Dequeue Element Array.vi"("queue in"=w3585, "queue index"=8, "error in"=w3589) -> ("queue out"=w3588:T25, "master data"=w3587:string, "secondary data"=w3586:string[], "error out"=w3584:errorcluster)  [unwired: 2 in, 1 out]
    n1429 = case shown="\"检测CCDA启动信号\"" w3587 {
      selector: w3587 -> [_ _ w3604 w3624 w3645 w3658 w3671 w3685 _ _ _ _ w3765 w3781 w3808 w3826 w3845 w3879 w3898 w3909 _ w3937 w3953 w3964 _]
      tunnel: w3588 -> [_ _ w3618 w3634 w3654 w3668 w3682 w3698 w3719 w3729 w3742 w3754 w3774 w3791 w3815 w3833 w3849 w3883 w3902 w3920 w3929 w3943 w3959 w3970 w3975]
      tunnel: w3584 -> [w3595 w3599 w3605 w3622 w3644 w3659 w3672 w3686 w3711 w3725 w3738 w3750 w3763 w3782 w3796 w3825 w3841 w3865 w3891 w3916 w3926 w3940 w3956 w3967 w3972]
      tunnel: [w3595 w3599 w3617 w3633 w3643 w3667 w3681 w3697 w3718 w3728 w3741 w3753 w3773 w3790 w3814 w3838 w3854 w3888 w3907 w3919 w3928 w3942 w3958 w3969 w3983] -> w3593
      tunnel: [50 50 10 10 10 10 10 10 w3714 50 20 30 10 10 10 w3834 w3850 w3884 w3903 w3908 50 50 50 50 50] -> w3592
      tunnel: w3591 -> [w3596 w3600 w3603 w3620 w3642 w3656 w3670 w3684 w3701 w3726 w3732 w3744 w3764 w3780 w3807 w3824 w3843 w3875 w3896 w3917 w3923 w3936 w3949 w3961 w3981]
      tunnel: [w3596 w3600 w3606 w3620 w3642 w3656 w3670 w3684 w3701 w3726 w3732 w3744 w3764 w3780 w3807 w3824 w3843 w3875 w3896 w3917 w3923 w3936 w3948 w3961 w3981] -> w3590
      tunnel: w3586 -> [_ _ _ _ _ _ _ _ _ _ _ _ _ _ _ _ _ _ _ _ _ _ _ _ _]
      tunnel: "一致性检测 : " -> [_ _ w3607 w3626 w3647 w3664 w3678 w3694 w3708 _ _ _ w3767 w3784 w3809 w3835 w3851 w3885 w3904 _ _ w3935 _ w3963 _]
      tunnel: "T4:" -> [_ _ _ _ _ _ _ _ _ _ _ _ _ _ _ _ _ _ _ _ _ _ _ _ _]
      tunnel: 5 -> [_ _ _ _ _ _ _ _ w3714 _ _ _ _ _ _ w3834 w3850 w3884 w3903 w3908 _ _ _ _ _]
      tunnel: w3579 -> [_ _ _ _ _ _ _ _ _ _ _ _ _ _ w3794 _ _ w3856 w3890 _ _ _ _ _ _]
      tunnel: w3578 -> [_ _ _ _ _ _ _ _ _ _ _ _ _ _ w3793 _ _ w3858 w3889 _ _ _ _ _ _]
      frame "No event", Default {
        # "Don't place any functions"
      }
      frame "EMG" {
        # "Don't place any functions"
        n1430 = local write "设备状态"("") -> ()
      }
      frame "Loading Variable" {
        w3615 = u16 0 items=["HPRI"=1, "LPRI"=0] ("priority")
        n1431 = control-ref of="设备状态"() -> (w3611:refnum<vi>)
        n1432 = call "设备状态循环显示.vi"("cmd:"=w3607, "Str引用句柄"=w3611, "新信息输入"=w3604) -> ()  [unwired: 9 in]
        n1433 = call "Read Config InI.vi"("名称或相对路径"="UserDefine.ini") -> ("ParamSet"=w3614:string[])  [unwired: 14 in, 4 out]
        n1434 = Index Array(array=w3614, index #1=0 ("索引")) -> (element #1=w3602:string)  [unwired: 1 in, 1 out]
        n1435 = property on="Auto Run Load Program Name" class="CmbBox"("Value"=w3602) -> ()  [unwired: 2 in, 2 out]
        n1436 = global read "Global System.vi" "Paus"() -> (w3609:bool)
        n1437 = call "KB-EMG Input.vi"("Other Message"="Loading Variable Config" ("Element 1"), "EMG Iput"="EMG", "Emg"=w3609) -> ("String OutPut"=w3601:string)  [unwired: 8 in]
        n1438 = Bundle By Name(cluster=w3603, "2 Pause Message"=w3601) -> (w3606:T21)
        n1439 = call "Enqueue Element Array.vi"("priority"=w3615, "queue index"=8, "error in"=w3605, "master data"=w3601, "queue in"=w3618) -> ("error out"=w3617:errorcluster)  [unwired: 5 in, 1 out]
      }
      frame "Loading Variable Config" {
        w3631 = u16 0 items=["HPRI"=1, "LPRI"=0] ("priority")
        n1440 = control-ref of="设备状态"() -> (w3630:refnum<vi>)
        n1441 = Unbundle By Name(w3620) -> ("LoadProgram"=w3623:string)
        n1442 = call "设备状态循环显示.vi"("cmd:"=w3626, "Str引用句柄"=w3630, "新信息输入"=w3624) -> ()  [unwired: 9 in]
        n1443 = call "读取产品参数信息-CCDA.vi"("错误输入（无错误）"=w3622, "LoadProductName"=w3623) -> ("错误输出"=w3621:errorcluster)  [unwired: 9 in]
        n1444 = global read "Global System.vi" "Paus"() -> (w3628:bool)
        n1445 = call "KB-EMG Input.vi"("Other Message"="Initial CCD" ("Element 1"), "EMG Iput"="EMG", "Emg"=w3628) -> ("String OutPut"=w3625:string)  [unwired: 8 in]
        n1446 = call "Enqueue Element Array.vi"("priority"=w3631, "device error in"=w3621, "queue index"=8, "error in"=w3622, "master data"=w3625, "queue in"=w3634) -> ("error out"=w3633:errorcluster)  [unwired: 4 in, 1 out]
      }
      frame "Initial CCD" {
        w3652 = u16 0 items=["HPRI"=1, "LPRI"=0] ("priority")
        n1447 = control-ref of="设备状态"() -> (w3651:refnum<vi>)
        n1448 = call "设备状态循环显示.vi"("cmd:"=w3647, "Str引用句柄"=w3651, "新信息输入"=w3645) -> ()  [unwired: 9 in]
        n1449 = call "CR-Initial CameraCCDA.vi"("error in (no error)"=w3644) -> ("error out"=w3637:errorcluster, "Session Out"=w3639:T28)  [unwired: 9 in]
        n1450 = property class="IMAQdx"(reference=w3639, error in=w3637, "ActiveAttribute"="ExposureTimeAbs", "ValueI64"=i64 2660) -> (reference out=w3638:T28, error out=w3636:errorcluster)
        n1451 = global read "Global System.vi" "Paus"() -> (w3649:bool)
        n1452 = global write "Global System.vi" "Session Out CCD1"(w3638) -> ()
        n1453 = call "KB-EMG Input.vi"("Other Message"="Open Telnet" ("Element 1"), "EMG Iput"="EMG", "Emg"=w3649) -> ("String OutPut"=w3646:string)  [unwired: 8 in]
        n1454 = call "Enqueue Element Array.vi"("priority"=w3652, "device error in"=w3636, "queue index"=8, "error in"=w3644, "master data"=w3646, "queue in"=w3654) -> ("error out"=w3643:errorcluster)  [unwired: 4 in, 1 out]
      }
      frame "Open Telnet" {
        w3665 = u16 0 items=["HPRI"=1, "LPRI"=0] ("priority")
        n1455 = control-ref of="设备状态"() -> (w3663:refnum<vi>)
        n1456 = call "设备状态循环显示.vi"("cmd:"=w3664, "Str引用句柄"=w3663, "新信息输入"=w3658) -> ()  [unwired: 9 in]
        n1457 = global read "Global System.vi" "Paus"() -> (w3661:bool)
        n1458 = call "KB-EMG Input.vi"("Other Message"="Open VISA" ("master data"), "EMG Iput"="EMG", "Emg"=w3661) -> ("String OutPut"=w3657:string)  [unwired: 8 in]
        n1459 = call "Enqueue Element Array.vi"("priority"=w3665, "queue index"=8, "error in"=w3659, "master data"=w3657, "queue in"=w3668) -> ("error out"=w3667:errorcluster)  [unwired: 5 in, 1 out]
      }
      frame "Open VISA" {
        w3679 = u16 0 items=["HPRI"=1, "LPRI"=0] ("priority")
        n1460 = control-ref of="设备状态"() -> (w3677:refnum<vi>)
        n1461 = call "设备状态循环显示.vi"("cmd:"=w3678, "Str引用句柄"=w3677, "新信息输入"=w3671) -> ()  [unwired: 9 in]
        n1462 = global read "Global System.vi" "Paus"() -> (w3675:bool)
        n1463 = call "KB-EMG Input.vi"("Other Message"="Create File" ("master data"), "EMG Iput"="EMG", "Emg"=w3675) -> ("String OutPut"=w3673:string)  [unwired: 8 in]
        n1464 = call "Enqueue Element Array.vi"("priority"=w3679, "queue index"=8, "error in"=w3672, "master data"=w3673, "queue in"=w3682) -> ("error out"=w3681:errorcluster)  [unwired: 5 in, 1 out]
      }
      frame "Create File" {
        w3695 = u16 0 items=["HPRI"=1, "LPRI"=0] ("priority")
        n1465 = control-ref of="设备状态"() -> (w3693:refnum<vi>)
        n1466 = call "设备状态循环显示.vi"("cmd:"=w3694, "Str引用句柄"=w3693, "新信息输入"=w3685) -> ()  [unwired: 9 in]
        n1467 = global read "Global System.vi" "ref path"() -> (w3688:path)
        n1468 = call "保存判定Title文件.vi"("基路径"=w3688) -> ("路径"=→"路径 2":path)  [unwired: 4 in, 6 out]
        n1469 = global read "Global System.vi" "Paus"() -> (w3691:bool)
        n1470 = call "KB-EMG Input.vi"("Other Message"="Initial-Clear Variable" ("master data"), "EMG Iput"="EMG", "Emg"=w3691) -> ("String OutPut"=w3689:string)  [unwired: 8 in]
        n1471 = call "Enqueue Element Array.vi"("priority"=w3695, "queue index"=8, "error in"=w3686, "master data"=w3689, "queue in"=w3698) -> ("error out"=w3697:errorcluster)  [unwired: 5 in, 1 out]
      }
      frame "Initial-Clear Variable" {
        w3716 = u16 0 items=["HPRI"=1, "LPRI"=0] ("priority")
        n1472 = control-ref of="设备状态"() -> (w3710:refnum<vi>)
        n1473 = call "设备状态循环显示.vi"("cmd:"=w3708, "Str引用句柄"=w3710, "新信息输入"="Initial Finish " ("字符串")) -> ()  [unwired: 9 in]
        n1474 = Current VI's Menubar() -> (w3713:refnum<k9>)
        n1475 = for {
          tunnel: w3713 -> [w3722]
          tunnel: string[] ["登陆"] -> [w3720] mode=indexing
          n1476 = Set Menu Item Info(7:w3720, 9:TRUE ("已启用"), 10:w3720, 11:w3722) -> ()  [unwired: 3 in, 2 out]
        }
        n1477 = property on="User Login" class="Bool (严格)"("DisabledEnum"=T22."Enabled" ("禁用"), "Visible"=TRUE ("可见")) -> ()  [unwired: 2 in, 2 out]
        n1478 = global read "Global System.vi" "Paus"() -> (w3706:bool)
        n1479 = call "KB-EMG Input.vi"("Other Message"="" ("Element 1"), "EMG Iput"="EMG", "Emg"=w3706) -> ("String OutPut"=w3704:string)  [unwired: 8 in]
        n1480 = local write "穿管检测初始化状态"(TRUE ("穿管检测初始化状态")) -> ()
        n1481 = global write "Global System.vi" "G_Status 1"(TRUE ("G_Status 1")) -> ()
        n1482 = call "Enqueue Element Array.vi"("priority"=w3716, "queue index"=8, "error in"=w3711, "master data"=w3704, "queue in"=w3719) -> ("error out"=w3718:errorcluster)  [unwired: 5 in, 1 out]
      }
      frame "<----自动加工------------->" {
        w3723 = u16 0 items=["HPRI"=1, "LPRI"=0] ("priority")
        # "//读取配置文件"
        n1483 = call "Enqueue Element Array.vi"("priority"=w3723, "queue index"=8, "error in"=w3725, "master data"="" ("Element 1"), "queue in"=w3729) -> ("error out"=w3728:errorcluster)  [unwired: 5 in, 1 out]
      }
      frame "自动开始" {
        w3739 = u16 0 items=["HPRI"=1, "LPRI"=0] ("priority")
        n1484 = global write "Global System.vi" "G_Status 1"(TRUE ("G_Status 1")) -> ()
        n1485 = global read "Global System.vi" "Paus"() -> (w3735:bool)
        n1486 = call "KB-EMG Input.vi"("Other Message"="读取配置文件", "EMG Iput"="EMG", "Emg"=w3735) -> ("String OutPut"=w3734:string)  [unwired: 8 in]
        n1487 = call "Enqueue Element Array.vi"("priority"=w3739, "queue index"=8, "error in"=w3738, "master data"=w3734, "queue in"=w3742) -> ("error out"=w3741:errorcluster)  [unwired: 5 in, 1 out]
      }
      frame "读取配置文件" {
        w3751 = u16 0 items=["HPRI"=1, "LPRI"=0] ("priority")
        n1488 = global write "Global System.vi" "G_Status 1"(TRUE ("G_Status 1")) -> ()
        n1489 = call "KB-EMG Input.vi"("Other Message"="Load Var1 ", "EMG Iput"="EMG", "Emg"=FALSE) -> ("String OutPut"=w3746:string)  [unwired: 8 in]
        n1490 = call "Enqueue Element Array.vi"("priority"=w3751, "queue index"=8, "error in"=w3750, "master data"=w3746, "queue in"=w3754) -> ("error out"=w3753:errorcluster)  [unwired: 5 in, 1 out]
      }
      frame "检测CCDA启动信号" {
        w3771 = u16 0 items=["HPRI"=1, "LPRI"=0] ("priority")
        n1491 = control-ref of="设备状态"() -> (w3768:refnum<vi>)
        n1492 = call "循环时状态显示.vi"("Str引用句柄"=w3768, "cmd:"=w3767, "新信息输入"=w3765) -> ()  [unwired: 9 in]
        n1493 = local read "DB5000.X"() -> (w3756:T4)
        n1494 = Unbundle By Name(w3756) -> ("一致性检测\n触发-读"=w3755:bool)
        n1495 = Or(x="CCDA手动触发", y=w3755) -> (x .or. y?=w3761:bool)
        n1496 = Select(t="获取图像" ("f"), s=w3761, f="检测CCDA启动信号") -> (s? t:f=w3760:string)
        n1497 = call "KB-EMG Input.vi"("Other Message"=w3760, "EMG Iput"="EMG", "Emg"=FALSE) -> ("String OutPut"=w3769:string)  [unwired: 8 in]
        n1498 = call "Enqueue Element Array.vi"("priority"=w3771, "queue index"=8, "error in"=w3763, "master data"=w3769, "queue in"=w3774) -> ("error out"=w3773:errorcluster)  [unwired: 5 in, 1 out]
      }
      frame "穿管启动信号处理" {
        w3788 = u16 0 items=["HPRI"=1, "LPRI"=0] ("priority")
        n1499 = control-ref of="设备状态"() -> (w3785:refnum<vi>)
        n1500 = call "循环时状态显示.vi"("Str引用句柄"=w3785, "cmd:"=w3784, "新信息输入"=w3781) -> ()  [unwired: 9 in]
        n1501 = Select(t="Load Var1" ("EMG Iput"), s=FALSE, f="获取图像") -> (s? t:f=w3777:string)
        n1502 = call "KB-EMG Input.vi"("Other Message"=w3777, "EMG Iput"="EMG", "Emg"=FALSE) -> ("String OutPut"=w3786:string)  [unwired: 8 in]
        n1503 = call "Enqueue Element Array.vi"("priority"=w3788, "queue index"=8, "error in"=w3782, "master data"=w3786, "queue in"=w3791) -> ("error out"=w3790:errorcluster)  [unwired: 5 in, 1 out]
      }
      frame "获取图像" {
        w3812 = u16 0 items=["HPRI"=1, "LPRI"=0] ("priority")
        n1504 = control-ref of="设备状态"() -> (w3805:refnum<vi>)
        n1505 = call "循环时状态显示.vi"("Str引用句柄"=w3805, "cmd:"=w3809, "新信息输入"=w3808) -> ()  [unwired: 9 in]
        n1506 = global read "Global System.vi" "CR导丝上料一致性基础参数"() -> (w3802:T30)
        n1507 = global read "Global System.vi" "Session Out CCD1"() -> (w3800:T28)
        n1508 = disable-structure shown="启用" {
          disable-tunnel: w3796 -> [w3821 w3822]
          disable-tunnel: [w3820 w3822] -> w3795
          disable-tunnel: w3794 -> [w3817 _]
          disable-tunnel: w3793 -> [w3816 _]
          frame Disabled {
            n1509 = call "DB5000.X写.vi"("引用"=w3816, "semaphore"=w3817, "地址名称"="一致性检测触发-读" ("组合框"), "value"=FALSE, "error in (no error)"=w3821) -> ("error out"=w3820:errorcluster)  [unwired: 9 in, 1 out]
          }
          frame Enabled {
          }
        }
        n1510 = call "AMX-CCDA获取图像.vi"("Session Out CCD2"=w3800, "error in (no error)"=w3796, "Image Name"="A1", "ParamsUI"=w3802) -> ("error out"=w3799:errorcluster, "Session Out"=w3801:T28, "Image out"=→"相机A":T1)  [unwired: 4 in, 1 out]
        n1511 = global write "Global System.vi" "Session Out CCD1"(w3801) -> ()
        n1512 = local write "CCDA手动触发"(FALSE ("CCDA手动触发")) -> ()
        n1513 = call "KB-EMG Input.vi"("Other Message"="CCDA图像处理模块" ("EMG Iput"), "EMG Iput"="EMG", "Emg"=FALSE) -> ("String OutPut"=w3810:string)  [unwired: 8 in]
        n1514 = call "Enqueue Element Array.vi"("priority"=w3812, "device error in"=w3799, "queue index"=8, "error in"=w3795, "master data"=w3810, "queue in"=w3815) -> ("error out"=w3814:errorcluster)  [unwired: 4 in, 1 out]
      }
      frame "Load Var1" {
        w3836 = u16 0 items=["HPRI"=1, "LPRI"=0] ("priority")
        n1515 = control-ref of="设备状态"() -> (w3828:refnum<vi>)
        n1516 = call "设备状态循环显示.vi"("cmd:"=w3835, "Str引用句柄"=w3828, "新信息输入"=w3826) -> ()  [unwired: 9 in]
        n1517 = global read "Global System.vi" "ref path"() -> (w3832:path)
        n1518 = call "保存判定Title文件.vi"("基路径"=w3832) -> ("路径"=w3831:path)  [unwired: 4 in, 6 out]
        n1519 = property on="路径 2" class="Path"("Value"=w3831) -> ()  [unwired: 2 in, 2 out]
        n1520 = call "KB-EMG Input.vi"("Other Message"="Load Var2" ("t"), "EMG Iput"="EMG", "Emg"=FALSE) -> ("String OutPut"=w3827:string)  [unwired: 8 in]
        n1521 = call "Enqueue Element Array.vi"("priority"=w3836, "queue index"=8, "error in"=w3825, "master data"=w3827, "queue in"=w3833) -> ("error out"=w3838:errorcluster)  [unwired: 5 in, 1 out]
      }
      frame "Load Var2" {
        w3852 = u16 0 items=["HPRI"=1, "LPRI"=0] ("priority")
        n1522 = control-ref of="设备状态"() -> (w3846:refnum<vi>)
        n1523 = call "设备状态循环显示.vi"("cmd:"=w3851, "Str引用句柄"=w3846, "新信息输入"=w3845) -> ()  [unwired: 9 in]
        n1524 = Unbundle By Name(w3843) -> ("LoadProgram"=w3842:string)
        n1525 = call "读取产品参数信息-CCDA.vi"("错误输入（无错误）"=w3841, "LoadProductName"=w3842) -> ("错误输出"=w3840:errorcluster)  [unwired: 9 in]
        n1526 = call "KB-EMG Input.vi"("Other Message"="检测CCDA启动信号" ("t"), "EMG Iput"="EMG", "Emg"=FALSE) -> ("String OutPut"=w3844:string)  [unwired: 8 in]
        n1527 = call "Enqueue Element Array.vi"("priority"=w3852, "device error in"=w3840, "queue index"=8, "error in"=w3841, "master data"=w3844, "queue in"=w3849) -> ("error out"=w3854:errorcluster)  [unwired: 4 in, 1 out]
      }
      frame "CCDA图像处理模块" {
        w3886 = u16 0 items=["HPRI"=1, "LPRI"=0] ("priority")
        n1528 = control-ref of="设备状态"() -> (w3880:refnum<vi>)
        n1529 = call "设备状态循环显示.vi"("cmd:"=w3885, "Str引用句柄"=w3880, "新信息输入"=w3879) -> ()  [unwired: 9 in]
        n1530 = local read "相机A"() -> (w3877:T1)
        n1531 = global read "Global System.vi" "CR位置范围设定"() -> (w3874:T42)
        n1532 = global read "Global System.vi" "CR导丝上料一致性参数"() -> (w3873:T45)
        n1533 = call "DB5000.X写.vi"("引用"=w3858, "semaphore"=w3856, "地址名称"="一致性检测触发-读" ("组合框"), "value"=FALSE) -> ("引用输出"=w3857:refnum<k24>)  [unwired: 10 in, 1 out]
        n1534 = call "CR-导丝上料一致性处理函数.vi"("error in (no error)"=w3865, "导丝上料一致性参数"=w3873, "位置范围设定"=w3874, "Image in"=w3877) -> ("error out"=w3863:errorcluster, "一致性结果字符串"=w3871:string, "Image out"=w3876:T1)  [unwired: 4 in, 1 out]
        "一致性结果字符串" <- w3871
        n1535 = call "一致性结果转换.vi"("一致性结果字符串"=w3871) -> ("数字"=w3866:u16)  [unwired: 10 in]
        n1536 = local write "相机A"(w3876) -> ()
        n1537 = call "DB5000.W写.vi"("gInitialSIEMENSS7 In"=w3857, "地址数组"=string[] ["DB5000.228"], "value"=w3866, "error in (no error)"=w3863) -> ("error out"=w3862:errorcluster)  [unwired: 14 in, 1 out]
        n1538 = call "KB-EMG Input.vi"("Other Message"="结果显示" ("t"), "EMG Iput"="EMG", "Emg"=FALSE) -> ("String OutPut"=w3878:string)  [unwired: 8 in]
        n1539 = call "AMX-SaveImage.vi"("基路径"=path "D:/Data/History Image", "CCD Name"="CCD9", "布尔"=TRUE, "结果"=TRUE, "Image in"=w3876, "error in (no error)"=w3862, "类型"="CCD9" ("CCD Name")) -> ("error out"=w3861:errorcluster)  [unwired: 8 in]
        n1540 = call "Enqueue Element Array.vi"("priority"=w3886, "queue index"=8, "error in"=w3861, "master data"=w3878, "queue in"=w3883) -> ("error out"=w3888:errorcluster)  [unwired: 5 in, 1 out]
      }
      frame "结果显示" {
        w3905 = u16 0 items=["HPRI"=1, "LPRI"=0] ("priority")
        n1541 = control-ref of="设备状态"() -> (w3899:refnum<vi>)
        n1542 = call "设备状态循环显示.vi"("cmd:"=w3904, "Str引用句柄"=w3899, "新信息输入"=w3898) -> ()  [unwired: 9 in]
        n1543 = call "DB5000.X写.vi"("引用"=w3889, "semaphore"=w3890, "地址名称"="一致性检测触发-读" ("组合框"), "value"=FALSE, "error in (no error)"=w3891) -> ("error out"=w3892:errorcluster)  [unwired: 9 in, 1 out]
        n1544 = call "KB-EMG Input.vi"("Other Message"="自动开始" ("t"), "EMG Iput"="EMG", "Emg"=FALSE) -> ("String OutPut"=w3897:string)  [unwired: 8 in]
        n1545 = call "Enqueue Element Array.vi"("priority"=w3905, "queue index"=8, "error in"=w3892, "master data"=w3897, "queue in"=w3902) -> ("error out"=w3907:errorcluster)  [unwired: 5 in, 1 out]
      }
      frame "<-----自动加工结束--------手动部分------->" {
        w3914 = u16 0 items=["HPRI"=1, "LPRI"=0] ("priority")
        # "//读取配置文件"
        n1546 = local read "设备状态"() -> (w3913:string)
        n1547 = Concatenate Strings(w3913, "....." ("字符串"), "\r\n", w3909) -> (w3910:string)
        n1548 = local write "设备状态"(w3910) -> ()
        n1549 = call "Enqueue Element Array.vi"("priority"=w3914, "queue index"=8, "error in"=w3916, "master data"="" ("Element 1"), "queue in"=w3920) -> ("error out"=w3919:errorcluster)  [unwired: 5 in, 1 out]
      }
      frame "Machine Paramter Save Buttom" {
        w3924 = u16 0 items=["HPRI"=1, "LPRI"=0] ("priority")
        n1550 = One Button Dialog(message="确认保存" ("消息")) -> (true=w3922:bool)  [unwired: 1 in]
        n1551 = case shown="真" w3922 {
          frame False {
          }
          frame True {
            n1552 = global read "Global System.vi" "ref path"() -> (w3933:path)
            n1553 = Build Path(base path=w3933, name or relative path="PLC Connect Signal.txt" ("名称或相对路径")) -> (appended path=w3931:path)
            n1554 = call-poly <vilib>:"Write Delimited Spreadsheet.vi"("file path (dialog if empty)"=w3931) -> ()  [unwired: 13 in, 2 out]
          }
        }
        n1555 = call "Enqueue Element Array.vi"("priority"=w3924, "queue index"=8, "error in"=w3926, "master data"="" ("Element 1"), "queue in"=w3929) -> ("error out"=w3928:errorcluster)  [unwired: 5 in, 1 out]
      }
      frame "Other Param Save Buttom" {
        w3938 = u16 0 items=["HPRI"=1, "LPRI"=0] ("priority")
        n1556 = control-ref of="设备状态"() -> (w3934:refnum<vi>)
        n1557 = call "设备状态循环显示.vi"("cmd:"=w3935, "Str引用句柄"=w3934, "新信息输入"=w3937) -> ()  [unwired: 9 in]
        n1558 = call "Enqueue Element Array.vi"("priority"=w3938, "queue index"=8, "error in"=w3940, "master data"="" ("Element 1"), "queue in"=w3943) -> ("error out"=w3942:errorcluster)  [unwired: 5 in, 1 out]
      }
      frame "Reset Static" {
        w3946 = "0" ("TotalNumber")
        w3954 = u16 0 items=["HPRI"=1, "LPRI"=0] ("priority")
        n1559 = control-ref of="设备状态"() -> (w3945:refnum<vi>)
        n1560 = call "设备状态循环显示.vi"("Str引用句柄"=w3945, "新信息输入"=w3953) -> ()  [unwired: 10 in]
        n1561 = Initialize Array("0", 3 ("维数大小")) -> (w3947:string[])
        n1562 = call "3D-ResetTotalNumber.vi"("Inputs_BaseParam"=w3947, "名称或相对路径"="UserDefine.ini") -> ()  [unwired: 10 in]
        n1563 = Bundle By Name(cluster=w3949, "TotalNumber"=w3946, "PassNumber"=w3946, "FailNumber"=w3946) -> (w3948:T21)
        n1564 = call "Enqueue Element Array.vi"("priority"=w3954, "queue index"=8, "error in"=w3956, "master data"="" ("Element 1"), "queue in"=w3959) -> ("error out"=w3958:errorcluster)  [unwired: 5 in, 1 out]
      }
      frame "Clear" {
        w3965 = u16 0 items=["HPRI"=1, "LPRI"=0] ("priority")
        n1565 = control-ref of="设备状态"() -> (w3962:refnum<vi>)
        n1566 = call "设备状态循环显示.vi"("cmd:"=w3963, "Str引用句柄"=w3962, "新信息输入"=w3964) -> ()  [unwired: 9 in]
        n1567 = call "Enqueue Element Array.vi"("priority"=w3965, "queue index"=8, "error in"=w3967, "master data"="" ("Element 1"), "queue in"=w3970) -> ("error out"=w3969:errorcluster)  [unwired: 5 in, 1 out]
      }
      frame "*Emergency alarm" {
        w3978 = u16 1 items=["HPRI"=1, "LPRI"=0] ("priority")
        w3979 = u16 0 items=["HPRI"=1, "LPRI"=0] ("priority")
        n1568 = call "Enqueue Element Array.vi"("priority"=w3978, "queue index"=0, "error in"=w3972, "master data"="" ("Element 1"), "queue in"=w3975) -> ("error out"=w3973:errorcluster, "queue out"=w3974:T25)  [unwired: 5 in]
        n1569 = call "Enqueue Element Array.vi"("priority"=w3979, "queue index"=8, "error in"=w3973, "master data"="" ("Element 1"), "queue in"=w3974) -> ("error out"=w3983:errorcluster)  [unwired: 5 in, 1 out]
      }
    }
    n1570 = Wait (ms)(milliseconds to wait=w3592) -> ()  [unwired: 1 out]
  }
  n1571 = while {
    shift-right: [w4000] -> w31
    shift-left: w2 -> [w3996]
    shift-right: [w3997] -> _
    shift-left: w14 -> [w3998]
    tunnel: w15 -> [w3992]
    tunnel: w17 -> [w3989]
    shift-right: [w3987] -> _
    shift-left: dbl[][] [] ("数组in") -> [w3988]
    shift-right: [w3985] -> _
    shift-left: dbl[][] [] ("夹爪数组out") -> [w3986]
    tunnel: w8 -> [_]
    tunnel: w7 -> [_]
    stop <- w3991 stop-if-true
    # "处理部分事件；处理部分弹出窗口（目的是避免在其他循环中因为弹出窗口而影响整个循环的运行）"
    # "主线程-穿管压力检测"
    n1572 = call "Dequeue Element Array.vi"("queue in"=w3992, "queue index"=7, "error in"=w3996) -> ("queue out"=w3995:T25, "master data"=w3994:string, "secondary data"=w3993:string[], "error out"=w3991:errorcluster)  [unwired: 2 in, 1 out]
    n1573 = case shown="\"R/W PLC Signal\"" w3994 {
      tunnel: w3995 -> [_ w4014 w4018 w4032 w4047 w4082 w4110 w4120 w4130 w4140 w4148]
      tunnel: w3991 -> [w4004 w4010 w4022 w4030 w4046 w4077 w4107 w4114 w4126 w4136 w4145]
      tunnel: [w4004 w4013 w4024 w4036 w4051 w4086 w4109 w4119 w4129 w4139 w4156] -> w4000
      tunnel: [5 5 5 5 5 40 5 5 5 5 5] -> w3999
      tunnel: w3998 -> [w4005 w4011 w4019 w4033 w4048 w4083 w4104 w4115 w4127 w4137 w4154]
      tunnel: [w4005 w4011 w4019 w4033 w4048 w4083 w4104 w4115 w4127 w4137 w4154] -> w3997
      tunnel: w3993 -> [_ _ _ _ _ _ _ _ _ _ _]
      tunnel: w3989 -> [_ _ _ _ _ _ _ _ _ _ _]
      tunnel: w3988 -> [w4001 w4006 w4017 w4028 w4045 w4076 _ w4113 w4122 w4132 w4142]
      tunnel: [w4001 w4006 w4017 w4028 w4045 w4075 w4103 w4113 w4122 w4132 w4142] -> w3987
      tunnel: w3986 -> [w4002 w4007 w4016 w4027 w4044 w4079 _ w4112 w4123 w4133 w4143]
      tunnel: [w4002 w4007 w4016 w4027 w4044 w4078 w4103 w4112 w4123 w4133 w4143] -> w3985
      frame "No event", Default {
        # "Don't place any functions"
      }
      frame "<----自动加工------------->" {
        w4008 = u16 1 items=["HPRI"=1, "LPRI"=0] ("priority")
        # "//读取配置文件"
        n1574 = call "Enqueue Element Array.vi"("priority"=w4008, "queue index"=7, "error in"=w4010, "master data"="" ("Element 1"), "queue in"=w4014) -> ("error out"=w4013:errorcluster)  [unwired: 5 in, 1 out]
      }
      frame "自动开始" {
        w4020 = u16 1 items=["HPRI"=1, "LPRI"=0] ("priority")
        n1575 = call "Enqueue Element Array.vi"("priority"=w4020, "queue index"=7, "error in"=w4022, "master data"="Loading Variable" ("Element 1"), "queue in"=w4018) -> ("error out"=w4024:errorcluster)  [unwired: 5 in, 1 out]
      }
      frame "Loading Variable" {
        w4034 = u16 1 items=["HPRI"=1, "LPRI"=0] ("priority")
        n1576 = disable-structure shown="禁用" {
          disable-tunnel: w4030 -> [w4041 _]
          disable-tunnel: [w4040 _] -> w4029
          frame Disabled {
            n1577 = call "Initial7230.vi"("error in (no error)"=w4041) -> ("error out"=w4040:errorcluster, "task out Output"=→"task out Output":refnum<k7>, "task out Input"=→"task out Input":refnum<k7>)  [unwired: 8 in]
          }
          frame Enabled {
          }
        }
        n1578 = local write "穿管压力获取初始化状态"(TRUE ("穿管压力获取初始化状态")) -> ()
        n1579 = call "Enqueue Element Array.vi"("priority"=w4034, "device error in"=w4029, "queue index"=7, "error in"=w4030, "master data"="Open PLC Connect" ("Element 1"), "queue in"=w4032) -> ("error out"=w4036:errorcluster)  [unwired: 4 in, 1 out]
      }
      frame "Open PLC Connect" {
        w4042 = dbl[] [0.0, 0.0, 0.0, 0.0, 0.0, 0.0, 0.0, 0.0, 0.0, 0.0, 0.0, 0.0, 0.0, 0.0, 0.0, 0.0, 0.0, 0.0, 0.0] ("盘管压力值")
        w4049 = u16 1 items=["HPRI"=1, "LPRI"=0] ("priority")
        n1580 = local write "盘管压力值 2"(w4042) -> ()
        n1581 = local write "夹爪压力值"(w4042) -> ()
        n1582 = call "Enqueue Element Array.vi"("priority"=w4049, "queue index"=7, "error in"=w4046, "master data"="R/W PLC Signal" ("Element 1"), "queue in"=w4047) -> ("error out"=w4051:errorcluster)  [unwired: 5 in, 1 out]
      }
      frame "R/W PLC Signal" {
        w4084 = u16 1 items=["HPRI"=1, "LPRI"=0] ("priority")
        n1583 = local read "DB5000.R"() -> (w4054:T7)
        n1584 = local read "DB5000.X"() -> (w4053:T4)
        n1585 = Unbundle By Name(w4053) -> ("电脑1压力获取\n触发-读"=w4056:bool)
        n1586 = Unbundle By Name(w4054) -> ("盘管底部压力值"=w4055:sgl)
        n1587 = control-ref of="设备状态"() -> (w4081:refnum<vi>)
        n1588 = call "UPdataMessage.vi"("错误输入（无错误）"=w4077, "Str引用句柄"=w4081) -> ("error out"=w4074:errorcluster)  [unwired: 9 in]
        n1589 = Subtract(x=w4055, y="补偿值") -> (x-y=w4073:dbl)
        "补偿后压力值" <- w4073
        n1590 = Build Array(w4055) -> (w4071:sgl[])
        n1591 = call "数据收集.vi"("error in (no error)"=w4077, "DB5000.X"=w4053, "Value"=w4073, "数组in"=w4076) -> ("error out"=w4068:errorcluster, "添加的数组"=→"盘管压力值 2":dbl[], "连接的字符串"=w4063:string, "数组out"=w4075:dbl[][])  [unwired: 4 in]
        "连接的字符串" <- w4063
        n1592 = Decimal String To Number(string=w4063) -> (number=w4064:i32)  [unwired: 2 in, 1 out]
        n1593 = case shown="真" w4056 {
          tunnel: w4071 -> [_ w4093]
          tunnel: [_ w4092] -> w4066
          tunnel: [_ w4091] -> w4065
          tunnel: w4064 -> [_ _]
          frame False {
          }
          frame True {
            n1594 = disable-structure shown="启用" {
              disable-tunnel: w4093 -> [w4096 _]
              frame Disabled {
                n1595 = call-poly <vilib>:"Write Delimited Spreadsheet.vi"("file path (dialog if empty)"=path "C:/Users/Administrator/Desktop/新建文本文档.txt", "format (%.3f)"="%.6f", "1D data"=w4096, "append to file? (new file:F)"=FALSE) -> ()  [unwired: 10 in, 2 out]
              }
              frame Enabled {
              }
            }
            n1596 = disable-structure shown="禁用" {
              disable-tunnel: [w4102 _] -> w4092
              disable-tunnel: [w4101 _] -> w4091
              disable-tunnel: "C0C01B2473005" ("barcode") -> [w4100 _]
              disable-tunnel: 34455.0 ("夹持力") -> [w4099 _]
              disable-tunnel: 111111.0 ("夹持力") -> [w4098 _]
              frame Disabled {
                n1597 = call "mess压力数据上传.vi"("夹持力"=w4099, "压力"=w4098, "barcode"=w4100) -> ("ValidateBarcode"=w4102:string, "数据上传OK/NG"=w4101:bool)  [unwired: 10 in, 1 out]
              }
              frame Enabled {
              }
            }
          }
        }
        "数据上传OK/NG 2" <- w4065
        "ValidateBarcode 3" <- w4066
        n1598 = call "ClearErr.vi"("error in (no error)"=w4068, "运行位置"="穿管压力检测") -> ("error out"=w4059:errorcluster)  [unwired: 9 in]
        n1599 = call <vilib>:"Clear Errors.vi"("error in (no error)"=w4059) -> ("error out"=w4057:errorcluster)  [unwired: 5 in, 1 out]
        n1600 = call "夹爪压力保存.vi"("error in (no error)"=w4057, "DB5000.R"=w4054, "DB5000.X"=w4053, "夹爪数组in"=w4079) -> ("字符串"=w4062:string, "夹爪压力值"=→"夹爪压力值":dbl[], "夹爪数组out"=w4078:dbl[][], "error out"=w4058:errorcluster)  [unwired: 3 in, 1 out]
        "字符串" <- w4062
        n1601 = Concatenate Strings(w4063, w4062) -> (w4061:string)
        n1602 = Fract/Exp String To Number(string=w4061) -> (number=→"数字 3":dbl)  [unwired: 3 in, 1 out]
        n1603 = call "Enqueue Element Array.vi"("priority"=w4084, "device error in"=w4058, "queue index"=7, "error in"=w4074, "master data"="R/W PLC Signal" ("Element 1"), "queue in"=w4082) -> ("error out"=w4086:errorcluster)  [unwired: 4 in, 1 out]
      }
      frame "清除状态信息" {
        w4103 = dbl[][] [[0.0, 0.0, 0.0, 0.0, 0.0, 0.0, 0.0, 0.0, 0.0, 0.0, 0.0, 0.0, 0.0, 0.0, 0.0, 0.0, 0.0, 0.0, 0.0]] ("盘管压力值")
        w4105 = u16 0 items=["HPRI"=1, "LPRI"=0] ("priority")
        # "打开TCP连接"
        n1604 = call "Enqueue Element Array.vi"("priority"=w4105, "queue index"=7, "error in"=w4107, "master data"="R/W PLC Signal" ("Element 1"), "queue in"=w4110) -> ("error out"=w4109:errorcluster)  [unwired: 5 in, 1 out]
      }
      frame "Updata" {
        w4117 = u16 0 items=["HPRI"=1, "LPRI"=0] ("priority")
        n1605 = call "Enqueue Element Array.vi"("priority"=w4117, "queue index"=7, "error in"=w4114, "master data"="自动开始", "queue in"=w4120) -> ("error out"=w4119:errorcluster)  [unwired: 5 in, 1 out]
      }
      frame "<-----自动加工结束--------->" {
        w4124 = u16 1 items=["HPRI"=1, "LPRI"=0] ("priority")
        # "//读取配置文件"
        n1606 = call "Enqueue Element Array.vi"("priority"=w4124, "queue index"=7, "error in"=w4126, "master data"="" ("Element 1"), "queue in"=w4130) -> ("error out"=w4129:errorcluster)  [unwired: 5 in, 1 out]
      }
      frame "<----------手动部分------------->" {
        w4134 = u16 1 items=["HPRI"=1, "LPRI"=0] ("priority")
        # "//读取配置文件"
        n1607 = call "Enqueue Element Array.vi"("priority"=w4134, "queue index"=7, "error in"=w4136, "master data"="" ("Element 1"), "queue in"=w4140) -> ("error out"=w4139:errorcluster)  [unwired: 5 in, 1 out]
      }
      frame "*Emergency alarm" {
        w4151 = u16 1 items=["HPRI"=1, "LPRI"=0] ("priority")
        w4152 = u16 1 items=["HPRI"=1, "LPRI"=0] ("priority")
        # "发出处理急停信号的命令"
        # "发出处理急停信号的命令"
        n1608 = call "Enqueue Element Array.vi"("priority"=w4151, "queue index"=0, "error in"=w4145, "master data"="" ("Element 1"), "queue in"=w4148) -> ("error out"=w4146:errorcluster, "queue out"=w4147:T25)  [unwired: 5 in]
        n1609 = call "SetTestInfoIndex.vi"("test info index"=13) -> ()
        n1610 = call "Enqueue Element Array.vi"("priority"=w4152, "queue index"=7, "error in"=w4146, "master data"="" ("Element 1"), "queue in"=w4147) -> ("error out"=w4156:errorcluster)  [unwired: 5 in, 1 out]
      }
    }
    n1611 = Wait (ms)(milliseconds to wait=w3999) -> ()  [unwired: 1 out]
  }
  n1612 = while {
    shift-right: [w4173] -> w24
    shift-left: w2 -> [w4169]
    shift-right: [w4170] -> _
    shift-left: w14 -> [w4171]
    tunnel: w15 -> [w4165]
    tunnel: w26 -> [w4162]
    tunnel: w17 -> [w4161]
    tunnel: w1 -> [w4160]
    tunnel: w9 -> [w4159]
    tunnel: w7 -> [w4158]
    stop <- w4164 stop-if-true
    # "处理部分事件；处理部分弹出窗口（目的是避免在其他循环中因为弹出窗口而影响整个循环的运行）"
    # "主线程-与PLC链接状态"
    n1613 = call "Dequeue Element Array.vi"("queue in"=w4165, "queue index"=1, "error in"=w4169) -> ("queue out"=w4168:T25, "master data"=w4167:string, "secondary data"=w4166:string[], "error out"=w4164:errorcluster)  [unwired: 2 in, 1 out]
    n1614 = case shown="\"清除状态信息\"" w4167 {
      tunnel: w4168 -> [_ w4183 w4185 w4196 w4208 w4230 w4305 w4340 w4368 w4395 w4441 w4449 w4455]
      tunnel: w4164 -> [w4175 w4179 w4189 w4195 w4207 w4225 w4283 w4334 w4367 w4389 w4437 w4445 w4452]
      tunnel: [w4175 w4182 w4191 w4200 w4212 w4234 w4304 w4339 w4376 w4394 w4440 w4448 w4463] -> w4173
      tunnel: [50 50 5 5 5 50 50 5 5 5 50 50 50] -> w4172
      tunnel: w4171 -> [w4176 w4180 w4186 w4197 w4209 w4231 w4300 w4335 w4372 w4390 w4438 w4446 w4461]
      tunnel: [w4176 w4180 w4186 w4197 w4209 w4231 w4300 w4335 w4372 w4390 w4438 w4446 w4461] -> w4170
      tunnel: w4166 -> [_ _ _ _ _ _ _ _ _ _ _ _ _]
      tunnel: w4162 -> [_ _ _ _ _ w4226 _ w4331 _ _ _ _ _]
      tunnel: w4161 -> [_ _ _ _ _ w4220 w4282 _ w4359 w4388 _ _ _]
      tunnel: w4160 -> [_ _ _ _ _ _ w4286 _ w4355 _ _ _ _]
      tunnel: w4159 -> [_ _ _ _ _ _ _ w4332 _ w4384 _ _ _]
      tunnel: w4158 -> [_ _ _ _ _ _ _ _ _ w4381 _ _ _]
      frame "No event", Default {
        # "Don't place any functions"
      }
      frame "<----自动加工------------->" {
        w4177 = u16 1 items=["HPRI"=1, "LPRI"=0] ("priority")
        # "//读取配置文件"
        n1615 = call "Enqueue Element Array.vi"("priority"=w4177, "queue index"=1, "error in"=w4179, "master data"="" ("Element 1"), "queue in"=w4183) -> ("error out"=w4182:errorcluster)  [unwired: 5 in, 1 out]
      }
      frame "自动开始" {
        w4187 = u16 1 items=["HPRI"=1, "LPRI"=0] ("priority")
        n1616 = call "Enqueue Element Array.vi"("priority"=w4187, "queue index"=1, "error in"=w4189, "master data"="清除状态信息" ("Element 1"), "queue in"=w4185) -> ("error out"=w4191:errorcluster)  [unwired: 5 in, 1 out]
      }
      frame "Loading Variable" {
        w4198 = u16 1 items=["HPRI"=1, "LPRI"=0] ("priority")
        n1617 = disable-structure shown="启用" {
          disable-tunnel: w4195 -> [w4205 _]
          disable-tunnel: [w4204 _] -> w4194
          frame Disabled {
            n1618 = call "Initial7230.vi"("error in (no error)"=w4205) -> ("error out"=w4204:errorcluster, "task out Output"=→"task out Output 2":refnum<k7>, "task out Input"=→"task out Input 2":refnum<k7>)  [unwired: 8 in]
          }
          frame Enabled {
          }
        }
        n1619 = call "Enqueue Element Array.vi"("priority"=w4198, "device error in"=w4194, "queue index"=1, "error in"=w4195, "master data"="Open PLC Connect" ("Element 1"), "queue in"=w4196) -> ("error out"=w4200:errorcluster)  [unwired: 4 in, 1 out]
      }
      frame "Open PLC Connect" {
        w4210 = u16 1 items=["HPRI"=1, "LPRI"=0] ("priority")
        n1620 = call "Enqueue Element Array.vi"("priority"=w4210, "queue index"=1, "error in"=w4207, "master data"="R/W PLC Signal" ("Element 1"), "queue in"=w4208) -> ("error out"=w4212:errorcluster)  [unwired: 5 in, 1 out]
      }
      frame "R/W PLC Signal" {
        (unwired) "R/W PLC Signal" ("Element 1")
        w4232 = u16 1 items=["HPRI"=1, "LPRI"=0] ("priority")
        # "R/W PLC Signal"
        n1621 = control-ref of="设备状态"() -> (w4229:refnum<vi>)
        n1622 = disable-structure shown="启用" {
          disable-tunnel: w4226 -> [w4241 _]
          disable-tunnel: w4220 -> [w4240 _]
          disable-tunnel: [w4239 _] -> _
          disable-tunnel: w4225 -> [w4238 _]
          disable-tunnel: [_ T22."Enabled" ("禁用")] -> w4224
          disable-tunnel: [_ TRUE ("可见")] -> w4223
          disable-tunnel: [_ w4269] -> w4221
          frame Disabled {
            n1623 = call <vilib>:"Acquire Semaphore.vi"("error in (no error)"=w4240, "semaphore"=w4241) -> ("error out"=w4236:errorcluster, "semaphore out"=w4237:T23)  [unwired: 3 in, 1 out]
            n1624 = case shown="无错误" w4236 {
              selector: w4236 -> [w4242 _]
              tunnel: w4238 -> [w4246 w4264]
              tunnel: [w4245 w4264] -> w4239
              tunnel: w4237 -> [w4244 _]
              frame No Error {
                n1625 = flat-sequence {
                  tunnel: w4246 -> [w4251]
                  tunnel: [w4250] -> w4245
                  tunnel: [w4248] -> w4243
                  tunnel: w4244 -> [w4248]
                  frame #0 {
                    n1626 = local read "task out Input"() -> (w4255:refnum<k7>)
                    n1627 = local read "task out Output"() -> (w4254:refnum<k7>)
                    n1628 = disable-structure shown="禁用" {
                      disable-tunnel: w4255 -> [w4263 _]
                      disable-tunnel: w4254 -> [w4262 _]
                      disable-tunnel: [w4261 _] -> w4253
                      disable-tunnel: [w4260 _] -> w4252
                      disable-tunnel: w4251 -> [w4259 _]
                      disable-tunnel: [w4258 _] -> w4250
                      disable-tunnel: [w4256 _] -> _
                      disable-tunnel: [w4257 _] -> w4249
                      disable-tunnel: "输出OUTPUT" -> [w4256 _]
                      frame Disabled {
                        n1629 = call "adlink7230ReadAndWriteIO.vi"("error in (no error)"=w4259, "输出OUTPUT 2"=w4256, "task in Output"=w4262, "task in Input"=w4263) -> ("error out"=w4258:errorcluster, "输入INPUT 2"=w4257:T46, "task out Output"=w4260:refnum<k7>, "task out Input"=w4261:refnum<k7>)  [unwired: 3 in, 1 out]
                      }
                      frame Enabled {
                      }
                    }
                    "输入INPUT" <- w4249
                    n1630 = local write "task out Output"(w4252) -> ()
                    n1631 = local write "task out Input"(w4253) -> ()
                  }
                }
                n1632 = call <vilib>:"Release Semaphore.vi"("error in (no error)"=w4242, "semaphore"=w4243) -> ()  [unwired: 4 in, 2 out]
              }
              frame Error {
              }
            }
          }
          frame Enabled {
            n1633 = local read "DB5000.X"() -> (w4267:T4)
            n1634 = Unbundle By Name(w4267) -> ("数据传递\n信号-读"=w4265:bool, "PLC初始化\n信号-读"=w4266:bool)
            n1635 = Build Array(w4265, w4266) -> (w4271:bool[])
            n1636 = Boolean Array To Number(Boolean array=w4271) -> (number=w4270:u32)
            n1637 = case shown="0, 默认" w4270 {
              tunnel: ["R/W PLC Signal" ("Element 1") w4275 "检测项复位" ("Element 1")] -> w4269
              frame 0, Default {
              }
              frame 1 {
                n1638 = local read "lock"() -> (w4274:bool)
                n1639 = case shown="真" w4274 {
                  selector: w4274 -> [_ w4278]
                  tunnel: ["R/W PLC Signal" ("Element 1") "清除状态信息" ("Element 1")] -> w4275
                  frame False {
                  }
                  frame True {
                    n1640 = Not(x=w4278) -> (.not. x?=w4277:bool)
                    n1641 = local write "lock"(w4277) -> ()
                  }
                }
              }
              frame 2 {
              }
            }
          }
        }
        n1642 = call "UPdataMessage.vi"("错误输入（无错误）"=w4225, "Str引用句柄"=w4229) -> ("error out"=w4228:errorcluster)  [unwired: 9 in]
        n1643 = local read "电脑一表面检测图像处理状态"() -> (w4217:bool)
        n1644 = local read "电脑一CCD读字符状态"() -> (w4218:bool)
        n1645 = local read "电脑一穿管检测状态"() -> (w4216:bool)
        n1646 = local read "电脑一穿管压力获取状态"() -> (w4215:bool)
        n1647 = local read "电脑一条码枪扫码状态"() -> (w4219:bool)
        n1648 = call "布尔字符串转换.vi"("布尔"=w4219, "布尔 2"=w4218, "布尔 3"=w4217, "布尔 4"=w4216, "布尔 5"=w4215) -> ("连接的字符串"=w4214:string)  [unwired: 10 in]
        n1649 = shared-variable "我的电脑\\网络共享变量库.lvlib\\电脑一运行状态字符串"(w4214) -> ()  [unwired: 1 in, 1 out]
        n1650 = property on="User Login" class="Bool (严格)"(error in=w4220, "DisabledEnum"=w4224, "Visible"=w4223) -> (error out=w4222:errorcluster)  [unwired: 1 in, 1 out]
        n1651 = Merge Errors(w4228, w4222) -> (w4227:errorcluster)
        n1652 = call "Enqueue Element Array.vi"("priority"=w4232, "device error in"=w4227, "queue index"=1, "error in"=w4225, "master data"=w4221, "queue in"=w4230) -> ("error out"=w4234:errorcluster)  [unwired: 4 in, 1 out]
      }
      frame "清除状态信息" {
        (unwired) FALSE
        w4301 = u16 0 items=["HPRI"=1, "LPRI"=0] ("priority")
        # "打开TCP连接"
        n1653 = local read "DB5000.X"() -> (w4285:T4)
        n1654 = Unbundle By Name(w4285) -> ("电脑1返工\n信号-写"=w4284:bool)
        n1655 = Or(x=w4284, y="返工按钮") -> (x .or. y?=w4297:bool)
        n1656 = case shown="真" w4297 {
          tunnel: ["0" ("电脑一新返工1") "1" ("电脑一新返工1")] -> w4299
          frame False {
          }
          frame True {
          }
        }
        n1657 = flat-sequence {
          tunnel: w4299 -> [w4314]
          tunnel: [w4313] -> w4296
          tunnel: [w4312] -> w4295
          tunnel: [w4311] -> w4294
          tunnel: [w4308] -> w4293
          tunnel: w4286 -> [w4310]
          tunnel: [w4309] -> w4287
          tunnel: w4282 -> [w4307]
          tunnel: w4296 -> [w4321]
          tunnel: w4295 -> [w4320]
          tunnel: w4294 -> [w4319]
          tunnel: w4293 -> [w4318]
          tunnel: [w4321] -> w4292
          tunnel: [w4320] -> w4291
          tunnel: [w4319] -> w4290
          tunnel: [w4318] -> w4289
          tunnel: [w4316] -> w4288
          tunnel: w4287 -> [w4316]
          tunnel: w4292 -> [w4328]
          tunnel: w4291 -> [w4327]
          tunnel: w4290 -> [w4326]
          tunnel: w4289 -> [w4325]
          tunnel: [w4324] -> w4281
          tunnel: w4288 -> [w4323]
          frame #0 {
            (unwired) 0.5 ("Delay Time (s)")
            n1658 = call "SQL读取.vi"("error in (no error)"=w4307, "ADODB._Connection In"=w4310, "电脑一新返工1"=w4314) -> ("error out"=w4308:errorcluster, "computer3"=w4311:string, "computer2"=w4312:string, "computer1"=w4313:string, "传递信息显示"=→"传递信息显示":string, "ADODB._Connection Out"=w4309:refnum<k7>)  [unwired: 3 in]
            "computer1" <- w4313
            "computer2" <- w4312
            "computer3" <- w4311
          }
          frame #1 {
            n1659 = disable-structure shown="禁用" {
              frame Disabled {
                n1660 = call "标签打印.vi"() -> ()  [unwired: 10 in, 2 out]
              }
              frame Enabled {
              }
            }
            n1661 = Wait (ms)(milliseconds to wait=u32 5 ("等待时间（毫秒）")) -> ()  [unwired: 1 out]
          }
          frame #2 {
            n1662 = local write "lock"(TRUE ("lock")) -> ()
            n1663 = call "SQL删除.vi"("computer1"=w4328, "ADODB._Connection In"=w4323, "computer2"=w4327, "computer3"=w4326, "error in (no error)"=w4325) -> ("error out"=w4324:errorcluster)  [unwired: 10 in]
          }
        }
        n1664 = call "Enqueue Element Array.vi"("priority"=w4301, "device error in"=w4281, "queue index"=1, "error in"=w4283, "master data"="Updata" ("Element 1"), "queue in"=w4305) -> ("error out"=w4304:errorcluster)  [unwired: 4 in, 1 out]
      }
      frame "Updata" {
        w4337 = u16 0 items=["HPRI"=1, "LPRI"=0] ("priority")
        n1665 = disable-structure shown="启用" {
          disable-tunnel: w4334 -> [w4346 w4353]
          disable-tunnel: [w4345 w4348] -> w4333
          disable-tunnel: w4332 -> [_ w4351]
          disable-tunnel: w4331 -> [_ w4350]
          frame Disabled {
            n1666 = local read "computer2"() -> (w4343:string)
            n1667 = local read "computer3"() -> (w4342:string)
            n1668 = local read "computer1"() -> (w4344:string)
            n1669 = call "SQL删除.vi"("computer1"=w4344, "computer2"=w4343, "computer3"=w4342, "error in (no error)"=w4346) -> ("error out"=w4345:errorcluster)  [unwired: 11 in]
          }
          frame Enabled {
            n1670 = call "DB5000.X写.vi"("引用"=w4351, "semaphore"=w4350, "地址名称"="数据传递信号-读" ("组合框"), "value"=FALSE, "error in (no error)"=w4353) -> ("error out"=w4352:errorcluster)  [unwired: 9 in, 1 out]
            n1671 = call "时间延迟"("error in (no error)"=w4352, "Delay Time (s)"=0.5) -> ("error out"=w4348:errorcluster)  [unwired: 9 in]
          }
        }
        n1672 = call "Enqueue Element Array.vi"("priority"=w4337, "device error in"=w4333, "queue index"=1, "error in"=w4334, "master data"="Loading Variable", "queue in"=w4340) -> ("error out"=w4339:errorcluster)  [unwired: 4 in, 1 out]
      }
      frame "检测项复位" {
        w4356 = TRUE ("type_c")
        w4371 = u16 1 items=["HPRI"=1, "LPRI"=0] ("priority")
        w4374 = u16 0 items=["HPRI"=1, "LPRI"=0] ("priority")
        n1673 = disable-structure shown="禁用" {
          frame Disabled {
            n1674 = shared-variable "我的电脑\\PLC-OPC.lvlib\\PLC初始化信号"() -> ()  [unwired: 1 in, 2 out]
          }
          frame Enabled {
          }
        }
        n1675 = call "Enqueue Element Array.vi"("priority"=w4371, "queue index"=0, "error in"=w4367, "master data"="检测启动按钮" ("t"), "queue in"=w4368) -> ("error out"=w4365:errorcluster, "queue out"=w4366:T25)  [unwired: 5 in]
        n1676 = call "SQL-选择清空数据库.vi"("computer1"=TRUE ("computer 4"), "computer 2"=TRUE ("computer 4"), "ADODB._Connection Out"=w4355, "computer 3"=TRUE ("computer 4"), "computer 4"=TRUE, "error in (no error)"=w4359, "type_c"=w4356, "computer 5"=TRUE, "type_b"=w4356) -> ("ADODB._Connection Out 2"=w4357:refnum<k7>, "error out"=w4358:errorcluster)  [unwired: 9 in]
        n1677 = disable-structure shown="禁用" {
          disable-tunnel: w4357 -> [w4378 _]
          frame Disabled {
            n1678 = global write "Global System.vi" "ADODB._Connection Out"(w4378) -> ()
          }
          frame Enabled {
          }
        }
        n1679 = call "Enqueue Element Array.vi"("priority"=w4374, "device error in"=w4358, "queue index"=1, "error in"=w4365, "master data"="复位完成", "queue in"=w4366) -> ("error out"=w4376:errorcluster)  [unwired: 4 in, 1 out]
      }
      frame "复位完成" {
        w4392 = u16 0 items=["HPRI"=1, "LPRI"=0] ("priority")
        n1680 = flat-sequence {
          tunnel: w4388 -> [w4416]
          tunnel: [w4408] -> w4386
          tunnel: w4384 -> [w4407]
          tunnel: [w4399] -> w4382
          tunnel: w4381 -> [w4397]
          tunnel: [w4397] -> w4379
          tunnel: [w4427] -> w4387
          tunnel: w4386 -> [w4427]
          tunnel: [w4426] -> w4383
          tunnel: w4382 -> [w4426]
          tunnel: [w4425] -> w4380
          tunnel: w4379 -> [w4425]
          tunnel: w4387 -> [w4434]
          tunnel: [w4433] -> w4385
          tunnel: w4383 -> [w4431]
          tunnel: w4380 -> [w4429]
          frame #0 {
            w4398 = FALSE
            n1681 = call "DB5000.X写.vi"("引用"=w4407, "semaphore"=w4397, "地址名称"="穿管检测pass-写" ("组合框"), "value"=w4398, "error in (no error)"=w4416) -> ("引用输出"=w4406:refnum<k24>, "error out"=w4415:errorcluster)  [unwired: 9 in]
            n1682 = call "DB5000.X写.vi"("引用"=w4406, "semaphore"=w4397, "地址名称"="穿管检测fail-写" ("组合框"), "value"=w4398, "error in (no error)"=w4415) -> ("引用输出"=w4405:refnum<k24>, "error out"=w4414:errorcluster)  [unwired: 9 in]
            n1683 = call "DB5000.X写.vi"("引用"=w4405, "semaphore"=w4397, "地址名称"="表面检测pass-写" ("组合框"), "value"=w4398, "error in (no error)"=w4414) -> ("引用输出"=w4404:refnum<k24>, "error out"=w4413:errorcluster)  [unwired: 9 in]
            n1684 = call "DB5000.X写.vi"("引用"=w4404, "semaphore"=w4397, "地址名称"="表面检测fail-写" ("组合框"), "value"=w4398, "error in (no error)"=w4413) -> ("引用输出"=w4403:refnum<k24>, "error out"=w4412:errorcluster)  [unwired: 9 in]
            n1685 = call "DB5000.X写.vi"("引用"=w4403, "semaphore"=w4397, "地址名称"="字符1检测pass-写" ("组合框"), "value"=w4398, "error in (no error)"=w4412) -> ("引用输出"=w4402:refnum<k24>, "error out"=w4411:errorcluster)  [unwired: 9 in]
            n1686 = call "DB5000.X写.vi"("引用"=w4402, "semaphore"=w4397, "地址名称"="字符1检测fail-写" ("组合框"), "value"=w4398, "error in (no error)"=w4411) -> ("引用输出"=w4401:refnum<k24>, "error out"=w4410:errorcluster)  [unwired: 9 in]
            n1687 = call "DB5000.X写.vi"("引用"=w4401, "semaphore"=w4397, "地址名称"="扫码枪pass-写" ("组合框"), "value"=w4398, "error in (no error)"=w4410) -> ("引用输出"=w4400:refnum<k24>, "error out"=w4409:errorcluster)  [unwired: 9 in]
            n1688 = call "DB5000.X写.vi"("引用"=w4400, "semaphore"=w4397, "地址名称"="扫码枪fail-写" ("组合框"), "value"=w4398, "error in (no error)"=w4409) -> ("引用输出"=w4399:refnum<k24>, "error out"=w4408:errorcluster)  [unwired: 9 in]
          }
          frame #1 {
            n1689 = Wait (ms)(milliseconds to wait=u32 100 ("等待时间（毫秒）")) -> ()  [unwired: 1 out]
          }
          frame #2 {
            n1690 = call "DB5000.X写.vi"("引用"=w4431, "semaphore"=w4429, "地址名称"="PLC初始化信号-读" ("组合框"), "value"=FALSE, "error in (no error)"=w4434) -> ("error out"=w4433:errorcluster)  [unwired: 9 in, 1 out]
          }
        }
        n1691 = call "Enqueue Element Array.vi"("priority"=w4392, "device error in"=w4385, "queue index"=1, "error in"=w4389, "master data"="Loading Variable", "queue in"=w4395) -> ("error out"=w4394:errorcluster)  [unwired: 4 in, 1 out]
      }
      frame "<-----自动加工结束--------->" {
        w4435 = u16 1 items=["HPRI"=1, "LPRI"=0] ("priority")
        # "//读取配置文件"
        n1692 = call "Enqueue Element Array.vi"("priority"=w4435, "queue index"=1, "error in"=w4437, "master data"="" ("Element 1"), "queue in"=w4441) -> ("error out"=w4440:errorcluster)  [unwired: 5 in, 1 out]
      }
      frame "<----------手动部分------------->" {
        w4443 = u16 1 items=["HPRI"=1, "LPRI"=0] ("priority")
        # "//读取配置文件"
        n1693 = call "Enqueue Element Array.vi"("priority"=w4443, "queue index"=1, "error in"=w4445, "master data"="" ("Element 1"), "queue in"=w4449) -> ("error out"=w4448:errorcluster)  [unwired: 5 in, 1 out]
      }
      frame "*Emergency alarm" {
        w4458 = u16 1 items=["HPRI"=1, "LPRI"=0] ("priority")
        w4459 = u16 1 items=["HPRI"=1, "LPRI"=0] ("priority")
        # "发出处理急停信号的命令"
        # "发出处理急停信号的命令"
        n1694 = call "Enqueue Element Array.vi"("priority"=w4458, "queue index"=0, "error in"=w4452, "master data"="" ("Element 1"), "queue in"=w4455) -> ("error out"=w4453:errorcluster, "queue out"=w4454:T25)  [unwired: 5 in]
        n1695 = call "SetTestInfoIndex.vi"("test info index"=13) -> ()
        n1696 = call "Enqueue Element Array.vi"("priority"=w4459, "queue index"=1, "error in"=w4453, "master data"="" ("Element 1"), "queue in"=w4454) -> ("error out"=w4463:errorcluster)  [unwired: 5 in, 1 out]
      }
    }
    n1697 = Wait (ms)(milliseconds to wait=w4172) -> ()  [unwired: 1 out]
  }
  n1698 = call "Release Queue Array.vi"("error in"=w12) -> ("error out"=w11:errorcluster)  [unwired: 3 in, 3 out]
  n1699 = call "Release Queue Array.vi"("error in"=w31, "queue in"=w15) -> ("error out"=w22:errorcluster)  [unwired: 2 in, 3 out]
  n1700 = call "Release Queue Array.vi"("error in"=w13, "queue in"=w15) -> ("error out"=w25:errorcluster)  [unwired: 2 in, 3 out]
  n1701 = call "Release Queue Array.vi"("error in"=w30, "queue in"=w15) -> ("error out"=w19:errorcluster)  [unwired: 2 in, 3 out]
  n1702 = call "Release Queue Array.vi"("error in"=w27, "queue in"=w15) -> ("error out"=w20:errorcluster)  [unwired: 2 in, 3 out]
  n1703 = call "Release Queue Array.vi"("error in"=w33, "queue in"=w15) -> ("error out"=w36:errorcluster)  [unwired: 2 in, 3 out]
  n1704 = call "Release Queue Array.vi"("error in"=w32, "queue in"=w15) -> ("error out"=w21:errorcluster)  [unwired: 2 in, 3 out]
  n1705 = call "Release Queue Array.vi"("error in"=w24, "queue in"=w15) -> ("error out"=w23:errorcluster)  [unwired: 2 in, 3 out]
  n1706 = Build Array(w11, w21, w22, w23, w25) -> (w29:errorcluster[])
  n1707 = call "Release Queue Array.vi"("error in"=w34, "queue in"=w15) -> ("error out"=w38:errorcluster)  [unwired: 2 in, 3 out]
  n1708 = call "MergeErrors.vi"("error in 1 (no error)"=w20, "error in 2 (no error)"=w36, "error in 3 (no error)"=w19, "error in 4 (no error)"=w38, "error array in"=w29) -> ("error out"=w37:errorcluster)  [unwired: 3 in]
  n1709 = call "ExitAppMode.vi"("error in (no error)"=w37) -> ("error out"=w35:errorcluster)  [unwired: 10 in]
  n1710 = call <vilib>:"Clear Errors.vi"("error in (no error)"=w35) -> ()  [unwired: 5 in, 2 out]
  "lock" <- TRUE ("lock")
